vi "RTS Combination Server.vi"() -> ()   [LabVIEW 2016]
uses:
  Drivers/WAGO 750-881/Type Definitions/Wago Main Control.ctl
  Drivers/WAGO 750-881/Type Definitions/Wago Output Data Process Image.ctl
  Drivers/WAGO 750-881/Type Definitions/Wago Room Condtions.ctl
  Drivers/WAGO 750-881/Type Definitions/Wago Door Relays.ctl
  Drivers/WAGO 750-881/Type Definitions/Wago Contactor Settings.ctl
  Drivers/WAGO 750-881/Type Definitions/Wago Ground Leakage.ctl
  Drivers/WAGO 750-881/Type Definitions/Wago Input Process Image.ctl
  Drivers/WAGO 750-881/Type Definitions/Wago Room PID Settings.ctl
  Drivers/WAGO 750-881/Type Definitions/Wago Measured Input Data.ctl
  Drivers/WAGO 750-881/Type Definitions/Wago Room Setpoint Targets.ctl
  Type Definitions/RTS Modbus Connections.ctl
  <vilib>/NI/Modbus Library/API/Master/Modbus Master.lvclass
  Drivers/Yokogawa MX100/Type Definitions/MX100 Initialization.ctl
  Drivers/Yokogawa MX100/Type Definitions/MX100 Data.ctl
  Type Definitions/RTS Configuration Setup.ctl
  Type Definitions/RTS Wago Config.ctl
  Type Definitions/RTS APLUS Config.ctl
  Type Definitions/RTS Yokogawa MX Config.ctl
  Type Definitions/RTS Replay Server Control.ctl
  Type Definitions/RTS Server Configuration.ctl
  Type Definitions/RTS Station Settions TCP Comms.ctl
  Type Definitions/RTS Chamber Save Status.ctl
  Type Definitions/RTS Test Pattern.ctl
  Type Definitions/RTS Chamber Data.ctl
  Utility/Type Definitions/UTILITY Power Data.ctl
  Type Definitions/RTS Chamber TCs.ctl
  Type Definitions/RTS MX5 AUX Data.ctl
  Type Definitions/RTS TDMS Filename Locations.ctl
  Type Definitions/RTS Save References.ctl
  Type Definitions/RTS All Station Door Opener Ctrl.ctl
  Type Definitions/RTS Station Relay Ops.ctl
  Type Definitions/RTS Door Opener Indicator.ctl
  Type Definitions/RTS Door Ops Client.ctl
  Type Definitions/RTS Door Opening Schedule.ctl
  Type Definitions/RTS Door Ops Sequence.ctl
  Drivers/WAGO 750-881/Type Definitions/Wago Ground Leakage Relays.ctl
  Drivers/WAGO 750-881/Type Definitions/Wago Polarity Selector Relays.ctl
  Drivers/WAGO 750-881/Type Definitions/Wago Polarity Selector.ctl
  Type Definitions/RTS Chamber Temperature Humidity Control.ctl
  Type Definitions/RTS Frequency Selector.ctl
  Type Definitions/RTS Reset Watt Hours.ctl
  Drivers/WAGO 750-881/Type Definitions/Wago Voltage Adjustment Parameters.ctl
  Drivers/WAGO 750-881/Type Definitions/Wago Door Settings.ctl
  Drivers/WAGO 750-881/Type Definitions/Wago Door Relays By Station.ctl
  Drivers/WAGO 750-881/Type Definitions/Wago Door Operation.ctl
  Type Definitions/RTS Enable Door Openers.ctl
  Type Definitions/RTS Select System Number.ctl
  Drivers/WAGO 750-881/Type Definitions/Wago Room Run.ctl
  Drivers/WAGO 750-881/Type Definitions/Wago Room Enable.ctl
  Type Definitions/RTS Save Titles.ctl
  <vilib>/event_ctls.llb/usereventprio.ctl
  Drivers/WAGO 750-881/Type Definitions/Wago Input Commands.ctl
  Type Definitions/RTS TCP Multiple Connections Data.ctl
  Type Definitions/RTS Room Selector.ctl
  <vilib>/Utility/error.llb/whitespace.ctl
  <vilib>/NI/Modbus Library/API/Wrapper/Create TCP Master.vi
  <vilib>/NI/Modbus Library/API/Wrapper/API Main.lvlib
panel:
  in  "Save Array":bool
  out "Save Array":string[](array[string])
  out "Exit":bool=TRUE
  out "Start Data Save Loop":bool=TRUE
  in  "Save Rate (Sec)":i32=50
  out "Custom Saved Title Save Loop":T1
  out "TDMS Data Save Loop":T2
  out "RTS Config Setup Save Loop":T4
  out "All Door Opener Ctrl 2":T13 {"Station 8"."Station Slide"."Chamber 1-1"."Start Time" format="%<%X\n%x>T"; "Station 8"."Station Slide"."Chamber 1-1"."End Time" format="%<%X\n%x>T"; "Station 8"."Station Slide"."Time Count (s)" format="%.2f"; "Station 8"."Station Cab"."Chamber 1-1"."Start Time" format="%<%X\n%x>T"; "Station 8"."Station Cab"."Chamber 1-1"."End Time" format="%<%X\n%x>T"; "Station 8"."Station Cab"."Time Count (s)" format="%.2f"; "Station 8"."Station Freezer"."Chamber 1-1"."Start Time" format="%<%X\n%x>T"; "Station 8"."Station Freezer"."Chamber 1-1"."End Time" format="%<%X\n%x>T"; "Station 8"."Station Freezer"."Time Count (s)" format="%.2f"; "Station 7"."Station Slide"."Chamber 1-1"."Start Time" format="%<%X\n%x>T"; "Station 7"."Station Slide"."Chamber 1-1"."End Time" format="%<%X\n%x>T"; "Station 7"."Station Slide"."Time Count (s)" format="%.2f"; "Station 7"."Station Cab"."Chamber 1-1"."Start Time" format="%<%X\n%x>T"; "Station 7"."Station Cab"."Chamber 1-1"."End Time" format="%<%X\n%x>T"; "Station 7"."Station Cab"."Time Count (s)" format="%.2f"; "Station 7"."Station Freezer"."Chamber 1-1"."Start Time" format="%<%X\n%x>T"; "Station 7"."Station Freezer"."Chamber 1-1"."End Time" format="%<%X\n%x>T"; "Station 7"."Station Freezer"."Time Count (s)" format="%.2f"; "Station 6"."Station Slide"."Chamber 1-1"."Start Time" format="%<%X\n%x>T"; "Station 6"."Station Slide"."Chamber 1-1"."End Time" format="%<%X\n%x>T"; "Station 6"."Station Slide"."Time Count (s)" format="%.2f"; "Station 6"."Station Cab"."Chamber 1-1"."Start Time" format="%<%X\n%x>T"; "Station 6"."Station Cab"."Chamber 1-1"."End Time" format="%<%X\n%x>T"; "Station 6"."Station Cab"."Time Count (s)" format="%.2f"; "Station 6"."Station Freezer"."Chamber 1-1"."Start Time" format="%<%X\n%x>T"; "Station 6"."Station Freezer"."Chamber 1-1"."End Time" format="%<%X\n%x>T"; "Station 6"."Station Freezer"."Time Count (s)" format="%.2f"; "Station 5"."Station Slide"."Chamber 1-1"."Start Time" format="%<%X\n%x>T"; "Station 5"."Station Slide"."Chamber 1-1"."End Time" format="%<%X\n%x>T"; "Station 5"."Station Slide"."Time Count (s)" format="%.2f"; "Station 5"."Station Cab"."Chamber 1-1"."Start Time" format="%<%X\n%x>T"; "Station 5"."Station Cab"."Chamber 1-1"."End Time" format="%<%X\n%x>T"; "Station 5"."Station Cab"."Time Count (s)" format="%.2f"; "Station 5"."Station Freezer"."Chamber 1-1"."Start Time" format="%<%X\n%x>T"; "Station 5"."Station Freezer"."Chamber 1-1"."End Time" format="%<%X\n%x>T"; "Station 5"."Station Freezer"."Time Count (s)" format="%.2f"; "Station 4"."Station Slide"."Chamber 1-1"."Start Time" format="%<%X\n%x>T"; "Station 4"."Station Slide"."Chamber 1-1"."End Time" format="%<%X\n%x>T"; "Station 4"."Station Slide"."Time Count (s)" format="%.2f"; "Station 4"."Station Cab"."Chamber 1-1"."Start Time" format="%<%X\n%x>T"; "Station 4"."Station Cab"."Chamber 1-1"."End Time" format="%<%X\n%x>T"; "Station 4"."Station Cab"."Time Count (s)" format="%.2f"; "Station 4"."Station Freezer"."Chamber 1-1"."Start Time" format="%<%X\n%x>T"; "Station 4"."Station Freezer"."Chamber 1-1"."End Time" format="%<%X\n%x>T"; "Station 4"."Station Freezer"."Time Count (s)" format="%.2f"; "Station 3"."Station Slide"."Chamber 1-1"."Start Time" format="%<%X\n%x>T"; "Station 3"."Station Slide"."Chamber 1-1"."End Time" format="%<%X\n%x>T"; "Station 3"."Station Slide"."Time Count (s)" format="%.2f"; "Station 3"."Station Cab"."Chamber 1-1"."Start Time" format="%<%X\n%x>T"; "Station 3"."Station Cab"."Chamber 1-1"."End Time" format="%<%X\n%x>T"; "Station 3"."Station Cab"."Time Count (s)" format="%.2f"; "Station 3"."Station Freezer"."Chamber 1-1"."Start Time" format="%<%X\n%x>T"; "Station 3"."Station Freezer"."Chamber 1-1"."End Time" format="%<%X\n%x>T"; "Station 3"."Station Freezer"."Time Count (s)" format="%.2f"; "Station 2"."Station Slide"."Chamber 1-1"."Start Time" format="%<%X\n%x>T"; "Station 2"."Station Slide"."Chamber 1-1"."End Time" format="%<%X\n%x>T"; "Station 2"."Station Slide"."Time Count (s)" format="%.2f"; "Station 2"."Station Cab"."Chamber 1-1"."Start Time" format="%<%X\n%x>T"; "Station 2"."Station Cab"."Chamber 1-1"."End Time" format="%<%X\n%x>T"; "Station 2"."Station Cab"."Time Count (s)" format="%.2f"; "Station 2"."Station Freezer"."Chamber 1-1"."Start Time" format="%<%X\n%x>T"; "Station 2"."Station Freezer"."Chamber 1-1"."End Time" format="%<%X\n%x>T"; "Station 2"."Station Freezer"."Time Count (s)" format="%.2f"; "Station 1"."Station Slide"."Chamber 1-1"."Start Time" format="%<%X\n%x>T"; "Station 1"."Station Slide"."Chamber 1-1"."End Time" format="%<%X\n%x>T"; "Station 1"."Station Slide"."Time Count (s)" format="%.2f"; "Station 1"."Station Cab"."Chamber 1-1"."Start Time" format="%<%X\n%x>T"; "Station 1"."Station Cab"."Chamber 1-1"."End Time" format="%<%X\n%x>T"; "Station 1"."Station Cab"."Time Count (s)" format="%.2f"; "Station 1"."Station Freezer"."Chamber 1-1"."Start Time" format="%<%X\n%x>T"; "Station 1"."Station Freezer"."Chamber 1-1"."End Time" format="%<%X\n%x>T"; "Station 1"."Station Freezer"."Time Count (s)" format="%.2f"}
  out "System Number":T19="Sys1"
  in  "Disable MX":bool
  in  "Main Array":bool
  in  "All Data?":bool=TRUE
  in  "CSV Data Save":T2
  out "Main Array":string[](array[string])
  in  "Disable APLUS":bool
  in  "Initialize Rate":bool
  in  "Main Loop Rate (Seconds)":dbl=1.0
  out "Rate":dbl format="%0.2f"
  in  "K(0.3)":dbl=0.3 format="%#_13g"
  out "Chamber 1 Connections":i32
  in  "Tab Control":T20(tab)
  out "Chamber Data":T21 {"Room PID Settings"."Room Dehumid Temperature I (*RM Dehum I1)" max=30000 step=1; "Room PID Settings"."Room Dehumid Temperature P (*RM Dehum P1)" max=30000 step=1; "Room PID Settings"."Room Cool Temperature I (*RM Cool I1)" max=30000 step=1; "Room PID Settings"."Room Cool Temperature P (*RM Cool P1)" max=30000 step=1; "Room PID Settings"."Room Heat I (*RM Heat I1)" max=30000 step=1; "Room PID Settings"."Room Heat P (*RM Heat P1)" max=30000 step=1; "Room PID Settings"."Room Humidity I (*RM Hum I1)" max=30000 step=1; "Room PID Settings"."Room Humidity P (*RM Hum P1)" max=30000 step=1; "Room PID Settings"."Room Dry I (*RM Dry I1)" max=30000 step=1; "Room PID Settings"."Room Dry P(*RM Dry P1)" max=30000 step=1; "Station 8"."Voltage (V):Element 1 Avg" format="%.3g"; "Station 8"."Voltage (V):Element 2 Avg" format="%.3g"; "Station 8"."Max Watt Hours" format="%.3g"; "Station 8"."Power Factor:Element 2" format="%.3g"; "Station 8"."Power Factor:Element 1" format="%.3g"; "Station 8"."Apparent Power (VA):Element 2" format="%.3g"; "Station 8"."Apparent Power (VA):Element 1" format="%.3g"; "Station 8"."Frequency (Hz):Element 1" format="%.3g"; "Station 8"."Time:Element 1" format="%.3g"; "Station 8"."Voltage Crest Factor:Element 2" format="%.3g"; "Station 8"."Voltage Crest Factor:Element 1" format="%.3g"; "Station 8"."Voltage Harmonic (%):Element 2" format="%.3g"; "Station 8"."Voltage Harmonic (%):Element 1" format="%.3g"; "Station 8"."Current Crest Factor:Element 2" format="%.3g"; "Station 8"."Current Crest Factor:Element 1" format="%.3g"; "Station 8"."Voltage (V):Element 1" format="%.3g"; "Station 8"."Voltage (V):Element 2" format="%.3g"; "Station 8"."Watt Hours (Wh):Sigma" format="%.3f"; "Station 8"."Power (W):Sigma" format="%.3g"; "Station 8"."Current (A):Element 2" format="%.3g"; "Station 8"."Current (A):Element 1" format="%.3g"; "Station 7"."Voltage (V):Element 1 Avg" format="%.3g"; "Station 7"."Voltage (V):Element 2 Avg" format="%.3g"; "Station 7"."Max Watt Hours" format="%.3g"; "Station 7"."Power Factor:Element 2" format="%.3g"; "Station 7"."Power Factor:Element 1" format="%.3g"; "Station 7"."Apparent Power (VA):Element 2" format="%.3g"; "Station 7"."Apparent Power (VA):Element 1" format="%.3g"; "Station 7"."Frequency (Hz):Element 1" format="%.3g"; "Station 7"."Time:Element 1" format="%.3g"; "Station 7"."Voltage Crest Factor:Element 2" format="%.3g"; "Station 7"."Voltage Crest Factor:Element 1" format="%.3g"; "Station 7"."Voltage Harmonic (%):Element 2" format="%.3g"; "Station 7"."Voltage Harmonic (%):Element 1" format="%.3g"; "Station 7"."Current Crest Factor:Element 2" format="%.3g"; "Station 7"."Current Crest Factor:Element 1" format="%.3g"; "Station 7"."Voltage (V):Element 1" format="%.3g"; "Station 7"."Voltage (V):Element 2" format="%.3g"; "Station 7"."Watt Hours (Wh):Sigma" format="%.3f"; "Station 7"."Power (W):Sigma" format="%.3g"; "Station 7"."Current (A):Element 2" format="%.3g"; "Station 7"."Current (A):Element 1" format="%.3g"; "Station 6"."Voltage (V):Element 1 Avg" format="%.3g"; "Station 6"."Voltage (V):Element 2 Avg" format="%.3g"; "Station 6"."Max Watt Hours" format="%.3g"; "Station 6"."Power Factor:Element 2" format="%.3g"; "Station 6"."Power Factor:Element 1" format="%.3g"; "Station 6"."Apparent Power (VA):Element 2" format="%.3g"; "Station 6"."Apparent Power (VA):Element 1" format="%.3g"; "Station 6"."Frequency (Hz):Element 1" format="%.3g"; "Station 6"."Time:Element 1" format="%.3g"; "Station 6"."Voltage Crest Factor:Element 2" format="%.3g"; "Station 6"."Voltage Crest Factor:Element 1" format="%.3g"; "Station 6"."Voltage Harmonic (%):Element 2" format="%.3g"; "Station 6"."Voltage Harmonic (%):Element 1" format="%.3g"; "Station 6"."Current Crest Factor:Element 2" format="%.3g"; "Station 6"."Current Crest Factor:Element 1" format="%.3g"; "Station 6"."Voltage (V):Element 1" format="%.3g"; "Station 6"."Voltage (V):Element 2" format="%.3g"; "Station 6"."Watt Hours (Wh):Sigma" format="%.3f"; "Station 6"."Power (W):Sigma" format="%.3g"; "Station 6"."Current (A):Element 2" format="%.3g"; "Station 6"."Current (A):Element 1" format="%.3g"; "Station 5"."Voltage (V):Element 1 Avg" format="%.3g"; "Station 5"."Voltage (V):Element 2 Avg" format="%.3g"; "Station 5"."Max Watt Hours" format="%.3g"; "Station 5"."Power Factor:Element 2" format="%.3g"; "Station 5"."Power Factor:Element 1" format="%.3g"; "Station 5"."Apparent Power (VA):Element 2" format="%.3g"; "Station 5"."Apparent Power (VA):Element 1" format="%.3g"; "Station 5"."Frequency (Hz):Element 1" format="%.3g"; "Station 5"."Time:Element 1" format="%.3g"; "Station 5"."Voltage Crest Factor:Element 2" format="%.3g"; "Station 5"."Voltage Crest Factor:Element 1" format="%.3g"; "Station 5"."Voltage Harmonic (%):Element 2" format="%.3g"; "Station 5"."Voltage Harmonic (%):Element 1" format="%.3g"; "Station 5"."Current Crest Factor:Element 2" format="%.3g"; "Station 5"."Current Crest Factor:Element 1" format="%.3g"; "Station 5"."Voltage (V):Element 1" format="%.3g"; "Station 5"."Voltage (V):Element 2" format="%.3g"; "Station 5"."Watt Hours (Wh):Sigma" format="%.3f"; "Station 5"."Power (W):Sigma" format="%.3g"; "Station 5"."Current (A):Element 2" format="%.3g"; "Station 5"."Current (A):Element 1" format="%.3g"; "Station 4"."Voltage (V):Element 1 Avg" format="%.3g"; "Station 4"."Voltage (V):Element 2 Avg" format="%.3g"; "Station 4"."Max Watt Hours" format="%.3g"; "Station 4"."Power Factor:Element 2" format="%.3g"; "Station 4"."Power Factor:Element 1" format="%.3g"; "Station 4"."Apparent Power (VA):Element 2" format="%.3g"; "Station 4"."Apparent Power (VA):Element 1" format="%.3g"; "Station 4"."Frequency (Hz):Element 1" format="%.3g"; "Station 4"."Time:Element 1" format="%.3g"; "Station 4"."Voltage Crest Factor:Element 2" format="%.3g"; "Station 4"."Voltage Crest Factor:Element 1" format="%.3g"; "Station 4"."Voltage Harmonic (%):Element 2" format="%.3g"; "Station 4"."Voltage Harmonic (%):Element 1" format="%.3g"; "Station 4"."Current Crest Factor:Element 2" format="%.3g"; "Station 4"."Current Crest Factor:Element 1" format="%.3g"; "Station 4"."Voltage (V):Element 1" format="%.3g"; "Station 4"."Voltage (V):Element 2" format="%.3g"; "Station 4"."Watt Hours (Wh):Sigma" format="%.3f"; "Station 4"."Power (W):Sigma" format="%.3g"; "Station 4"."Current (A):Element 2" format="%.3g"; "Station 4"."Current (A):Element 1" format="%.3g"; "Station 3"."Voltage (V):Element 1 Avg" format="%.3g"; "Station 3"."Voltage (V):Element 2 Avg" format="%.3g"; "Station 3"."Max Watt Hours" format="%.3g"; "Station 3"."Power Factor:Element 2" format="%.3g"; "Station 3"."Power Factor:Element 1" format="%.3g"; "Station 3"."Apparent Power (VA):Element 2" format="%.3g"; "Station 3"."Apparent Power (VA):Element 1" format="%.3g"; "Station 3"."Frequency (Hz):Element 1" format="%.3g"; "Station 3"."Time:Element 1" format="%.3g"; "Station 3"."Voltage Crest Factor:Element 2" format="%.3g"; "Station 3"."Voltage Crest Factor:Element 1" format="%.3g"; "Station 3"."Voltage Harmonic (%):Element 2" format="%.3g"; "Station 3"."Voltage Harmonic (%):Element 1" format="%.3g"; "Station 3"."Current Crest Factor:Element 2" format="%.3g"; "Station 3"."Current Crest Factor:Element 1" format="%.3g"; "Station 3"."Voltage (V):Element 1" format="%.3g"; "Station 3"."Voltage (V):Element 2" format="%.3g"; "Station 3"."Watt Hours (Wh):Sigma" format="%.3f"; "Station 3"."Power (W):Sigma" format="%.3g"; "Station 3"."Current (A):Element 2" format="%.3g"; "Station 3"."Current (A):Element 1" format="%.3g"; "Station 2"."Voltage (V):Element 1 Avg" format="%.3g"; "Station 2"."Voltage (V):Element 2 Avg" format="%.3g"; "Station 2"."Max Watt Hours" format="%.3g"; "Station 2"."Power Factor:Element 2" format="%.3g"; "Station 2"."Power Factor:Element 1" format="%.3g"; "Station 2"."Apparent Power (VA):Element 2" format="%.3g"; "Station 2"."Apparent Power (VA):Element 1" format="%.3g"; "Station 2"."Frequency (Hz):Element 1" format="%.3g"; "Station 2"."Time:Element 1" format="%.3g"; "Station 2"."Voltage Crest Factor:Element 2" format="%.3g"; "Station 2"."Voltage Crest Factor:Element 1" format="%.3g"; "Station 2"."Voltage Harmonic (%):Element 2" format="%.3g"; "Station 2"."Voltage Harmonic (%):Element 1" format="%.3g"; "Station 2"."Current Crest Factor:Element 2" format="%.3g"; "Station 2"."Current Crest Factor:Element 1" format="%.3g"; "Station 2"."Voltage (V):Element 1" format="%.3g"; "Station 2"."Voltage (V):Element 2" format="%.3g"; "Station 2"."Watt Hours (Wh):Sigma" format="%.3f"; "Station 2"."Power (W):Sigma" format="%.3g"; "Station 2"."Current (A):Element 2" format="%.3g"; "Station 2"."Current (A):Element 1" format="%.3g"; "Station 1"."Voltage (V):Element 1 Avg" format="%.3g"; "Station 1"."Voltage (V):Element 2 Avg" format="%.3g"; "Station 1"."Max Watt Hours" format="%.3g"; "Station 1"."Power Factor:Element 2" format="%.3g"; "Station 1"."Power Factor:Element 1" format="%.3g"; "Station 1"."Apparent Power (VA):Element 2" format="%.3g"; "Station 1"."Apparent Power (VA):Element 1" format="%.3g"; "Station 1"."Frequency (Hz):Element 1" format="%.3g"; "Station 1"."Time:Element 1" format="%.3g"; "Station 1"."Voltage Crest Factor:Element 2" format="%.3g"; "Station 1"."Voltage Crest Factor:Element 1" format="%.3g"; "Station 1"."Voltage Harmonic (%):Element 2" format="%.3g"; "Station 1"."Voltage Harmonic (%):Element 1" format="%.3g"; "Station 1"."Current Crest Factor:Element 2" format="%.3g"; "Station 1"."Current Crest Factor:Element 1" format="%.3g"; "Station 1"."Voltage (V):Element 1" format="%.3g"; "Station 1"."Voltage (V):Element 2" format="%.3g"; "Station 1"."Watt Hours (Wh):Sigma" format="%.3f"; "Station 1"."Power (W):Sigma" format="%.3g"; "Station 1"."Current (A):Element 2" format="%.3g"; "Station 1"."Current (A):Element 1" format="%.3g"}
  out "RTS Config Setup Output":T4
  out "CSV Data Save Out":T2
  out "Error Out":errorcluster
  in  "Error In":errorcluster
  in  "All Door Opener Ctrl":T13 {"Station 8"."Station Slide"."Chamber 1-1"."Start Time" format="%<%X\n%x>T"; "Station 8"."Station Slide"."Chamber 1-1"."End Time" format="%<%X\n%x>T"; "Station 8"."Station Slide"."Time Count (s)" format="%.2f"; "Station 8"."Station Cab"."Chamber 1-1"."Start Time" format="%<%X\n%x>T"; "Station 8"."Station Cab"."Chamber 1-1"."End Time" format="%<%X\n%x>T"; "Station 8"."Station Cab"."Time Count (s)" format="%.2f"; "Station 8"."Station Freezer"."Chamber 1-1"."Start Time" format="%<%X\n%x>T"; "Station 8"."Station Freezer"."Chamber 1-1"."End Time" format="%<%X\n%x>T"; "Station 8"."Station Freezer"."Time Count (s)" format="%.2f"; "Station 7"."Station Slide"."Chamber 1-1"."Start Time" format="%<%X\n%x>T"; "Station 7"."Station Slide"."Chamber 1-1"."End Time" format="%<%X\n%x>T"; "Station 7"."Station Slide"."Time Count (s)" format="%.2f"; "Station 7"."Station Cab"."Chamber 1-1"."Start Time" format="%<%X\n%x>T"; "Station 7"."Station Cab"."Chamber 1-1"."End Time" format="%<%X\n%x>T"; "Station 7"."Station Cab"."Time Count (s)" format="%.2f"; "Station 7"."Station Freezer"."Chamber 1-1"."Start Time" format="%<%X\n%x>T"; "Station 7"."Station Freezer"."Chamber 1-1"."End Time" format="%<%X\n%x>T"; "Station 7"."Station Freezer"."Time Count (s)" format="%.2f"; "Station 6"."Station Slide"."Chamber 1-1"."Start Time" format="%<%X\n%x>T"; "Station 6"."Station Slide"."Chamber 1-1"."End Time" format="%<%X\n%x>T"; "Station 6"."Station Slide"."Time Count (s)" format="%.2f"; "Station 6"."Station Cab"."Chamber 1-1"."Start Time" format="%<%X\n%x>T"; "Station 6"."Station Cab"."Chamber 1-1"."End Time" format="%<%X\n%x>T"; "Station 6"."Station Cab"."Time Count (s)" format="%.2f"; "Station 6"."Station Freezer"."Chamber 1-1"."Start Time" format="%<%X\n%x>T"; "Station 6"."Station Freezer"."Chamber 1-1"."End Time" format="%<%X\n%x>T"; "Station 6"."Station Freezer"."Time Count (s)" format="%.2f"; "Station 5"."Station Slide"."Chamber 1-1"."Start Time" format="%<%X\n%x>T"; "Station 5"."Station Slide"."Chamber 1-1"."End Time" format="%<%X\n%x>T"; "Station 5"."Station Slide"."Time Count (s)" format="%.2f"; "Station 5"."Station Cab"."Chamber 1-1"."Start Time" format="%<%X\n%x>T"; "Station 5"."Station Cab"."Chamber 1-1"."End Time" format="%<%X\n%x>T"; "Station 5"."Station Cab"."Time Count (s)" format="%.2f"; "Station 5"."Station Freezer"."Chamber 1-1"."Start Time" format="%<%X\n%x>T"; "Station 5"."Station Freezer"."Chamber 1-1"."End Time" format="%<%X\n%x>T"; "Station 5"."Station Freezer"."Time Count (s)" format="%.2f"; "Station 4"."Station Slide"."Chamber 1-1"."Start Time" format="%<%X\n%x>T"; "Station 4"."Station Slide"."Chamber 1-1"."End Time" format="%<%X\n%x>T"; "Station 4"."Station Slide"."Time Count (s)" format="%.2f"; "Station 4"."Station Cab"."Chamber 1-1"."Start Time" format="%<%X\n%x>T"; "Station 4"."Station Cab"."Chamber 1-1"."End Time" format="%<%X\n%x>T"; "Station 4"."Station Cab"."Time Count (s)" format="%.2f"; "Station 4"."Station Freezer"."Chamber 1-1"."Start Time" format="%<%X\n%x>T"; "Station 4"."Station Freezer"."Chamber 1-1"."End Time" format="%<%X\n%x>T"; "Station 4"."Station Freezer"."Time Count (s)" format="%.2f"; "Station 3"."Station Slide"."Chamber 1-1"."Start Time" format="%<%X\n%x>T"; "Station 3"."Station Slide"."Chamber 1-1"."End Time" format="%<%X\n%x>T"; "Station 3"."Station Slide"."Time Count (s)" format="%.2f"; "Station 3"."Station Cab"."Chamber 1-1"."Start Time" format="%<%X\n%x>T"; "Station 3"."Station Cab"."Chamber 1-1"."End Time" format="%<%X\n%x>T"; "Station 3"."Station Cab"."Time Count (s)" format="%.2f"; "Station 3"."Station Freezer"."Chamber 1-1"."Start Time" format="%<%X\n%x>T"; "Station 3"."Station Freezer"."Chamber 1-1"."End Time" format="%<%X\n%x>T"; "Station 3"."Station Freezer"."Time Count (s)" format="%.2f"; "Station 2"."Station Slide"."Chamber 1-1"."Start Time" format="%<%X\n%x>T"; "Station 2"."Station Slide"."Chamber 1-1"."End Time" format="%<%X\n%x>T"; "Station 2"."Station Slide"."Time Count (s)" format="%.2f"; "Station 2"."Station Cab"."Chamber 1-1"."Start Time" format="%<%X\n%x>T"; "Station 2"."Station Cab"."Chamber 1-1"."End Time" format="%<%X\n%x>T"; "Station 2"."Station Cab"."Time Count (s)" format="%.2f"; "Station 2"."Station Freezer"."Chamber 1-1"."Start Time" format="%<%X\n%x>T"; "Station 2"."Station Freezer"."Chamber 1-1"."End Time" format="%<%X\n%x>T"; "Station 2"."Station Freezer"."Time Count (s)" format="%.2f"; "Station 1"."Station Slide"."Chamber 1-1"."Start Time" format="%<%X\n%x>T"; "Station 1"."Station Slide"."Chamber 1-1"."End Time" format="%<%X\n%x>T"; "Station 1"."Station Slide"."Time Count (s)" format="%.2f"; "Station 1"."Station Cab"."Chamber 1-1"."Start Time" format="%<%X\n%x>T"; "Station 1"."Station Cab"."Chamber 1-1"."End Time" format="%<%X\n%x>T"; "Station 1"."Station Cab"."Time Count (s)" format="%.2f"; "Station 1"."Station Freezer"."Chamber 1-1"."Start Time" format="%<%X\n%x>T"; "Station 1"."Station Freezer"."Chamber 1-1"."End Time" format="%<%X\n%x>T"; "Station 1"."Station Freezer"."Time Count (s)" format="%.2f"}
  out "Door Output Relays":T25
  in  "Test Chamber Set Parameters":bool
  out "Set Chamber Conditions":bool
  out "Matching Setpoints?":bool
  out "Room Setpoints Set Parameter Algo":T29
  out "Chamber Setpoint Reference":T16 {"Start Time" format="%<%X\n%x>T"; "End Time" format="%<%X\n%x>T"}
  out "Index":i32
  in  "Station 8 CMD":bool
  in  "Station 7 CMD":bool
  in  "Station 6 CMD":bool
  in  "Station 5 CMD":bool
  in  "Station 4 CMD":bool
  in  "Station 3 CMD":bool
  in  "Station 2 CMD":bool
  in  "Station 1 CMD":bool
  in  "Door Settings":T32={"Station 1"={"Freezer"=enum."Clear Time Close Door", "Cab"=enum."Clear Time Close Door", "Slide"=enum."Clear Time Close Door"}, "Station 2"={"Freezer"=enum."Clear Time Close Door", "Cab"=enum."Clear Time Close Door", "Slide"=enum."Clear Time Close Door"}, "Station 3"={"Freezer"=enum."Clear Time Close Door", "Cab"=enum."Clear Time Close Door", "Slide"=enum."Clear Time Close Door"}, "Station 4"={"Freezer"=enum."Clear Time Close Door", "Cab"=enum."Clear Time Close Door", "Slide"=enum."Clear Time Close Door"}, "Station 5"={"Freezer"=enum."Clear Time Close Door", "Cab"=enum."Clear Time Close Door", "Slide"=enum."Clear Time Close Door"}, "Station 6"={"Freezer"=enum."Clear Time Close Door", "Cab"=enum."Clear Time Close Door", "Slide"=enum."Clear Time Close Door"}, "Station 7"={"Freezer"=enum."Clear Time Close Door", "Cab"=enum."Clear Time Close Door", "Slide"=enum."Clear Time Close Door"}, "Station 8"={"Freezer"=enum."Clear Time Close Door", "Cab"=enum."Clear Time Close Door", "Slide"=enum."Clear Time Close Door"}, "Door Enable"=enum."Enable Door Openers"}
  in  "Room Run":T36
  in  "Room OK?":T37
  out "Custom Commands":string[](array[string])
  out "Read Door CMD":string
  out "Server to Client Data":string[][](array[string])
  in  "Reload PID":bool
  in  "Room PID Parameters":bool
  in  "Room PID Settings":T30={"Room Dry P(*RM Dry P1)"=200, "Room Dry I (*RM Dry I1)"=15000, "Room Humidity P (*RM Hum P1)"=400, "Room Humidity I (*RM Hum I1)"=15000, "Room Heat P (*RM Heat P1)"=1000, "Room Heat I (*RM Heat I1)"=2000, "Room Cool Temperature P (*RM Cool P1)"=500, "Room Cool Temperature I (*RM Cool I1)"=6000, "Room Dehumid Temperature P (*RM Dehum P1)"=500, "Room Dehumid Temperature I (*RM Dehum I1)"=6000} {"Room Dehumid Temperature I (*RM Dehum I1)" max=30000 step=1; "Room Dehumid Temperature P (*RM Dehum P1)" max=30000 step=1; "Room Cool Temperature I (*RM Cool I1)" max=30000 step=1; "Room Cool Temperature P (*RM Cool P1)" max=30000 step=1; "Room Heat I (*RM Heat I1)" max=30000 step=1; "Room Heat P (*RM Heat P1)" max=30000 step=1; "Room Humidity I (*RM Hum I1)" max=30000 step=1; "Room Humidity P (*RM Hum P1)" max=30000 step=1; "Room Dry I (*RM Dry I1)" max=30000 step=1; "Room Dry P(*RM Dry P1)" max=30000 step=1}
  in  "Wh Reset 8":T38 caption="Wh Reset"
  in  "Frequency 8":T39 caption="Frequency" items=["60 Hz", "50 Hz"]
  in  "Voltage 8":dbl caption="Voltage"
  in  "Wh Reset 7":T38 caption="Wh Reset"
  in  "Frequency 7":T39 caption="Frequency" items=["60 Hz", "50 Hz"]
  in  "Voltage 7":dbl caption="Voltage"
  in  "Wh Reset 6":T38 caption="Wh Reset"
  in  "Frequency 6":T39 caption="Frequency" items=["60 Hz", "50 Hz"]
  in  "Voltage 6":dbl caption="Voltage"
  in  "Wh Reset 5":T38 caption="Wh Reset"
  in  "Frequency 5":T39 caption="Frequency" items=["60 Hz", "50 Hz"]
  in  "Voltage 5":dbl caption="Voltage"
  in  "Wh Reset 4":T38 caption="Wh Reset"
  in  "Frequency 4":T39 caption="Frequency" items=["60 Hz", "50 Hz"]
  in  "Voltage 4":dbl caption="Voltage"
  in  "Wh Reset 3":T38 caption="Wh Reset"
  in  "Frequency 3":T39 caption="Frequency" items=["60 Hz", "50 Hz"]
  in  "Voltage 3":dbl caption="Voltage"
  in  "Wh Reset 2":T38 caption="Wh Reset"
  in  "Frequency 2":T39 caption="Frequency" items=["60 Hz", "50 Hz"]
  in  "Voltage 2":dbl caption="Voltage"
  in  "Wh Reset 1":T38 caption="Wh Reset"
  in  "Frequency":T39 items=["60 Hz", "50 Hz"]
  in  "Voltage":dbl
  in  "Station Voltage Send 5":bool
  in  "Station Voltage Send 1":bool
  in  "Station Voltage Send 6":bool
  in  "Station Voltage Send 2":bool
  in  "Station Voltage Send 7":bool
  in  "Station Voltage Send 3":bool
  in  "Station Voltage Send 8":bool
  in  "Station Voltage Send 4":bool
  in  "Polarity Selector":T40
  in  "Ground Leak Relays":T42
  out "Wago Data Output":T43 {"Input Process Image"."Software Constants"."Room PID Settings"."Room Dehumid Temperature I (*RM Dehum I1)" max=30000 step=1; "Input Process Image"."Software Constants"."Room PID Settings"."Room Dehumid Temperature P (*RM Dehum P1)" max=30000 step=1; "Input Process Image"."Software Constants"."Room PID Settings"."Room Cool Temperature I (*RM Cool I1)" max=30000 step=1; "Input Process Image"."Software Constants"."Room PID Settings"."Room Cool Temperature P (*RM Cool P1)" max=30000 step=1; "Input Process Image"."Software Constants"."Room PID Settings"."Room Heat I (*RM Heat I1)" max=30000 step=1; "Input Process Image"."Software Constants"."Room PID Settings"."Room Heat P (*RM Heat P1)" max=30000 step=1; "Input Process Image"."Software Constants"."Room PID Settings"."Room Humidity I (*RM Hum I1)" max=30000 step=1; "Input Process Image"."Software Constants"."Room PID Settings"."Room Humidity P (*RM Hum P1)" max=30000 step=1; "Input Process Image"."Software Constants"."Room PID Settings"."Room Dry I (*RM Dry I1)" max=30000 step=1; "Input Process Image"."Software Constants"."Room PID Settings"."Room Dry P(*RM Dry P1)" max=30000 step=1}
  in  "Room Setpoints":T46={"Room Setpoint Temperature (*RM Dry Set P1)"=90.0, "Room Setpoint Humidity (*RM Hum Set P1)"=20.0, "Room Cool Temperature (*RM Cool Setp 1)"=65.0, "Room Dehum Temperature (*RM De Hum Set P1)"=60.0} {"Room Dehum Temperature (*RM De Hum Set P1)" min=30.0 max=120.0; "Room Cool Temperature (*RM Cool Setp 1)" min=30.0 max=120.0; "Room Setpoint Humidity (*RM Hum Set P1)" min=5.0 max=98.0; "Room Setpoint Temperature (*RM Dry Set P1)" min=40.0 max=120.0}
  in  "Update Room Setpoint":bool
  in  "Voltage Adjustment Parameters":T47={"Volt Rate 1"=5, "Volt Rate 2"=5, "Volt Rate 3"=0, "Volt Rate 4"=0, "Volt Rate 5"=0, "Volt Rate 6"=0, "Volt Rate 7"=0, "Volt Rate 8"=0, "Volt Window 1 & 5"=30, "Volt Window 2 & 6"=60, "Volt Window 3 & 7 "=0, "Volt Window 4 & 8"=0}
  in  "Update Voltage Adjustment Parameters":bool
  in  "Core System Path":path=path "D:/RTSdata/Haier RTS"
  in  "Device Connections":T48={"Wago ModBus Connection"=refnum, "APLUS 1 Modbus Connection"=refnum, "APLUS 2 Modbus Connection"=refnum, "APLUS 3 Modbus Connection"=refnum, "APLUS 4 Modbus Connection"=refnum, "APLUS 5 Modbus Connection"=refnum, "APLUS 6 Modbus Connection"=refnum, "APLUS 7 Modbus Connection"=refnum, "APLUS 8 Modbus Connection"=refnum, "MX 1 VISA Connection"="", "MX 2 VISA Connection"="", "MX 3 VISA Connection"="", "MX 4 VISA Connection"="", "MX 5 VISA Connection"="", "MX1"={"Base Time"=0, "Session Number"=0, "Last Data Number"={"High"=-1, "Low"=4294967295}, "Channel List"=[], "FIFO Number (0)"=0, "Channel Number (1)"=1, "Select FIFO or Channel (F:Channel)"=FALSE, "MX100 Data"={"Measurement Values out"=[], "Date/Time"=""}}, "MX2"={"Base Time"=0, "Session Number"=0, "Last Data Number"={"High"=-1, "Low"=4294967295}, "Channel List"=[], "FIFO Number (0)"=0, "Channel Number (1)"=1, "Select FIFO or Channel (F:Channel)"=FALSE, "MX100 Data"={"Measurement Values out"=[], "Date/Time"=""}}, "MX3"={"Base Time"=0, "Session Number"=0, "Last Data Number"={"High"=-1, "Low"=4294967295}, "Channel List"=[], "FIFO Number (0)"=0, "Channel Number (1)"=1, "Select FIFO or Channel (F:Channel)"=FALSE, "MX100 Data"={"Measurement Values out"=[], "Date/Time"=""}}, "MX4"={"Base Time"=0, "Session Number"=0, "Last Data Number"={"High"=-1, "Low"=4294967295}, "Channel List"=[], "FIFO Number (0)"=0, "Channel Number (1)"=1, "Select FIFO or Channel (F:Channel)"=FALSE, "MX100 Data"={"Measurement Values out"=[], "Date/Time"=""}}, "MX5"={"Base Time"=0, "Session Number"=0, "Last Data Number"={"High"=-1, "Low"=4294967295}, "Channel List"=[], "FIFO Number (0)"=0, "Channel Number (1)"=1, "Select FIFO or Channel (F:Channel)"=FALSE, "MX100 Data"={"Measurement Values out"=[], "Date/Time"=""}}} {"MX5"."Channel Number (1)" min=1 max=60 step=1; "MX5"."FIFO Number (0)" min=-1 max=2 step=1; "MX4"."Channel Number (1)" min=1 max=60 step=1; "MX4"."FIFO Number (0)" min=-1 max=2 step=1; "MX3"."Channel Number (1)" min=1 max=60 step=1; "MX3"."FIFO Number (0)" min=-1 max=2 step=1; "MX2"."Channel Number (1)" min=1 max=60 step=1; "MX2"."FIFO Number (0)" min=-1 max=2 step=1; "MX1"."Channel Number (1)" min=1 max=60 step=1; "MX1"."FIFO Number (0)" min=-1 max=2 step=1}
  in  "Wago Data Input":T43 {"Input Process Image"."Software Constants"."Room PID Settings"."Room Dehumid Temperature I (*RM Dehum I1)" max=30000 step=1; "Input Process Image"."Software Constants"."Room PID Settings"."Room Dehumid Temperature P (*RM Dehum P1)" max=30000 step=1; "Input Process Image"."Software Constants"."Room PID Settings"."Room Cool Temperature I (*RM Cool I1)" max=30000 step=1; "Input Process Image"."Software Constants"."Room PID Settings"."Room Cool Temperature P (*RM Cool P1)" max=30000 step=1; "Input Process Image"."Software Constants"."Room PID Settings"."Room Heat I (*RM Heat I1)" max=30000 step=1; "Input Process Image"."Software Constants"."Room PID Settings"."Room Heat P (*RM Heat P1)" max=30000 step=1; "Input Process Image"."Software Constants"."Room PID Settings"."Room Humidity I (*RM Hum I1)" max=30000 step=1; "Input Process Image"."Software Constants"."Room PID Settings"."Room Humidity P (*RM Hum P1)" max=30000 step=1; "Input Process Image"."Software Constants"."Room PID Settings"."Room Dry I (*RM Dry I1)" max=30000 step=1; "Input Process Image"."Software Constants"."Room PID Settings"."Room Dry P(*RM Dry P1)" max=30000 step=1}
  # "RTS Server Application Interface"
  # "D:\\Hooks RTS"
  # "C:\\Technology Lab\\NI-2010\\Trunk\\Refrigeration\\RTS\\Old System"
  # "This application only polls the data from each of the \ninstruments. It will post the data in string comma delimited\nformat and post to TCP port."
  # "Chamber Conditions:"
  # "Chamber Conditions:"
  # "Chamber Conditions:"
  # "Chamber Conditions:"
  # "Chamber Conditions:"
  # "Chamber Conditions:"
  # "Chamber Conditions:"
  # "Chamber Conditions:"
  # "Chamber Conditions:"
  # "Chamber Conditions:"
  # "Chamber Conditions:"
  # "Chamber Conditions:"
  # "Chamber Conditions:"
  # "Chamber Conditions:"
  # "Chamber Conditions:"
  # "Chamber Conditions:"
  # "Chamber Conditions:"
  # "Chamber Conditions:"
  # "Chamber Conditions:"
  # "Chamber Conditions:"
  # "Chamber Conditions:"
  # "Chamber Conditions:"
  # "Chamber Conditions:"
  # "Chamber Conditions:"
  # "APLUS"
  # "MX100"
  # "Wago Controller"
  # "Chamber Conditions:"
  # "Chamber Conditions:"
  # "Chamber Conditions:"
  # "Chamber Conditions:"
  # "Chamber Conditions:"
  # "Chamber Conditions:"
  # "Chamber Conditions:"
  # "Chamber Conditions:"
  # "Chamber Conditions:"
  # "Chamber Conditions:"
  # "Chamber Conditions:"
  # "Chamber Conditions:"
  # "Chamber Conditions:"
  # "Chamber Conditions:"
  # "Chamber Conditions:"
  # "Chamber Conditions:"
  # "Chamber Conditions:"
  # "Chamber Conditions:"
  # "Chamber Conditions:"
  # "Chamber Conditions:"
  # "Chamber Conditions:"
  # "Chamber Conditions:"
  # "Chamber Conditions:"
  # "Chamber Conditions:"
  # "Chamber Conditions:"
  # "Voltage, Frequency & Watt Hour Selection"
  # "Station 1"
  # "Station 5"
  # "Station 2"
  # "Station 6"
  # "Station 3"
  # "Station 7"
  # "Station 4"
  # "Station 8"
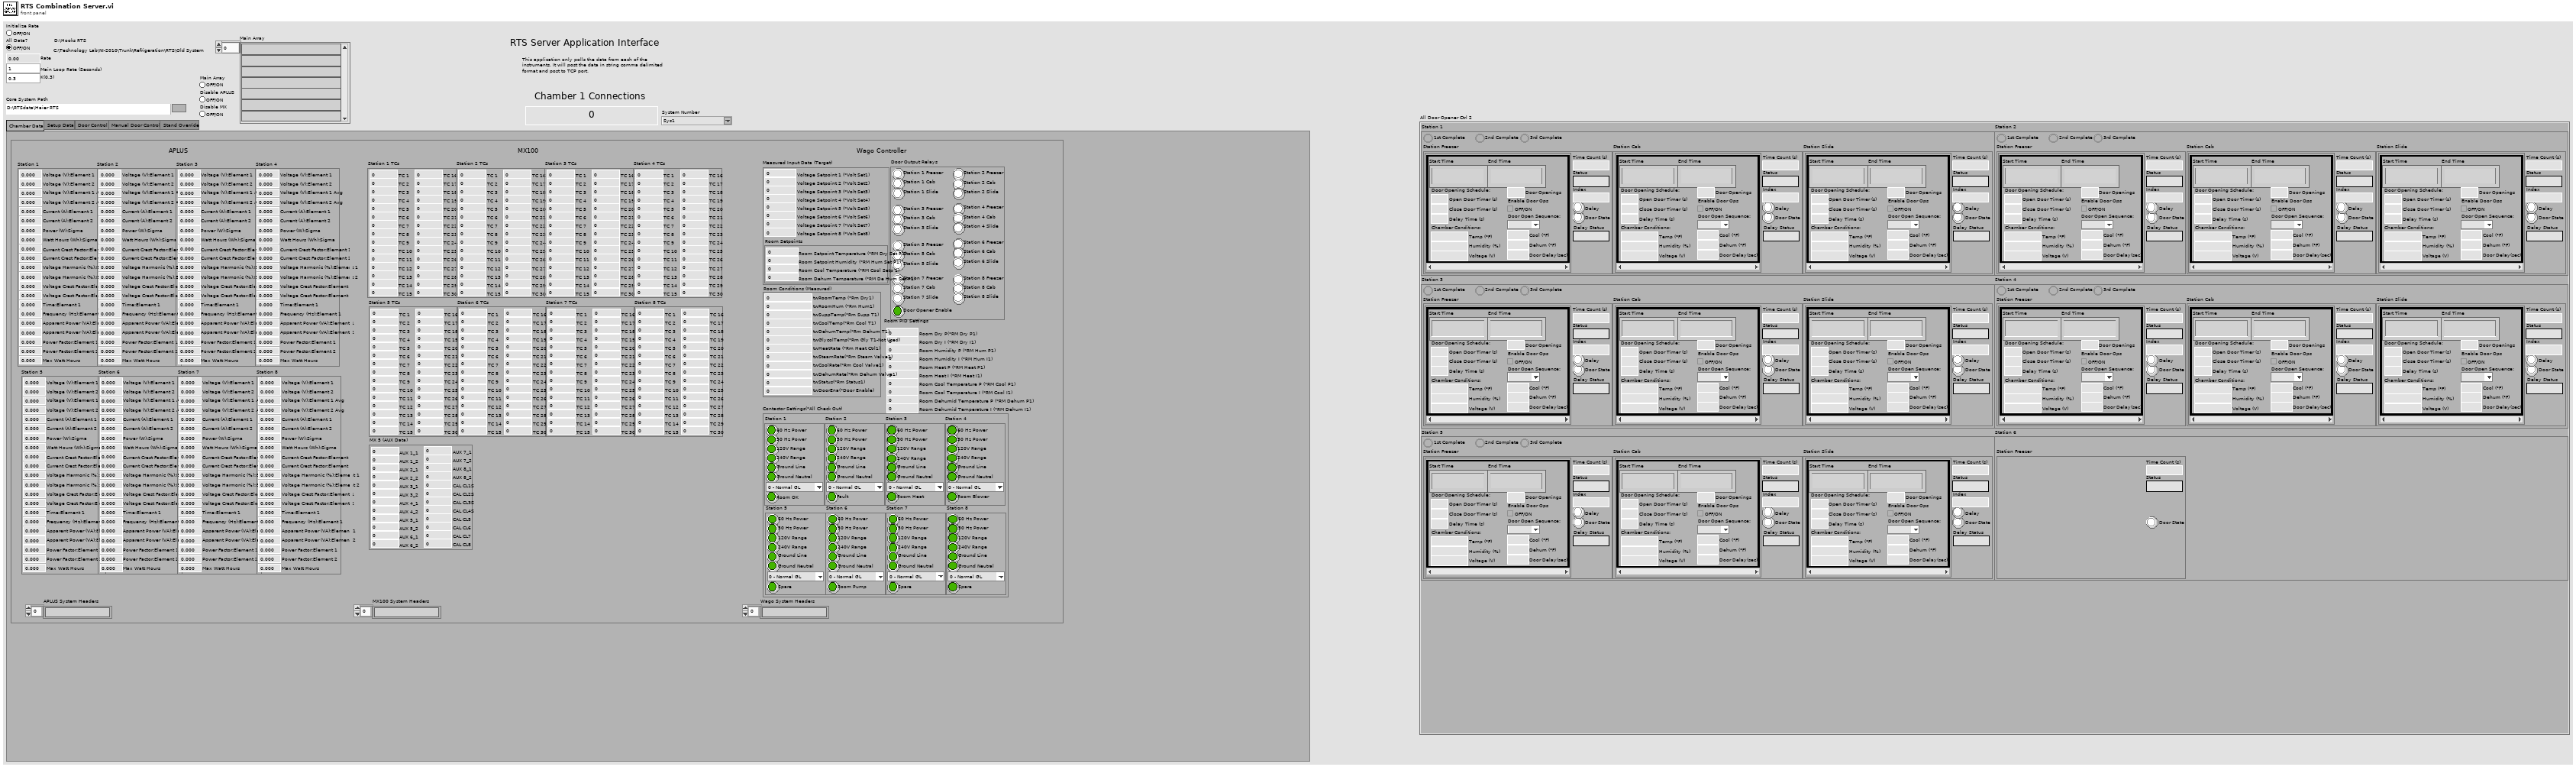
[diagram p1: front panel]
types:
  T1 = typedef "RTS Save Titles.ctl" = cluster{"Custom Saved Titles 1":string[][], "Custom Saved Titles 2":string[][], "Custom Saved Titles 3":string[][], "Custom Saved Titles 4":string[][], "Custom Saved Titles 5":string[][], "Custom Saved Titles 6":string[][], "Custom Saved Titles 7":string[][], "Custom Saved Titles 8":string[][]}
  T2 = typedef "RTS TDMS Filename Locations.ctl" = cluster{"CSV File Location":path, "CSV File Location 2":path, "CSV File Location 3":path, "CSV File Location 4":path, "CSV File Location 5":path, "CSV File Location 6":path, "CSV File Location 7":path, "CSV File Location 8":path, "Save References":T3}
  T3 = typedef "RTS Save References.ctl" = cluster{"CSV 1":refnum<file>, "CSV 2":refnum<file>, "CSV 3":refnum<file>, "CSV 4":refnum<file>, "CSV 5":refnum<file>, "CSV 6":refnum<file>, "CSV 7":refnum<file>, "CSV 8":refnum<file>}
  T4 = typedef "RTS Configuration Setup.ctl" = cluster{"Wago RTS":T5, "APLUS Array":T6[], "Yokogawa MX100 RTS Array":T7[], "Replay Server":T8[], "Server Configuration Array":T9[], "Station Settings":T10}
  T5 = typedef "RTS Wago Config.ctl" = cluster{"Disable":u16, "Interval":u16, "Controller":u16, "Address":u16, "IP Address":string, "AtoDmax":u16, "FullScale":u16, "VoltageType":u16, "Window1":u16, "Control1":u16, "Window2":u16, "Control2":u16}
  T6 = typedef "RTS APLUS Config.ctl" = cluster{"Disable":u16, "IP Address":string, "Input (4 Wire Unbalanced Load)":u16, "Dual Input (L1 115V, L2 230V)":u16, "LowLeakLimit":dbl, "Voltage Type":u16}
  T7 = typedef "RTS Yokogawa MX Config.ctl" = cluster{"IP Address":string, "TC Type":string, "Interval":u16, "Single Range":u16, "CalcWh":u16}
  T8 = typedef "RTS Replay Server Control.ctl" = cluster{"Interval":i16, "Repeat":u16, "Station":u16, "Load Path":path, "AutoMap":u16, "WattFactor":dbl, "AmpFactor":dbl}
  T9 = typedef "RTS Server Configuration.ctl" = cluster{"System":u16, "SysID":u16, "Title":string, "Enabled Server":u16, "Directory":string, "Configuration":string, "ValUpdate":u16, "TrendUpdate":u16, "ControlUpdate":u16, "Monitor":u16, "Pfact":u16, "Pipe":string, "TcpIP":u16, "Tunit":string, "ResultPath":path, "Door Sch DataLink":path, "MaxTCRate":u16, "Recovery":u16, "AutoRecovery":u16, "UsePowerFactor":u16, "OperatorPath":string, "Room":u16, "Station":u16, "Title":string, "DefMake":string, "Enabled Stall":u16, "Room":u16, "Title":string, "Station 1":u16, "Enabled 1":u16, "Station 2":u16, "Enabled 2":u16, "Station 3":u16, "Enabled 3":u16, "Station 4":u16, "Enabled 4":u16, "Station 5":u16, "Enabled 5":u16, "Station 6":u16, "Enabled 6":u16, "Station 7":u16, "Enabled 7":u16, "Station 8":u16, "Enabled 8":u16, "Title S1":string, "Title S2":string, "Title S3":string, "Title S5":string, "Title S6":string, "Title S7":string, "Title S8":string, "Title S4":string}
  T10 = typedef "RTS Station Settions TCP Comms.ctl" = cluster{"Point Files":cluster{"Point File 1":path, "Point File 2":path, "Point File 3":path, "Point File 4":path, "Point File 5":path, "Point File 6":path, "Point File 7":path, "Point File 8":path}, "Save Status":T11, "Setup Info":cluster{"Setup Info Station 1":string[][], "Setup Info Station 2":string[][], "Setup Info Station 3":string[][], "Setup Info Station 4":string[][], "Setup Info Station 5":string[][], "Setup Info Station 6":string[][], "Setup Info Station 7":string[][], "Setup Info Station 8":string[][]}, "Chamber Test Pattern":T12}
  T11 = typedef "RTS Chamber Save Status.ctl" = cluster{"Save Status 1":bool, "Save Status 2":bool, "Save Status 3":bool, "Save Status 4":bool, "Save Status 5":bool, "Save Status 6":bool, "Save Status 7":bool, "Save Status 8":bool}
  T12 = typedef "RTS Test Pattern.ctl" = cluster{" Pattern 1":path, "Pattern 2":path, "Pattern 3":path, "Pattern 4":path, "Pattern 5":path, "Pattern 6":path, "Pattern 7":path, "Pattern 8":path}
  T13 = typedef "RTS All Station Door Opener Ctrl.ctl" = cluster{"Station 1":T14, "Station 2":T14, "Station 3":T14, "Station 4":T14, "Station 5":T14, "Station 6":T14, "Station 7":T14, "Station 8":T14}
  T14 = typedef "RTS Station Relay Ops.ctl" = cluster{"Station Freezer":T15, "Station Cab":T15, "Station Slide":T15, "1st Complete":bool, "2nd Complete":bool, "3rd Complete":bool}
  T15 = typedef "RTS Door Opener Indicator.ctl" = cluster{"Time Count (s)":dbl, "Status":string, "Door State":bool, "Delay":bool, "Chamber 1-1":T16[], "Index":i32, "Delay Status":string}
  T16 = typedef "RTS Door Ops Client.ctl" = cluster{"End Time":timestamp, "Start Time":timestamp, "Door Opening Schedule:":T17, "Enable Door Ops":bool, "Door Openings":u32, "Temp (°F)":dbl, "Humidity (%)":dbl, "Voltage (V)":dbl, "Door Open Sequence:":T18, "Door Delay(sec)":dbl, "Dehum (°F)":dbl, "Cool (°F)":dbl}
  T17 = typedef "RTS Door Opening Schedule.ctl" = cluster{"Open Door Timer (s)":dbl, "Delay Time (s)":dbl, "Close Door Timer (s)":dbl}
  T18 = typedef "RTS Door Ops Sequence.ctl" = enum16{"", "1st", "2nd", "3rd"}
  T19 = typedef "RTS Select System Number.ctl" = string
  T20 = enum32{"Chamber Data", "Setup Data", "Door Control", "Manual Door Control", "Stand Override"}
  T21 = typedef "RTS Chamber Data.ctl" = cluster{"Station 1":T22, "Station 2":T22, "Station 3":T22, "Station 4":T22, "Station 5":T22, "Station 6":T22, "Station 7":T22, "Station 8":T22, "Station 1 TCs":T23, "Station 2 TCs":T23, "Station 3 TCs":T23, "Station 4 TCs":T23, "Station 5 TCs":T23, "Station 6 TCs":T23, "Station 7 TCs":T23, "Station 8 TCs":T23, "MX 5 (AUX Data)":T24, "Door Output Relays":T25, "Contactor Settings(*All Check Out)":T26, "Measured Input Data (Target)":T28, "Room PID Settings":T30, "Room Conditions (Measured)":T31, "APLUS System Headers":string[], "MX100 System Headers":string[], "Wago System Headers":string[]}
  T22 = typedef "UTILITY Power Data.ctl" = cluster{"Current (A):Element 1":dbl, "Current (A):Element 2":dbl, "Power (W):Sigma":dbl, "Watt Hours (Wh):Sigma":dbl, "Voltage (V):Element 2":dbl, "Voltage (V):Element 1":dbl, "Current Crest Factor:Element 1":dbl, "Current Crest Factor:Element 2":dbl, "Voltage Harmonic (%):Element 1":dbl, "Voltage Harmonic (%):Element 2":dbl, "Voltage Crest Factor:Element 1":dbl, "Voltage Crest Factor:Element 2":dbl, "Time:Element 1":dbl, "Frequency (Hz):Element 1":dbl, "Apparent Power (VA):Element 1":dbl, "Apparent Power (VA):Element 2":dbl, "Power Factor:Element 1":dbl, "Power Factor:Element 2":dbl, "Max Watt Hours":dbl, "Voltage (V):Element 2 Avg":dbl, "Voltage (V):Element 1 Avg":dbl}
  T23 = typedef "RTS Chamber TCs.ctl" = cluster{"TC 1":dbl, "TC 2":dbl, "TC 3":dbl, "TC 4":dbl, "TC 5":dbl, "TC 6":dbl, "TC 7":dbl, "TC 8":dbl, "TC 9":dbl, "TC 10":dbl, "TC 11":dbl, "TC 12":dbl, "TC 13":dbl, "TC 14":dbl, "TC 15":dbl, "TC 16":dbl, "TC 17":dbl, "TC 18":dbl, "TC 19":dbl, "TC 20":dbl, "TC 21":dbl, "TC 22":dbl, "TC 23":dbl, "TC 24":dbl, "TC 25":dbl, "TC 26":dbl, "TC 27":dbl, "TC 28":dbl, "TC 29":dbl, "TC 30":dbl}
  T24 = typedef "RTS MX5 AUX Data.ctl" = cluster{"AUX 1_1":dbl, "AUX 1_2":dbl, "AUX 2_1":dbl, "AUX 2_2":dbl, "AUX 3_1":dbl, "AUX 3_2":dbl, "AUX 4_1":dbl, "AUX 4_2":dbl, "AUX 5_1":dbl, "AUX 5_2":dbl, "AUX 6_1":dbl, "AUX 6_2":dbl, "AUX 7_1":dbl, "AUX 7_2":dbl, "AUX 8_1":dbl, "AUX 8_2":dbl, "CAL CL1S":dbl, "CAL CL2S":dbl, "CAL CL3S":dbl, "CAL CL4S":dbl, "CAL CL5":dbl, "CAL CL6":dbl, "CAL CL7":dbl, "CAL CL8":dbl}
  T25 = typedef "Wago Door Relays.ctl" = cluster{"Station 1 Freezer":bool, "Station 1 Cab":bool, "Station 1 Slide":bool, "Station 2 Freezer":bool, "Station 2 Cab":bool, "Station 2 Slide":bool, "Station 3 Freezer":bool, "Station 3 Cab":bool, "Station 3 Slide":bool, "Station 4 Freezer":bool, "Station 4 Cab":bool, "Station 4 Slide":bool, "Station 5 Freezer":bool, "Station 5 Cab":bool, "Station 5 Slide":bool, "Station 6 Freezer":bool, "Station 6 Cab":bool, "Station 6 Slide":bool, "Station 7 Freezer":bool, "Station 7 Cab":bool, "Station 7 Slide":bool, "Station 8 Freezer":bool, "Station 8 Cab":bool, "Station 8 Slide":bool, "Door Opener Enable":bool}
  T26 = typedef "Wago Contactor Settings.ctl" = cluster{"Station 1":cluster{"60 Hz Power":bool, "50 Hz Power":bool, "120V Range":bool, "240V Range":bool, "Ground Line":bool, "Ground Neutral":bool, "Room OK":bool, "Ground Leakage":T27}, "Station 2":cluster{"60 Hz Power":bool, "50 Hz Power":bool, "120V Range":bool, "240V Range":bool, "Ground Line":bool, "Ground Neutral":bool, "Fault":bool, "Ground Leakage":T27}, "Station 3":cluster{"60 Hz Power":bool, "50 Hz Power":bool, "120V Range":bool, "240V Range":bool, "Ground Line":bool, "Ground Neutral":bool, "Room Heat":bool, "Ground Leakage":T27}, "Station 4":cluster{"60 Hz Power":bool, "50 Hz Power":bool, "120V Range":bool, "240V Range":bool, "Ground Line":bool, "Ground Neutral":bool, "Room Blower":bool, "Ground Leakage":T27}, "Station 5":cluster{"60 Hz Power":bool, "50 Hz Power":bool, "120V Range":bool, "240V Range":bool, "Ground Line":bool, "Ground Neutral":bool, "Spare":bool, "Ground Leakage":T27}, "Station 6":cluster{"60 Hz Power":bool, "50 Hz Power":bool, "120V Range":bool, "240V Range":bool, "Ground Line":bool, "Ground Neutral":bool, "Room Pump":bool, "Ground Leakage":T27}, "Station 7":cluster{"60 Hz Power":bool, "50 Hz Power":bool, "120V Range":bool, "240V Range":bool, "Ground Line":bool, "Ground Neutral":bool, "Spare":bool, "Ground Leakage":T27}, "Station 8":cluster{"60 Hz Power":bool, "50 Hz Power":bool, "120V Range":bool, "240V Range":bool, "Ground Line":bool, "Ground Neutral":bool, "Spare":bool, "Ground Leakage":T27}}
  T27 = typedef "Wago Ground Leakage.ctl" = enum16{"0 - Normal GL", "1 - Measure GL"}
  T28 = typedef "Wago Measured Input Data.ctl" = cluster{"Voltage Setpoint 1 (*Volt Set1)":dbl, "Voltage Setpoint 2 (*Volt Set2)":dbl, "Voltage Setpoint 3 (*Volt Set3)":dbl, "Voltage Setpoint 4 (*Volt Set4)":dbl, "Voltage Setpoint 5 (*Volt Set5)":dbl, "Voltage Setpoint 6 (*Volt Set6)":dbl, "Voltage Setpoint 7 (*Volt Set7)":dbl, "Voltage Setpoint 8 (*Volt Set8)":dbl, "Room Setpoints":T29}
  T29 = typedef "Wago Room Setpoint Targets.ctl" = cluster{"Room Setpoint Temperature (*RM Dry Set P1)":dbl, "Room Setpoint Humidity (*RM Hum Set P1)":dbl, "Room Cool Temperature (*RM Cool Setp 1)":dbl, "Room Dehum Temperature (*RM De Hum Set P1)":dbl}
  T30 = typedef "Wago Room PID Settings.ctl" = cluster{"Room Dry P(*RM Dry P1)":u16, "Room Dry I (*RM Dry I1)":u16, "Room Humidity P (*RM Hum P1)":u16, "Room Humidity I (*RM Hum I1)":u16, "Room Heat P (*RM Heat P1)":u16, "Room Heat I (*RM Heat I1)":u16, "Room Cool Temperature P (*RM Cool P1)":u16, "Room Cool Temperature I (*RM Cool I1)":u16, "Room Dehumid Temperature P (*RM Dehum P1)":u16, "Room Dehumid Temperature I (*RM Dehum I1)":u16}
  T31 = typedef "Wago Room Condtions.ctl" = cluster{"twDoorEna(*Door Enable)":u16, "twStatus(*Rm Status1)":u16, "twRoomTemp (*Rm Dry1)":dbl, "twRoomHum (*Rm Hum1)":dbl, "twSuppTemp(*Rm Supp T1)":dbl, "twCoolTemp(*Rm Cool T1)":dbl, "twDehumTemp(*Rm Dehum T1)":dbl, "twGlycolTemp(*Rm Gly T1-Not Used)":dbl, "twDehumRate(*Rm Dehum Valve1)":dbl, "twCoolRate(*Rm Cool Valve1)":dbl, "twSteamRate(*Rm Steam Valve1)":dbl, "twHeatRate (*Rm Heat Ctrl1)":dbl}
  T32 = typedef "Wago Door Settings.ctl" = cluster{"Station 1":T33, "Station 2":T33, "Station 3":T33, "Station 4":T33, "Station 5":T33, "Station 6":T33, "Station 7":T33, "Station 8":T33, "Door Enable":T35}
  T33 = typedef "Wago Door Relays By Station.ctl" = cluster{"Freezer":T34, "Cab":T34, "Slide":T34}
  T34 = typedef "Wago Door Operation.ctl" = enum16{"Clear Time Close Door", "Open Door", "Close Door", "PLC Timed Door Op"}
  T35 = typedef "RTS Enable Door Openers.ctl" = enum16{"Disable Door Openers", "Enable Door Openers"}
  T36 = typedef "Wago Room Run.ctl" = enum16{"Room Shutdown", "Room Run"}
  T37 = typedef "Wago Room Enable.ctl" = enum16{"Room Disable", "Room OK"}
  T38 = typedef "RTS Reset Watt Hours.ctl" = enum16{"", "Reset Watt Hours"}
  T39 = typedef "RTS Frequency Selector.ctl" = u16
  T40 = typedef "Wago Polarity Selector Relays.ctl" = cluster{"Station 1":T41, "Station 2":T41, "Station 3":T41, "Station 4":T41, "Station 5":T41, "Station 6":T41, "Station 7":T41, "Station 8":T41}
  T41 = typedef "Wago Polarity Selector.ctl" = enum16{"Ground Neutral", "Ground Line"}
  T42 = typedef "Wago Ground Leakage Relays.ctl" = cluster{"Ground Leakage 1":T27, "Ground Leakage 2":T27, "Ground Leakage 3":T27, "Ground Leakage 4":T27, "Ground Leakage 5":T27, "Ground Leakage 6":T27, "Ground Leakage 7":T27, "Ground Leakage 8":T27}
  T43 = typedef "Wago Main Control.ctl" = cluster{"Output Data Process Image":T44, "Input Process Image":T45, "System Send Data":string[][], "System Data To Save":string[][]}
  T44 = typedef "Wago Output Data Process Image.ctl" = cluster{"Room Door Opener Status":cluster{"Station 1, Door 1":u16, "Station 1, Door 2":u16, "Station 1, Door 3":u16, "Station 2, Door 1":u16, "Station 2, Door 2":u16, "Station 2, Door 3":u16, "Station 3, Door 1":u16, "Station 3, Door 2":u16, "Station 3, Door 3":u16, "Station 4, Door 1":u16, "Station 4, Door 2":u16, "Station 4, Door 3":u16, "Station 5, Door 1":u16, "Station 5, Door 2":u16, "Station 5, Door 3":u16, "Station 6, Door 1":u16, "Station 6, Door 2":u16, "Station 6, Door 3":u16, "Station 7, Door 1":u16, "Station 7, Door 2":u16, "Station 7, Door 3":u16, "Station 8, Door 1":u16, "Station 8, Door 2":u16, "Station 8, Door 3":u16}, "Room Conditions (Measured)":T31, "Chamber AO Controls (Controls Chamber)":cluster{"twDehumCtrl (mA)":u16, "twCoolCtrl (mA)":u16, "twSteamCtrl (mA)":u16, "twHeatCtrl (mA)":u16}, "Variac Output(*All Check Out)":cluster{"Station 1 Volt Increase":bool, "Station 1 Volt Decrease":bool, "Station 2 Volt Increase":bool, "Station 2 Volt Decrease":bool, "Station 3 Volt Increase":bool, "Station 3 Volt Decrease":bool, "Station 4 Volt Increase":bool, "Station 4 Volt Decrease":bool, "Station 5 Volt Increase":bool, "Station 5 Volt Decrease":bool, "Station 6 Volt Increase":bool, "Station 6 Volt Decrease":bool, "Station 7 Volt Increase":bool, "Station 7 Volt Decrease":bool, "Station 8 Volt Increase":bool, "Station 8 Volt Decrease":bool}, "Door Output Relays":T25, "Wago Input Voltage Monitor (*Target_ All Check Out)":cluster{"twWoltMon1":dbl, "twWoltMon2":dbl, "twWoltMon3":dbl, "twWoltMon4":dbl, "twWoltMon5":dbl, "twWoltMon6":dbl, "twWoltMon7":dbl, "twWoltMon8":dbl, "twVoltStat1":u16, "twVoltStat2":u16, "twVoltStat3":u16, "twVoltStat4":u16, "twVoltStat5":u16, "twVoltStat6":u16, "twVoltStat7":u16, "twVoltStat8":u16}, "Contactor Settings(*All Check Out)":T26}
  T45 = typedef "Wago Input Process Image.ctl" = cluster{"fbEstop":bool, "fbDoors":bool, "fbSafety":bool, "Input Variables":cluster{"Station 1 Volt 1":dbl, "Station 1 Volt 2":dbl, "Station 2 Volt 1":dbl, "Station 2 Volt 2":dbl, "Station 3 Volt 1":dbl, "Station 3 Volt 2":dbl, "Station 4 Volt 1":dbl, "Station 4 Volt 2":dbl, "Station 5 Volt 1":dbl, "Station 5 Volt 2":dbl, "Station 6 Volt 1":dbl, "Station 6 Volt 2":dbl, "Station 7 Volt 1":dbl, "Station 7 Votl 2":dbl, "Station 8 Volt 1":dbl, "Station 8 Volt 2":dbl}, "Input Data":cluster{"Room Humidity  (Measured)":dbl, "Room Temperature (Measured)":dbl, "Spare 1":dbl, "Spare 2":dbl, "Supply Temperature (Measured)":dbl, "Cooling Temperature (Measured)":dbl, "Dehumidification Temperature (Measured)":dbl, "Un-used":dbl}, "Software Constants":cluster{"Volt Rate 1":u16, "Volt Rate 2":u16, "Volt Rate 3":u16, "Volt Rate 4":u16, "Volt Rate 5":u16, "Volt Rate 6":u16, "Volt Rate 7":u16, "Volt Rate 8":u16, "Volt Window 1":u16, "Volt Window 2":u16, "Volt Window 3":u16, "Volt Window 4":u16, "Volt Window 5":u16, "Volt Window 6":u16, "Volt Window 7":u16, "Volt Window 8":u16, "Voltage Range 1":u16, "Voltage Range 2":u16, "Voltage Range 3":u16, "Voltage Range 4":u16, "Voltage Range 5":u16, "Voltage Range 6":u16, "Voltage Range 7":u16, "Voltage Range 8":u16, "Voltage Polarity 1":u16, "Voltage Polarity 2":u16, "Voltage Polarity 3":u16, "Voltage Polarity 4":u16, "Voltage Polarity 5":u16, "Voltage Polarity 6":u16, "Voltage Polarity 7":u16, "Voltage Polarity 8":u16, "Room Run":bool, "Room OK":bool, "Room Testing":bool, "Room PID Settings":T30}, "Measured Input Data (Target)":T28}
  T46 = typedef "RTS Chamber Temperature Humidity Control.ctl" = cluster{"Room Setpoint Temperature (*RM Dry Set P1)":dbl, "Room Setpoint Humidity (*RM Hum Set P1)":dbl, "Room Cool Temperature (*RM Cool Setp 1)":dbl, "Room Dehum Temperature (*RM De Hum Set P1)":dbl}
  T47 = typedef "Wago Voltage Adjustment Parameters.ctl" = cluster{"Volt Rate 1":u16, "Volt Rate 2":u16, "Volt Rate 3":u16, "Volt Rate 4":u16, "Volt Rate 5":u16, "Volt Rate 6":u16, "Volt Rate 7":u16, "Volt Rate 8":u16, "Volt Window 1 & 5":u16, "Volt Window 2 & 6":u16, "Volt Window 3 & 7 ":u16, "Volt Window 4 & 8":u16}
  T48 = typedef "RTS Modbus Connections.ctl" = cluster{"Wago ModBus Connection":refnum<class "Modbus Master.lvclass">, "APLUS 1 Modbus Connection":refnum<class "Modbus Master.lvclass">, "APLUS 2 Modbus Connection":refnum<class "Modbus Master.lvclass">, "APLUS 3 Modbus Connection":refnum<class "Modbus Master.lvclass">, "APLUS 4 Modbus Connection":refnum<class "Modbus Master.lvclass">, "APLUS 5 Modbus Connection":refnum<class "Modbus Master.lvclass">, "APLUS 6 Modbus Connection":refnum<class "Modbus Master.lvclass">, "APLUS 7 Modbus Connection":refnum<class "Modbus Master.lvclass">, "APLUS 8 Modbus Connection":refnum<class "Modbus Master.lvclass">, "MX 1 VISA Connection":refnum<visa-resource-name>, "MX 2 VISA Connection":refnum<visa-resource-name>, "MX 3 VISA Connection":refnum<visa-resource-name>, "MX 4 VISA Connection":refnum<visa-resource-name>, "MX 5 VISA Connection":refnum<visa-resource-name>, "MX1":T49, "MX2":T49, "MX3":T49, "MX4":T49, "MX5":T49}
  T49 = typedef "MX100 Initialization.ctl" = cluster{"Base Time":i32, "Session Number":i32, "Last Data Number":cluster{"High":i32, "Low":u32}, "Channel List":string[], "FIFO Number (0)":i32, "Channel Number (1)":i32, "Select FIFO or Channel (F:Channel)":bool, "MX100 Data":T50}
  T50 = typedef "MX100 Data.ctl" = cluster{"Measurement Values out":dbl[], "Date/Time":string}
  T51 = enum32{"invalid app kind", "Development System", "Run Time System", "Student Edition", "Embedded LabVIEW", "Evaluation", "Custom"}
  T52 = enum32{"Invalid", "Standard", "Closed", "Hidden", "Minimized", "Maximized"}
  T53 = typedef "RTS Room Selector.ctl" = string
  T54 = typedef "RTS TCP Multiple Connections Data.ctl" = cluster{"Clients":refnum<k5>[], "Listener":refnum<k5>, "Data Array":string[]}
  T55 = cluster{"Core":cluster{"Current VI Reference":refnum<vi>, "Close Panel on Exit?":bool}, "Wago Data Input":T43, "Device Connections":T48, "Modbus Remote Port":u16, "Chamber Data":T21, "Data":T54, "RTS Config Setup":T4, "Send Data":string[][], "CSV Data Save":T2, "All Door Opener Ctrl":T13, "Custom Command":string[]}
  T56 = typedef "Wago Input Commands.ctl" = u16
  T57 = cluster{"Current VI Reference":refnum<vi>, "Close Panel on Exit?":bool}
  T58 = typedef "whitespace.ctl" = u16
  T59 = typedef "usereventprio.ctl" = enum32{"high priority", "normal priority"}
  T60 = cluster{"Core":cluster{"Current VI Reference":refnum<vi>, "Close Panel on Exit?":bool}, "CSV Data Save (Updated)":T2}
  T61 = cluster{"CSV 1":bool, "CSV 2":bool, "CSV 3":bool, "CSV 4":bool, "CSV 5":bool, "CSV 6":bool, "CSV 7":bool, "CSV 8":bool}
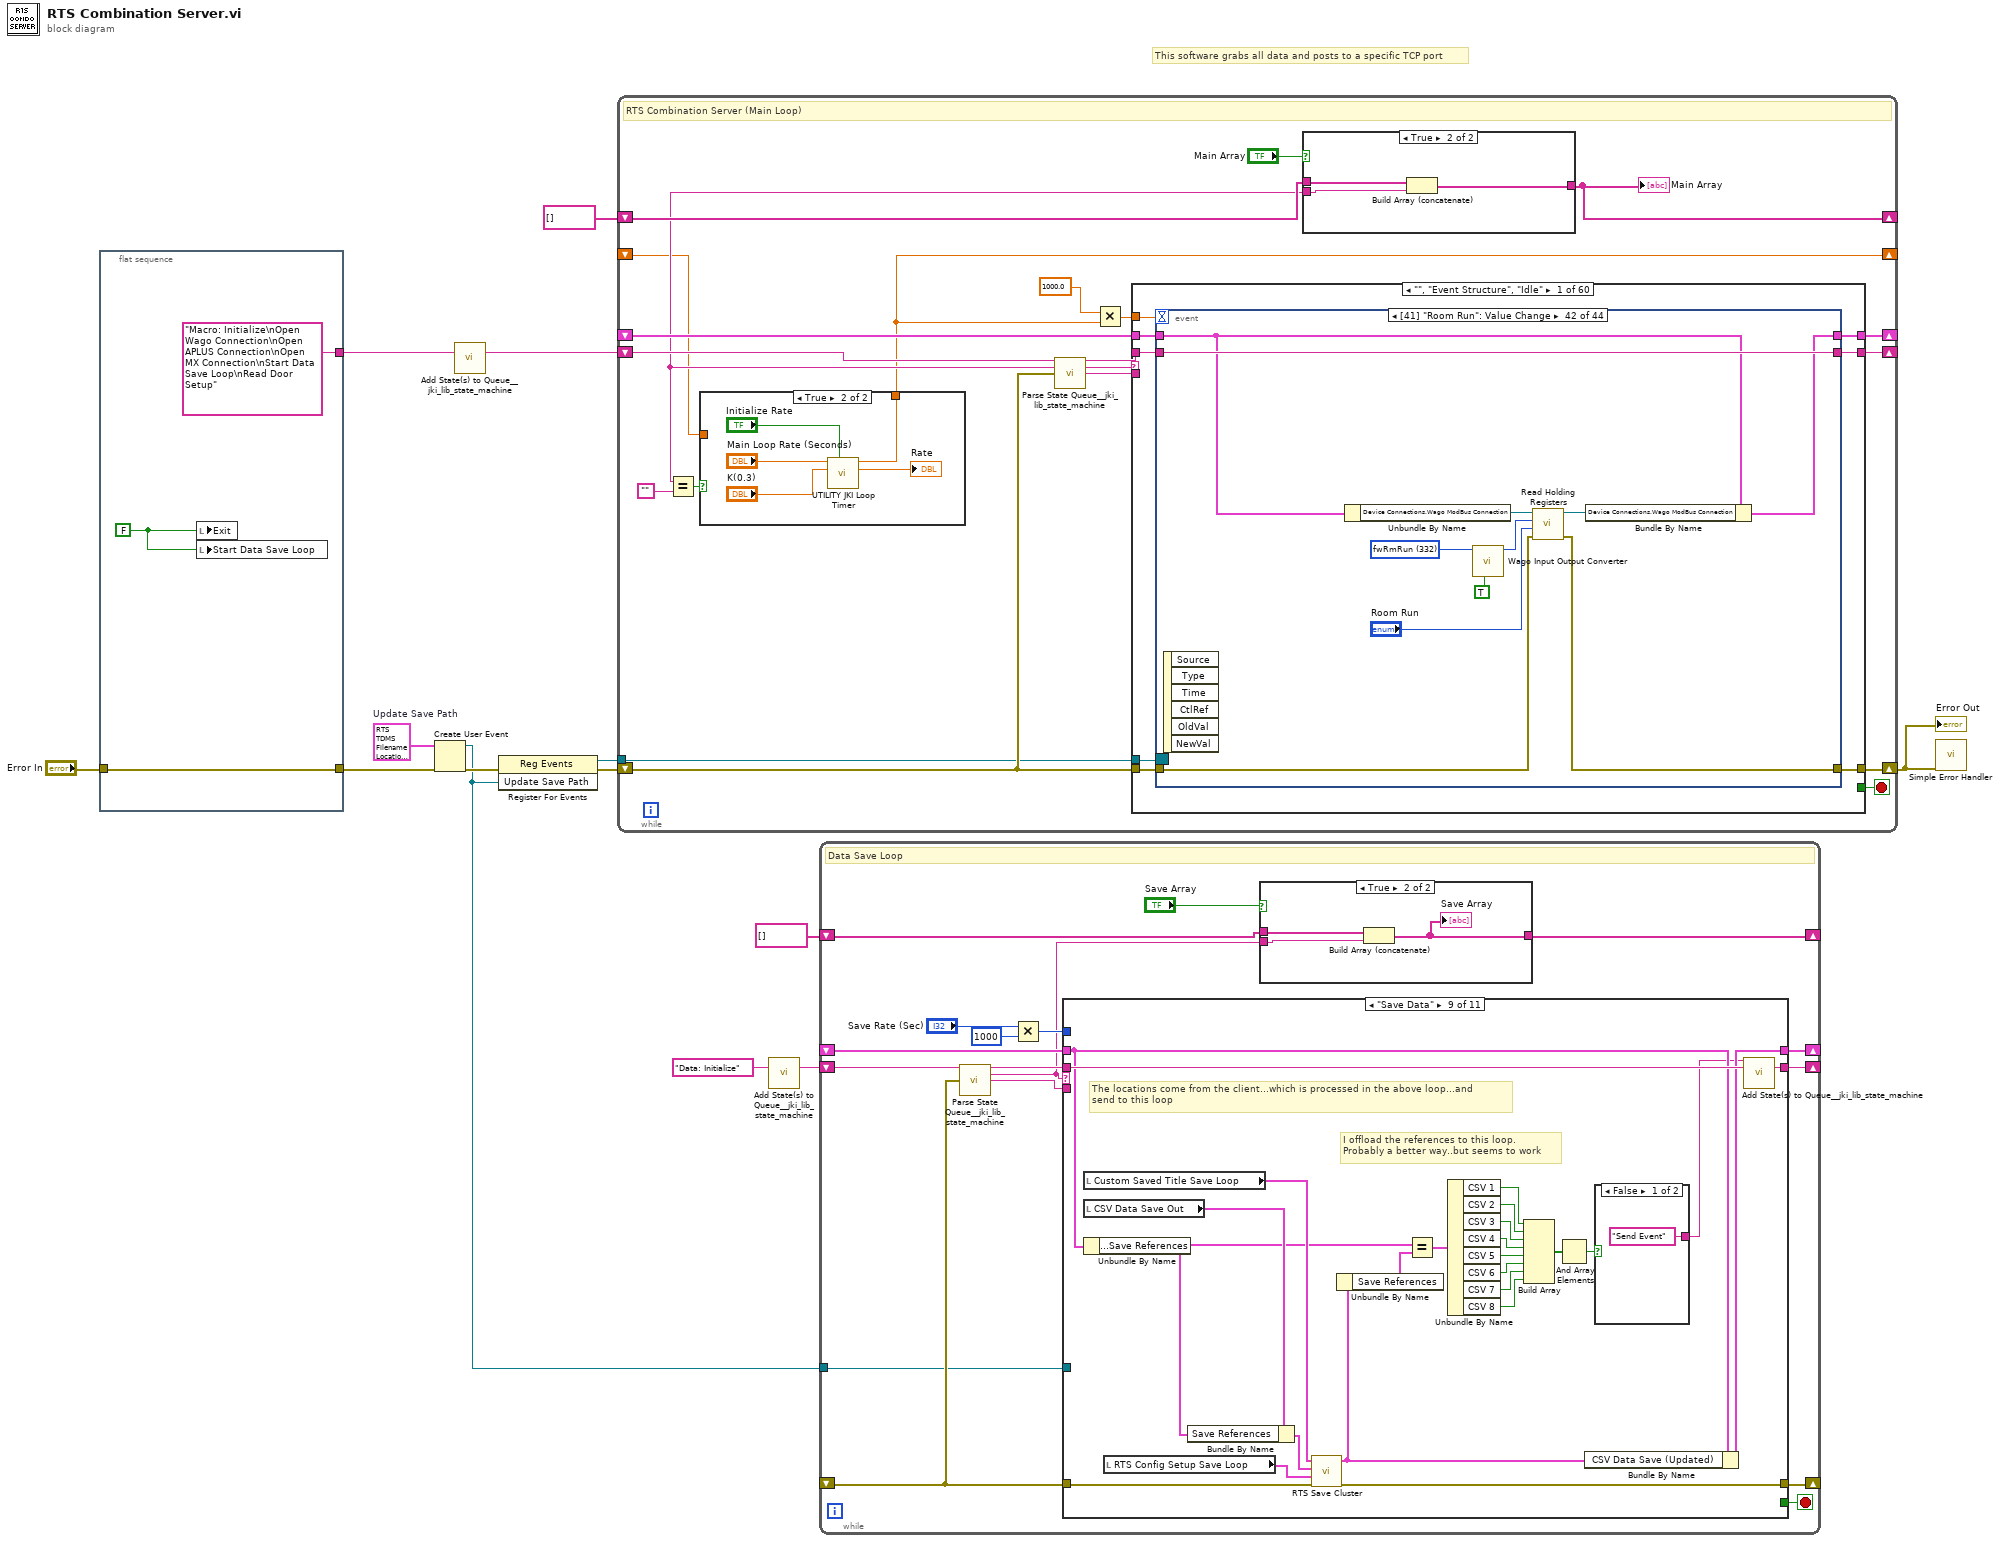
[diagram p0: block diagram]
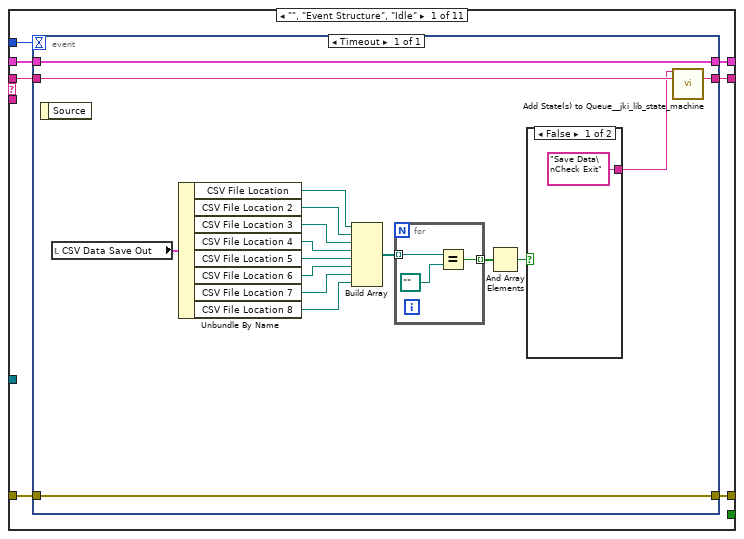
[diagram p3: hidden frame]
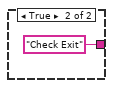
[diagram p4: hidden frame]
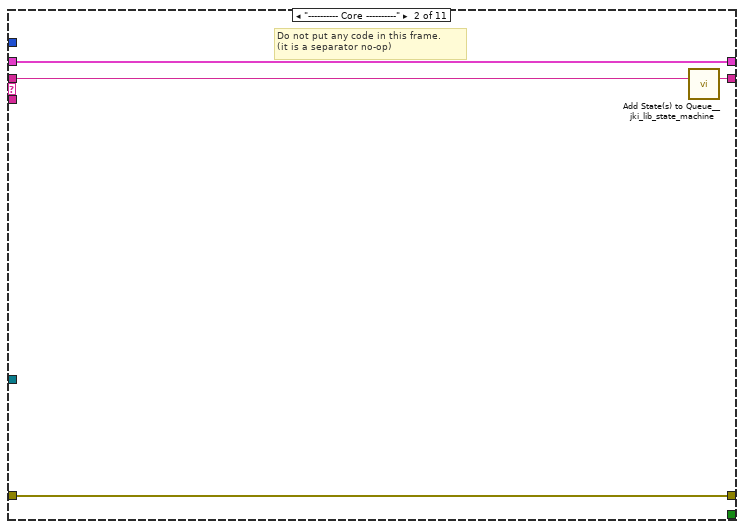
[diagram p5: hidden frame]
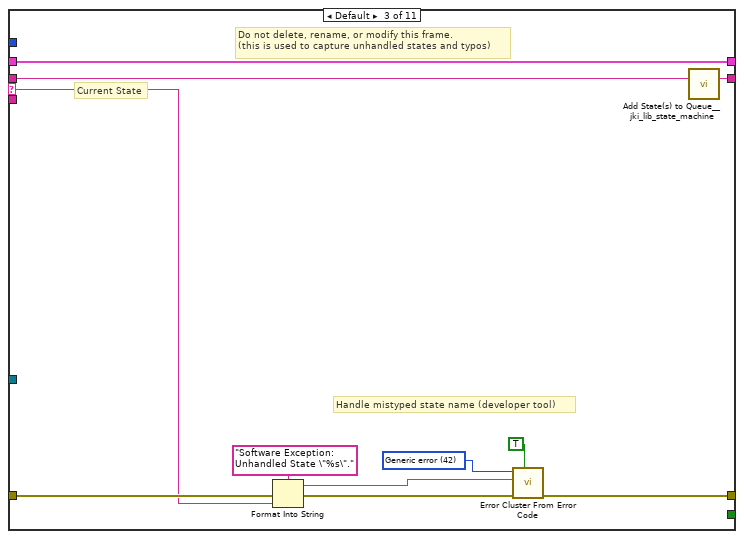
[diagram p6: hidden frame]
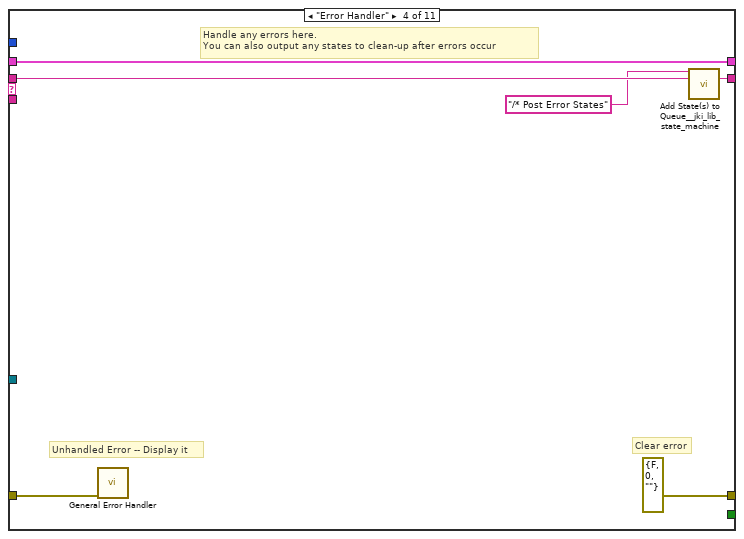
[diagram p7: hidden frame]
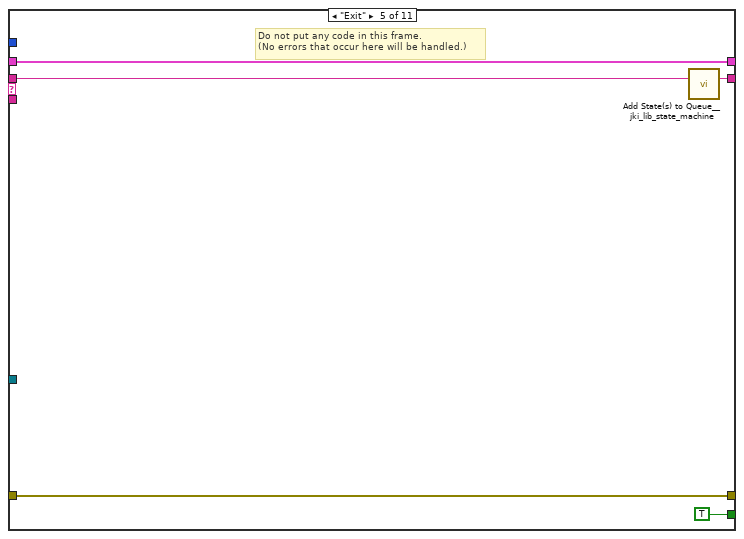
[diagram p8: hidden frame]
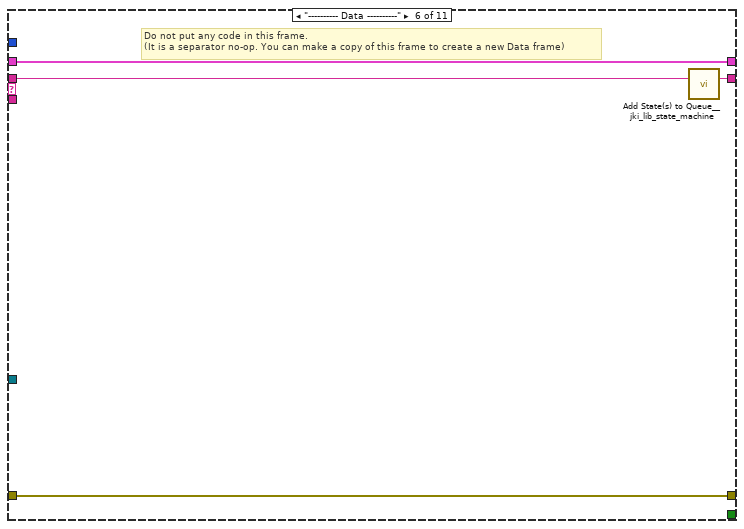
[diagram p9: hidden frame]
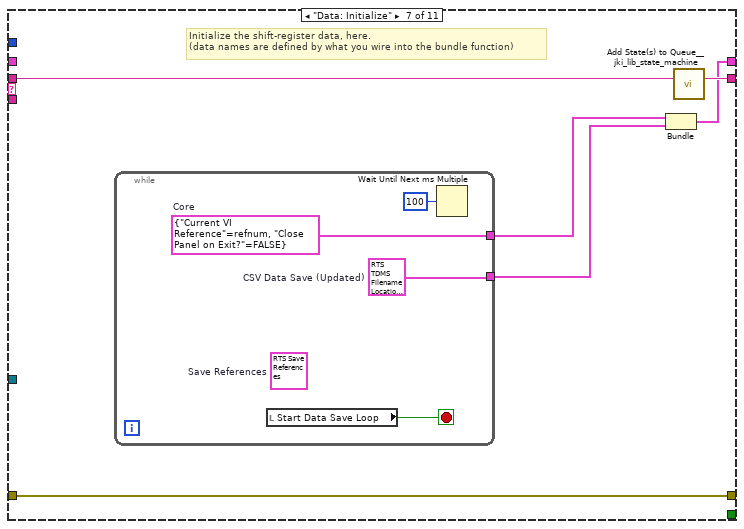
[diagram p10: hidden frame]
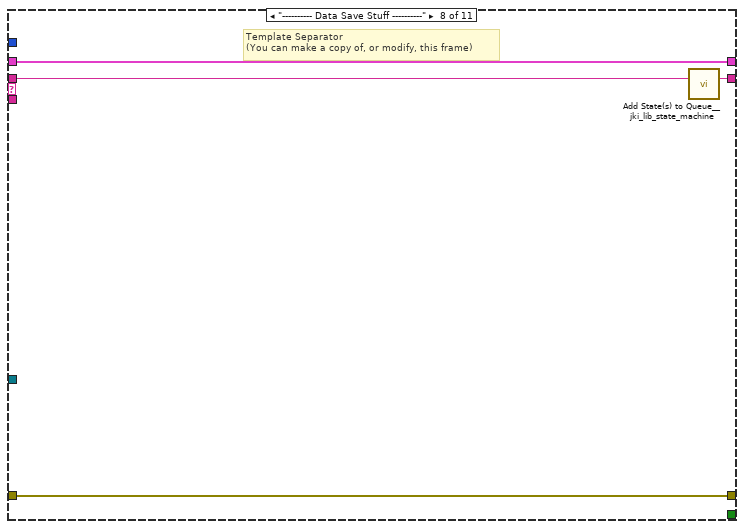
[diagram p11: hidden frame]
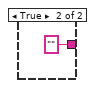
[diagram p12: hidden frame]
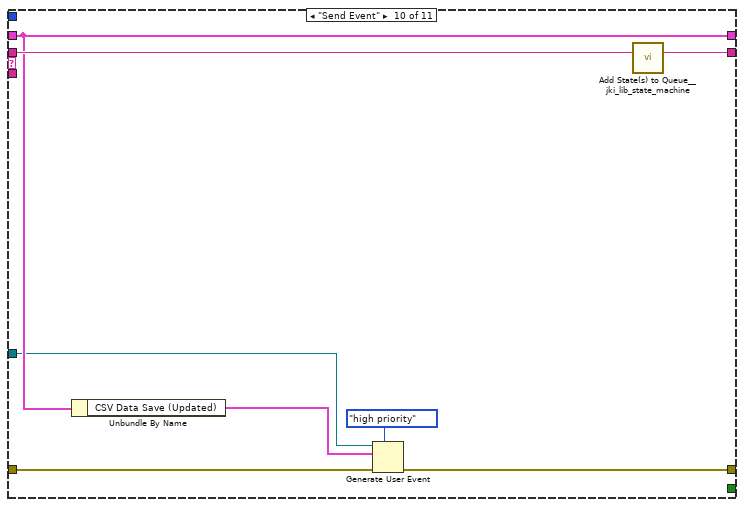
[diagram p13: hidden frame]
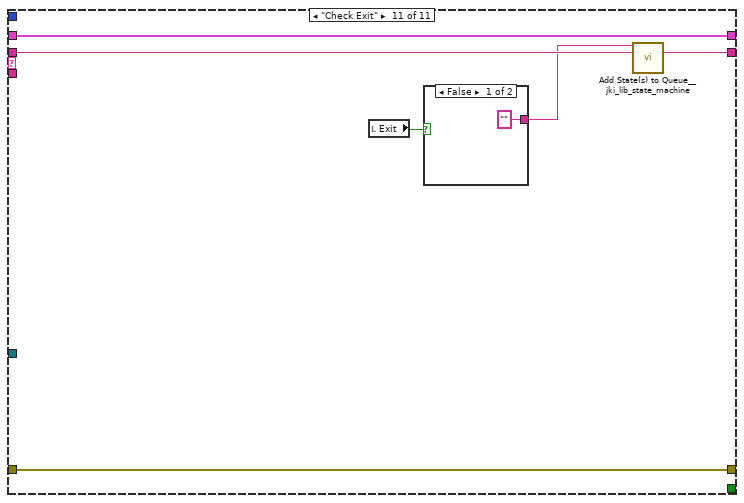
[diagram p14: hidden frame]
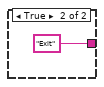
[diagram p15: hidden frame]
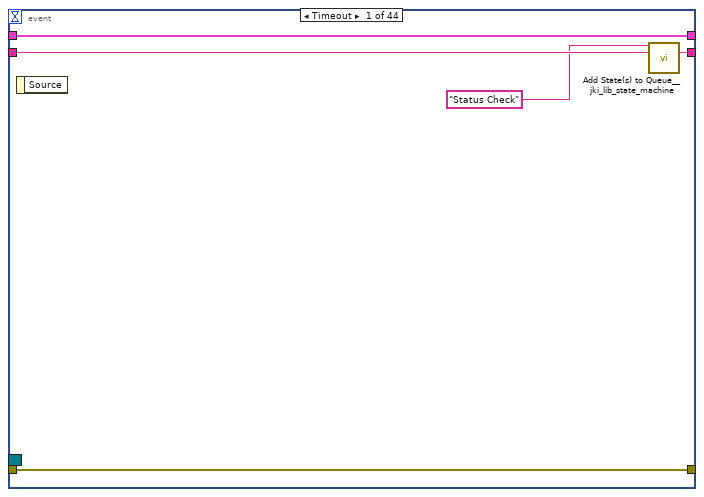
[diagram p18: hidden frame]
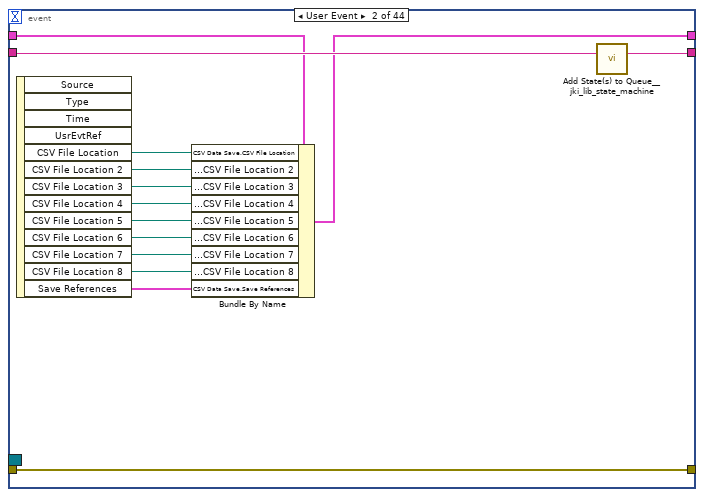
[diagram p19: hidden frame]
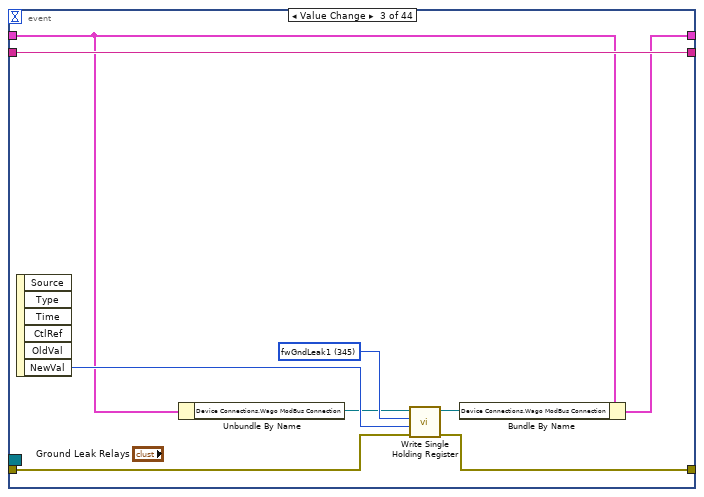
[diagram p20: hidden frame]
diagram:
  w1 = T2 {"CSV File Location"=path "", "CSV File Location 2"=path "", "CSV File Location 3"=path "", "CSV File Location 4"=path "", "CSV File Location 5"=path "", "CSV File Location 6"=path "", "CSV File Location 7"=path "", "CSV File Location 8"=path "", "Save References"={"CSV 1"=refnum, "CSV 2"=refnum, "CSV 3"=refnum, "CSV 4"=refnum, "CSV 5"=refnum, "CSV 6"=refnum, "CSV 7"=refnum, "CSV 8"=refnum}}  # Update Save Path
  # "This software grabs all data and posts to a specific TCP port"
  n1 = flat-sequence {
    tunnel: "Error In" -> [w17]
    tunnel: [w17] -> w6
    tunnel: ["Macro: Initialize\nOpen Wago Connection\nOpen APLUS Connection\nOpen MX Connection\nStart Data Save Loop\nRead Door Setup"] -> w12
    frame #0 {
      w15 = FALSE ("Exit")
      n2 = local write "Exit"(w15) -> ()
      n3 = local write "Start Data Save Loop"(w15) -> ()
    }
  }
  n4 = Create User Event(user event datatype=w1, error in=w6) -> (user event=w3:refnum<user-event>, error out=w5:errorcluster)
  n5 = call <vilib>:"Add State(s) to Queue__jki_lib_state_machine.vi"("State(s) in (\"\")"=w12) -> ("States Out"=w14:string)  [unwired: 14 in]
  n6 = register-events(error in=w5, w3) -> (reference out=w2:refnum<event-registration>, error out=w4:errorcluster)  [unwired: 1 in]
  n7 = while "RTS Combination Server" {
    shift-right: [w31] -> _
    shift-left: _ -> [w30]
    shift-right: [w34] -> w10
    shift-left: w4 -> [w19]
    shift-right: [w33] -> _
    shift-left: w14 -> [w35]
    shift-right: [w28] -> _
    shift-left: string[] [] -> [w29]
    shift-right: [w22] -> _
    shift-left: _ -> [w21]
    tunnel: w2 -> [w18]
    stop <- w32 stop-if-true
    # "RTS Combination Server (Main Loop)"
    n8 = call <vilib>:"Parse State Queue__jki_lib_state_machine.vi"("State Queue"=w35, "Error In (no error)"=w19) -> ("Remaining States"=w37:string, "Current State"=w26:string, "Arguments"=w36:string)  [unwired: 11 in]
    n9 = Equal?(x=w26, y="") -> (x = y?=w27:bool)
    n10 = case shown="True" w27 {
      tunnel: [w38 w39] -> w22
      tunnel: w21 -> [w38 _]
      frame False {
      }
      frame True {
        n11 = call "UTILITY JKI Loop Timer.vi"("Initialize Rate"="Initialize Rate", "K(0.3)"="K(0.3)", "Scan Rate (Seconds)"="Main Loop Rate (Seconds)") -> ("Rate"=→"Rate":dbl, "New Time"=w39:dbl)  [unwired: 7 in]
      }
    }
    n12 = Multiply(x=1000.0, y=w22) -> (x*y=w23:dbl)
    n13 = case shown="\"\", \"Event Structure\", \"Idle\"" w26 {
      selector: w26 -> [_ _ w618 _ _ _ _ _ _ _ _ _ _ _ _ _ _ _ _ _ _ _ _ _ _ _ _ _ _ _ _ _ _ _ _ _ _ _ _ _ _ _ _ _ _ _ _ _ _ _ _ _ _ _ _ _ _ _ _ _]
      tunnel: w37 -> [w55 w617 w622 w640 w646 w651 w655 w670 w676 w680 w692 w698 w709 w740 w749 w757 w772 w786 w797 w813 w828 w841 w848 w862 w881 w885 w890 w900 w904 w915 w942 w953 w964 w975 w986 w997 w1008 w1019 w1031 w1043 w1055 w1067 w1079 w1091 w1104 w1118 w1127 w1145 w1154 _ w1182 w1194 w1206 w1218 w1230 w1242 w1254 w1266 w1280 w1286]
      tunnel: w36 -> [_ _ _ _ _ _ _ _ _ _ _ w693 w703 _ _ _ _ _ _ _ _ _ _ _ _ _ _ _ _ _ _ _ _ _ _ _ _ _ _ _ _ _ _ _ _ _ _ _ _ _ _ _ _ _ _ _ _ _ _ _]
      tunnel: w30 -> [w53 w614 w620 w631 w643 w649 w652 _ w672 w677 w685 w696 w705 w736 w744 w751 w769 w782 w792 w810 w825 w839 w844 w860 w865 w882 w887 w897 w901 w909 w938 w948 w957 w969 w980 w991 w1002 w1013 w1026 w1037 w1048 w1060 w1072 w1087 w1098 w1114 w1125 w1140 w1150 w1166 w1178 w1192 w1199 w1208 w1223 w1235 w1247 w1259 w1277 w1282]
      tunnel: [w52 w615 w624 w637 errorcluster {"status"=FALSE, "code"=0, "source"=""} ("error out") w648 w653 w667 w671 w678 w688 w694 w706 w737 w745 w753 w766 w783 w793 w808 w821 w838 w845 w857 w879 w883 w888 w898 w902 w906 w939 w950 w959 w970 w981 w992 w1003 w1014 w1027 w1039 w1051 w1063 w1075 w1080 w1101 w1110 w1119 w1142 w1151 w1168 w1172 w1188 w1196 w1210 w1220 w1232 w1244 w1256 w1273 w1284] -> w34
      tunnel: w19 -> [w51 w615 w623 w637 w641 w648 w653 w667 w673 w678 w689 w695 w707 w738 w746 w755 w767 w784 w794 w809 w822 w838 w846 w858 w874 w883 w888 w898 w902 w907 w940 w951 w960 w971 w982 w993 w1004 w1015 w1028 w1040 w1052 w1064 w1076 w1081 w1102 w1116 w1120 w1143 w1152 w1169 w1180 w1189 w1197 w1211 w1221 w1233 w1245 w1257 w1274 w1284]
      tunnel: [w54 w616 w621 w639 w645 w650 w654 w669 w675 w679 w691 w697 w708 w739 w748 w756 w771 w785 w796 w812 w827 w840 w847 w861 w880 w884 w889 w899 w903 w914 w941 w952 w963 w974 w985 w996 w1007 w1018 w1030 w1042 w1054 w1066 w1078 w1090 w1103 w1117 w1126 w1144 w1155 w1170 w1181 w1193 w1205 w1217 w1229 w1241 w1253 w1265 w1279 w1285] -> w33
      tunnel: [_ _ _ _ _ w647 _ _ _ _ _ _ _ _ _ _ _ _ _ _ _ _ _ _ _ _ _ _ _ _ _ _ _ _ _ _ _ _ _ _ _ _ _ _ _ _ _ _ _ _ _ _ _ _ _ _ _ _ _ _] -> w32
      tunnel: [w50 w614 w620 w638 w643 w649 w652 w668 w672 w677 w687 w696 w705 w735 w747 w754 w770 w782 w795 w810 w826 w839 w844 w859 w864 w882 w887 w897 w901 w908 w937 w947 w958 w968 w979 w990 w1001 w1012 w1025 w1036 w1047 w1059 w1071 w1086 w1097 w1113 w1124 w1139 w1149 w1167 w1179 w1191 w1198 w1209 w1222 w1234 w1246 w1258 w1276 w1282] -> w31
      tunnel: w23 -> [w49 _ _ _ _ _ _ _ _ _ _ _ _ _ _ _ _ _ _ _ _ _ _ _ _ _ _ _ _ _ _ _ _ _ _ _ _ _ _ _ _ _ _ _ _ _ _ _ _ _ _ _ _ _ _ _ _ _ _ _]
      tunnel: w18 -> [w48 _ _ _ _ _ _ _ _ _ _ _ _ _ _ _ _ _ _ _ _ _ _ _ _ _ _ _ _ _ _ _ _ _ _ _ _ _ _ _ _ _ _ _ _ _ _ _ _ _ _ _ _ _ _ _ _ _ _ _]
      frame "", "Event Structure", "Idle" {
        n14 = event shown="[41] \"Room Run\": Value Change" {
          selector: w48 -> [_ _ _ _ _ _ _ _ _ _ _ _ _ _ _ _ _ _ _ _ _ _ _ _ _ _ _ _ _ _ _ _ _ _ _ _ _ _ _ _ _ _ _ _]
          dyn-events: _ -> [_ _ _ _ _ _ _ _ _ _ _ _ _ _ _ _ _ _ _ _ _ _ _ _ _ _ _ _ _ _ _ _ _ _ _ _ _ _ _ _ _ _ _ _]
          timeout: w49 -> [_ _ _ _ _ _ _ _ _ _ _ _ _ _ _ _ _ _ _ _ _ _ _ _ _ _ _ _ _ _ _ _ _ _ _ _ _ _ _ _ _ _ _ _]
          tunnel: w55 -> [w60 w73 w83 w90 w101 w110 w117 w128 w137 w146 w155 w164 w171 w181 w189 w198 w209 w216 w226 w230 w245 w266 w287 w308 w329 w350 w371 w392 w407 w415 w425 w433 w452 w470 w488 w506 w524 w542 w560 w578 w585 w596 w606 w613]
          tunnel: [w59 w74 w83 w90 w101 w110 w117 w128 w137 w146 w155 w164 w171 w181 w189 w198 w209 w216 w226 w229 w245 w266 w287 w308 w329 w350 w371 w392 w407 w415 w425 w434 w452 w470 w488 w506 w524 w542 w560 w578 w585 w596 w607 w612] -> w54
          tunnel: w53 -> [w57 w72 w78 w86 w94 w103 w112 w121 w130 w139 w148 w158 w166 w175 w184 w194 w202 w210 w220 w228 w235 w254 w277 w297 w319 w338 w359 w381 w401 w409 w416 w430 w438 w455 w475 w491 w509 w529 w545 w563 w584 w593 w604 w610]
          tunnel: [w58 w61 w75 w84 w95 w106 w116 w123 w134 w141 w151 w156 w168 w179 w188 w197 w205 w214 w222 w231 w240 w261 w285 w306 w327 w348 w369 w390 w403 w413 w420 w426 w435 w458 w472 w494 w512 w530 w543 w561 w579 w590 w605 w611] -> w52
          tunnel: w51 -> [w58 w61 w80 w88 w97 w107 w115 w124 w132 w142 w152 w160 w170 w178 w187 w196 w206 w215 w224 w231 w239 w260 w280 w302 w322 w344 w365 w385 w404 w412 w422 w427 w439 w459 w476 w495 w513 w531 w548 w565 w580 w591 w605 w611]
          tunnel: [w57 w71 w77 w85 w93 w102 w111 w120 w129 w138 w147 w157 w165 w174 w183 w193 w201 w211 w219 w228 w234 w253 w276 w296 w318 w337 w358 w380 w400 w408 w418 w429 w437 w454 w474 w490 w508 w528 w544 w562 w583 w592 w603 w610] -> w50
          event Timeout {
            n15 = event-data() -> ()  [unwired: 1 in, 1 out]
            n16 = call <vilib>:"Add State(s) to Queue__jki_lib_state_machine.vi"("State(s) in Front (\"\")"="Status Check" ("State(s) in Front (\"\")"), "State(s) in (\"\")"=w60) -> ("States Out"=w59:string)  [unwired: 13 in]
          }
          event User Event {
            n17 = event-data() -> ("CSV File Location"=w70:path, "CSV File Location 2"=w69:path, "CSV File Location 3"=w68:path, "CSV File Location 4"=w67:path, "CSV File Location 5"=w66:path, "CSV File Location 6"=w65:path, "CSV File Location 7"=w64:path, "CSV File Location 8"=w63:path, "Save References"=w62:T3)  [unwired: 1 in, 4 out]
            n18 = Bundle By Name(cluster=w72, "CSV Data Save.CSV File Location"=w70, "CSV Data Save.CSV File Location 2"=w69, "CSV Data Save.CSV File Location 3"=w68, "CSV Data Save.CSV File Location 4"=w67, "CSV Data Save.CSV File Location 5"=w66, "CSV Data Save.CSV File Location 6"=w65, "CSV Data Save.CSV File Location 7"=w64, "CSV Data Save.CSV File Location 8"=w63, "CSV Data Save.Save References"=w62) -> (w71:T55)
            n19 = call <vilib>:"Add State(s) to Queue__jki_lib_state_machine.vi"("State(s) in (\"\")"=w73) -> ("States Out"=w74:string)  [unwired: 14 in]
          }
          event Value Change {
            w82 = T56 345 items=["fwS1Volt1"=0, "fwS1Volt2"=1, "fwS2Volt1"=2, "fwS2Volt2"=3, "fwS3Volt1"=4, "fwS3Volt2"=5, "fwS4Volt1"=6, "fwS4Volt2"=7, "fwS5Volt1"=8, "fwS5Volt2"=9, "fwS6Volt1"=10, "fwS6Volt2 "=11, "fwS7Volt1"=12, "fwS7Volt2"=13, "fwS8Volt1"=14, "fwS8Volt2"=15, "fwRoomHum"=16, "fwRoomTemp"=17, "fwAISpare1"=18, "fwAISpare2"=19, "fwSuppTemp"=20, "fwCoolTemp"=21, "fwDehumTemp"=22, "fwUnused"=23, "Bool Inputs"=24, "gwVoltRate1"=256, "gwVoltRate2"=257, "gwVoltRate3"=258, "gwVoltRate4"=259, "gwVoltRate5"=260, "gwVoltRate6"=261, "gwVoltRate7"=262, "gwVoltRate8"=263, "gwVoltWindow5/1"=264, "gwVoltWindow6/2"=265, "gwVoltWindow7/3"=266, "gwVoltWindow8/4"=267, "fwVoltSet1"=272, "fwVoltSet2"=273, "fwVoltSet3"=274, "fwVoltSet4"=275, "fwVoltSet5"=276, "fwVoltSet6"=277, "fwVoltSet7"=278, "fwVoltSet8"=279, "fwVoltRng1"=280, "fwVoltRng2"=281, "fwVoltRng3"=282, "fwVoltRng4"=283, "fwVoltRng5"=284, "fwVoltRng6"=285, "fwVoltRng7"=286, "fwVoltRng8"=287, "fwVoltPol1"=296, "fwVoltPol2"=297, "fwVoltPol3"=298, "fwVoltPol4"=299, "fwVoltPol5"=300, "fwVoltPol6"=301, "fwVoltPol7"=302, "fwVoltPol8"=303, "Rm1St1Dr1Cmd"=304, "Rm1St2Dr1Cmd"=305, "Rm1St3Dr1Cmd"=306, "Rm1St4Dr1Cmd"=307, "Rm1St5Dr1Cmd"=308, "Rm1St6Dr1Cmd"=309, "Rm1St7Dr1Cmd"=310, "Rm1St8Dr1Cmd"=311, "Rm1St1Dr2Cmd"=312, "Rm1St2Dr2Cmd"=313, "Rm1St3Dr2Cmd"=314, "Rm1St4Dr2Cmd"=315, "Rm1St5Dr2Cmd"=316, "Rm1St6Dr2Cmd"=317, "Rm1St7Dr2Cmd"=318, "Rm1St8Dr2Cmd"=319, "Rm1St1Dr3Cmd"=320, "Rm1St2Dr3Cmd"=321, "Rm1St3Dr3Cmd"=322, "Rm1St4Dr3Cmd"=323, "Rm1St5Dr3Cmd"=324, "Rm1St6Dr3Cmd"=325, "Rm1St7Dr3Cmd"=326, "Rm1St8Dr3Cmd"=327, "fwRmTempSP"=328, "fwRmHumSP"=329, "fwCoolTempSP"=330, "fwDehumTempSP"=331, "fwRmRun"=332, "fwRmOk"=333, "fwTesting"=334, "fwRmDryP"=335, "fwRmDryI"=336, "fwRmHumP"=337, "fwRmHumI"=338, "fwRmHeatP"=339, "fwRmHeatI"=340, "fwCoolTempP"=341, "fwCoolTempI"=342, "fwDehumTempP"=343, "fwDehumTempI"=344, "fwGndLeak1"=345, "fwGndLeak2"=346, "fwGndLeak3"=347, "fwGndLeak4"=348, "fwGndLeak5"=349, "fwGndLeak6"=350, "fwGndLeak7"=351, "fwGndLeak8"=352, "Rm1OpenerCmd"=353] ("Ring")
            n20 = event-data() -> ("NewVal"=w81:T27)  [unwired: 1 in, 5 out]
            n21 = Unbundle By Name(w78) -> ("Device Connections.Wago ModBus Connection"=w79:refnum<class "Modbus Master.lvclass">)
            n22 = call-dynamic "Write Single Holding Register.vi"("error in"=w80, "register to write"=w81, "address"=w82, "Modbus master in"=w79) -> ("error out"=w75:errorcluster, "Modbus master out"=w76:refnum<class "Modbus Master.lvclass">)  [unwired: 6 in]
            n23 = Bundle By Name(cluster=w78, "Device Connections.Wago ModBus Connection"=w76) -> (w77:T55)
          }
          event Value Change {
            w92 = T56 346 items=["fwS1Volt1"=0, "fwS1Volt2"=1, "fwS2Volt1"=2, "fwS2Volt2"=3, "fwS3Volt1"=4, "fwS3Volt2"=5, "fwS4Volt1"=6, "fwS4Volt2"=7, "fwS5Volt1"=8, "fwS5Volt2"=9, "fwS6Volt1"=10, "fwS6Volt2 "=11, "fwS7Volt1"=12, "fwS7Volt2"=13, "fwS8Volt1"=14, "fwS8Volt2"=15, "fwRoomHum"=16, "fwRoomTemp"=17, "fwAISpare1"=18, "fwAISpare2"=19, "fwSuppTemp"=20, "fwCoolTemp"=21, "fwDehumTemp"=22, "fwUnused"=23, "Bool Inputs"=24, "gwVoltRate1"=256, "gwVoltRate2"=257, "gwVoltRate3"=258, "gwVoltRate4"=259, "gwVoltRate5"=260, "gwVoltRate6"=261, "gwVoltRate7"=262, "gwVoltRate8"=263, "gwVoltWindow5/1"=264, "gwVoltWindow6/2"=265, "gwVoltWindow7/3"=266, "gwVoltWindow8/4"=267, "fwVoltSet1"=272, "fwVoltSet2"=273, "fwVoltSet3"=274, "fwVoltSet4"=275, "fwVoltSet5"=276, "fwVoltSet6"=277, "fwVoltSet7"=278, "fwVoltSet8"=279, "fwVoltRng1"=280, "fwVoltRng2"=281, "fwVoltRng3"=282, "fwVoltRng4"=283, "fwVoltRng5"=284, "fwVoltRng6"=285, "fwVoltRng7"=286, "fwVoltRng8"=287, "fwVoltPol1"=296, "fwVoltPol2"=297, "fwVoltPol3"=298, "fwVoltPol4"=299, "fwVoltPol5"=300, "fwVoltPol6"=301, "fwVoltPol7"=302, "fwVoltPol8"=303, "Rm1St1Dr1Cmd"=304, "Rm1St2Dr1Cmd"=305, "Rm1St3Dr1Cmd"=306, "Rm1St4Dr1Cmd"=307, "Rm1St5Dr1Cmd"=308, "Rm1St6Dr1Cmd"=309, "Rm1St7Dr1Cmd"=310, "Rm1St8Dr1Cmd"=311, "Rm1St1Dr2Cmd"=312, "Rm1St2Dr2Cmd"=313, "Rm1St3Dr2Cmd"=314, "Rm1St4Dr2Cmd"=315, "Rm1St5Dr2Cmd"=316, "Rm1St6Dr2Cmd"=317, "Rm1St7Dr2Cmd"=318, "Rm1St8Dr2Cmd"=319, "Rm1St1Dr3Cmd"=320, "Rm1St2Dr3Cmd"=321, "Rm1St3Dr3Cmd"=322, "Rm1St4Dr3Cmd"=323, "Rm1St5Dr3Cmd"=324, "Rm1St6Dr3Cmd"=325, "Rm1St7Dr3Cmd"=326, "Rm1St8Dr3Cmd"=327, "fwRmTempSP"=328, "fwRmHumSP"=329, "fwCoolTempSP"=330, "fwDehumTempSP"=331, "fwRmRun"=332, "fwRmOk"=333, "fwTesting"=334, "fwRmDryP"=335, "fwRmDryI"=336, "fwRmHumP"=337, "fwRmHumI"=338, "fwRmHeatP"=339, "fwRmHeatI"=340, "fwCoolTempP"=341, "fwCoolTempI"=342, "fwDehumTempP"=343, "fwDehumTempI"=344, "fwGndLeak1"=345, "fwGndLeak2"=346, "fwGndLeak3"=347, "fwGndLeak4"=348, "fwGndLeak5"=349, "fwGndLeak6"=350, "fwGndLeak7"=351, "fwGndLeak8"=352, "Rm1OpenerCmd"=353] ("Ring")
            n24 = event-data() -> ("NewVal"=w91:T27)  [unwired: 1 in, 5 out]
            n25 = Unbundle By Name(w86) -> ("Device Connections.Wago ModBus Connection"=w89:refnum<class "Modbus Master.lvclass">)
            n26 = call-dynamic "Write Single Holding Register.vi"("error in"=w88, "register to write"=w91, "address"=w92, "Modbus master in"=w89) -> ("error out"=w84:errorcluster, "Modbus master out"=w87:refnum<class "Modbus Master.lvclass">)  [unwired: 6 in]
            n27 = Bundle By Name(cluster=w86, "Device Connections.Wago ModBus Connection"=w87) -> (w85:T55)
          }
          event Value Change {
            w100 = T56 347 items=["fwS1Volt1"=0, "fwS1Volt2"=1, "fwS2Volt1"=2, "fwS2Volt2"=3, "fwS3Volt1"=4, "fwS3Volt2"=5, "fwS4Volt1"=6, "fwS4Volt2"=7, "fwS5Volt1"=8, "fwS5Volt2"=9, "fwS6Volt1"=10, "fwS6Volt2 "=11, "fwS7Volt1"=12, "fwS7Volt2"=13, "fwS8Volt1"=14, "fwS8Volt2"=15, "fwRoomHum"=16, "fwRoomTemp"=17, "fwAISpare1"=18, "fwAISpare2"=19, "fwSuppTemp"=20, "fwCoolTemp"=21, "fwDehumTemp"=22, "fwUnused"=23, "Bool Inputs"=24, "gwVoltRate1"=256, "gwVoltRate2"=257, "gwVoltRate3"=258, "gwVoltRate4"=259, "gwVoltRate5"=260, "gwVoltRate6"=261, "gwVoltRate7"=262, "gwVoltRate8"=263, "gwVoltWindow5/1"=264, "gwVoltWindow6/2"=265, "gwVoltWindow7/3"=266, "gwVoltWindow8/4"=267, "fwVoltSet1"=272, "fwVoltSet2"=273, "fwVoltSet3"=274, "fwVoltSet4"=275, "fwVoltSet5"=276, "fwVoltSet6"=277, "fwVoltSet7"=278, "fwVoltSet8"=279, "fwVoltRng1"=280, "fwVoltRng2"=281, "fwVoltRng3"=282, "fwVoltRng4"=283, "fwVoltRng5"=284, "fwVoltRng6"=285, "fwVoltRng7"=286, "fwVoltRng8"=287, "fwVoltPol1"=296, "fwVoltPol2"=297, "fwVoltPol3"=298, "fwVoltPol4"=299, "fwVoltPol5"=300, "fwVoltPol6"=301, "fwVoltPol7"=302, "fwVoltPol8"=303, "Rm1St1Dr1Cmd"=304, "Rm1St2Dr1Cmd"=305, "Rm1St3Dr1Cmd"=306, "Rm1St4Dr1Cmd"=307, "Rm1St5Dr1Cmd"=308, "Rm1St6Dr1Cmd"=309, "Rm1St7Dr1Cmd"=310, "Rm1St8Dr1Cmd"=311, "Rm1St1Dr2Cmd"=312, "Rm1St2Dr2Cmd"=313, "Rm1St3Dr2Cmd"=314, "Rm1St4Dr2Cmd"=315, "Rm1St5Dr2Cmd"=316, "Rm1St6Dr2Cmd"=317, "Rm1St7Dr2Cmd"=318, "Rm1St8Dr2Cmd"=319, "Rm1St1Dr3Cmd"=320, "Rm1St2Dr3Cmd"=321, "Rm1St3Dr3Cmd"=322, "Rm1St4Dr3Cmd"=323, "Rm1St5Dr3Cmd"=324, "Rm1St6Dr3Cmd"=325, "Rm1St7Dr3Cmd"=326, "Rm1St8Dr3Cmd"=327, "fwRmTempSP"=328, "fwRmHumSP"=329, "fwCoolTempSP"=330, "fwDehumTempSP"=331, "fwRmRun"=332, "fwRmOk"=333, "fwTesting"=334, "fwRmDryP"=335, "fwRmDryI"=336, "fwRmHumP"=337, "fwRmHumI"=338, "fwRmHeatP"=339, "fwRmHeatI"=340, "fwCoolTempP"=341, "fwCoolTempI"=342, "fwDehumTempP"=343, "fwDehumTempI"=344, "fwGndLeak1"=345, "fwGndLeak2"=346, "fwGndLeak3"=347, "fwGndLeak4"=348, "fwGndLeak5"=349, "fwGndLeak6"=350, "fwGndLeak7"=351, "fwGndLeak8"=352, "Rm1OpenerCmd"=353] ("Ring")
            n28 = event-data() -> ("NewVal"=w99:T27)  [unwired: 1 in, 5 out]
            n29 = Unbundle By Name(w94) -> ("Device Connections.Wago ModBus Connection"=w98:refnum<class "Modbus Master.lvclass">)
            n30 = call-dynamic "Write Single Holding Register.vi"("error in"=w97, "register to write"=w99, "address"=w100, "Modbus master in"=w98) -> ("error out"=w95:errorcluster, "Modbus master out"=w96:refnum<class "Modbus Master.lvclass">)  [unwired: 6 in]
            n31 = Bundle By Name(cluster=w94, "Device Connections.Wago ModBus Connection"=w96) -> (w93:T55)
          }
          event Value Change {
            w108 = T56 348 items=["fwS1Volt1"=0, "fwS1Volt2"=1, "fwS2Volt1"=2, "fwS2Volt2"=3, "fwS3Volt1"=4, "fwS3Volt2"=5, "fwS4Volt1"=6, "fwS4Volt2"=7, "fwS5Volt1"=8, "fwS5Volt2"=9, "fwS6Volt1"=10, "fwS6Volt2 "=11, "fwS7Volt1"=12, "fwS7Volt2"=13, "fwS8Volt1"=14, "fwS8Volt2"=15, "fwRoomHum"=16, "fwRoomTemp"=17, "fwAISpare1"=18, "fwAISpare2"=19, "fwSuppTemp"=20, "fwCoolTemp"=21, "fwDehumTemp"=22, "fwUnused"=23, "Bool Inputs"=24, "gwVoltRate1"=256, "gwVoltRate2"=257, "gwVoltRate3"=258, "gwVoltRate4"=259, "gwVoltRate5"=260, "gwVoltRate6"=261, "gwVoltRate7"=262, "gwVoltRate8"=263, "gwVoltWindow5/1"=264, "gwVoltWindow6/2"=265, "gwVoltWindow7/3"=266, "gwVoltWindow8/4"=267, "fwVoltSet1"=272, "fwVoltSet2"=273, "fwVoltSet3"=274, "fwVoltSet4"=275, "fwVoltSet5"=276, "fwVoltSet6"=277, "fwVoltSet7"=278, "fwVoltSet8"=279, "fwVoltRng1"=280, "fwVoltRng2"=281, "fwVoltRng3"=282, "fwVoltRng4"=283, "fwVoltRng5"=284, "fwVoltRng6"=285, "fwVoltRng7"=286, "fwVoltRng8"=287, "fwVoltPol1"=296, "fwVoltPol2"=297, "fwVoltPol3"=298, "fwVoltPol4"=299, "fwVoltPol5"=300, "fwVoltPol6"=301, "fwVoltPol7"=302, "fwVoltPol8"=303, "Rm1St1Dr1Cmd"=304, "Rm1St2Dr1Cmd"=305, "Rm1St3Dr1Cmd"=306, "Rm1St4Dr1Cmd"=307, "Rm1St5Dr1Cmd"=308, "Rm1St6Dr1Cmd"=309, "Rm1St7Dr1Cmd"=310, "Rm1St8Dr1Cmd"=311, "Rm1St1Dr2Cmd"=312, "Rm1St2Dr2Cmd"=313, "Rm1St3Dr2Cmd"=314, "Rm1St4Dr2Cmd"=315, "Rm1St5Dr2Cmd"=316, "Rm1St6Dr2Cmd"=317, "Rm1St7Dr2Cmd"=318, "Rm1St8Dr2Cmd"=319, "Rm1St1Dr3Cmd"=320, "Rm1St2Dr3Cmd"=321, "Rm1St3Dr3Cmd"=322, "Rm1St4Dr3Cmd"=323, "Rm1St5Dr3Cmd"=324, "Rm1St6Dr3Cmd"=325, "Rm1St7Dr3Cmd"=326, "Rm1St8Dr3Cmd"=327, "fwRmTempSP"=328, "fwRmHumSP"=329, "fwCoolTempSP"=330, "fwDehumTempSP"=331, "fwRmRun"=332, "fwRmOk"=333, "fwTesting"=334, "fwRmDryP"=335, "fwRmDryI"=336, "fwRmHumP"=337, "fwRmHumI"=338, "fwRmHeatP"=339, "fwRmHeatI"=340, "fwCoolTempP"=341, "fwCoolTempI"=342, "fwDehumTempP"=343, "fwDehumTempI"=344, "fwGndLeak1"=345, "fwGndLeak2"=346, "fwGndLeak3"=347, "fwGndLeak4"=348, "fwGndLeak5"=349, "fwGndLeak6"=350, "fwGndLeak7"=351, "fwGndLeak8"=352, "Rm1OpenerCmd"=353] ("Ring")
            # "Disconnect from the slave\nand display errors"
            n32 = event-data() -> ("NewVal"=w109:T27)  [unwired: 1 in, 5 out]
            n33 = Unbundle By Name(w103) -> ("Device Connections.Wago ModBus Connection"=w105:refnum<class "Modbus Master.lvclass">)
            n34 = call-dynamic "Write Single Holding Register.vi"("error in"=w107, "register to write"=w109, "address"=w108, "Modbus master in"=w105) -> ("error out"=w106:errorcluster, "Modbus master out"=w104:refnum<class "Modbus Master.lvclass">)  [unwired: 6 in]
            n35 = Bundle By Name(cluster=w103, "Device Connections.Wago ModBus Connection"=w104) -> (w102:T55)
          }
          event Value Change {
            w119 = T56 349 items=["fwS1Volt1"=0, "fwS1Volt2"=1, "fwS2Volt1"=2, "fwS2Volt2"=3, "fwS3Volt1"=4, "fwS3Volt2"=5, "fwS4Volt1"=6, "fwS4Volt2"=7, "fwS5Volt1"=8, "fwS5Volt2"=9, "fwS6Volt1"=10, "fwS6Volt2 "=11, "fwS7Volt1"=12, "fwS7Volt2"=13, "fwS8Volt1"=14, "fwS8Volt2"=15, "fwRoomHum"=16, "fwRoomTemp"=17, "fwAISpare1"=18, "fwAISpare2"=19, "fwSuppTemp"=20, "fwCoolTemp"=21, "fwDehumTemp"=22, "fwUnused"=23, "Bool Inputs"=24, "gwVoltRate1"=256, "gwVoltRate2"=257, "gwVoltRate3"=258, "gwVoltRate4"=259, "gwVoltRate5"=260, "gwVoltRate6"=261, "gwVoltRate7"=262, "gwVoltRate8"=263, "gwVoltWindow5/1"=264, "gwVoltWindow6/2"=265, "gwVoltWindow7/3"=266, "gwVoltWindow8/4"=267, "fwVoltSet1"=272, "fwVoltSet2"=273, "fwVoltSet3"=274, "fwVoltSet4"=275, "fwVoltSet5"=276, "fwVoltSet6"=277, "fwVoltSet7"=278, "fwVoltSet8"=279, "fwVoltRng1"=280, "fwVoltRng2"=281, "fwVoltRng3"=282, "fwVoltRng4"=283, "fwVoltRng5"=284, "fwVoltRng6"=285, "fwVoltRng7"=286, "fwVoltRng8"=287, "fwVoltPol1"=296, "fwVoltPol2"=297, "fwVoltPol3"=298, "fwVoltPol4"=299, "fwVoltPol5"=300, "fwVoltPol6"=301, "fwVoltPol7"=302, "fwVoltPol8"=303, "Rm1St1Dr1Cmd"=304, "Rm1St2Dr1Cmd"=305, "Rm1St3Dr1Cmd"=306, "Rm1St4Dr1Cmd"=307, "Rm1St5Dr1Cmd"=308, "Rm1St6Dr1Cmd"=309, "Rm1St7Dr1Cmd"=310, "Rm1St8Dr1Cmd"=311, "Rm1St1Dr2Cmd"=312, "Rm1St2Dr2Cmd"=313, "Rm1St3Dr2Cmd"=314, "Rm1St4Dr2Cmd"=315, "Rm1St5Dr2Cmd"=316, "Rm1St6Dr2Cmd"=317, "Rm1St7Dr2Cmd"=318, "Rm1St8Dr2Cmd"=319, "Rm1St1Dr3Cmd"=320, "Rm1St2Dr3Cmd"=321, "Rm1St3Dr3Cmd"=322, "Rm1St4Dr3Cmd"=323, "Rm1St5Dr3Cmd"=324, "Rm1St6Dr3Cmd"=325, "Rm1St7Dr3Cmd"=326, "Rm1St8Dr3Cmd"=327, "fwRmTempSP"=328, "fwRmHumSP"=329, "fwCoolTempSP"=330, "fwDehumTempSP"=331, "fwRmRun"=332, "fwRmOk"=333, "fwTesting"=334, "fwRmDryP"=335, "fwRmDryI"=336, "fwRmHumP"=337, "fwRmHumI"=338, "fwRmHeatP"=339, "fwRmHeatI"=340, "fwCoolTempP"=341, "fwCoolTempI"=342, "fwDehumTempP"=343, "fwDehumTempI"=344, "fwGndLeak1"=345, "fwGndLeak2"=346, "fwGndLeak3"=347, "fwGndLeak4"=348, "fwGndLeak5"=349, "fwGndLeak6"=350, "fwGndLeak7"=351, "fwGndLeak8"=352, "Rm1OpenerCmd"=353] ("Ring")
            n36 = event-data() -> ("NewVal"=w118:T27)  [unwired: 1 in, 5 out]
            n37 = Unbundle By Name(w112) -> ("Device Connections.Wago ModBus Connection"=w114:refnum<class "Modbus Master.lvclass">)
            n38 = call-dynamic "Write Single Holding Register.vi"("error in"=w115, "register to write"=w118, "address"=w119, "Modbus master in"=w114) -> ("error out"=w116:errorcluster, "Modbus master out"=w113:refnum<class "Modbus Master.lvclass">)  [unwired: 6 in]
            n39 = Bundle By Name(cluster=w112, "Device Connections.Wago ModBus Connection"=w113) -> (w111:T55)
          }
          event Value Change {
            w127 = T56 350 items=["fwS1Volt1"=0, "fwS1Volt2"=1, "fwS2Volt1"=2, "fwS2Volt2"=3, "fwS3Volt1"=4, "fwS3Volt2"=5, "fwS4Volt1"=6, "fwS4Volt2"=7, "fwS5Volt1"=8, "fwS5Volt2"=9, "fwS6Volt1"=10, "fwS6Volt2 "=11, "fwS7Volt1"=12, "fwS7Volt2"=13, "fwS8Volt1"=14, "fwS8Volt2"=15, "fwRoomHum"=16, "fwRoomTemp"=17, "fwAISpare1"=18, "fwAISpare2"=19, "fwSuppTemp"=20, "fwCoolTemp"=21, "fwDehumTemp"=22, "fwUnused"=23, "Bool Inputs"=24, "gwVoltRate1"=256, "gwVoltRate2"=257, "gwVoltRate3"=258, "gwVoltRate4"=259, "gwVoltRate5"=260, "gwVoltRate6"=261, "gwVoltRate7"=262, "gwVoltRate8"=263, "gwVoltWindow5/1"=264, "gwVoltWindow6/2"=265, "gwVoltWindow7/3"=266, "gwVoltWindow8/4"=267, "fwVoltSet1"=272, "fwVoltSet2"=273, "fwVoltSet3"=274, "fwVoltSet4"=275, "fwVoltSet5"=276, "fwVoltSet6"=277, "fwVoltSet7"=278, "fwVoltSet8"=279, "fwVoltRng1"=280, "fwVoltRng2"=281, "fwVoltRng3"=282, "fwVoltRng4"=283, "fwVoltRng5"=284, "fwVoltRng6"=285, "fwVoltRng7"=286, "fwVoltRng8"=287, "fwVoltPol1"=296, "fwVoltPol2"=297, "fwVoltPol3"=298, "fwVoltPol4"=299, "fwVoltPol5"=300, "fwVoltPol6"=301, "fwVoltPol7"=302, "fwVoltPol8"=303, "Rm1St1Dr1Cmd"=304, "Rm1St2Dr1Cmd"=305, "Rm1St3Dr1Cmd"=306, "Rm1St4Dr1Cmd"=307, "Rm1St5Dr1Cmd"=308, "Rm1St6Dr1Cmd"=309, "Rm1St7Dr1Cmd"=310, "Rm1St8Dr1Cmd"=311, "Rm1St1Dr2Cmd"=312, "Rm1St2Dr2Cmd"=313, "Rm1St3Dr2Cmd"=314, "Rm1St4Dr2Cmd"=315, "Rm1St5Dr2Cmd"=316, "Rm1St6Dr2Cmd"=317, "Rm1St7Dr2Cmd"=318, "Rm1St8Dr2Cmd"=319, "Rm1St1Dr3Cmd"=320, "Rm1St2Dr3Cmd"=321, "Rm1St3Dr3Cmd"=322, "Rm1St4Dr3Cmd"=323, "Rm1St5Dr3Cmd"=324, "Rm1St6Dr3Cmd"=325, "Rm1St7Dr3Cmd"=326, "Rm1St8Dr3Cmd"=327, "fwRmTempSP"=328, "fwRmHumSP"=329, "fwCoolTempSP"=330, "fwDehumTempSP"=331, "fwRmRun"=332, "fwRmOk"=333, "fwTesting"=334, "fwRmDryP"=335, "fwRmDryI"=336, "fwRmHumP"=337, "fwRmHumI"=338, "fwRmHeatP"=339, "fwRmHeatI"=340, "fwCoolTempP"=341, "fwCoolTempI"=342, "fwDehumTempP"=343, "fwDehumTempI"=344, "fwGndLeak1"=345, "fwGndLeak2"=346, "fwGndLeak3"=347, "fwGndLeak4"=348, "fwGndLeak5"=349, "fwGndLeak6"=350, "fwGndLeak7"=351, "fwGndLeak8"=352, "Rm1OpenerCmd"=353] ("Ring")
            n40 = event-data() -> ("NewVal"=w126:T27)  [unwired: 1 in, 5 out]
            n41 = Unbundle By Name(w121) -> ("Device Connections.Wago ModBus Connection"=w125:refnum<class "Modbus Master.lvclass">)
            n42 = call-dynamic "Write Single Holding Register.vi"("error in"=w124, "register to write"=w126, "address"=w127, "Modbus master in"=w125) -> ("error out"=w123:errorcluster, "Modbus master out"=w122:refnum<class "Modbus Master.lvclass">)  [unwired: 6 in]
            n43 = Bundle By Name(cluster=w121, "Device Connections.Wago ModBus Connection"=w122) -> (w120:T55)
          }
          event Value Change {
            w136 = T56 351 items=["fwS1Volt1"=0, "fwS1Volt2"=1, "fwS2Volt1"=2, "fwS2Volt2"=3, "fwS3Volt1"=4, "fwS3Volt2"=5, "fwS4Volt1"=6, "fwS4Volt2"=7, "fwS5Volt1"=8, "fwS5Volt2"=9, "fwS6Volt1"=10, "fwS6Volt2 "=11, "fwS7Volt1"=12, "fwS7Volt2"=13, "fwS8Volt1"=14, "fwS8Volt2"=15, "fwRoomHum"=16, "fwRoomTemp"=17, "fwAISpare1"=18, "fwAISpare2"=19, "fwSuppTemp"=20, "fwCoolTemp"=21, "fwDehumTemp"=22, "fwUnused"=23, "Bool Inputs"=24, "gwVoltRate1"=256, "gwVoltRate2"=257, "gwVoltRate3"=258, "gwVoltRate4"=259, "gwVoltRate5"=260, "gwVoltRate6"=261, "gwVoltRate7"=262, "gwVoltRate8"=263, "gwVoltWindow5/1"=264, "gwVoltWindow6/2"=265, "gwVoltWindow7/3"=266, "gwVoltWindow8/4"=267, "fwVoltSet1"=272, "fwVoltSet2"=273, "fwVoltSet3"=274, "fwVoltSet4"=275, "fwVoltSet5"=276, "fwVoltSet6"=277, "fwVoltSet7"=278, "fwVoltSet8"=279, "fwVoltRng1"=280, "fwVoltRng2"=281, "fwVoltRng3"=282, "fwVoltRng4"=283, "fwVoltRng5"=284, "fwVoltRng6"=285, "fwVoltRng7"=286, "fwVoltRng8"=287, "fwVoltPol1"=296, "fwVoltPol2"=297, "fwVoltPol3"=298, "fwVoltPol4"=299, "fwVoltPol5"=300, "fwVoltPol6"=301, "fwVoltPol7"=302, "fwVoltPol8"=303, "Rm1St1Dr1Cmd"=304, "Rm1St2Dr1Cmd"=305, "Rm1St3Dr1Cmd"=306, "Rm1St4Dr1Cmd"=307, "Rm1St5Dr1Cmd"=308, "Rm1St6Dr1Cmd"=309, "Rm1St7Dr1Cmd"=310, "Rm1St8Dr1Cmd"=311, "Rm1St1Dr2Cmd"=312, "Rm1St2Dr2Cmd"=313, "Rm1St3Dr2Cmd"=314, "Rm1St4Dr2Cmd"=315, "Rm1St5Dr2Cmd"=316, "Rm1St6Dr2Cmd"=317, "Rm1St7Dr2Cmd"=318, "Rm1St8Dr2Cmd"=319, "Rm1St1Dr3Cmd"=320, "Rm1St2Dr3Cmd"=321, "Rm1St3Dr3Cmd"=322, "Rm1St4Dr3Cmd"=323, "Rm1St5Dr3Cmd"=324, "Rm1St6Dr3Cmd"=325, "Rm1St7Dr3Cmd"=326, "Rm1St8Dr3Cmd"=327, "fwRmTempSP"=328, "fwRmHumSP"=329, "fwCoolTempSP"=330, "fwDehumTempSP"=331, "fwRmRun"=332, "fwRmOk"=333, "fwTesting"=334, "fwRmDryP"=335, "fwRmDryI"=336, "fwRmHumP"=337, "fwRmHumI"=338, "fwRmHeatP"=339, "fwRmHeatI"=340, "fwCoolTempP"=341, "fwCoolTempI"=342, "fwDehumTempP"=343, "fwDehumTempI"=344, "fwGndLeak1"=345, "fwGndLeak2"=346, "fwGndLeak3"=347, "fwGndLeak4"=348, "fwGndLeak5"=349, "fwGndLeak6"=350, "fwGndLeak7"=351, "fwGndLeak8"=352, "Rm1OpenerCmd"=353] ("Ring")
            n44 = event-data() -> ("NewVal"=w135:T27)  [unwired: 1 in, 5 out]
            n45 = Unbundle By Name(w130) -> ("Device Connections.Wago ModBus Connection"=w133:refnum<class "Modbus Master.lvclass">)
            n46 = call-dynamic "Write Single Holding Register.vi"("error in"=w132, "register to write"=w135, "address"=w136, "Modbus master in"=w133) -> ("error out"=w134:errorcluster, "Modbus master out"=w131:refnum<class "Modbus Master.lvclass">)  [unwired: 6 in]
            n47 = Bundle By Name(cluster=w130, "Device Connections.Wago ModBus Connection"=w131) -> (w129:T55)
          }
          event Value Change {
            w145 = T56 352 items=["fwS1Volt1"=0, "fwS1Volt2"=1, "fwS2Volt1"=2, "fwS2Volt2"=3, "fwS3Volt1"=4, "fwS3Volt2"=5, "fwS4Volt1"=6, "fwS4Volt2"=7, "fwS5Volt1"=8, "fwS5Volt2"=9, "fwS6Volt1"=10, "fwS6Volt2 "=11, "fwS7Volt1"=12, "fwS7Volt2"=13, "fwS8Volt1"=14, "fwS8Volt2"=15, "fwRoomHum"=16, "fwRoomTemp"=17, "fwAISpare1"=18, "fwAISpare2"=19, "fwSuppTemp"=20, "fwCoolTemp"=21, "fwDehumTemp"=22, "fwUnused"=23, "Bool Inputs"=24, "gwVoltRate1"=256, "gwVoltRate2"=257, "gwVoltRate3"=258, "gwVoltRate4"=259, "gwVoltRate5"=260, "gwVoltRate6"=261, "gwVoltRate7"=262, "gwVoltRate8"=263, "gwVoltWindow5/1"=264, "gwVoltWindow6/2"=265, "gwVoltWindow7/3"=266, "gwVoltWindow8/4"=267, "fwVoltSet1"=272, "fwVoltSet2"=273, "fwVoltSet3"=274, "fwVoltSet4"=275, "fwVoltSet5"=276, "fwVoltSet6"=277, "fwVoltSet7"=278, "fwVoltSet8"=279, "fwVoltRng1"=280, "fwVoltRng2"=281, "fwVoltRng3"=282, "fwVoltRng4"=283, "fwVoltRng5"=284, "fwVoltRng6"=285, "fwVoltRng7"=286, "fwVoltRng8"=287, "fwVoltPol1"=296, "fwVoltPol2"=297, "fwVoltPol3"=298, "fwVoltPol4"=299, "fwVoltPol5"=300, "fwVoltPol6"=301, "fwVoltPol7"=302, "fwVoltPol8"=303, "Rm1St1Dr1Cmd"=304, "Rm1St2Dr1Cmd"=305, "Rm1St3Dr1Cmd"=306, "Rm1St4Dr1Cmd"=307, "Rm1St5Dr1Cmd"=308, "Rm1St6Dr1Cmd"=309, "Rm1St7Dr1Cmd"=310, "Rm1St8Dr1Cmd"=311, "Rm1St1Dr2Cmd"=312, "Rm1St2Dr2Cmd"=313, "Rm1St3Dr2Cmd"=314, "Rm1St4Dr2Cmd"=315, "Rm1St5Dr2Cmd"=316, "Rm1St6Dr2Cmd"=317, "Rm1St7Dr2Cmd"=318, "Rm1St8Dr2Cmd"=319, "Rm1St1Dr3Cmd"=320, "Rm1St2Dr3Cmd"=321, "Rm1St3Dr3Cmd"=322, "Rm1St4Dr3Cmd"=323, "Rm1St5Dr3Cmd"=324, "Rm1St6Dr3Cmd"=325, "Rm1St7Dr3Cmd"=326, "Rm1St8Dr3Cmd"=327, "fwRmTempSP"=328, "fwRmHumSP"=329, "fwCoolTempSP"=330, "fwDehumTempSP"=331, "fwRmRun"=332, "fwRmOk"=333, "fwTesting"=334, "fwRmDryP"=335, "fwRmDryI"=336, "fwRmHumP"=337, "fwRmHumI"=338, "fwRmHeatP"=339, "fwRmHeatI"=340, "fwCoolTempP"=341, "fwCoolTempI"=342, "fwDehumTempP"=343, "fwDehumTempI"=344, "fwGndLeak1"=345, "fwGndLeak2"=346, "fwGndLeak3"=347, "fwGndLeak4"=348, "fwGndLeak5"=349, "fwGndLeak6"=350, "fwGndLeak7"=351, "fwGndLeak8"=352, "Rm1OpenerCmd"=353] ("Ring")
            n48 = event-data() -> ("NewVal"=w144:T27)  [unwired: 1 in, 5 out]
            n49 = Unbundle By Name(w139) -> ("Device Connections.Wago ModBus Connection"=w143:refnum<class "Modbus Master.lvclass">)
            n50 = call-dynamic "Write Single Holding Register.vi"("error in"=w142, "register to write"=w144, "address"=w145, "Modbus master in"=w143) -> ("error out"=w141:errorcluster, "Modbus master out"=w140:refnum<class "Modbus Master.lvclass">)  [unwired: 6 in]
            n51 = Bundle By Name(cluster=w139, "Device Connections.Wago ModBus Connection"=w140) -> (w138:T55)
          }
          event Value Change {
            w153 = T56 296 items=["fwS1Volt1"=0, "fwS1Volt2"=1, "fwS2Volt1"=2, "fwS2Volt2"=3, "fwS3Volt1"=4, "fwS3Volt2"=5, "fwS4Volt1"=6, "fwS4Volt2"=7, "fwS5Volt1"=8, "fwS5Volt2"=9, "fwS6Volt1"=10, "fwS6Volt2 "=11, "fwS7Volt1"=12, "fwS7Volt2"=13, "fwS8Volt1"=14, "fwS8Volt2"=15, "fwRoomHum"=16, "fwRoomTemp"=17, "fwAISpare1"=18, "fwAISpare2"=19, "fwSuppTemp"=20, "fwCoolTemp"=21, "fwDehumTemp"=22, "fwUnused"=23, "Bool Inputs"=24, "gwVoltRate1"=256, "gwVoltRate2"=257, "gwVoltRate3"=258, "gwVoltRate4"=259, "gwVoltRate5"=260, "gwVoltRate6"=261, "gwVoltRate7"=262, "gwVoltRate8"=263, "gwVoltWindow5/1"=264, "gwVoltWindow6/2"=265, "gwVoltWindow7/3"=266, "gwVoltWindow8/4"=267, "fwVoltSet1"=272, "fwVoltSet2"=273, "fwVoltSet3"=274, "fwVoltSet4"=275, "fwVoltSet5"=276, "fwVoltSet6"=277, "fwVoltSet7"=278, "fwVoltSet8"=279, "fwVoltRng1"=280, "fwVoltRng2"=281, "fwVoltRng3"=282, "fwVoltRng4"=283, "fwVoltRng5"=284, "fwVoltRng6"=285, "fwVoltRng7"=286, "fwVoltRng8"=287, "fwVoltPol1"=296, "fwVoltPol2"=297, "fwVoltPol3"=298, "fwVoltPol4"=299, "fwVoltPol5"=300, "fwVoltPol6"=301, "fwVoltPol7"=302, "fwVoltPol8"=303, "Rm1St1Dr1Cmd"=304, "Rm1St2Dr1Cmd"=305, "Rm1St3Dr1Cmd"=306, "Rm1St4Dr1Cmd"=307, "Rm1St5Dr1Cmd"=308, "Rm1St6Dr1Cmd"=309, "Rm1St7Dr1Cmd"=310, "Rm1St8Dr1Cmd"=311, "Rm1St1Dr2Cmd"=312, "Rm1St2Dr2Cmd"=313, "Rm1St3Dr2Cmd"=314, "Rm1St4Dr2Cmd"=315, "Rm1St5Dr2Cmd"=316, "Rm1St6Dr2Cmd"=317, "Rm1St7Dr2Cmd"=318, "Rm1St8Dr2Cmd"=319, "Rm1St1Dr3Cmd"=320, "Rm1St2Dr3Cmd"=321, "Rm1St3Dr3Cmd"=322, "Rm1St4Dr3Cmd"=323, "Rm1St5Dr3Cmd"=324, "Rm1St6Dr3Cmd"=325, "Rm1St7Dr3Cmd"=326, "Rm1St8Dr3Cmd"=327, "fwRmTempSP"=328, "fwRmHumSP"=329, "fwCoolTempSP"=330, "fwDehumTempSP"=331, "fwRmRun"=332, "fwRmOk"=333, "fwTesting"=334, "fwRmDryP"=335, "fwRmDryI"=336, "fwRmHumP"=337, "fwRmHumI"=338, "fwRmHeatP"=339, "fwRmHeatI"=340, "fwCoolTempP"=341, "fwCoolTempI"=342, "fwDehumTempP"=343, "fwDehumTempI"=344, "fwGndLeak1"=345, "fwGndLeak2"=346, "fwGndLeak3"=347, "fwGndLeak4"=348, "fwGndLeak5"=349, "fwGndLeak6"=350, "fwGndLeak7"=351, "fwGndLeak8"=352, "Rm1OpenerCmd"=353] ("Ring")
            n52 = event-data() -> ("NewVal"=w154:T41)  [unwired: 1 in, 5 out]
            n53 = Unbundle By Name(w148) -> ("Device Connections.Wago ModBus Connection"=w150:refnum<class "Modbus Master.lvclass">)
            n54 = call-dynamic "Write Single Holding Register.vi"("error in"=w152, "register to write"=w154, "address"=w153, "Modbus master in"=w150) -> ("error out"=w151:errorcluster, "Modbus master out"=w149:refnum<class "Modbus Master.lvclass">)  [unwired: 6 in]
            n55 = Bundle By Name(cluster=w148, "Device Connections.Wago ModBus Connection"=w149) -> (w147:T55)
          }
          event Value Change {
            w163 = T56 297 items=["fwS1Volt1"=0, "fwS1Volt2"=1, "fwS2Volt1"=2, "fwS2Volt2"=3, "fwS3Volt1"=4, "fwS3Volt2"=5, "fwS4Volt1"=6, "fwS4Volt2"=7, "fwS5Volt1"=8, "fwS5Volt2"=9, "fwS6Volt1"=10, "fwS6Volt2 "=11, "fwS7Volt1"=12, "fwS7Volt2"=13, "fwS8Volt1"=14, "fwS8Volt2"=15, "fwRoomHum"=16, "fwRoomTemp"=17, "fwAISpare1"=18, "fwAISpare2"=19, "fwSuppTemp"=20, "fwCoolTemp"=21, "fwDehumTemp"=22, "fwUnused"=23, "Bool Inputs"=24, "gwVoltRate1"=256, "gwVoltRate2"=257, "gwVoltRate3"=258, "gwVoltRate4"=259, "gwVoltRate5"=260, "gwVoltRate6"=261, "gwVoltRate7"=262, "gwVoltRate8"=263, "gwVoltWindow5/1"=264, "gwVoltWindow6/2"=265, "gwVoltWindow7/3"=266, "gwVoltWindow8/4"=267, "fwVoltSet1"=272, "fwVoltSet2"=273, "fwVoltSet3"=274, "fwVoltSet4"=275, "fwVoltSet5"=276, "fwVoltSet6"=277, "fwVoltSet7"=278, "fwVoltSet8"=279, "fwVoltRng1"=280, "fwVoltRng2"=281, "fwVoltRng3"=282, "fwVoltRng4"=283, "fwVoltRng5"=284, "fwVoltRng6"=285, "fwVoltRng7"=286, "fwVoltRng8"=287, "fwVoltPol1"=296, "fwVoltPol2"=297, "fwVoltPol3"=298, "fwVoltPol4"=299, "fwVoltPol5"=300, "fwVoltPol6"=301, "fwVoltPol7"=302, "fwVoltPol8"=303, "Rm1St1Dr1Cmd"=304, "Rm1St2Dr1Cmd"=305, "Rm1St3Dr1Cmd"=306, "Rm1St4Dr1Cmd"=307, "Rm1St5Dr1Cmd"=308, "Rm1St6Dr1Cmd"=309, "Rm1St7Dr1Cmd"=310, "Rm1St8Dr1Cmd"=311, "Rm1St1Dr2Cmd"=312, "Rm1St2Dr2Cmd"=313, "Rm1St3Dr2Cmd"=314, "Rm1St4Dr2Cmd"=315, "Rm1St5Dr2Cmd"=316, "Rm1St6Dr2Cmd"=317, "Rm1St7Dr2Cmd"=318, "Rm1St8Dr2Cmd"=319, "Rm1St1Dr3Cmd"=320, "Rm1St2Dr3Cmd"=321, "Rm1St3Dr3Cmd"=322, "Rm1St4Dr3Cmd"=323, "Rm1St5Dr3Cmd"=324, "Rm1St6Dr3Cmd"=325, "Rm1St7Dr3Cmd"=326, "Rm1St8Dr3Cmd"=327, "fwRmTempSP"=328, "fwRmHumSP"=329, "fwCoolTempSP"=330, "fwDehumTempSP"=331, "fwRmRun"=332, "fwRmOk"=333, "fwTesting"=334, "fwRmDryP"=335, "fwRmDryI"=336, "fwRmHumP"=337, "fwRmHumI"=338, "fwRmHeatP"=339, "fwRmHeatI"=340, "fwCoolTempP"=341, "fwCoolTempI"=342, "fwDehumTempP"=343, "fwDehumTempI"=344, "fwGndLeak1"=345, "fwGndLeak2"=346, "fwGndLeak3"=347, "fwGndLeak4"=348, "fwGndLeak5"=349, "fwGndLeak6"=350, "fwGndLeak7"=351, "fwGndLeak8"=352, "Rm1OpenerCmd"=353] ("Ring")
            n56 = event-data() -> ("NewVal"=w162:T41)  [unwired: 1 in, 5 out]
            n57 = Unbundle By Name(w158) -> ("Device Connections.Wago ModBus Connection"=w161:refnum<class "Modbus Master.lvclass">)
            n58 = call-dynamic "Write Single Holding Register.vi"("error in"=w160, "register to write"=w162, "address"=w163, "Modbus master in"=w161) -> ("error out"=w156:errorcluster, "Modbus master out"=w159:refnum<class "Modbus Master.lvclass">)  [unwired: 6 in]
            n59 = Bundle By Name(cluster=w158, "Device Connections.Wago ModBus Connection"=w159) -> (w157:T55)
          }
          event Value Change {
            w173 = T56 298 items=["fwS1Volt1"=0, "fwS1Volt2"=1, "fwS2Volt1"=2, "fwS2Volt2"=3, "fwS3Volt1"=4, "fwS3Volt2"=5, "fwS4Volt1"=6, "fwS4Volt2"=7, "fwS5Volt1"=8, "fwS5Volt2"=9, "fwS6Volt1"=10, "fwS6Volt2 "=11, "fwS7Volt1"=12, "fwS7Volt2"=13, "fwS8Volt1"=14, "fwS8Volt2"=15, "fwRoomHum"=16, "fwRoomTemp"=17, "fwAISpare1"=18, "fwAISpare2"=19, "fwSuppTemp"=20, "fwCoolTemp"=21, "fwDehumTemp"=22, "fwUnused"=23, "Bool Inputs"=24, "gwVoltRate1"=256, "gwVoltRate2"=257, "gwVoltRate3"=258, "gwVoltRate4"=259, "gwVoltRate5"=260, "gwVoltRate6"=261, "gwVoltRate7"=262, "gwVoltRate8"=263, "gwVoltWindow5/1"=264, "gwVoltWindow6/2"=265, "gwVoltWindow7/3"=266, "gwVoltWindow8/4"=267, "fwVoltSet1"=272, "fwVoltSet2"=273, "fwVoltSet3"=274, "fwVoltSet4"=275, "fwVoltSet5"=276, "fwVoltSet6"=277, "fwVoltSet7"=278, "fwVoltSet8"=279, "fwVoltRng1"=280, "fwVoltRng2"=281, "fwVoltRng3"=282, "fwVoltRng4"=283, "fwVoltRng5"=284, "fwVoltRng6"=285, "fwVoltRng7"=286, "fwVoltRng8"=287, "fwVoltPol1"=296, "fwVoltPol2"=297, "fwVoltPol3"=298, "fwVoltPol4"=299, "fwVoltPol5"=300, "fwVoltPol6"=301, "fwVoltPol7"=302, "fwVoltPol8"=303, "Rm1St1Dr1Cmd"=304, "Rm1St2Dr1Cmd"=305, "Rm1St3Dr1Cmd"=306, "Rm1St4Dr1Cmd"=307, "Rm1St5Dr1Cmd"=308, "Rm1St6Dr1Cmd"=309, "Rm1St7Dr1Cmd"=310, "Rm1St8Dr1Cmd"=311, "Rm1St1Dr2Cmd"=312, "Rm1St2Dr2Cmd"=313, "Rm1St3Dr2Cmd"=314, "Rm1St4Dr2Cmd"=315, "Rm1St5Dr2Cmd"=316, "Rm1St6Dr2Cmd"=317, "Rm1St7Dr2Cmd"=318, "Rm1St8Dr2Cmd"=319, "Rm1St1Dr3Cmd"=320, "Rm1St2Dr3Cmd"=321, "Rm1St3Dr3Cmd"=322, "Rm1St4Dr3Cmd"=323, "Rm1St5Dr3Cmd"=324, "Rm1St6Dr3Cmd"=325, "Rm1St7Dr3Cmd"=326, "Rm1St8Dr3Cmd"=327, "fwRmTempSP"=328, "fwRmHumSP"=329, "fwCoolTempSP"=330, "fwDehumTempSP"=331, "fwRmRun"=332, "fwRmOk"=333, "fwTesting"=334, "fwRmDryP"=335, "fwRmDryI"=336, "fwRmHumP"=337, "fwRmHumI"=338, "fwRmHeatP"=339, "fwRmHeatI"=340, "fwCoolTempP"=341, "fwCoolTempI"=342, "fwDehumTempP"=343, "fwDehumTempI"=344, "fwGndLeak1"=345, "fwGndLeak2"=346, "fwGndLeak3"=347, "fwGndLeak4"=348, "fwGndLeak5"=349, "fwGndLeak6"=350, "fwGndLeak7"=351, "fwGndLeak8"=352, "Rm1OpenerCmd"=353] ("Ring")
            n60 = event-data() -> ("NewVal"=w172:T41)  [unwired: 1 in, 5 out]
            n61 = Unbundle By Name(w166) -> ("Device Connections.Wago ModBus Connection"=w169:refnum<class "Modbus Master.lvclass">)
            n62 = call-dynamic "Write Single Holding Register.vi"("error in"=w170, "register to write"=w172, "address"=w173, "Modbus master in"=w169) -> ("error out"=w168:errorcluster, "Modbus master out"=w167:refnum<class "Modbus Master.lvclass">)  [unwired: 6 in]
            n63 = Bundle By Name(cluster=w166, "Device Connections.Wago ModBus Connection"=w167) -> (w165:T55)
          }
          event Value Change {
            w182 = T56 299 items=["fwS1Volt1"=0, "fwS1Volt2"=1, "fwS2Volt1"=2, "fwS2Volt2"=3, "fwS3Volt1"=4, "fwS3Volt2"=5, "fwS4Volt1"=6, "fwS4Volt2"=7, "fwS5Volt1"=8, "fwS5Volt2"=9, "fwS6Volt1"=10, "fwS6Volt2 "=11, "fwS7Volt1"=12, "fwS7Volt2"=13, "fwS8Volt1"=14, "fwS8Volt2"=15, "fwRoomHum"=16, "fwRoomTemp"=17, "fwAISpare1"=18, "fwAISpare2"=19, "fwSuppTemp"=20, "fwCoolTemp"=21, "fwDehumTemp"=22, "fwUnused"=23, "Bool Inputs"=24, "gwVoltRate1"=256, "gwVoltRate2"=257, "gwVoltRate3"=258, "gwVoltRate4"=259, "gwVoltRate5"=260, "gwVoltRate6"=261, "gwVoltRate7"=262, "gwVoltRate8"=263, "gwVoltWindow5/1"=264, "gwVoltWindow6/2"=265, "gwVoltWindow7/3"=266, "gwVoltWindow8/4"=267, "fwVoltSet1"=272, "fwVoltSet2"=273, "fwVoltSet3"=274, "fwVoltSet4"=275, "fwVoltSet5"=276, "fwVoltSet6"=277, "fwVoltSet7"=278, "fwVoltSet8"=279, "fwVoltRng1"=280, "fwVoltRng2"=281, "fwVoltRng3"=282, "fwVoltRng4"=283, "fwVoltRng5"=284, "fwVoltRng6"=285, "fwVoltRng7"=286, "fwVoltRng8"=287, "fwVoltPol1"=296, "fwVoltPol2"=297, "fwVoltPol3"=298, "fwVoltPol4"=299, "fwVoltPol5"=300, "fwVoltPol6"=301, "fwVoltPol7"=302, "fwVoltPol8"=303, "Rm1St1Dr1Cmd"=304, "Rm1St2Dr1Cmd"=305, "Rm1St3Dr1Cmd"=306, "Rm1St4Dr1Cmd"=307, "Rm1St5Dr1Cmd"=308, "Rm1St6Dr1Cmd"=309, "Rm1St7Dr1Cmd"=310, "Rm1St8Dr1Cmd"=311, "Rm1St1Dr2Cmd"=312, "Rm1St2Dr2Cmd"=313, "Rm1St3Dr2Cmd"=314, "Rm1St4Dr2Cmd"=315, "Rm1St5Dr2Cmd"=316, "Rm1St6Dr2Cmd"=317, "Rm1St7Dr2Cmd"=318, "Rm1St8Dr2Cmd"=319, "Rm1St1Dr3Cmd"=320, "Rm1St2Dr3Cmd"=321, "Rm1St3Dr3Cmd"=322, "Rm1St4Dr3Cmd"=323, "Rm1St5Dr3Cmd"=324, "Rm1St6Dr3Cmd"=325, "Rm1St7Dr3Cmd"=326, "Rm1St8Dr3Cmd"=327, "fwRmTempSP"=328, "fwRmHumSP"=329, "fwCoolTempSP"=330, "fwDehumTempSP"=331, "fwRmRun"=332, "fwRmOk"=333, "fwTesting"=334, "fwRmDryP"=335, "fwRmDryI"=336, "fwRmHumP"=337, "fwRmHumI"=338, "fwRmHeatP"=339, "fwRmHeatI"=340, "fwCoolTempP"=341, "fwCoolTempI"=342, "fwDehumTempP"=343, "fwDehumTempI"=344, "fwGndLeak1"=345, "fwGndLeak2"=346, "fwGndLeak3"=347, "fwGndLeak4"=348, "fwGndLeak5"=349, "fwGndLeak6"=350, "fwGndLeak7"=351, "fwGndLeak8"=352, "Rm1OpenerCmd"=353] ("Ring")
            n64 = event-data() -> ("NewVal"=w180:T41)  [unwired: 1 in, 5 out]
            n65 = Unbundle By Name(w175) -> ("Device Connections.Wago ModBus Connection"=w177:refnum<class "Modbus Master.lvclass">)
            n66 = call-dynamic "Write Single Holding Register.vi"("error in"=w178, "register to write"=w180, "address"=w182, "Modbus master in"=w177) -> ("error out"=w179:errorcluster, "Modbus master out"=w176:refnum<class "Modbus Master.lvclass">)  [unwired: 6 in]
            n67 = Bundle By Name(cluster=w175, "Device Connections.Wago ModBus Connection"=w176) -> (w174:T55)
          }
          event Value Change {
            w191 = T56 300 items=["fwS1Volt1"=0, "fwS1Volt2"=1, "fwS2Volt1"=2, "fwS2Volt2"=3, "fwS3Volt1"=4, "fwS3Volt2"=5, "fwS4Volt1"=6, "fwS4Volt2"=7, "fwS5Volt1"=8, "fwS5Volt2"=9, "fwS6Volt1"=10, "fwS6Volt2 "=11, "fwS7Volt1"=12, "fwS7Volt2"=13, "fwS8Volt1"=14, "fwS8Volt2"=15, "fwRoomHum"=16, "fwRoomTemp"=17, "fwAISpare1"=18, "fwAISpare2"=19, "fwSuppTemp"=20, "fwCoolTemp"=21, "fwDehumTemp"=22, "fwUnused"=23, "Bool Inputs"=24, "gwVoltRate1"=256, "gwVoltRate2"=257, "gwVoltRate3"=258, "gwVoltRate4"=259, "gwVoltRate5"=260, "gwVoltRate6"=261, "gwVoltRate7"=262, "gwVoltRate8"=263, "gwVoltWindow5/1"=264, "gwVoltWindow6/2"=265, "gwVoltWindow7/3"=266, "gwVoltWindow8/4"=267, "fwVoltSet1"=272, "fwVoltSet2"=273, "fwVoltSet3"=274, "fwVoltSet4"=275, "fwVoltSet5"=276, "fwVoltSet6"=277, "fwVoltSet7"=278, "fwVoltSet8"=279, "fwVoltRng1"=280, "fwVoltRng2"=281, "fwVoltRng3"=282, "fwVoltRng4"=283, "fwVoltRng5"=284, "fwVoltRng6"=285, "fwVoltRng7"=286, "fwVoltRng8"=287, "fwVoltPol1"=296, "fwVoltPol2"=297, "fwVoltPol3"=298, "fwVoltPol4"=299, "fwVoltPol5"=300, "fwVoltPol6"=301, "fwVoltPol7"=302, "fwVoltPol8"=303, "Rm1St1Dr1Cmd"=304, "Rm1St2Dr1Cmd"=305, "Rm1St3Dr1Cmd"=306, "Rm1St4Dr1Cmd"=307, "Rm1St5Dr1Cmd"=308, "Rm1St6Dr1Cmd"=309, "Rm1St7Dr1Cmd"=310, "Rm1St8Dr1Cmd"=311, "Rm1St1Dr2Cmd"=312, "Rm1St2Dr2Cmd"=313, "Rm1St3Dr2Cmd"=314, "Rm1St4Dr2Cmd"=315, "Rm1St5Dr2Cmd"=316, "Rm1St6Dr2Cmd"=317, "Rm1St7Dr2Cmd"=318, "Rm1St8Dr2Cmd"=319, "Rm1St1Dr3Cmd"=320, "Rm1St2Dr3Cmd"=321, "Rm1St3Dr3Cmd"=322, "Rm1St4Dr3Cmd"=323, "Rm1St5Dr3Cmd"=324, "Rm1St6Dr3Cmd"=325, "Rm1St7Dr3Cmd"=326, "Rm1St8Dr3Cmd"=327, "fwRmTempSP"=328, "fwRmHumSP"=329, "fwCoolTempSP"=330, "fwDehumTempSP"=331, "fwRmRun"=332, "fwRmOk"=333, "fwTesting"=334, "fwRmDryP"=335, "fwRmDryI"=336, "fwRmHumP"=337, "fwRmHumI"=338, "fwRmHeatP"=339, "fwRmHeatI"=340, "fwCoolTempP"=341, "fwCoolTempI"=342, "fwDehumTempP"=343, "fwDehumTempI"=344, "fwGndLeak1"=345, "fwGndLeak2"=346, "fwGndLeak3"=347, "fwGndLeak4"=348, "fwGndLeak5"=349, "fwGndLeak6"=350, "fwGndLeak7"=351, "fwGndLeak8"=352, "Rm1OpenerCmd"=353] ("Ring")
            n68 = event-data() -> ("NewVal"=w190:T41)  [unwired: 1 in, 5 out]
            n69 = Unbundle By Name(w184) -> ("Device Connections.Wago ModBus Connection"=w186:refnum<class "Modbus Master.lvclass">)
            n70 = call-dynamic "Write Single Holding Register.vi"("error in"=w187, "register to write"=w190, "address"=w191, "Modbus master in"=w186) -> ("error out"=w188:errorcluster, "Modbus master out"=w185:refnum<class "Modbus Master.lvclass">)  [unwired: 6 in]
            n71 = Bundle By Name(cluster=w184, "Device Connections.Wago ModBus Connection"=w185) -> (w183:T55)
          }
          event Value Change {
            w200 = T56 301 items=["fwS1Volt1"=0, "fwS1Volt2"=1, "fwS2Volt1"=2, "fwS2Volt2"=3, "fwS3Volt1"=4, "fwS3Volt2"=5, "fwS4Volt1"=6, "fwS4Volt2"=7, "fwS5Volt1"=8, "fwS5Volt2"=9, "fwS6Volt1"=10, "fwS6Volt2 "=11, "fwS7Volt1"=12, "fwS7Volt2"=13, "fwS8Volt1"=14, "fwS8Volt2"=15, "fwRoomHum"=16, "fwRoomTemp"=17, "fwAISpare1"=18, "fwAISpare2"=19, "fwSuppTemp"=20, "fwCoolTemp"=21, "fwDehumTemp"=22, "fwUnused"=23, "Bool Inputs"=24, "gwVoltRate1"=256, "gwVoltRate2"=257, "gwVoltRate3"=258, "gwVoltRate4"=259, "gwVoltRate5"=260, "gwVoltRate6"=261, "gwVoltRate7"=262, "gwVoltRate8"=263, "gwVoltWindow5/1"=264, "gwVoltWindow6/2"=265, "gwVoltWindow7/3"=266, "gwVoltWindow8/4"=267, "fwVoltSet1"=272, "fwVoltSet2"=273, "fwVoltSet3"=274, "fwVoltSet4"=275, "fwVoltSet5"=276, "fwVoltSet6"=277, "fwVoltSet7"=278, "fwVoltSet8"=279, "fwVoltRng1"=280, "fwVoltRng2"=281, "fwVoltRng3"=282, "fwVoltRng4"=283, "fwVoltRng5"=284, "fwVoltRng6"=285, "fwVoltRng7"=286, "fwVoltRng8"=287, "fwVoltPol1"=296, "fwVoltPol2"=297, "fwVoltPol3"=298, "fwVoltPol4"=299, "fwVoltPol5"=300, "fwVoltPol6"=301, "fwVoltPol7"=302, "fwVoltPol8"=303, "Rm1St1Dr1Cmd"=304, "Rm1St2Dr1Cmd"=305, "Rm1St3Dr1Cmd"=306, "Rm1St4Dr1Cmd"=307, "Rm1St5Dr1Cmd"=308, "Rm1St6Dr1Cmd"=309, "Rm1St7Dr1Cmd"=310, "Rm1St8Dr1Cmd"=311, "Rm1St1Dr2Cmd"=312, "Rm1St2Dr2Cmd"=313, "Rm1St3Dr2Cmd"=314, "Rm1St4Dr2Cmd"=315, "Rm1St5Dr2Cmd"=316, "Rm1St6Dr2Cmd"=317, "Rm1St7Dr2Cmd"=318, "Rm1St8Dr2Cmd"=319, "Rm1St1Dr3Cmd"=320, "Rm1St2Dr3Cmd"=321, "Rm1St3Dr3Cmd"=322, "Rm1St4Dr3Cmd"=323, "Rm1St5Dr3Cmd"=324, "Rm1St6Dr3Cmd"=325, "Rm1St7Dr3Cmd"=326, "Rm1St8Dr3Cmd"=327, "fwRmTempSP"=328, "fwRmHumSP"=329, "fwCoolTempSP"=330, "fwDehumTempSP"=331, "fwRmRun"=332, "fwRmOk"=333, "fwTesting"=334, "fwRmDryP"=335, "fwRmDryI"=336, "fwRmHumP"=337, "fwRmHumI"=338, "fwRmHeatP"=339, "fwRmHeatI"=340, "fwCoolTempP"=341, "fwCoolTempI"=342, "fwDehumTempP"=343, "fwDehumTempI"=344, "fwGndLeak1"=345, "fwGndLeak2"=346, "fwGndLeak3"=347, "fwGndLeak4"=348, "fwGndLeak5"=349, "fwGndLeak6"=350, "fwGndLeak7"=351, "fwGndLeak8"=352, "Rm1OpenerCmd"=353] ("Ring")
            n72 = event-data() -> ("NewVal"=w199:T41)  [unwired: 1 in, 5 out]
            n73 = Unbundle By Name(w194) -> ("Device Connections.Wago ModBus Connection"=w192:refnum<class "Modbus Master.lvclass">)
            n74 = call-dynamic "Write Single Holding Register.vi"("error in"=w196, "register to write"=w199, "address"=w200, "Modbus master in"=w192) -> ("error out"=w197:errorcluster, "Modbus master out"=w195:refnum<class "Modbus Master.lvclass">)  [unwired: 6 in]
            n75 = Bundle By Name(cluster=w194, "Device Connections.Wago ModBus Connection"=w195) -> (w193:T55)
          }
          event Value Change {
            w208 = T56 302 items=["fwS1Volt1"=0, "fwS1Volt2"=1, "fwS2Volt1"=2, "fwS2Volt2"=3, "fwS3Volt1"=4, "fwS3Volt2"=5, "fwS4Volt1"=6, "fwS4Volt2"=7, "fwS5Volt1"=8, "fwS5Volt2"=9, "fwS6Volt1"=10, "fwS6Volt2 "=11, "fwS7Volt1"=12, "fwS7Volt2"=13, "fwS8Volt1"=14, "fwS8Volt2"=15, "fwRoomHum"=16, "fwRoomTemp"=17, "fwAISpare1"=18, "fwAISpare2"=19, "fwSuppTemp"=20, "fwCoolTemp"=21, "fwDehumTemp"=22, "fwUnused"=23, "Bool Inputs"=24, "gwVoltRate1"=256, "gwVoltRate2"=257, "gwVoltRate3"=258, "gwVoltRate4"=259, "gwVoltRate5"=260, "gwVoltRate6"=261, "gwVoltRate7"=262, "gwVoltRate8"=263, "gwVoltWindow5/1"=264, "gwVoltWindow6/2"=265, "gwVoltWindow7/3"=266, "gwVoltWindow8/4"=267, "fwVoltSet1"=272, "fwVoltSet2"=273, "fwVoltSet3"=274, "fwVoltSet4"=275, "fwVoltSet5"=276, "fwVoltSet6"=277, "fwVoltSet7"=278, "fwVoltSet8"=279, "fwVoltRng1"=280, "fwVoltRng2"=281, "fwVoltRng3"=282, "fwVoltRng4"=283, "fwVoltRng5"=284, "fwVoltRng6"=285, "fwVoltRng7"=286, "fwVoltRng8"=287, "fwVoltPol1"=296, "fwVoltPol2"=297, "fwVoltPol3"=298, "fwVoltPol4"=299, "fwVoltPol5"=300, "fwVoltPol6"=301, "fwVoltPol7"=302, "fwVoltPol8"=303, "Rm1St1Dr1Cmd"=304, "Rm1St2Dr1Cmd"=305, "Rm1St3Dr1Cmd"=306, "Rm1St4Dr1Cmd"=307, "Rm1St5Dr1Cmd"=308, "Rm1St6Dr1Cmd"=309, "Rm1St7Dr1Cmd"=310, "Rm1St8Dr1Cmd"=311, "Rm1St1Dr2Cmd"=312, "Rm1St2Dr2Cmd"=313, "Rm1St3Dr2Cmd"=314, "Rm1St4Dr2Cmd"=315, "Rm1St5Dr2Cmd"=316, "Rm1St6Dr2Cmd"=317, "Rm1St7Dr2Cmd"=318, "Rm1St8Dr2Cmd"=319, "Rm1St1Dr3Cmd"=320, "Rm1St2Dr3Cmd"=321, "Rm1St3Dr3Cmd"=322, "Rm1St4Dr3Cmd"=323, "Rm1St5Dr3Cmd"=324, "Rm1St6Dr3Cmd"=325, "Rm1St7Dr3Cmd"=326, "Rm1St8Dr3Cmd"=327, "fwRmTempSP"=328, "fwRmHumSP"=329, "fwCoolTempSP"=330, "fwDehumTempSP"=331, "fwRmRun"=332, "fwRmOk"=333, "fwTesting"=334, "fwRmDryP"=335, "fwRmDryI"=336, "fwRmHumP"=337, "fwRmHumI"=338, "fwRmHeatP"=339, "fwRmHeatI"=340, "fwCoolTempP"=341, "fwCoolTempI"=342, "fwDehumTempP"=343, "fwDehumTempI"=344, "fwGndLeak1"=345, "fwGndLeak2"=346, "fwGndLeak3"=347, "fwGndLeak4"=348, "fwGndLeak5"=349, "fwGndLeak6"=350, "fwGndLeak7"=351, "fwGndLeak8"=352, "Rm1OpenerCmd"=353] ("Ring")
            n76 = event-data() -> ("NewVal"=w207:T41)  [unwired: 1 in, 5 out]
            n77 = Unbundle By Name(w202) -> ("Device Connections.Wago ModBus Connection"=w204:refnum<class "Modbus Master.lvclass">)
            n78 = call-dynamic "Write Single Holding Register.vi"("error in"=w206, "register to write"=w207, "address"=w208, "Modbus master in"=w204) -> ("error out"=w205:errorcluster, "Modbus master out"=w203:refnum<class "Modbus Master.lvclass">)  [unwired: 6 in]
            n79 = Bundle By Name(cluster=w202, "Device Connections.Wago ModBus Connection"=w203) -> (w201:T55)
          }
          event Value Change {
            w218 = T56 303 items=["fwS1Volt1"=0, "fwS1Volt2"=1, "fwS2Volt1"=2, "fwS2Volt2"=3, "fwS3Volt1"=4, "fwS3Volt2"=5, "fwS4Volt1"=6, "fwS4Volt2"=7, "fwS5Volt1"=8, "fwS5Volt2"=9, "fwS6Volt1"=10, "fwS6Volt2 "=11, "fwS7Volt1"=12, "fwS7Volt2"=13, "fwS8Volt1"=14, "fwS8Volt2"=15, "fwRoomHum"=16, "fwRoomTemp"=17, "fwAISpare1"=18, "fwAISpare2"=19, "fwSuppTemp"=20, "fwCoolTemp"=21, "fwDehumTemp"=22, "fwUnused"=23, "Bool Inputs"=24, "gwVoltRate1"=256, "gwVoltRate2"=257, "gwVoltRate3"=258, "gwVoltRate4"=259, "gwVoltRate5"=260, "gwVoltRate6"=261, "gwVoltRate7"=262, "gwVoltRate8"=263, "gwVoltWindow5/1"=264, "gwVoltWindow6/2"=265, "gwVoltWindow7/3"=266, "gwVoltWindow8/4"=267, "fwVoltSet1"=272, "fwVoltSet2"=273, "fwVoltSet3"=274, "fwVoltSet4"=275, "fwVoltSet5"=276, "fwVoltSet6"=277, "fwVoltSet7"=278, "fwVoltSet8"=279, "fwVoltRng1"=280, "fwVoltRng2"=281, "fwVoltRng3"=282, "fwVoltRng4"=283, "fwVoltRng5"=284, "fwVoltRng6"=285, "fwVoltRng7"=286, "fwVoltRng8"=287, "fwVoltPol1"=296, "fwVoltPol2"=297, "fwVoltPol3"=298, "fwVoltPol4"=299, "fwVoltPol5"=300, "fwVoltPol6"=301, "fwVoltPol7"=302, "fwVoltPol8"=303, "Rm1St1Dr1Cmd"=304, "Rm1St2Dr1Cmd"=305, "Rm1St3Dr1Cmd"=306, "Rm1St4Dr1Cmd"=307, "Rm1St5Dr1Cmd"=308, "Rm1St6Dr1Cmd"=309, "Rm1St7Dr1Cmd"=310, "Rm1St8Dr1Cmd"=311, "Rm1St1Dr2Cmd"=312, "Rm1St2Dr2Cmd"=313, "Rm1St3Dr2Cmd"=314, "Rm1St4Dr2Cmd"=315, "Rm1St5Dr2Cmd"=316, "Rm1St6Dr2Cmd"=317, "Rm1St7Dr2Cmd"=318, "Rm1St8Dr2Cmd"=319, "Rm1St1Dr3Cmd"=320, "Rm1St2Dr3Cmd"=321, "Rm1St3Dr3Cmd"=322, "Rm1St4Dr3Cmd"=323, "Rm1St5Dr3Cmd"=324, "Rm1St6Dr3Cmd"=325, "Rm1St7Dr3Cmd"=326, "Rm1St8Dr3Cmd"=327, "fwRmTempSP"=328, "fwRmHumSP"=329, "fwCoolTempSP"=330, "fwDehumTempSP"=331, "fwRmRun"=332, "fwRmOk"=333, "fwTesting"=334, "fwRmDryP"=335, "fwRmDryI"=336, "fwRmHumP"=337, "fwRmHumI"=338, "fwRmHeatP"=339, "fwRmHeatI"=340, "fwCoolTempP"=341, "fwCoolTempI"=342, "fwDehumTempP"=343, "fwDehumTempI"=344, "fwGndLeak1"=345, "fwGndLeak2"=346, "fwGndLeak3"=347, "fwGndLeak4"=348, "fwGndLeak5"=349, "fwGndLeak6"=350, "fwGndLeak7"=351, "fwGndLeak8"=352, "Rm1OpenerCmd"=353] ("Ring")
            n80 = event-data() -> ("NewVal"=w217:T41)  [unwired: 1 in, 5 out]
            n81 = Unbundle By Name(w210) -> ("Device Connections.Wago ModBus Connection"=w213:refnum<class "Modbus Master.lvclass">)
            n82 = call-dynamic "Write Single Holding Register.vi"("error in"=w215, "register to write"=w217, "address"=w218, "Modbus master in"=w213) -> ("error out"=w214:errorcluster, "Modbus master out"=w212:refnum<class "Modbus Master.lvclass">)  [unwired: 6 in]
            n83 = Bundle By Name(cluster=w210, "Device Connections.Wago ModBus Connection"=w212) -> (w211:T55)
          }
          event "Update Room Setpoint": Value Change {
            n84 = event-data() -> ()  [unwired: 1 in, 6 out]
            n85 = Unbundle By Name(w220) -> ("Device Connections.Wago ModBus Connection"=w223:refnum<class "Modbus Master.lvclass">)
            n86 = call "Wago Chamber Setpoints.vi"("error in (no error)"=w224, "Room Setpoints"="Room Setpoints", "Modbus Master in"=w223) -> ("error out"=w222:errorcluster, "Modbus master out"=w221:refnum<class "Modbus Master.lvclass">)  [unwired: 7 in]
            n87 = Bundle By Name(cluster=w220, "Device Connections.Wago ModBus Connection"=w221) -> (w219:T55)
          }
          event "Test Chamber Set Parameters": Value Change {
            n88 = event-data() -> ()  [unwired: 1 in, 6 out]
            n89 = call <vilib>:"Add State(s) to Queue__jki_lib_state_machine.vi"("State(s) in Front (\"\")"="Set Chamber Parameters" ("State(s) in Front (\"\")"), "State(s) in (\"\")"=w230) -> ("States Out"=w229:string)  [unwired: 13 in]
          }
          event "Station Voltage Send 1": Value Change {
            n90 = event-data() -> ()  [unwired: 1 in, 6 out]
            n91 = Unbundle By Name(w235) -> ("Device Connections.APLUS 1 Modbus Connection"=w236:refnum<class "Modbus Master.lvclass">, "Device Connections.Wago ModBus Connection"=w237:refnum<class "Modbus Master.lvclass">)
            n92 = call "RTS Voltage Frequency Selector.vi"("Frequency"="Frequency", "Station Number"=u16 1, "Voltage"="Voltage", "error in (no error)"=w239, "Modbus Master in"=w237) -> ("error out"=w238:errorcluster, "Modbus master out"=w232:refnum<class "Modbus Master.lvclass">)  [unwired: 5 in]
            n93 = case shown="\"Reset Watt Hours\"" "Wh Reset 1" {
              tunnel: w238 -> [w247 w250]
              tunnel: [w247 w251] -> w240
              tunnel: w236 -> [w246 w249]
              tunnel: [w246 w248] -> w233
              frame "", Default {
              }
              frame "Reset Watt Hours" {
                n94 = call "APLUS Reset WH Coil.vi"("Error In"=w250, "Reset WattHours"=TRUE, "Modbus Master in"=w249) -> ("Error Out"=w251:errorcluster, "Modbus Master out"=w248:refnum<class "Modbus Master.lvclass">)  [unwired: 7 in]
              }
            }
            n95 = Bundle By Name(cluster=w235, "Device Connections.APLUS 1 Modbus Connection"=w233, "Device Connections.Wago ModBus Connection"=w232) -> (w234:T55)
          }
          event "Station Voltage Send 2": Value Change {
            n96 = event-data() -> ()  [unwired: 1 in, 6 out]
            n97 = Unbundle By Name(w254) -> ("Device Connections.APLUS 2 Modbus Connection"=w258:refnum<class "Modbus Master.lvclass">, "Device Connections.Wago ModBus Connection"=w259:refnum<class "Modbus Master.lvclass">)
            n98 = call "RTS Voltage Frequency Selector.vi"("Frequency"="Frequency 2", "Station Number"=u16 2, "Voltage"="Voltage 2", "error in (no error)"=w260, "Modbus Master in"=w259) -> ("error out"=w257:errorcluster, "Modbus master out"=w255:refnum<class "Modbus Master.lvclass">)  [unwired: 5 in]
            n99 = case shown="\"Reset Watt Hours\"" "Wh Reset 2" {
              tunnel: w257 -> [w268 w271]
              tunnel: [w268 w272] -> w261
              tunnel: w258 -> [w267 w270]
              tunnel: [w267 w269] -> w256
              frame "", Default {
              }
              frame "Reset Watt Hours" {
                n100 = call "APLUS Reset WH Coil.vi"("Error In"=w271, "Reset WattHours"=TRUE, "Modbus Master in"=w270) -> ("Error Out"=w272:errorcluster, "Modbus Master out"=w269:refnum<class "Modbus Master.lvclass">)  [unwired: 7 in]
              }
            }
            n101 = Bundle By Name(cluster=w254, "Device Connections.APLUS 2 Modbus Connection"=w256, "Device Connections.Wago ModBus Connection"=w255) -> (w253:T55)
          }
          event "Station Voltage Send 3": Value Change {
            n102 = event-data() -> ()  [unwired: 1 in, 6 out]
            n103 = Unbundle By Name(w277) -> ("Device Connections.APLUS 3 Modbus Connection"=w279:refnum<class "Modbus Master.lvclass">, "Device Connections.Wago ModBus Connection"=w278:refnum<class "Modbus Master.lvclass">)
            n104 = call "RTS Voltage Frequency Selector.vi"("Frequency"="Frequency 3", "Station Number"=u16 3, "Voltage"="Voltage 3", "error in (no error)"=w280, "Modbus Master in"=w278) -> ("error out"=w281:errorcluster, "Modbus master out"=w275:refnum<class "Modbus Master.lvclass">)  [unwired: 5 in]
            n105 = case shown="\"\", Default" "Wh Reset 3" {
              tunnel: w281 -> [w289 w292]
              tunnel: [w289 w293] -> w285
              tunnel: w279 -> [w288 w291]
              tunnel: [w288 w290] -> w274
              frame "", Default {
              }
              frame "Reset Watt Hours" {
                n106 = call "APLUS Reset WH Coil.vi"("Error In"=w292, "Reset WattHours"=TRUE, "Modbus Master in"=w291) -> ("Error Out"=w293:errorcluster, "Modbus Master out"=w290:refnum<class "Modbus Master.lvclass">)  [unwired: 7 in]
              }
            }
            n107 = Bundle By Name(cluster=w277, "Device Connections.APLUS 3 Modbus Connection"=w274, "Device Connections.Wago ModBus Connection"=w275) -> (w276:T55)
          }
          event "Station Voltage Send 4": Value Change {
            n108 = event-data() -> ()  [unwired: 1 in, 6 out]
            n109 = Unbundle By Name(w297) -> ("Device Connections.APLUS 4 Modbus Connection"=w299:refnum<class "Modbus Master.lvclass">, "Device Connections.Wago ModBus Connection"=w300:refnum<class "Modbus Master.lvclass">)
            n110 = call "RTS Voltage Frequency Selector.vi"("Frequency"="Frequency 4", "Station Number"=u16 4, "Voltage"="Voltage 4", "error in (no error)"=w302, "Modbus Master in"=w300) -> ("error out"=w301:errorcluster, "Modbus master out"=w295:refnum<class "Modbus Master.lvclass">)  [unwired: 5 in]
            n111 = case shown="\"Reset Watt Hours\"" "Wh Reset 4" {
              tunnel: w301 -> [w310 w314]
              tunnel: [w310 w313] -> w306
              tunnel: w299 -> [w309 w312]
              tunnel: [w309 w311] -> w298
              frame "", Default {
              }
              frame "Reset Watt Hours" {
                n112 = call "APLUS Reset WH Coil.vi"("Error In"=w314, "Reset WattHours"=TRUE, "Modbus Master in"=w312) -> ("Error Out"=w313:errorcluster, "Modbus Master out"=w311:refnum<class "Modbus Master.lvclass">)  [unwired: 7 in]
              }
            }
            n113 = Bundle By Name(cluster=w297, "Device Connections.APLUS 4 Modbus Connection"=w298, "Device Connections.Wago ModBus Connection"=w295) -> (w296:T55)
          }
          event "Station Voltage Send 5": Value Change {
            n114 = event-data() -> ()  [unwired: 1 in, 6 out]
            n115 = Unbundle By Name(w319) -> ("Device Connections.APLUS 5 Modbus Connection"=w320:refnum<class "Modbus Master.lvclass">, "Device Connections.Wago ModBus Connection"=w321:refnum<class "Modbus Master.lvclass">)
            n116 = call "RTS Voltage Frequency Selector.vi"("Frequency"="Frequency 5", "Station Number"=u16 5, "Voltage"="Voltage 5", "error in (no error)"=w322, "Modbus Master in"=w321) -> ("error out"=w323:errorcluster, "Modbus master out"=w316:refnum<class "Modbus Master.lvclass">)  [unwired: 5 in]
            n117 = case shown="\"\", Default" "Wh Reset 5" {
              tunnel: w323 -> [w331 w335]
              tunnel: [w331 w334] -> w327
              tunnel: w320 -> [w330 w333]
              tunnel: [w330 w332] -> w317
              frame "", Default {
              }
              frame "Reset Watt Hours" {
                n118 = call "APLUS Reset WH Coil.vi"("Error In"=w335, "Reset WattHours"=TRUE, "Modbus Master in"=w333) -> ("Error Out"=w334:errorcluster, "Modbus Master out"=w332:refnum<class "Modbus Master.lvclass">)  [unwired: 7 in]
              }
            }
            n119 = Bundle By Name(cluster=w319, "Device Connections.APLUS 5 Modbus Connection"=w317, "Device Connections.Wago ModBus Connection"=w316) -> (w318:T55)
          }
          event "Station Voltage Send 6": Value Change {
            n120 = event-data() -> ()  [unwired: 1 in, 6 out]
            n121 = Unbundle By Name(w338) -> ("Device Connections.APLUS 6 Modbus Connection"=w341:refnum<class "Modbus Master.lvclass">, "Device Connections.Wago ModBus Connection"=w342:refnum<class "Modbus Master.lvclass">)
            n122 = call "RTS Voltage Frequency Selector.vi"("Frequency"="Frequency 6", "Station Number"=u16 6, "Voltage"="Voltage 6", "error in (no error)"=w344, "Modbus Master in"=w342) -> ("error out"=w343:errorcluster, "Modbus master out"=w339:refnum<class "Modbus Master.lvclass">)  [unwired: 5 in]
            n123 = case shown="\"Reset Watt Hours\"" "Wh Reset 6" {
              tunnel: w343 -> [w352 w356]
              tunnel: [w352 w355] -> w348
              tunnel: w341 -> [w351 w354]
              tunnel: [w351 w353] -> w340
              frame "", Default {
              }
              frame "Reset Watt Hours" {
                n124 = call "APLUS Reset WH Coil.vi"("Error In"=w356, "Reset WattHours"=TRUE, "Modbus Master in"=w354) -> ("Error Out"=w355:errorcluster, "Modbus Master out"=w353:refnum<class "Modbus Master.lvclass">)  [unwired: 7 in]
              }
            }
            n125 = Bundle By Name(cluster=w338, "Device Connections.APLUS 6 Modbus Connection"=w340, "Device Connections.Wago ModBus Connection"=w339) -> (w337:T55)
          }
          event "Station Voltage Send 7": Value Change {
            n126 = event-data() -> ()  [unwired: 1 in, 6 out]
            n127 = Unbundle By Name(w359) -> ("Device Connections.APLUS 7 Modbus Connection"=w362:refnum<class "Modbus Master.lvclass">, "Device Connections.Wago ModBus Connection"=w363:refnum<class "Modbus Master.lvclass">)
            n128 = call "RTS Voltage Frequency Selector.vi"("Frequency"="Frequency 7", "Station Number"=u16 7, "Voltage"="Voltage 7", "error in (no error)"=w365, "Modbus Master in"=w363) -> ("error out"=w364:errorcluster, "Modbus master out"=w361:refnum<class "Modbus Master.lvclass">)  [unwired: 5 in]
            n129 = case shown="\"Reset Watt Hours\"" "Wh Reset 7" {
              tunnel: w364 -> [w373 w377]
              tunnel: [w373 w376] -> w369
              tunnel: w362 -> [w372 w375]
              tunnel: [w372 w374] -> w360
              frame "", Default {
              }
              frame "Reset Watt Hours" {
                n130 = call "APLUS Reset WH Coil.vi"("Error In"=w377, "Reset WattHours"=TRUE, "Modbus Master in"=w375) -> ("Error Out"=w376:errorcluster, "Modbus Master out"=w374:refnum<class "Modbus Master.lvclass">)  [unwired: 7 in]
              }
            }
            n131 = Bundle By Name(cluster=w359, "Device Connections.APLUS 7 Modbus Connection"=w360, "Device Connections.Wago ModBus Connection"=w361) -> (w358:T55)
          }
          event "Station Voltage Send 8": Value Change {
            n132 = event-data() -> ()  [unwired: 1 in, 6 out]
            n133 = Unbundle By Name(w381) -> ("Device Connections.APLUS 8 Modbus Connection"=w383:refnum<class "Modbus Master.lvclass">, "Device Connections.Wago ModBus Connection"=w384:refnum<class "Modbus Master.lvclass">)
            n134 = call "RTS Voltage Frequency Selector.vi"("Frequency"="Frequency 8", "Station Number"=u16 8, "Voltage"="Voltage 8", "error in (no error)"=w385, "Modbus Master in"=w384) -> ("error out"=w386:errorcluster, "Modbus master out"=w379:refnum<class "Modbus Master.lvclass">)  [unwired: 5 in]
            n135 = case shown="\"Reset Watt Hours\"" "Wh Reset 8" {
              tunnel: w386 -> [w394 w397]
              tunnel: [w394 w398] -> w390
              tunnel: w383 -> [w393 w396]
              tunnel: [w393 w395] -> w382
              frame "", Default {
              }
              frame "Reset Watt Hours" {
                n136 = call "APLUS Reset WH Coil.vi"("Error In"=w397, "Reset WattHours"=TRUE, "Modbus Master in"=w396) -> ("Error Out"=w398:errorcluster, "Modbus Master out"=w395:refnum<class "Modbus Master.lvclass">)  [unwired: 7 in]
              }
            }
            n137 = Bundle By Name(cluster=w381, "Device Connections.APLUS 8 Modbus Connection"=w382, "Device Connections.Wago ModBus Connection"=w379) -> (w380:T55)
          }
          event "Update Voltage Adjustment Parameters": Value Change {
            n138 = event-data() -> ()  [unwired: 1 in, 6 out]
            n139 = Unbundle By Name(w401) -> ("Device Connections.Wago ModBus Connection"=w405:refnum<class "Modbus Master.lvclass">)
            n140 = call "Wago Update Voltage Adjustment Parameters.vi"("error in (no error)"=w404, "Voltage Adjustment Parameters"="Voltage Adjustment Parameters", "Modbus Master in"=w405) -> ("error out"=w403:errorcluster, "Modbus master out"=w402:refnum<class "Modbus Master.lvclass">)  [unwired: 7 in]
            n141 = Bundle By Name(cluster=w401, "Device Connections.Wago ModBus Connection"=w402) -> (w400:T55)
          }
          event "Room PID Parameters": Value Change {
            n142 = event-data() -> ()  [unwired: 1 in, 6 out]
            n143 = Unbundle By Name(w409) -> ("Device Connections.Wago ModBus Connection"=w411:refnum<class "Modbus Master.lvclass">)
            n144 = call "Wago Room PID Setting SET.vi"("error in (no error)"=w412, "Room PID Settings"="Room PID Settings", "Modbus Master in"=w411) -> ("error out"=w413:errorcluster, "Modbus master out"=w410:refnum<class "Modbus Master.lvclass">)  [unwired: 7 in]
            n145 = Bundle By Name(cluster=w409, "Device Connections.Wago ModBus Connection"=w410) -> (w408:T55)
          }
          event "Reload PID": Value Change {
            # "This will pull the latest saved\nparameters from file"
            n146 = event-data() -> ()  [unwired: 1 in, 6 out]
            n147 = local read "Core System Path"() -> (w424:path)
            n148 = call "Wago Reload PIDs.vi"("Error In"=w422, "Path"=w424) -> ("Error Out"=w421:errorcluster, "Room PID Settings"=w423:T30)  [unwired: 8 in]
            n149 = Unbundle By Name(w416) -> ("Device Connections.Wago ModBus Connection"=w417:refnum<class "Modbus Master.lvclass">)
            n150 = call "Wago Room PID Setting SET.vi"("error in (no error)"=w421, "Room PID Settings"=w423, "Modbus Master in"=w417) -> ("error out"=w420:errorcluster, "Modbus master out"=w419:refnum<class "Modbus Master.lvclass">)  [unwired: 7 in]
            n151 = local write "Room PID Settings"(w423) -> ()
            n152 = Bundle By Name(cluster=w416, "Device Connections.Wago ModBus Connection"=w419) -> (w418:T55)
          }
          event Value Change {
            n153 = event-data() -> ("NewVal"=w432:T35)  [unwired: 1 in, 5 out]
            n154 = Unbundle By Name(w430) -> ("Device Connections.Wago ModBus Connection"=w431:refnum<class "Modbus Master.lvclass">)
            n155 = call "RTS Door Ops CMD.vi"("error in (no error)"=w427, "Door Enable"=w432, "Modbus Master in"=w431) -> ("error out"=w426:errorcluster, "Modbus Master out"=w428:refnum<class "Modbus Master.lvclass">)  [unwired: 7 in]
            n156 = Bundle By Name(cluster=w430, "Device Connections.Wago ModBus Connection"=w428) -> (w429:T55)
            n157 = call <vilib>:"Add State(s) to Queue__jki_lib_state_machine.vi"("State(s) in (\"\")"=w433) -> ("States Out"=w434:string)  [unwired: 14 in]
          }
          event "Station 1 CMD": Value Change {
            w444 = T56 320 items=["fwS1Volt1"=0, "fwS1Volt2"=1, "fwS2Volt1"=2, "fwS2Volt2"=3, "fwS3Volt1"=4, "fwS3Volt2"=5, "fwS4Volt1"=6, "fwS4Volt2"=7, "fwS5Volt1"=8, "fwS5Volt2"=9, "fwS6Volt1"=10, "fwS6Volt2 "=11, "fwS7Volt1"=12, "fwS7Volt2"=13, "fwS8Volt1"=14, "fwS8Volt2"=15, "fwRoomHum"=16, "fwRoomTemp"=17, "fwAISpare1"=18, "fwAISpare2"=19, "fwSuppTemp"=20, "fwCoolTemp"=21, "fwDehumTemp"=22, "fwUnused"=23, "Bool Inputs"=24, "gwVoltRate1"=256, "gwVoltRate2"=257, "gwVoltRate3"=258, "gwVoltRate4"=259, "gwVoltRate5"=260, "gwVoltRate6"=261, "gwVoltRate7"=262, "gwVoltRate8"=263, "gwVoltWindow5/1"=264, "gwVoltWindow6/2"=265, "gwVoltWindow7/3"=266, "gwVoltWindow8/4"=267, "fwVoltSet1"=272, "fwVoltSet2"=273, "fwVoltSet3"=274, "fwVoltSet4"=275, "fwVoltSet5"=276, "fwVoltSet6"=277, "fwVoltSet7"=278, "fwVoltSet8"=279, "fwVoltRng1"=280, "fwVoltRng2"=281, "fwVoltRng3"=282, "fwVoltRng4"=283, "fwVoltRng5"=284, "fwVoltRng6"=285, "fwVoltRng7"=286, "fwVoltRng8"=287, "fwVoltPol1"=296, "fwVoltPol2"=297, "fwVoltPol3"=298, "fwVoltPol4"=299, "fwVoltPol5"=300, "fwVoltPol6"=301, "fwVoltPol7"=302, "fwVoltPol8"=303, "Rm1St1Dr1Cmd"=304, "Rm1St2Dr1Cmd"=305, "Rm1St3Dr1Cmd"=306, "Rm1St4Dr1Cmd"=307, "Rm1St5Dr1Cmd"=308, "Rm1St6Dr1Cmd"=309, "Rm1St7Dr1Cmd"=310, "Rm1St8Dr1Cmd"=311, "Rm1St1Dr2Cmd"=312, "Rm1St2Dr2Cmd"=313, "Rm1St3Dr2Cmd"=314, "Rm1St4Dr2Cmd"=315, "Rm1St5Dr2Cmd"=316, "Rm1St6Dr2Cmd"=317, "Rm1St7Dr2Cmd"=318, "Rm1St8Dr2Cmd"=319, "Rm1St1Dr3Cmd"=320, "Rm1St2Dr3Cmd"=321, "Rm1St3Dr3Cmd"=322, "Rm1St4Dr3Cmd"=323, "Rm1St5Dr3Cmd"=324, "Rm1St6Dr3Cmd"=325, "Rm1St7Dr3Cmd"=326, "Rm1St8Dr3Cmd"=327, "fwRmTempSP"=328, "fwRmHumSP"=329, "fwCoolTempSP"=330, "fwDehumTempSP"=331, "fwRmRun"=332, "fwRmOk"=333, "fwTesting"=334, "fwRmDryP"=335, "fwRmDryI"=336, "fwRmHumP"=337, "fwRmHumI"=338, "fwRmHeatP"=339, "fwRmHeatI"=340, "fwCoolTempP"=341, "fwCoolTempI"=342, "fwDehumTempP"=343, "fwDehumTempI"=344, "fwGndLeak1"=345, "fwGndLeak2"=346, "fwGndLeak3"=347, "fwGndLeak4"=348, "fwGndLeak5"=349, "fwGndLeak6"=350, "fwGndLeak7"=351, "fwGndLeak8"=352, "Rm1OpenerCmd"=353] ("Ring")
            w443 = T56 312 items=["fwS1Volt1"=0, "fwS1Volt2"=1, "fwS2Volt1"=2, "fwS2Volt2"=3, "fwS3Volt1"=4, "fwS3Volt2"=5, "fwS4Volt1"=6, "fwS4Volt2"=7, "fwS5Volt1"=8, "fwS5Volt2"=9, "fwS6Volt1"=10, "fwS6Volt2 "=11, "fwS7Volt1"=12, "fwS7Volt2"=13, "fwS8Volt1"=14, "fwS8Volt2"=15, "fwRoomHum"=16, "fwRoomTemp"=17, "fwAISpare1"=18, "fwAISpare2"=19, "fwSuppTemp"=20, "fwCoolTemp"=21, "fwDehumTemp"=22, "fwUnused"=23, "Bool Inputs"=24, "gwVoltRate1"=256, "gwVoltRate2"=257, "gwVoltRate3"=258, "gwVoltRate4"=259, "gwVoltRate5"=260, "gwVoltRate6"=261, "gwVoltRate7"=262, "gwVoltRate8"=263, "gwVoltWindow5/1"=264, "gwVoltWindow6/2"=265, "gwVoltWindow7/3"=266, "gwVoltWindow8/4"=267, "fwVoltSet1"=272, "fwVoltSet2"=273, "fwVoltSet3"=274, "fwVoltSet4"=275, "fwVoltSet5"=276, "fwVoltSet6"=277, "fwVoltSet7"=278, "fwVoltSet8"=279, "fwVoltRng1"=280, "fwVoltRng2"=281, "fwVoltRng3"=282, "fwVoltRng4"=283, "fwVoltRng5"=284, "fwVoltRng6"=285, "fwVoltRng7"=286, "fwVoltRng8"=287, "fwVoltPol1"=296, "fwVoltPol2"=297, "fwVoltPol3"=298, "fwVoltPol4"=299, "fwVoltPol5"=300, "fwVoltPol6"=301, "fwVoltPol7"=302, "fwVoltPol8"=303, "Rm1St1Dr1Cmd"=304, "Rm1St2Dr1Cmd"=305, "Rm1St3Dr1Cmd"=306, "Rm1St4Dr1Cmd"=307, "Rm1St5Dr1Cmd"=308, "Rm1St6Dr1Cmd"=309, "Rm1St7Dr1Cmd"=310, "Rm1St8Dr1Cmd"=311, "Rm1St1Dr2Cmd"=312, "Rm1St2Dr2Cmd"=313, "Rm1St3Dr2Cmd"=314, "Rm1St4Dr2Cmd"=315, "Rm1St5Dr2Cmd"=316, "Rm1St6Dr2Cmd"=317, "Rm1St7Dr2Cmd"=318, "Rm1St8Dr2Cmd"=319, "Rm1St1Dr3Cmd"=320, "Rm1St2Dr3Cmd"=321, "Rm1St3Dr3Cmd"=322, "Rm1St4Dr3Cmd"=323, "Rm1St5Dr3Cmd"=324, "Rm1St6Dr3Cmd"=325, "Rm1St7Dr3Cmd"=326, "Rm1St8Dr3Cmd"=327, "fwRmTempSP"=328, "fwRmHumSP"=329, "fwCoolTempSP"=330, "fwDehumTempSP"=331, "fwRmRun"=332, "fwRmOk"=333, "fwTesting"=334, "fwRmDryP"=335, "fwRmDryI"=336, "fwRmHumP"=337, "fwRmHumI"=338, "fwRmHeatP"=339, "fwRmHeatI"=340, "fwCoolTempP"=341, "fwCoolTempI"=342, "fwDehumTempP"=343, "fwDehumTempI"=344, "fwGndLeak1"=345, "fwGndLeak2"=346, "fwGndLeak3"=347, "fwGndLeak4"=348, "fwGndLeak5"=349, "fwGndLeak6"=350, "fwGndLeak7"=351, "fwGndLeak8"=352, "Rm1OpenerCmd"=353] ("Ring")
            w442 = T56 304 items=["fwS1Volt1"=0, "fwS1Volt2"=1, "fwS2Volt1"=2, "fwS2Volt2"=3, "fwS3Volt1"=4, "fwS3Volt2"=5, "fwS4Volt1"=6, "fwS4Volt2"=7, "fwS5Volt1"=8, "fwS5Volt2"=9, "fwS6Volt1"=10, "fwS6Volt2 "=11, "fwS7Volt1"=12, "fwS7Volt2"=13, "fwS8Volt1"=14, "fwS8Volt2"=15, "fwRoomHum"=16, "fwRoomTemp"=17, "fwAISpare1"=18, "fwAISpare2"=19, "fwSuppTemp"=20, "fwCoolTemp"=21, "fwDehumTemp"=22, "fwUnused"=23, "Bool Inputs"=24, "gwVoltRate1"=256, "gwVoltRate2"=257, "gwVoltRate3"=258, "gwVoltRate4"=259, "gwVoltRate5"=260, "gwVoltRate6"=261, "gwVoltRate7"=262, "gwVoltRate8"=263, "gwVoltWindow5/1"=264, "gwVoltWindow6/2"=265, "gwVoltWindow7/3"=266, "gwVoltWindow8/4"=267, "fwVoltSet1"=272, "fwVoltSet2"=273, "fwVoltSet3"=274, "fwVoltSet4"=275, "fwVoltSet5"=276, "fwVoltSet6"=277, "fwVoltSet7"=278, "fwVoltSet8"=279, "fwVoltRng1"=280, "fwVoltRng2"=281, "fwVoltRng3"=282, "fwVoltRng4"=283, "fwVoltRng5"=284, "fwVoltRng6"=285, "fwVoltRng7"=286, "fwVoltRng8"=287, "fwVoltPol1"=296, "fwVoltPol2"=297, "fwVoltPol3"=298, "fwVoltPol4"=299, "fwVoltPol5"=300, "fwVoltPol6"=301, "fwVoltPol7"=302, "fwVoltPol8"=303, "Rm1St1Dr1Cmd"=304, "Rm1St2Dr1Cmd"=305, "Rm1St3Dr1Cmd"=306, "Rm1St4Dr1Cmd"=307, "Rm1St5Dr1Cmd"=308, "Rm1St6Dr1Cmd"=309, "Rm1St7Dr1Cmd"=310, "Rm1St8Dr1Cmd"=311, "Rm1St1Dr2Cmd"=312, "Rm1St2Dr2Cmd"=313, "Rm1St3Dr2Cmd"=314, "Rm1St4Dr2Cmd"=315, "Rm1St5Dr2Cmd"=316, "Rm1St6Dr2Cmd"=317, "Rm1St7Dr2Cmd"=318, "Rm1St8Dr2Cmd"=319, "Rm1St1Dr3Cmd"=320, "Rm1St2Dr3Cmd"=321, "Rm1St3Dr3Cmd"=322, "Rm1St4Dr3Cmd"=323, "Rm1St5Dr3Cmd"=324, "Rm1St6Dr3Cmd"=325, "Rm1St7Dr3Cmd"=326, "Rm1St8Dr3Cmd"=327, "fwRmTempSP"=328, "fwRmHumSP"=329, "fwCoolTempSP"=330, "fwDehumTempSP"=331, "fwRmRun"=332, "fwRmOk"=333, "fwTesting"=334, "fwRmDryP"=335, "fwRmDryI"=336, "fwRmHumP"=337, "fwRmHumI"=338, "fwRmHeatP"=339, "fwRmHeatI"=340, "fwCoolTempP"=341, "fwCoolTempI"=342, "fwDehumTempP"=343, "fwDehumTempI"=344, "fwGndLeak1"=345, "fwGndLeak2"=346, "fwGndLeak3"=347, "fwGndLeak4"=348, "fwGndLeak5"=349, "fwGndLeak6"=350, "fwGndLeak7"=351, "fwGndLeak8"=352, "Rm1OpenerCmd"=353] ("Ring")
            n158 = event-data() -> ()  [unwired: 1 in, 6 out]
            n159 = Unbundle By Name(w438) -> ("Device Connections.Wago ModBus Connection"=w440:refnum<class "Modbus Master.lvclass">)
            n160 = Unbundle By Name("Door Settings") -> ("Station 1.Slide"=w451:T34, "Station 1.Cab"=w450:T34, "Station 1.Freezer"=w449:T34)
            n161 = call-dynamic "Write Single Holding Register.vi"("error in"=w439, "register to write"=w449, "address"=w442, "Modbus master in"=w440) -> ("error out"=w445:errorcluster, "Modbus master out"=w447:refnum<class "Modbus Master.lvclass">)  [unwired: 6 in]
            n162 = call-dynamic "Write Single Holding Register.vi"("error in"=w445, "register to write"=w450, "address"=w443, "Modbus master in"=w447) -> ("error out"=w446:errorcluster, "Modbus master out"=w448:refnum<class "Modbus Master.lvclass">)  [unwired: 6 in]
            n163 = call-dynamic "Write Single Holding Register.vi"("error in"=w446, "register to write"=w451, "address"=w444, "Modbus master in"=w448) -> ("error out"=w435:errorcluster, "Modbus master out"=w436:refnum<class "Modbus Master.lvclass">)  [unwired: 6 in]
            n164 = Bundle By Name(cluster=w438, "Device Connections.Wago ModBus Connection"=w436) -> (w437:T55)
          }
          event "Station 2 CMD": Value Change {
            w467 = T56 321 items=["fwS1Volt1"=0, "fwS1Volt2"=1, "fwS2Volt1"=2, "fwS2Volt2"=3, "fwS3Volt1"=4, "fwS3Volt2"=5, "fwS4Volt1"=6, "fwS4Volt2"=7, "fwS5Volt1"=8, "fwS5Volt2"=9, "fwS6Volt1"=10, "fwS6Volt2 "=11, "fwS7Volt1"=12, "fwS7Volt2"=13, "fwS8Volt1"=14, "fwS8Volt2"=15, "fwRoomHum"=16, "fwRoomTemp"=17, "fwAISpare1"=18, "fwAISpare2"=19, "fwSuppTemp"=20, "fwCoolTemp"=21, "fwDehumTemp"=22, "fwUnused"=23, "Bool Inputs"=24, "gwVoltRate1"=256, "gwVoltRate2"=257, "gwVoltRate3"=258, "gwVoltRate4"=259, "gwVoltRate5"=260, "gwVoltRate6"=261, "gwVoltRate7"=262, "gwVoltRate8"=263, "gwVoltWindow5/1"=264, "gwVoltWindow6/2"=265, "gwVoltWindow7/3"=266, "gwVoltWindow8/4"=267, "fwVoltSet1"=272, "fwVoltSet2"=273, "fwVoltSet3"=274, "fwVoltSet4"=275, "fwVoltSet5"=276, "fwVoltSet6"=277, "fwVoltSet7"=278, "fwVoltSet8"=279, "fwVoltRng1"=280, "fwVoltRng2"=281, "fwVoltRng3"=282, "fwVoltRng4"=283, "fwVoltRng5"=284, "fwVoltRng6"=285, "fwVoltRng7"=286, "fwVoltRng8"=287, "fwVoltPol1"=296, "fwVoltPol2"=297, "fwVoltPol3"=298, "fwVoltPol4"=299, "fwVoltPol5"=300, "fwVoltPol6"=301, "fwVoltPol7"=302, "fwVoltPol8"=303, "Rm1St1Dr1Cmd"=304, "Rm1St2Dr1Cmd"=305, "Rm1St3Dr1Cmd"=306, "Rm1St4Dr1Cmd"=307, "Rm1St5Dr1Cmd"=308, "Rm1St6Dr1Cmd"=309, "Rm1St7Dr1Cmd"=310, "Rm1St8Dr1Cmd"=311, "Rm1St1Dr2Cmd"=312, "Rm1St2Dr2Cmd"=313, "Rm1St3Dr2Cmd"=314, "Rm1St4Dr2Cmd"=315, "Rm1St5Dr2Cmd"=316, "Rm1St6Dr2Cmd"=317, "Rm1St7Dr2Cmd"=318, "Rm1St8Dr2Cmd"=319, "Rm1St1Dr3Cmd"=320, "Rm1St2Dr3Cmd"=321, "Rm1St3Dr3Cmd"=322, "Rm1St4Dr3Cmd"=323, "Rm1St5Dr3Cmd"=324, "Rm1St6Dr3Cmd"=325, "Rm1St7Dr3Cmd"=326, "Rm1St8Dr3Cmd"=327, "fwRmTempSP"=328, "fwRmHumSP"=329, "fwCoolTempSP"=330, "fwDehumTempSP"=331, "fwRmRun"=332, "fwRmOk"=333, "fwTesting"=334, "fwRmDryP"=335, "fwRmDryI"=336, "fwRmHumP"=337, "fwRmHumI"=338, "fwRmHeatP"=339, "fwRmHeatI"=340, "fwCoolTempP"=341, "fwCoolTempI"=342, "fwDehumTempP"=343, "fwDehumTempI"=344, "fwGndLeak1"=345, "fwGndLeak2"=346, "fwGndLeak3"=347, "fwGndLeak4"=348, "fwGndLeak5"=349, "fwGndLeak6"=350, "fwGndLeak7"=351, "fwGndLeak8"=352, "Rm1OpenerCmd"=353] ("Ring")
            w468 = T56 313 items=["fwS1Volt1"=0, "fwS1Volt2"=1, "fwS2Volt1"=2, "fwS2Volt2"=3, "fwS3Volt1"=4, "fwS3Volt2"=5, "fwS4Volt1"=6, "fwS4Volt2"=7, "fwS5Volt1"=8, "fwS5Volt2"=9, "fwS6Volt1"=10, "fwS6Volt2 "=11, "fwS7Volt1"=12, "fwS7Volt2"=13, "fwS8Volt1"=14, "fwS8Volt2"=15, "fwRoomHum"=16, "fwRoomTemp"=17, "fwAISpare1"=18, "fwAISpare2"=19, "fwSuppTemp"=20, "fwCoolTemp"=21, "fwDehumTemp"=22, "fwUnused"=23, "Bool Inputs"=24, "gwVoltRate1"=256, "gwVoltRate2"=257, "gwVoltRate3"=258, "gwVoltRate4"=259, "gwVoltRate5"=260, "gwVoltRate6"=261, "gwVoltRate7"=262, "gwVoltRate8"=263, "gwVoltWindow5/1"=264, "gwVoltWindow6/2"=265, "gwVoltWindow7/3"=266, "gwVoltWindow8/4"=267, "fwVoltSet1"=272, "fwVoltSet2"=273, "fwVoltSet3"=274, "fwVoltSet4"=275, "fwVoltSet5"=276, "fwVoltSet6"=277, "fwVoltSet7"=278, "fwVoltSet8"=279, "fwVoltRng1"=280, "fwVoltRng2"=281, "fwVoltRng3"=282, "fwVoltRng4"=283, "fwVoltRng5"=284, "fwVoltRng6"=285, "fwVoltRng7"=286, "fwVoltRng8"=287, "fwVoltPol1"=296, "fwVoltPol2"=297, "fwVoltPol3"=298, "fwVoltPol4"=299, "fwVoltPol5"=300, "fwVoltPol6"=301, "fwVoltPol7"=302, "fwVoltPol8"=303, "Rm1St1Dr1Cmd"=304, "Rm1St2Dr1Cmd"=305, "Rm1St3Dr1Cmd"=306, "Rm1St4Dr1Cmd"=307, "Rm1St5Dr1Cmd"=308, "Rm1St6Dr1Cmd"=309, "Rm1St7Dr1Cmd"=310, "Rm1St8Dr1Cmd"=311, "Rm1St1Dr2Cmd"=312, "Rm1St2Dr2Cmd"=313, "Rm1St3Dr2Cmd"=314, "Rm1St4Dr2Cmd"=315, "Rm1St5Dr2Cmd"=316, "Rm1St6Dr2Cmd"=317, "Rm1St7Dr2Cmd"=318, "Rm1St8Dr2Cmd"=319, "Rm1St1Dr3Cmd"=320, "Rm1St2Dr3Cmd"=321, "Rm1St3Dr3Cmd"=322, "Rm1St4Dr3Cmd"=323, "Rm1St5Dr3Cmd"=324, "Rm1St6Dr3Cmd"=325, "Rm1St7Dr3Cmd"=326, "Rm1St8Dr3Cmd"=327, "fwRmTempSP"=328, "fwRmHumSP"=329, "fwCoolTempSP"=330, "fwDehumTempSP"=331, "fwRmRun"=332, "fwRmOk"=333, "fwTesting"=334, "fwRmDryP"=335, "fwRmDryI"=336, "fwRmHumP"=337, "fwRmHumI"=338, "fwRmHeatP"=339, "fwRmHeatI"=340, "fwCoolTempP"=341, "fwCoolTempI"=342, "fwDehumTempP"=343, "fwDehumTempI"=344, "fwGndLeak1"=345, "fwGndLeak2"=346, "fwGndLeak3"=347, "fwGndLeak4"=348, "fwGndLeak5"=349, "fwGndLeak6"=350, "fwGndLeak7"=351, "fwGndLeak8"=352, "Rm1OpenerCmd"=353] ("Ring")
            w469 = T56 305 items=["fwS1Volt1"=0, "fwS1Volt2"=1, "fwS2Volt1"=2, "fwS2Volt2"=3, "fwS3Volt1"=4, "fwS3Volt2"=5, "fwS4Volt1"=6, "fwS4Volt2"=7, "fwS5Volt1"=8, "fwS5Volt2"=9, "fwS6Volt1"=10, "fwS6Volt2 "=11, "fwS7Volt1"=12, "fwS7Volt2"=13, "fwS8Volt1"=14, "fwS8Volt2"=15, "fwRoomHum"=16, "fwRoomTemp"=17, "fwAISpare1"=18, "fwAISpare2"=19, "fwSuppTemp"=20, "fwCoolTemp"=21, "fwDehumTemp"=22, "fwUnused"=23, "Bool Inputs"=24, "gwVoltRate1"=256, "gwVoltRate2"=257, "gwVoltRate3"=258, "gwVoltRate4"=259, "gwVoltRate5"=260, "gwVoltRate6"=261, "gwVoltRate7"=262, "gwVoltRate8"=263, "gwVoltWindow5/1"=264, "gwVoltWindow6/2"=265, "gwVoltWindow7/3"=266, "gwVoltWindow8/4"=267, "fwVoltSet1"=272, "fwVoltSet2"=273, "fwVoltSet3"=274, "fwVoltSet4"=275, "fwVoltSet5"=276, "fwVoltSet6"=277, "fwVoltSet7"=278, "fwVoltSet8"=279, "fwVoltRng1"=280, "fwVoltRng2"=281, "fwVoltRng3"=282, "fwVoltRng4"=283, "fwVoltRng5"=284, "fwVoltRng6"=285, "fwVoltRng7"=286, "fwVoltRng8"=287, "fwVoltPol1"=296, "fwVoltPol2"=297, "fwVoltPol3"=298, "fwVoltPol4"=299, "fwVoltPol5"=300, "fwVoltPol6"=301, "fwVoltPol7"=302, "fwVoltPol8"=303, "Rm1St1Dr1Cmd"=304, "Rm1St2Dr1Cmd"=305, "Rm1St3Dr1Cmd"=306, "Rm1St4Dr1Cmd"=307, "Rm1St5Dr1Cmd"=308, "Rm1St6Dr1Cmd"=309, "Rm1St7Dr1Cmd"=310, "Rm1St8Dr1Cmd"=311, "Rm1St1Dr2Cmd"=312, "Rm1St2Dr2Cmd"=313, "Rm1St3Dr2Cmd"=314, "Rm1St4Dr2Cmd"=315, "Rm1St5Dr2Cmd"=316, "Rm1St6Dr2Cmd"=317, "Rm1St7Dr2Cmd"=318, "Rm1St8Dr2Cmd"=319, "Rm1St1Dr3Cmd"=320, "Rm1St2Dr3Cmd"=321, "Rm1St3Dr3Cmd"=322, "Rm1St4Dr3Cmd"=323, "Rm1St5Dr3Cmd"=324, "Rm1St6Dr3Cmd"=325, "Rm1St7Dr3Cmd"=326, "Rm1St8Dr3Cmd"=327, "fwRmTempSP"=328, "fwRmHumSP"=329, "fwCoolTempSP"=330, "fwDehumTempSP"=331, "fwRmRun"=332, "fwRmOk"=333, "fwTesting"=334, "fwRmDryP"=335, "fwRmDryI"=336, "fwRmHumP"=337, "fwRmHumI"=338, "fwRmHeatP"=339, "fwRmHeatI"=340, "fwCoolTempP"=341, "fwCoolTempI"=342, "fwDehumTempP"=343, "fwDehumTempI"=344, "fwGndLeak1"=345, "fwGndLeak2"=346, "fwGndLeak3"=347, "fwGndLeak4"=348, "fwGndLeak5"=349, "fwGndLeak6"=350, "fwGndLeak7"=351, "fwGndLeak8"=352, "Rm1OpenerCmd"=353] ("Ring")
            n165 = event-data() -> ()  [unwired: 1 in, 6 out]
            n166 = local read "Door Settings"() -> (w457:T32)
            n167 = Unbundle By Name(w455) -> ("Device Connections.Wago ModBus Connection"=w453:refnum<class "Modbus Master.lvclass">)
            n168 = Unbundle By Name(w457) -> ("Station 2.Slide"=w462:T34, "Station 2.Cab"=w463:T34, "Station 2.Freezer"=w464:T34)
            n169 = call-dynamic "Write Single Holding Register.vi"("error in"=w459, "register to write"=w464, "address"=w469, "Modbus master in"=w453) -> ("error out"=w461:errorcluster, "Modbus master out"=w466:refnum<class "Modbus Master.lvclass">)  [unwired: 6 in]
            n170 = call-dynamic "Write Single Holding Register.vi"("error in"=w461, "register to write"=w463, "address"=w468, "Modbus master in"=w466) -> ("error out"=w460:errorcluster, "Modbus master out"=w465:refnum<class "Modbus Master.lvclass">)  [unwired: 6 in]
            n171 = call-dynamic "Write Single Holding Register.vi"("error in"=w460, "register to write"=w462, "address"=w467, "Modbus master in"=w465) -> ("error out"=w458:errorcluster, "Modbus master out"=w456:refnum<class "Modbus Master.lvclass">)  [unwired: 6 in]
            n172 = Bundle By Name(cluster=w455, "Device Connections.Wago ModBus Connection"=w456) -> (w454:T55)
          }
          event "Station 3 CMD": Value Change {
            w481 = T56 322 items=["fwS1Volt1"=0, "fwS1Volt2"=1, "fwS2Volt1"=2, "fwS2Volt2"=3, "fwS3Volt1"=4, "fwS3Volt2"=5, "fwS4Volt1"=6, "fwS4Volt2"=7, "fwS5Volt1"=8, "fwS5Volt2"=9, "fwS6Volt1"=10, "fwS6Volt2 "=11, "fwS7Volt1"=12, "fwS7Volt2"=13, "fwS8Volt1"=14, "fwS8Volt2"=15, "fwRoomHum"=16, "fwRoomTemp"=17, "fwAISpare1"=18, "fwAISpare2"=19, "fwSuppTemp"=20, "fwCoolTemp"=21, "fwDehumTemp"=22, "fwUnused"=23, "Bool Inputs"=24, "gwVoltRate1"=256, "gwVoltRate2"=257, "gwVoltRate3"=258, "gwVoltRate4"=259, "gwVoltRate5"=260, "gwVoltRate6"=261, "gwVoltRate7"=262, "gwVoltRate8"=263, "gwVoltWindow5/1"=264, "gwVoltWindow6/2"=265, "gwVoltWindow7/3"=266, "gwVoltWindow8/4"=267, "fwVoltSet1"=272, "fwVoltSet2"=273, "fwVoltSet3"=274, "fwVoltSet4"=275, "fwVoltSet5"=276, "fwVoltSet6"=277, "fwVoltSet7"=278, "fwVoltSet8"=279, "fwVoltRng1"=280, "fwVoltRng2"=281, "fwVoltRng3"=282, "fwVoltRng4"=283, "fwVoltRng5"=284, "fwVoltRng6"=285, "fwVoltRng7"=286, "fwVoltRng8"=287, "fwVoltPol1"=296, "fwVoltPol2"=297, "fwVoltPol3"=298, "fwVoltPol4"=299, "fwVoltPol5"=300, "fwVoltPol6"=301, "fwVoltPol7"=302, "fwVoltPol8"=303, "Rm1St1Dr1Cmd"=304, "Rm1St2Dr1Cmd"=305, "Rm1St3Dr1Cmd"=306, "Rm1St4Dr1Cmd"=307, "Rm1St5Dr1Cmd"=308, "Rm1St6Dr1Cmd"=309, "Rm1St7Dr1Cmd"=310, "Rm1St8Dr1Cmd"=311, "Rm1St1Dr2Cmd"=312, "Rm1St2Dr2Cmd"=313, "Rm1St3Dr2Cmd"=314, "Rm1St4Dr2Cmd"=315, "Rm1St5Dr2Cmd"=316, "Rm1St6Dr2Cmd"=317, "Rm1St7Dr2Cmd"=318, "Rm1St8Dr2Cmd"=319, "Rm1St1Dr3Cmd"=320, "Rm1St2Dr3Cmd"=321, "Rm1St3Dr3Cmd"=322, "Rm1St4Dr3Cmd"=323, "Rm1St5Dr3Cmd"=324, "Rm1St6Dr3Cmd"=325, "Rm1St7Dr3Cmd"=326, "Rm1St8Dr3Cmd"=327, "fwRmTempSP"=328, "fwRmHumSP"=329, "fwCoolTempSP"=330, "fwDehumTempSP"=331, "fwRmRun"=332, "fwRmOk"=333, "fwTesting"=334, "fwRmDryP"=335, "fwRmDryI"=336, "fwRmHumP"=337, "fwRmHumI"=338, "fwRmHeatP"=339, "fwRmHeatI"=340, "fwCoolTempP"=341, "fwCoolTempI"=342, "fwDehumTempP"=343, "fwDehumTempI"=344, "fwGndLeak1"=345, "fwGndLeak2"=346, "fwGndLeak3"=347, "fwGndLeak4"=348, "fwGndLeak5"=349, "fwGndLeak6"=350, "fwGndLeak7"=351, "fwGndLeak8"=352, "Rm1OpenerCmd"=353] ("Ring")
            w482 = T56 314 items=["fwS1Volt1"=0, "fwS1Volt2"=1, "fwS2Volt1"=2, "fwS2Volt2"=3, "fwS3Volt1"=4, "fwS3Volt2"=5, "fwS4Volt1"=6, "fwS4Volt2"=7, "fwS5Volt1"=8, "fwS5Volt2"=9, "fwS6Volt1"=10, "fwS6Volt2 "=11, "fwS7Volt1"=12, "fwS7Volt2"=13, "fwS8Volt1"=14, "fwS8Volt2"=15, "fwRoomHum"=16, "fwRoomTemp"=17, "fwAISpare1"=18, "fwAISpare2"=19, "fwSuppTemp"=20, "fwCoolTemp"=21, "fwDehumTemp"=22, "fwUnused"=23, "Bool Inputs"=24, "gwVoltRate1"=256, "gwVoltRate2"=257, "gwVoltRate3"=258, "gwVoltRate4"=259, "gwVoltRate5"=260, "gwVoltRate6"=261, "gwVoltRate7"=262, "gwVoltRate8"=263, "gwVoltWindow5/1"=264, "gwVoltWindow6/2"=265, "gwVoltWindow7/3"=266, "gwVoltWindow8/4"=267, "fwVoltSet1"=272, "fwVoltSet2"=273, "fwVoltSet3"=274, "fwVoltSet4"=275, "fwVoltSet5"=276, "fwVoltSet6"=277, "fwVoltSet7"=278, "fwVoltSet8"=279, "fwVoltRng1"=280, "fwVoltRng2"=281, "fwVoltRng3"=282, "fwVoltRng4"=283, "fwVoltRng5"=284, "fwVoltRng6"=285, "fwVoltRng7"=286, "fwVoltRng8"=287, "fwVoltPol1"=296, "fwVoltPol2"=297, "fwVoltPol3"=298, "fwVoltPol4"=299, "fwVoltPol5"=300, "fwVoltPol6"=301, "fwVoltPol7"=302, "fwVoltPol8"=303, "Rm1St1Dr1Cmd"=304, "Rm1St2Dr1Cmd"=305, "Rm1St3Dr1Cmd"=306, "Rm1St4Dr1Cmd"=307, "Rm1St5Dr1Cmd"=308, "Rm1St6Dr1Cmd"=309, "Rm1St7Dr1Cmd"=310, "Rm1St8Dr1Cmd"=311, "Rm1St1Dr2Cmd"=312, "Rm1St2Dr2Cmd"=313, "Rm1St3Dr2Cmd"=314, "Rm1St4Dr2Cmd"=315, "Rm1St5Dr2Cmd"=316, "Rm1St6Dr2Cmd"=317, "Rm1St7Dr2Cmd"=318, "Rm1St8Dr2Cmd"=319, "Rm1St1Dr3Cmd"=320, "Rm1St2Dr3Cmd"=321, "Rm1St3Dr3Cmd"=322, "Rm1St4Dr3Cmd"=323, "Rm1St5Dr3Cmd"=324, "Rm1St6Dr3Cmd"=325, "Rm1St7Dr3Cmd"=326, "Rm1St8Dr3Cmd"=327, "fwRmTempSP"=328, "fwRmHumSP"=329, "fwCoolTempSP"=330, "fwDehumTempSP"=331, "fwRmRun"=332, "fwRmOk"=333, "fwTesting"=334, "fwRmDryP"=335, "fwRmDryI"=336, "fwRmHumP"=337, "fwRmHumI"=338, "fwRmHeatP"=339, "fwRmHeatI"=340, "fwCoolTempP"=341, "fwCoolTempI"=342, "fwDehumTempP"=343, "fwDehumTempI"=344, "fwGndLeak1"=345, "fwGndLeak2"=346, "fwGndLeak3"=347, "fwGndLeak4"=348, "fwGndLeak5"=349, "fwGndLeak6"=350, "fwGndLeak7"=351, "fwGndLeak8"=352, "Rm1OpenerCmd"=353] ("Ring")
            w487 = T56 306 items=["fwS1Volt1"=0, "fwS1Volt2"=1, "fwS2Volt1"=2, "fwS2Volt2"=3, "fwS3Volt1"=4, "fwS3Volt2"=5, "fwS4Volt1"=6, "fwS4Volt2"=7, "fwS5Volt1"=8, "fwS5Volt2"=9, "fwS6Volt1"=10, "fwS6Volt2 "=11, "fwS7Volt1"=12, "fwS7Volt2"=13, "fwS8Volt1"=14, "fwS8Volt2"=15, "fwRoomHum"=16, "fwRoomTemp"=17, "fwAISpare1"=18, "fwAISpare2"=19, "fwSuppTemp"=20, "fwCoolTemp"=21, "fwDehumTemp"=22, "fwUnused"=23, "Bool Inputs"=24, "gwVoltRate1"=256, "gwVoltRate2"=257, "gwVoltRate3"=258, "gwVoltRate4"=259, "gwVoltRate5"=260, "gwVoltRate6"=261, "gwVoltRate7"=262, "gwVoltRate8"=263, "gwVoltWindow5/1"=264, "gwVoltWindow6/2"=265, "gwVoltWindow7/3"=266, "gwVoltWindow8/4"=267, "fwVoltSet1"=272, "fwVoltSet2"=273, "fwVoltSet3"=274, "fwVoltSet4"=275, "fwVoltSet5"=276, "fwVoltSet6"=277, "fwVoltSet7"=278, "fwVoltSet8"=279, "fwVoltRng1"=280, "fwVoltRng2"=281, "fwVoltRng3"=282, "fwVoltRng4"=283, "fwVoltRng5"=284, "fwVoltRng6"=285, "fwVoltRng7"=286, "fwVoltRng8"=287, "fwVoltPol1"=296, "fwVoltPol2"=297, "fwVoltPol3"=298, "fwVoltPol4"=299, "fwVoltPol5"=300, "fwVoltPol6"=301, "fwVoltPol7"=302, "fwVoltPol8"=303, "Rm1St1Dr1Cmd"=304, "Rm1St2Dr1Cmd"=305, "Rm1St3Dr1Cmd"=306, "Rm1St4Dr1Cmd"=307, "Rm1St5Dr1Cmd"=308, "Rm1St6Dr1Cmd"=309, "Rm1St7Dr1Cmd"=310, "Rm1St8Dr1Cmd"=311, "Rm1St1Dr2Cmd"=312, "Rm1St2Dr2Cmd"=313, "Rm1St3Dr2Cmd"=314, "Rm1St4Dr2Cmd"=315, "Rm1St5Dr2Cmd"=316, "Rm1St6Dr2Cmd"=317, "Rm1St7Dr2Cmd"=318, "Rm1St8Dr2Cmd"=319, "Rm1St1Dr3Cmd"=320, "Rm1St2Dr3Cmd"=321, "Rm1St3Dr3Cmd"=322, "Rm1St4Dr3Cmd"=323, "Rm1St5Dr3Cmd"=324, "Rm1St6Dr3Cmd"=325, "Rm1St7Dr3Cmd"=326, "Rm1St8Dr3Cmd"=327, "fwRmTempSP"=328, "fwRmHumSP"=329, "fwCoolTempSP"=330, "fwDehumTempSP"=331, "fwRmRun"=332, "fwRmOk"=333, "fwTesting"=334, "fwRmDryP"=335, "fwRmDryI"=336, "fwRmHumP"=337, "fwRmHumI"=338, "fwRmHeatP"=339, "fwRmHeatI"=340, "fwCoolTempP"=341, "fwCoolTempI"=342, "fwDehumTempP"=343, "fwDehumTempI"=344, "fwGndLeak1"=345, "fwGndLeak2"=346, "fwGndLeak3"=347, "fwGndLeak4"=348, "fwGndLeak5"=349, "fwGndLeak6"=350, "fwGndLeak7"=351, "fwGndLeak8"=352, "Rm1OpenerCmd"=353] ("Ring")
            n173 = event-data() -> ()  [unwired: 1 in, 6 out]
            n174 = local read "Door Settings"() -> (w471:T32)
            n175 = Unbundle By Name(w475) -> ("Device Connections.Wago ModBus Connection"=w477:refnum<class "Modbus Master.lvclass">)
            n176 = Unbundle By Name(w471) -> ("Station 3.Slide"=w483:T34, "Station 3.Cab"=w484:T34, "Station 3.Freezer"=w485:T34)
            n177 = call-dynamic "Write Single Holding Register.vi"("error in"=w476, "register to write"=w485, "address"=w487, "Modbus master in"=w477) -> ("error out"=w479:errorcluster, "Modbus master out"=w486:refnum<class "Modbus Master.lvclass">)  [unwired: 6 in]
            n178 = call-dynamic "Write Single Holding Register.vi"("error in"=w479, "register to write"=w484, "address"=w482, "Modbus master in"=w486) -> ("error out"=w478:errorcluster, "Modbus master out"=w480:refnum<class "Modbus Master.lvclass">)  [unwired: 6 in]
            n179 = call-dynamic "Write Single Holding Register.vi"("error in"=w478, "register to write"=w483, "address"=w481, "Modbus master in"=w480) -> ("error out"=w472:errorcluster, "Modbus master out"=w473:refnum<class "Modbus Master.lvclass">)  [unwired: 6 in]
            n180 = Bundle By Name(cluster=w475, "Device Connections.Wago ModBus Connection"=w473) -> (w474:T55)
          }
          event "Station 4 CMD": Value Change {
            w503 = T56 323 items=["fwS1Volt1"=0, "fwS1Volt2"=1, "fwS2Volt1"=2, "fwS2Volt2"=3, "fwS3Volt1"=4, "fwS3Volt2"=5, "fwS4Volt1"=6, "fwS4Volt2"=7, "fwS5Volt1"=8, "fwS5Volt2"=9, "fwS6Volt1"=10, "fwS6Volt2 "=11, "fwS7Volt1"=12, "fwS7Volt2"=13, "fwS8Volt1"=14, "fwS8Volt2"=15, "fwRoomHum"=16, "fwRoomTemp"=17, "fwAISpare1"=18, "fwAISpare2"=19, "fwSuppTemp"=20, "fwCoolTemp"=21, "fwDehumTemp"=22, "fwUnused"=23, "Bool Inputs"=24, "gwVoltRate1"=256, "gwVoltRate2"=257, "gwVoltRate3"=258, "gwVoltRate4"=259, "gwVoltRate5"=260, "gwVoltRate6"=261, "gwVoltRate7"=262, "gwVoltRate8"=263, "gwVoltWindow5/1"=264, "gwVoltWindow6/2"=265, "gwVoltWindow7/3"=266, "gwVoltWindow8/4"=267, "fwVoltSet1"=272, "fwVoltSet2"=273, "fwVoltSet3"=274, "fwVoltSet4"=275, "fwVoltSet5"=276, "fwVoltSet6"=277, "fwVoltSet7"=278, "fwVoltSet8"=279, "fwVoltRng1"=280, "fwVoltRng2"=281, "fwVoltRng3"=282, "fwVoltRng4"=283, "fwVoltRng5"=284, "fwVoltRng6"=285, "fwVoltRng7"=286, "fwVoltRng8"=287, "fwVoltPol1"=296, "fwVoltPol2"=297, "fwVoltPol3"=298, "fwVoltPol4"=299, "fwVoltPol5"=300, "fwVoltPol6"=301, "fwVoltPol7"=302, "fwVoltPol8"=303, "Rm1St1Dr1Cmd"=304, "Rm1St2Dr1Cmd"=305, "Rm1St3Dr1Cmd"=306, "Rm1St4Dr1Cmd"=307, "Rm1St5Dr1Cmd"=308, "Rm1St6Dr1Cmd"=309, "Rm1St7Dr1Cmd"=310, "Rm1St8Dr1Cmd"=311, "Rm1St1Dr2Cmd"=312, "Rm1St2Dr2Cmd"=313, "Rm1St3Dr2Cmd"=314, "Rm1St4Dr2Cmd"=315, "Rm1St5Dr2Cmd"=316, "Rm1St6Dr2Cmd"=317, "Rm1St7Dr2Cmd"=318, "Rm1St8Dr2Cmd"=319, "Rm1St1Dr3Cmd"=320, "Rm1St2Dr3Cmd"=321, "Rm1St3Dr3Cmd"=322, "Rm1St4Dr3Cmd"=323, "Rm1St5Dr3Cmd"=324, "Rm1St6Dr3Cmd"=325, "Rm1St7Dr3Cmd"=326, "Rm1St8Dr3Cmd"=327, "fwRmTempSP"=328, "fwRmHumSP"=329, "fwCoolTempSP"=330, "fwDehumTempSP"=331, "fwRmRun"=332, "fwRmOk"=333, "fwTesting"=334, "fwRmDryP"=335, "fwRmDryI"=336, "fwRmHumP"=337, "fwRmHumI"=338, "fwRmHeatP"=339, "fwRmHeatI"=340, "fwCoolTempP"=341, "fwCoolTempI"=342, "fwDehumTempP"=343, "fwDehumTempI"=344, "fwGndLeak1"=345, "fwGndLeak2"=346, "fwGndLeak3"=347, "fwGndLeak4"=348, "fwGndLeak5"=349, "fwGndLeak6"=350, "fwGndLeak7"=351, "fwGndLeak8"=352, "Rm1OpenerCmd"=353] ("Ring")
            w504 = T56 315 items=["fwS1Volt1"=0, "fwS1Volt2"=1, "fwS2Volt1"=2, "fwS2Volt2"=3, "fwS3Volt1"=4, "fwS3Volt2"=5, "fwS4Volt1"=6, "fwS4Volt2"=7, "fwS5Volt1"=8, "fwS5Volt2"=9, "fwS6Volt1"=10, "fwS6Volt2 "=11, "fwS7Volt1"=12, "fwS7Volt2"=13, "fwS8Volt1"=14, "fwS8Volt2"=15, "fwRoomHum"=16, "fwRoomTemp"=17, "fwAISpare1"=18, "fwAISpare2"=19, "fwSuppTemp"=20, "fwCoolTemp"=21, "fwDehumTemp"=22, "fwUnused"=23, "Bool Inputs"=24, "gwVoltRate1"=256, "gwVoltRate2"=257, "gwVoltRate3"=258, "gwVoltRate4"=259, "gwVoltRate5"=260, "gwVoltRate6"=261, "gwVoltRate7"=262, "gwVoltRate8"=263, "gwVoltWindow5/1"=264, "gwVoltWindow6/2"=265, "gwVoltWindow7/3"=266, "gwVoltWindow8/4"=267, "fwVoltSet1"=272, "fwVoltSet2"=273, "fwVoltSet3"=274, "fwVoltSet4"=275, "fwVoltSet5"=276, "fwVoltSet6"=277, "fwVoltSet7"=278, "fwVoltSet8"=279, "fwVoltRng1"=280, "fwVoltRng2"=281, "fwVoltRng3"=282, "fwVoltRng4"=283, "fwVoltRng5"=284, "fwVoltRng6"=285, "fwVoltRng7"=286, "fwVoltRng8"=287, "fwVoltPol1"=296, "fwVoltPol2"=297, "fwVoltPol3"=298, "fwVoltPol4"=299, "fwVoltPol5"=300, "fwVoltPol6"=301, "fwVoltPol7"=302, "fwVoltPol8"=303, "Rm1St1Dr1Cmd"=304, "Rm1St2Dr1Cmd"=305, "Rm1St3Dr1Cmd"=306, "Rm1St4Dr1Cmd"=307, "Rm1St5Dr1Cmd"=308, "Rm1St6Dr1Cmd"=309, "Rm1St7Dr1Cmd"=310, "Rm1St8Dr1Cmd"=311, "Rm1St1Dr2Cmd"=312, "Rm1St2Dr2Cmd"=313, "Rm1St3Dr2Cmd"=314, "Rm1St4Dr2Cmd"=315, "Rm1St5Dr2Cmd"=316, "Rm1St6Dr2Cmd"=317, "Rm1St7Dr2Cmd"=318, "Rm1St8Dr2Cmd"=319, "Rm1St1Dr3Cmd"=320, "Rm1St2Dr3Cmd"=321, "Rm1St3Dr3Cmd"=322, "Rm1St4Dr3Cmd"=323, "Rm1St5Dr3Cmd"=324, "Rm1St6Dr3Cmd"=325, "Rm1St7Dr3Cmd"=326, "Rm1St8Dr3Cmd"=327, "fwRmTempSP"=328, "fwRmHumSP"=329, "fwCoolTempSP"=330, "fwDehumTempSP"=331, "fwRmRun"=332, "fwRmOk"=333, "fwTesting"=334, "fwRmDryP"=335, "fwRmDryI"=336, "fwRmHumP"=337, "fwRmHumI"=338, "fwRmHeatP"=339, "fwRmHeatI"=340, "fwCoolTempP"=341, "fwCoolTempI"=342, "fwDehumTempP"=343, "fwDehumTempI"=344, "fwGndLeak1"=345, "fwGndLeak2"=346, "fwGndLeak3"=347, "fwGndLeak4"=348, "fwGndLeak5"=349, "fwGndLeak6"=350, "fwGndLeak7"=351, "fwGndLeak8"=352, "Rm1OpenerCmd"=353] ("Ring")
            w505 = T56 307 items=["fwS1Volt1"=0, "fwS1Volt2"=1, "fwS2Volt1"=2, "fwS2Volt2"=3, "fwS3Volt1"=4, "fwS3Volt2"=5, "fwS4Volt1"=6, "fwS4Volt2"=7, "fwS5Volt1"=8, "fwS5Volt2"=9, "fwS6Volt1"=10, "fwS6Volt2 "=11, "fwS7Volt1"=12, "fwS7Volt2"=13, "fwS8Volt1"=14, "fwS8Volt2"=15, "fwRoomHum"=16, "fwRoomTemp"=17, "fwAISpare1"=18, "fwAISpare2"=19, "fwSuppTemp"=20, "fwCoolTemp"=21, "fwDehumTemp"=22, "fwUnused"=23, "Bool Inputs"=24, "gwVoltRate1"=256, "gwVoltRate2"=257, "gwVoltRate3"=258, "gwVoltRate4"=259, "gwVoltRate5"=260, "gwVoltRate6"=261, "gwVoltRate7"=262, "gwVoltRate8"=263, "gwVoltWindow5/1"=264, "gwVoltWindow6/2"=265, "gwVoltWindow7/3"=266, "gwVoltWindow8/4"=267, "fwVoltSet1"=272, "fwVoltSet2"=273, "fwVoltSet3"=274, "fwVoltSet4"=275, "fwVoltSet5"=276, "fwVoltSet6"=277, "fwVoltSet7"=278, "fwVoltSet8"=279, "fwVoltRng1"=280, "fwVoltRng2"=281, "fwVoltRng3"=282, "fwVoltRng4"=283, "fwVoltRng5"=284, "fwVoltRng6"=285, "fwVoltRng7"=286, "fwVoltRng8"=287, "fwVoltPol1"=296, "fwVoltPol2"=297, "fwVoltPol3"=298, "fwVoltPol4"=299, "fwVoltPol5"=300, "fwVoltPol6"=301, "fwVoltPol7"=302, "fwVoltPol8"=303, "Rm1St1Dr1Cmd"=304, "Rm1St2Dr1Cmd"=305, "Rm1St3Dr1Cmd"=306, "Rm1St4Dr1Cmd"=307, "Rm1St5Dr1Cmd"=308, "Rm1St6Dr1Cmd"=309, "Rm1St7Dr1Cmd"=310, "Rm1St8Dr1Cmd"=311, "Rm1St1Dr2Cmd"=312, "Rm1St2Dr2Cmd"=313, "Rm1St3Dr2Cmd"=314, "Rm1St4Dr2Cmd"=315, "Rm1St5Dr2Cmd"=316, "Rm1St6Dr2Cmd"=317, "Rm1St7Dr2Cmd"=318, "Rm1St8Dr2Cmd"=319, "Rm1St1Dr3Cmd"=320, "Rm1St2Dr3Cmd"=321, "Rm1St3Dr3Cmd"=322, "Rm1St4Dr3Cmd"=323, "Rm1St5Dr3Cmd"=324, "Rm1St6Dr3Cmd"=325, "Rm1St7Dr3Cmd"=326, "Rm1St8Dr3Cmd"=327, "fwRmTempSP"=328, "fwRmHumSP"=329, "fwCoolTempSP"=330, "fwDehumTempSP"=331, "fwRmRun"=332, "fwRmOk"=333, "fwTesting"=334, "fwRmDryP"=335, "fwRmDryI"=336, "fwRmHumP"=337, "fwRmHumI"=338, "fwRmHeatP"=339, "fwRmHeatI"=340, "fwCoolTempP"=341, "fwCoolTempI"=342, "fwDehumTempP"=343, "fwDehumTempI"=344, "fwGndLeak1"=345, "fwGndLeak2"=346, "fwGndLeak3"=347, "fwGndLeak4"=348, "fwGndLeak5"=349, "fwGndLeak6"=350, "fwGndLeak7"=351, "fwGndLeak8"=352, "Rm1OpenerCmd"=353] ("Ring")
            n181 = event-data() -> ()  [unwired: 1 in, 6 out]
            n182 = Unbundle By Name(w491) -> ("Device Connections.Wago ModBus Connection"=w492:refnum<class "Modbus Master.lvclass">)
            n183 = local read "Door Settings"() -> (w493:T32)
            n184 = Unbundle By Name(w493) -> ("Station 4.Slide"=w498:T34, "Station 4.Cab"=w499:T34, "Station 4.Freezer"=w500:T34)
            n185 = call-dynamic "Write Single Holding Register.vi"("error in"=w495, "register to write"=w500, "address"=w505, "Modbus master in"=w492) -> ("error out"=w497:errorcluster, "Modbus master out"=w502:refnum<class "Modbus Master.lvclass">)  [unwired: 6 in]
            n186 = call-dynamic "Write Single Holding Register.vi"("error in"=w497, "register to write"=w499, "address"=w504, "Modbus master in"=w502) -> ("error out"=w496:errorcluster, "Modbus master out"=w501:refnum<class "Modbus Master.lvclass">)  [unwired: 6 in]
            n187 = call-dynamic "Write Single Holding Register.vi"("error in"=w496, "register to write"=w498, "address"=w503, "Modbus master in"=w501) -> ("error out"=w494:errorcluster, "Modbus master out"=w489:refnum<class "Modbus Master.lvclass">)  [unwired: 6 in]
            n188 = Bundle By Name(cluster=w491, "Device Connections.Wago ModBus Connection"=w489) -> (w490:T55)
          }
          event "Station 5 CMD": Value Change {
            w521 = T56 324 items=["fwS1Volt1"=0, "fwS1Volt2"=1, "fwS2Volt1"=2, "fwS2Volt2"=3, "fwS3Volt1"=4, "fwS3Volt2"=5, "fwS4Volt1"=6, "fwS4Volt2"=7, "fwS5Volt1"=8, "fwS5Volt2"=9, "fwS6Volt1"=10, "fwS6Volt2 "=11, "fwS7Volt1"=12, "fwS7Volt2"=13, "fwS8Volt1"=14, "fwS8Volt2"=15, "fwRoomHum"=16, "fwRoomTemp"=17, "fwAISpare1"=18, "fwAISpare2"=19, "fwSuppTemp"=20, "fwCoolTemp"=21, "fwDehumTemp"=22, "fwUnused"=23, "Bool Inputs"=24, "gwVoltRate1"=256, "gwVoltRate2"=257, "gwVoltRate3"=258, "gwVoltRate4"=259, "gwVoltRate5"=260, "gwVoltRate6"=261, "gwVoltRate7"=262, "gwVoltRate8"=263, "gwVoltWindow5/1"=264, "gwVoltWindow6/2"=265, "gwVoltWindow7/3"=266, "gwVoltWindow8/4"=267, "fwVoltSet1"=272, "fwVoltSet2"=273, "fwVoltSet3"=274, "fwVoltSet4"=275, "fwVoltSet5"=276, "fwVoltSet6"=277, "fwVoltSet7"=278, "fwVoltSet8"=279, "fwVoltRng1"=280, "fwVoltRng2"=281, "fwVoltRng3"=282, "fwVoltRng4"=283, "fwVoltRng5"=284, "fwVoltRng6"=285, "fwVoltRng7"=286, "fwVoltRng8"=287, "fwVoltPol1"=296, "fwVoltPol2"=297, "fwVoltPol3"=298, "fwVoltPol4"=299, "fwVoltPol5"=300, "fwVoltPol6"=301, "fwVoltPol7"=302, "fwVoltPol8"=303, "Rm1St1Dr1Cmd"=304, "Rm1St2Dr1Cmd"=305, "Rm1St3Dr1Cmd"=306, "Rm1St4Dr1Cmd"=307, "Rm1St5Dr1Cmd"=308, "Rm1St6Dr1Cmd"=309, "Rm1St7Dr1Cmd"=310, "Rm1St8Dr1Cmd"=311, "Rm1St1Dr2Cmd"=312, "Rm1St2Dr2Cmd"=313, "Rm1St3Dr2Cmd"=314, "Rm1St4Dr2Cmd"=315, "Rm1St5Dr2Cmd"=316, "Rm1St6Dr2Cmd"=317, "Rm1St7Dr2Cmd"=318, "Rm1St8Dr2Cmd"=319, "Rm1St1Dr3Cmd"=320, "Rm1St2Dr3Cmd"=321, "Rm1St3Dr3Cmd"=322, "Rm1St4Dr3Cmd"=323, "Rm1St5Dr3Cmd"=324, "Rm1St6Dr3Cmd"=325, "Rm1St7Dr3Cmd"=326, "Rm1St8Dr3Cmd"=327, "fwRmTempSP"=328, "fwRmHumSP"=329, "fwCoolTempSP"=330, "fwDehumTempSP"=331, "fwRmRun"=332, "fwRmOk"=333, "fwTesting"=334, "fwRmDryP"=335, "fwRmDryI"=336, "fwRmHumP"=337, "fwRmHumI"=338, "fwRmHeatP"=339, "fwRmHeatI"=340, "fwCoolTempP"=341, "fwCoolTempI"=342, "fwDehumTempP"=343, "fwDehumTempI"=344, "fwGndLeak1"=345, "fwGndLeak2"=346, "fwGndLeak3"=347, "fwGndLeak4"=348, "fwGndLeak5"=349, "fwGndLeak6"=350, "fwGndLeak7"=351, "fwGndLeak8"=352, "Rm1OpenerCmd"=353] ("Ring")
            w522 = T56 316 items=["fwS1Volt1"=0, "fwS1Volt2"=1, "fwS2Volt1"=2, "fwS2Volt2"=3, "fwS3Volt1"=4, "fwS3Volt2"=5, "fwS4Volt1"=6, "fwS4Volt2"=7, "fwS5Volt1"=8, "fwS5Volt2"=9, "fwS6Volt1"=10, "fwS6Volt2 "=11, "fwS7Volt1"=12, "fwS7Volt2"=13, "fwS8Volt1"=14, "fwS8Volt2"=15, "fwRoomHum"=16, "fwRoomTemp"=17, "fwAISpare1"=18, "fwAISpare2"=19, "fwSuppTemp"=20, "fwCoolTemp"=21, "fwDehumTemp"=22, "fwUnused"=23, "Bool Inputs"=24, "gwVoltRate1"=256, "gwVoltRate2"=257, "gwVoltRate3"=258, "gwVoltRate4"=259, "gwVoltRate5"=260, "gwVoltRate6"=261, "gwVoltRate7"=262, "gwVoltRate8"=263, "gwVoltWindow5/1"=264, "gwVoltWindow6/2"=265, "gwVoltWindow7/3"=266, "gwVoltWindow8/4"=267, "fwVoltSet1"=272, "fwVoltSet2"=273, "fwVoltSet3"=274, "fwVoltSet4"=275, "fwVoltSet5"=276, "fwVoltSet6"=277, "fwVoltSet7"=278, "fwVoltSet8"=279, "fwVoltRng1"=280, "fwVoltRng2"=281, "fwVoltRng3"=282, "fwVoltRng4"=283, "fwVoltRng5"=284, "fwVoltRng6"=285, "fwVoltRng7"=286, "fwVoltRng8"=287, "fwVoltPol1"=296, "fwVoltPol2"=297, "fwVoltPol3"=298, "fwVoltPol4"=299, "fwVoltPol5"=300, "fwVoltPol6"=301, "fwVoltPol7"=302, "fwVoltPol8"=303, "Rm1St1Dr1Cmd"=304, "Rm1St2Dr1Cmd"=305, "Rm1St3Dr1Cmd"=306, "Rm1St4Dr1Cmd"=307, "Rm1St5Dr1Cmd"=308, "Rm1St6Dr1Cmd"=309, "Rm1St7Dr1Cmd"=310, "Rm1St8Dr1Cmd"=311, "Rm1St1Dr2Cmd"=312, "Rm1St2Dr2Cmd"=313, "Rm1St3Dr2Cmd"=314, "Rm1St4Dr2Cmd"=315, "Rm1St5Dr2Cmd"=316, "Rm1St6Dr2Cmd"=317, "Rm1St7Dr2Cmd"=318, "Rm1St8Dr2Cmd"=319, "Rm1St1Dr3Cmd"=320, "Rm1St2Dr3Cmd"=321, "Rm1St3Dr3Cmd"=322, "Rm1St4Dr3Cmd"=323, "Rm1St5Dr3Cmd"=324, "Rm1St6Dr3Cmd"=325, "Rm1St7Dr3Cmd"=326, "Rm1St8Dr3Cmd"=327, "fwRmTempSP"=328, "fwRmHumSP"=329, "fwCoolTempSP"=330, "fwDehumTempSP"=331, "fwRmRun"=332, "fwRmOk"=333, "fwTesting"=334, "fwRmDryP"=335, "fwRmDryI"=336, "fwRmHumP"=337, "fwRmHumI"=338, "fwRmHeatP"=339, "fwRmHeatI"=340, "fwCoolTempP"=341, "fwCoolTempI"=342, "fwDehumTempP"=343, "fwDehumTempI"=344, "fwGndLeak1"=345, "fwGndLeak2"=346, "fwGndLeak3"=347, "fwGndLeak4"=348, "fwGndLeak5"=349, "fwGndLeak6"=350, "fwGndLeak7"=351, "fwGndLeak8"=352, "Rm1OpenerCmd"=353] ("Ring")
            w523 = T56 308 items=["fwS1Volt1"=0, "fwS1Volt2"=1, "fwS2Volt1"=2, "fwS2Volt2"=3, "fwS3Volt1"=4, "fwS3Volt2"=5, "fwS4Volt1"=6, "fwS4Volt2"=7, "fwS5Volt1"=8, "fwS5Volt2"=9, "fwS6Volt1"=10, "fwS6Volt2 "=11, "fwS7Volt1"=12, "fwS7Volt2"=13, "fwS8Volt1"=14, "fwS8Volt2"=15, "fwRoomHum"=16, "fwRoomTemp"=17, "fwAISpare1"=18, "fwAISpare2"=19, "fwSuppTemp"=20, "fwCoolTemp"=21, "fwDehumTemp"=22, "fwUnused"=23, "Bool Inputs"=24, "gwVoltRate1"=256, "gwVoltRate2"=257, "gwVoltRate3"=258, "gwVoltRate4"=259, "gwVoltRate5"=260, "gwVoltRate6"=261, "gwVoltRate7"=262, "gwVoltRate8"=263, "gwVoltWindow5/1"=264, "gwVoltWindow6/2"=265, "gwVoltWindow7/3"=266, "gwVoltWindow8/4"=267, "fwVoltSet1"=272, "fwVoltSet2"=273, "fwVoltSet3"=274, "fwVoltSet4"=275, "fwVoltSet5"=276, "fwVoltSet6"=277, "fwVoltSet7"=278, "fwVoltSet8"=279, "fwVoltRng1"=280, "fwVoltRng2"=281, "fwVoltRng3"=282, "fwVoltRng4"=283, "fwVoltRng5"=284, "fwVoltRng6"=285, "fwVoltRng7"=286, "fwVoltRng8"=287, "fwVoltPol1"=296, "fwVoltPol2"=297, "fwVoltPol3"=298, "fwVoltPol4"=299, "fwVoltPol5"=300, "fwVoltPol6"=301, "fwVoltPol7"=302, "fwVoltPol8"=303, "Rm1St1Dr1Cmd"=304, "Rm1St2Dr1Cmd"=305, "Rm1St3Dr1Cmd"=306, "Rm1St4Dr1Cmd"=307, "Rm1St5Dr1Cmd"=308, "Rm1St6Dr1Cmd"=309, "Rm1St7Dr1Cmd"=310, "Rm1St8Dr1Cmd"=311, "Rm1St1Dr2Cmd"=312, "Rm1St2Dr2Cmd"=313, "Rm1St3Dr2Cmd"=314, "Rm1St4Dr2Cmd"=315, "Rm1St5Dr2Cmd"=316, "Rm1St6Dr2Cmd"=317, "Rm1St7Dr2Cmd"=318, "Rm1St8Dr2Cmd"=319, "Rm1St1Dr3Cmd"=320, "Rm1St2Dr3Cmd"=321, "Rm1St3Dr3Cmd"=322, "Rm1St4Dr3Cmd"=323, "Rm1St5Dr3Cmd"=324, "Rm1St6Dr3Cmd"=325, "Rm1St7Dr3Cmd"=326, "Rm1St8Dr3Cmd"=327, "fwRmTempSP"=328, "fwRmHumSP"=329, "fwCoolTempSP"=330, "fwDehumTempSP"=331, "fwRmRun"=332, "fwRmOk"=333, "fwTesting"=334, "fwRmDryP"=335, "fwRmDryI"=336, "fwRmHumP"=337, "fwRmHumI"=338, "fwRmHeatP"=339, "fwRmHeatI"=340, "fwCoolTempP"=341, "fwCoolTempI"=342, "fwDehumTempP"=343, "fwDehumTempI"=344, "fwGndLeak1"=345, "fwGndLeak2"=346, "fwGndLeak3"=347, "fwGndLeak4"=348, "fwGndLeak5"=349, "fwGndLeak6"=350, "fwGndLeak7"=351, "fwGndLeak8"=352, "Rm1OpenerCmd"=353] ("Ring")
            n189 = event-data() -> ()  [unwired: 1 in, 6 out]
            n190 = Unbundle By Name(w509) -> ("Device Connections.Wago ModBus Connection"=w511:refnum<class "Modbus Master.lvclass">)
            n191 = local read "Door Settings"() -> (w507:T32)
            n192 = Unbundle By Name(w507) -> ("Station 5.Slide"=w516:T34, "Station 5.Cab"=w517:T34, "Station 5.Freezer"=w518:T34)
            n193 = call-dynamic "Write Single Holding Register.vi"("error in"=w513, "register to write"=w518, "address"=w523, "Modbus master in"=w511) -> ("error out"=w515:errorcluster, "Modbus master out"=w520:refnum<class "Modbus Master.lvclass">)  [unwired: 6 in]
            n194 = call-dynamic "Write Single Holding Register.vi"("error in"=w515, "register to write"=w517, "address"=w522, "Modbus master in"=w520) -> ("error out"=w514:errorcluster, "Modbus master out"=w519:refnum<class "Modbus Master.lvclass">)  [unwired: 6 in]
            n195 = call-dynamic "Write Single Holding Register.vi"("error in"=w514, "register to write"=w516, "address"=w521, "Modbus master in"=w519) -> ("error out"=w512:errorcluster, "Modbus master out"=w510:refnum<class "Modbus Master.lvclass">)  [unwired: 6 in]
            n196 = Bundle By Name(cluster=w509, "Device Connections.Wago ModBus Connection"=w510) -> (w508:T55)
          }
          event "Station 6 CMD": Value Change {
            w539 = T56 325 items=["fwS1Volt1"=0, "fwS1Volt2"=1, "fwS2Volt1"=2, "fwS2Volt2"=3, "fwS3Volt1"=4, "fwS3Volt2"=5, "fwS4Volt1"=6, "fwS4Volt2"=7, "fwS5Volt1"=8, "fwS5Volt2"=9, "fwS6Volt1"=10, "fwS6Volt2 "=11, "fwS7Volt1"=12, "fwS7Volt2"=13, "fwS8Volt1"=14, "fwS8Volt2"=15, "fwRoomHum"=16, "fwRoomTemp"=17, "fwAISpare1"=18, "fwAISpare2"=19, "fwSuppTemp"=20, "fwCoolTemp"=21, "fwDehumTemp"=22, "fwUnused"=23, "Bool Inputs"=24, "gwVoltRate1"=256, "gwVoltRate2"=257, "gwVoltRate3"=258, "gwVoltRate4"=259, "gwVoltRate5"=260, "gwVoltRate6"=261, "gwVoltRate7"=262, "gwVoltRate8"=263, "gwVoltWindow5/1"=264, "gwVoltWindow6/2"=265, "gwVoltWindow7/3"=266, "gwVoltWindow8/4"=267, "fwVoltSet1"=272, "fwVoltSet2"=273, "fwVoltSet3"=274, "fwVoltSet4"=275, "fwVoltSet5"=276, "fwVoltSet6"=277, "fwVoltSet7"=278, "fwVoltSet8"=279, "fwVoltRng1"=280, "fwVoltRng2"=281, "fwVoltRng3"=282, "fwVoltRng4"=283, "fwVoltRng5"=284, "fwVoltRng6"=285, "fwVoltRng7"=286, "fwVoltRng8"=287, "fwVoltPol1"=296, "fwVoltPol2"=297, "fwVoltPol3"=298, "fwVoltPol4"=299, "fwVoltPol5"=300, "fwVoltPol6"=301, "fwVoltPol7"=302, "fwVoltPol8"=303, "Rm1St1Dr1Cmd"=304, "Rm1St2Dr1Cmd"=305, "Rm1St3Dr1Cmd"=306, "Rm1St4Dr1Cmd"=307, "Rm1St5Dr1Cmd"=308, "Rm1St6Dr1Cmd"=309, "Rm1St7Dr1Cmd"=310, "Rm1St8Dr1Cmd"=311, "Rm1St1Dr2Cmd"=312, "Rm1St2Dr2Cmd"=313, "Rm1St3Dr2Cmd"=314, "Rm1St4Dr2Cmd"=315, "Rm1St5Dr2Cmd"=316, "Rm1St6Dr2Cmd"=317, "Rm1St7Dr2Cmd"=318, "Rm1St8Dr2Cmd"=319, "Rm1St1Dr3Cmd"=320, "Rm1St2Dr3Cmd"=321, "Rm1St3Dr3Cmd"=322, "Rm1St4Dr3Cmd"=323, "Rm1St5Dr3Cmd"=324, "Rm1St6Dr3Cmd"=325, "Rm1St7Dr3Cmd"=326, "Rm1St8Dr3Cmd"=327, "fwRmTempSP"=328, "fwRmHumSP"=329, "fwCoolTempSP"=330, "fwDehumTempSP"=331, "fwRmRun"=332, "fwRmOk"=333, "fwTesting"=334, "fwRmDryP"=335, "fwRmDryI"=336, "fwRmHumP"=337, "fwRmHumI"=338, "fwRmHeatP"=339, "fwRmHeatI"=340, "fwCoolTempP"=341, "fwCoolTempI"=342, "fwDehumTempP"=343, "fwDehumTempI"=344, "fwGndLeak1"=345, "fwGndLeak2"=346, "fwGndLeak3"=347, "fwGndLeak4"=348, "fwGndLeak5"=349, "fwGndLeak6"=350, "fwGndLeak7"=351, "fwGndLeak8"=352, "Rm1OpenerCmd"=353] ("Ring")
            w540 = T56 317 items=["fwS1Volt1"=0, "fwS1Volt2"=1, "fwS2Volt1"=2, "fwS2Volt2"=3, "fwS3Volt1"=4, "fwS3Volt2"=5, "fwS4Volt1"=6, "fwS4Volt2"=7, "fwS5Volt1"=8, "fwS5Volt2"=9, "fwS6Volt1"=10, "fwS6Volt2 "=11, "fwS7Volt1"=12, "fwS7Volt2"=13, "fwS8Volt1"=14, "fwS8Volt2"=15, "fwRoomHum"=16, "fwRoomTemp"=17, "fwAISpare1"=18, "fwAISpare2"=19, "fwSuppTemp"=20, "fwCoolTemp"=21, "fwDehumTemp"=22, "fwUnused"=23, "Bool Inputs"=24, "gwVoltRate1"=256, "gwVoltRate2"=257, "gwVoltRate3"=258, "gwVoltRate4"=259, "gwVoltRate5"=260, "gwVoltRate6"=261, "gwVoltRate7"=262, "gwVoltRate8"=263, "gwVoltWindow5/1"=264, "gwVoltWindow6/2"=265, "gwVoltWindow7/3"=266, "gwVoltWindow8/4"=267, "fwVoltSet1"=272, "fwVoltSet2"=273, "fwVoltSet3"=274, "fwVoltSet4"=275, "fwVoltSet5"=276, "fwVoltSet6"=277, "fwVoltSet7"=278, "fwVoltSet8"=279, "fwVoltRng1"=280, "fwVoltRng2"=281, "fwVoltRng3"=282, "fwVoltRng4"=283, "fwVoltRng5"=284, "fwVoltRng6"=285, "fwVoltRng7"=286, "fwVoltRng8"=287, "fwVoltPol1"=296, "fwVoltPol2"=297, "fwVoltPol3"=298, "fwVoltPol4"=299, "fwVoltPol5"=300, "fwVoltPol6"=301, "fwVoltPol7"=302, "fwVoltPol8"=303, "Rm1St1Dr1Cmd"=304, "Rm1St2Dr1Cmd"=305, "Rm1St3Dr1Cmd"=306, "Rm1St4Dr1Cmd"=307, "Rm1St5Dr1Cmd"=308, "Rm1St6Dr1Cmd"=309, "Rm1St7Dr1Cmd"=310, "Rm1St8Dr1Cmd"=311, "Rm1St1Dr2Cmd"=312, "Rm1St2Dr2Cmd"=313, "Rm1St3Dr2Cmd"=314, "Rm1St4Dr2Cmd"=315, "Rm1St5Dr2Cmd"=316, "Rm1St6Dr2Cmd"=317, "Rm1St7Dr2Cmd"=318, "Rm1St8Dr2Cmd"=319, "Rm1St1Dr3Cmd"=320, "Rm1St2Dr3Cmd"=321, "Rm1St3Dr3Cmd"=322, "Rm1St4Dr3Cmd"=323, "Rm1St5Dr3Cmd"=324, "Rm1St6Dr3Cmd"=325, "Rm1St7Dr3Cmd"=326, "Rm1St8Dr3Cmd"=327, "fwRmTempSP"=328, "fwRmHumSP"=329, "fwCoolTempSP"=330, "fwDehumTempSP"=331, "fwRmRun"=332, "fwRmOk"=333, "fwTesting"=334, "fwRmDryP"=335, "fwRmDryI"=336, "fwRmHumP"=337, "fwRmHumI"=338, "fwRmHeatP"=339, "fwRmHeatI"=340, "fwCoolTempP"=341, "fwCoolTempI"=342, "fwDehumTempP"=343, "fwDehumTempI"=344, "fwGndLeak1"=345, "fwGndLeak2"=346, "fwGndLeak3"=347, "fwGndLeak4"=348, "fwGndLeak5"=349, "fwGndLeak6"=350, "fwGndLeak7"=351, "fwGndLeak8"=352, "Rm1OpenerCmd"=353] ("Ring")
            w541 = T56 309 items=["fwS1Volt1"=0, "fwS1Volt2"=1, "fwS2Volt1"=2, "fwS2Volt2"=3, "fwS3Volt1"=4, "fwS3Volt2"=5, "fwS4Volt1"=6, "fwS4Volt2"=7, "fwS5Volt1"=8, "fwS5Volt2"=9, "fwS6Volt1"=10, "fwS6Volt2 "=11, "fwS7Volt1"=12, "fwS7Volt2"=13, "fwS8Volt1"=14, "fwS8Volt2"=15, "fwRoomHum"=16, "fwRoomTemp"=17, "fwAISpare1"=18, "fwAISpare2"=19, "fwSuppTemp"=20, "fwCoolTemp"=21, "fwDehumTemp"=22, "fwUnused"=23, "Bool Inputs"=24, "gwVoltRate1"=256, "gwVoltRate2"=257, "gwVoltRate3"=258, "gwVoltRate4"=259, "gwVoltRate5"=260, "gwVoltRate6"=261, "gwVoltRate7"=262, "gwVoltRate8"=263, "gwVoltWindow5/1"=264, "gwVoltWindow6/2"=265, "gwVoltWindow7/3"=266, "gwVoltWindow8/4"=267, "fwVoltSet1"=272, "fwVoltSet2"=273, "fwVoltSet3"=274, "fwVoltSet4"=275, "fwVoltSet5"=276, "fwVoltSet6"=277, "fwVoltSet7"=278, "fwVoltSet8"=279, "fwVoltRng1"=280, "fwVoltRng2"=281, "fwVoltRng3"=282, "fwVoltRng4"=283, "fwVoltRng5"=284, "fwVoltRng6"=285, "fwVoltRng7"=286, "fwVoltRng8"=287, "fwVoltPol1"=296, "fwVoltPol2"=297, "fwVoltPol3"=298, "fwVoltPol4"=299, "fwVoltPol5"=300, "fwVoltPol6"=301, "fwVoltPol7"=302, "fwVoltPol8"=303, "Rm1St1Dr1Cmd"=304, "Rm1St2Dr1Cmd"=305, "Rm1St3Dr1Cmd"=306, "Rm1St4Dr1Cmd"=307, "Rm1St5Dr1Cmd"=308, "Rm1St6Dr1Cmd"=309, "Rm1St7Dr1Cmd"=310, "Rm1St8Dr1Cmd"=311, "Rm1St1Dr2Cmd"=312, "Rm1St2Dr2Cmd"=313, "Rm1St3Dr2Cmd"=314, "Rm1St4Dr2Cmd"=315, "Rm1St5Dr2Cmd"=316, "Rm1St6Dr2Cmd"=317, "Rm1St7Dr2Cmd"=318, "Rm1St8Dr2Cmd"=319, "Rm1St1Dr3Cmd"=320, "Rm1St2Dr3Cmd"=321, "Rm1St3Dr3Cmd"=322, "Rm1St4Dr3Cmd"=323, "Rm1St5Dr3Cmd"=324, "Rm1St6Dr3Cmd"=325, "Rm1St7Dr3Cmd"=326, "Rm1St8Dr3Cmd"=327, "fwRmTempSP"=328, "fwRmHumSP"=329, "fwCoolTempSP"=330, "fwDehumTempSP"=331, "fwRmRun"=332, "fwRmOk"=333, "fwTesting"=334, "fwRmDryP"=335, "fwRmDryI"=336, "fwRmHumP"=337, "fwRmHumI"=338, "fwRmHeatP"=339, "fwRmHeatI"=340, "fwCoolTempP"=341, "fwCoolTempI"=342, "fwDehumTempP"=343, "fwDehumTempI"=344, "fwGndLeak1"=345, "fwGndLeak2"=346, "fwGndLeak3"=347, "fwGndLeak4"=348, "fwGndLeak5"=349, "fwGndLeak6"=350, "fwGndLeak7"=351, "fwGndLeak8"=352, "Rm1OpenerCmd"=353] ("Ring")
            n197 = event-data() -> ()  [unwired: 1 in, 6 out]
            n198 = Unbundle By Name(w529) -> ("Device Connections.Wago ModBus Connection"=w526:refnum<class "Modbus Master.lvclass">)
            n199 = local read "Door Settings"() -> (w525:T32)
            n200 = Unbundle By Name(w525) -> ("Station 6.Slide"=w534:T34, "Station 6.Cab"=w535:T34, "Station 6.Freezer"=w536:T34)
            n201 = call-dynamic "Write Single Holding Register.vi"("error in"=w531, "register to write"=w536, "address"=w541, "Modbus master in"=w526) -> ("error out"=w533:errorcluster, "Modbus master out"=w538:refnum<class "Modbus Master.lvclass">)  [unwired: 6 in]
            n202 = call-dynamic "Write Single Holding Register.vi"("error in"=w533, "register to write"=w535, "address"=w540, "Modbus master in"=w538) -> ("error out"=w532:errorcluster, "Modbus master out"=w537:refnum<class "Modbus Master.lvclass">)  [unwired: 6 in]
            n203 = call-dynamic "Write Single Holding Register.vi"("error in"=w532, "register to write"=w534, "address"=w539, "Modbus master in"=w537) -> ("error out"=w530:errorcluster, "Modbus master out"=w527:refnum<class "Modbus Master.lvclass">)  [unwired: 6 in]
            n204 = Bundle By Name(cluster=w529, "Device Connections.Wago ModBus Connection"=w527) -> (w528:T55)
          }
          event "Station 7 CMD": Value Change {
            w557 = T56 326 items=["fwS1Volt1"=0, "fwS1Volt2"=1, "fwS2Volt1"=2, "fwS2Volt2"=3, "fwS3Volt1"=4, "fwS3Volt2"=5, "fwS4Volt1"=6, "fwS4Volt2"=7, "fwS5Volt1"=8, "fwS5Volt2"=9, "fwS6Volt1"=10, "fwS6Volt2 "=11, "fwS7Volt1"=12, "fwS7Volt2"=13, "fwS8Volt1"=14, "fwS8Volt2"=15, "fwRoomHum"=16, "fwRoomTemp"=17, "fwAISpare1"=18, "fwAISpare2"=19, "fwSuppTemp"=20, "fwCoolTemp"=21, "fwDehumTemp"=22, "fwUnused"=23, "Bool Inputs"=24, "gwVoltRate1"=256, "gwVoltRate2"=257, "gwVoltRate3"=258, "gwVoltRate4"=259, "gwVoltRate5"=260, "gwVoltRate6"=261, "gwVoltRate7"=262, "gwVoltRate8"=263, "gwVoltWindow5/1"=264, "gwVoltWindow6/2"=265, "gwVoltWindow7/3"=266, "gwVoltWindow8/4"=267, "fwVoltSet1"=272, "fwVoltSet2"=273, "fwVoltSet3"=274, "fwVoltSet4"=275, "fwVoltSet5"=276, "fwVoltSet6"=277, "fwVoltSet7"=278, "fwVoltSet8"=279, "fwVoltRng1"=280, "fwVoltRng2"=281, "fwVoltRng3"=282, "fwVoltRng4"=283, "fwVoltRng5"=284, "fwVoltRng6"=285, "fwVoltRng7"=286, "fwVoltRng8"=287, "fwVoltPol1"=296, "fwVoltPol2"=297, "fwVoltPol3"=298, "fwVoltPol4"=299, "fwVoltPol5"=300, "fwVoltPol6"=301, "fwVoltPol7"=302, "fwVoltPol8"=303, "Rm1St1Dr1Cmd"=304, "Rm1St2Dr1Cmd"=305, "Rm1St3Dr1Cmd"=306, "Rm1St4Dr1Cmd"=307, "Rm1St5Dr1Cmd"=308, "Rm1St6Dr1Cmd"=309, "Rm1St7Dr1Cmd"=310, "Rm1St8Dr1Cmd"=311, "Rm1St1Dr2Cmd"=312, "Rm1St2Dr2Cmd"=313, "Rm1St3Dr2Cmd"=314, "Rm1St4Dr2Cmd"=315, "Rm1St5Dr2Cmd"=316, "Rm1St6Dr2Cmd"=317, "Rm1St7Dr2Cmd"=318, "Rm1St8Dr2Cmd"=319, "Rm1St1Dr3Cmd"=320, "Rm1St2Dr3Cmd"=321, "Rm1St3Dr3Cmd"=322, "Rm1St4Dr3Cmd"=323, "Rm1St5Dr3Cmd"=324, "Rm1St6Dr3Cmd"=325, "Rm1St7Dr3Cmd"=326, "Rm1St8Dr3Cmd"=327, "fwRmTempSP"=328, "fwRmHumSP"=329, "fwCoolTempSP"=330, "fwDehumTempSP"=331, "fwRmRun"=332, "fwRmOk"=333, "fwTesting"=334, "fwRmDryP"=335, "fwRmDryI"=336, "fwRmHumP"=337, "fwRmHumI"=338, "fwRmHeatP"=339, "fwRmHeatI"=340, "fwCoolTempP"=341, "fwCoolTempI"=342, "fwDehumTempP"=343, "fwDehumTempI"=344, "fwGndLeak1"=345, "fwGndLeak2"=346, "fwGndLeak3"=347, "fwGndLeak4"=348, "fwGndLeak5"=349, "fwGndLeak6"=350, "fwGndLeak7"=351, "fwGndLeak8"=352, "Rm1OpenerCmd"=353] ("Ring")
            w558 = T56 318 items=["fwS1Volt1"=0, "fwS1Volt2"=1, "fwS2Volt1"=2, "fwS2Volt2"=3, "fwS3Volt1"=4, "fwS3Volt2"=5, "fwS4Volt1"=6, "fwS4Volt2"=7, "fwS5Volt1"=8, "fwS5Volt2"=9, "fwS6Volt1"=10, "fwS6Volt2 "=11, "fwS7Volt1"=12, "fwS7Volt2"=13, "fwS8Volt1"=14, "fwS8Volt2"=15, "fwRoomHum"=16, "fwRoomTemp"=17, "fwAISpare1"=18, "fwAISpare2"=19, "fwSuppTemp"=20, "fwCoolTemp"=21, "fwDehumTemp"=22, "fwUnused"=23, "Bool Inputs"=24, "gwVoltRate1"=256, "gwVoltRate2"=257, "gwVoltRate3"=258, "gwVoltRate4"=259, "gwVoltRate5"=260, "gwVoltRate6"=261, "gwVoltRate7"=262, "gwVoltRate8"=263, "gwVoltWindow5/1"=264, "gwVoltWindow6/2"=265, "gwVoltWindow7/3"=266, "gwVoltWindow8/4"=267, "fwVoltSet1"=272, "fwVoltSet2"=273, "fwVoltSet3"=274, "fwVoltSet4"=275, "fwVoltSet5"=276, "fwVoltSet6"=277, "fwVoltSet7"=278, "fwVoltSet8"=279, "fwVoltRng1"=280, "fwVoltRng2"=281, "fwVoltRng3"=282, "fwVoltRng4"=283, "fwVoltRng5"=284, "fwVoltRng6"=285, "fwVoltRng7"=286, "fwVoltRng8"=287, "fwVoltPol1"=296, "fwVoltPol2"=297, "fwVoltPol3"=298, "fwVoltPol4"=299, "fwVoltPol5"=300, "fwVoltPol6"=301, "fwVoltPol7"=302, "fwVoltPol8"=303, "Rm1St1Dr1Cmd"=304, "Rm1St2Dr1Cmd"=305, "Rm1St3Dr1Cmd"=306, "Rm1St4Dr1Cmd"=307, "Rm1St5Dr1Cmd"=308, "Rm1St6Dr1Cmd"=309, "Rm1St7Dr1Cmd"=310, "Rm1St8Dr1Cmd"=311, "Rm1St1Dr2Cmd"=312, "Rm1St2Dr2Cmd"=313, "Rm1St3Dr2Cmd"=314, "Rm1St4Dr2Cmd"=315, "Rm1St5Dr2Cmd"=316, "Rm1St6Dr2Cmd"=317, "Rm1St7Dr2Cmd"=318, "Rm1St8Dr2Cmd"=319, "Rm1St1Dr3Cmd"=320, "Rm1St2Dr3Cmd"=321, "Rm1St3Dr3Cmd"=322, "Rm1St4Dr3Cmd"=323, "Rm1St5Dr3Cmd"=324, "Rm1St6Dr3Cmd"=325, "Rm1St7Dr3Cmd"=326, "Rm1St8Dr3Cmd"=327, "fwRmTempSP"=328, "fwRmHumSP"=329, "fwCoolTempSP"=330, "fwDehumTempSP"=331, "fwRmRun"=332, "fwRmOk"=333, "fwTesting"=334, "fwRmDryP"=335, "fwRmDryI"=336, "fwRmHumP"=337, "fwRmHumI"=338, "fwRmHeatP"=339, "fwRmHeatI"=340, "fwCoolTempP"=341, "fwCoolTempI"=342, "fwDehumTempP"=343, "fwDehumTempI"=344, "fwGndLeak1"=345, "fwGndLeak2"=346, "fwGndLeak3"=347, "fwGndLeak4"=348, "fwGndLeak5"=349, "fwGndLeak6"=350, "fwGndLeak7"=351, "fwGndLeak8"=352, "Rm1OpenerCmd"=353] ("Ring")
            w559 = T56 310 items=["fwS1Volt1"=0, "fwS1Volt2"=1, "fwS2Volt1"=2, "fwS2Volt2"=3, "fwS3Volt1"=4, "fwS3Volt2"=5, "fwS4Volt1"=6, "fwS4Volt2"=7, "fwS5Volt1"=8, "fwS5Volt2"=9, "fwS6Volt1"=10, "fwS6Volt2 "=11, "fwS7Volt1"=12, "fwS7Volt2"=13, "fwS8Volt1"=14, "fwS8Volt2"=15, "fwRoomHum"=16, "fwRoomTemp"=17, "fwAISpare1"=18, "fwAISpare2"=19, "fwSuppTemp"=20, "fwCoolTemp"=21, "fwDehumTemp"=22, "fwUnused"=23, "Bool Inputs"=24, "gwVoltRate1"=256, "gwVoltRate2"=257, "gwVoltRate3"=258, "gwVoltRate4"=259, "gwVoltRate5"=260, "gwVoltRate6"=261, "gwVoltRate7"=262, "gwVoltRate8"=263, "gwVoltWindow5/1"=264, "gwVoltWindow6/2"=265, "gwVoltWindow7/3"=266, "gwVoltWindow8/4"=267, "fwVoltSet1"=272, "fwVoltSet2"=273, "fwVoltSet3"=274, "fwVoltSet4"=275, "fwVoltSet5"=276, "fwVoltSet6"=277, "fwVoltSet7"=278, "fwVoltSet8"=279, "fwVoltRng1"=280, "fwVoltRng2"=281, "fwVoltRng3"=282, "fwVoltRng4"=283, "fwVoltRng5"=284, "fwVoltRng6"=285, "fwVoltRng7"=286, "fwVoltRng8"=287, "fwVoltPol1"=296, "fwVoltPol2"=297, "fwVoltPol3"=298, "fwVoltPol4"=299, "fwVoltPol5"=300, "fwVoltPol6"=301, "fwVoltPol7"=302, "fwVoltPol8"=303, "Rm1St1Dr1Cmd"=304, "Rm1St2Dr1Cmd"=305, "Rm1St3Dr1Cmd"=306, "Rm1St4Dr1Cmd"=307, "Rm1St5Dr1Cmd"=308, "Rm1St6Dr1Cmd"=309, "Rm1St7Dr1Cmd"=310, "Rm1St8Dr1Cmd"=311, "Rm1St1Dr2Cmd"=312, "Rm1St2Dr2Cmd"=313, "Rm1St3Dr2Cmd"=314, "Rm1St4Dr2Cmd"=315, "Rm1St5Dr2Cmd"=316, "Rm1St6Dr2Cmd"=317, "Rm1St7Dr2Cmd"=318, "Rm1St8Dr2Cmd"=319, "Rm1St1Dr3Cmd"=320, "Rm1St2Dr3Cmd"=321, "Rm1St3Dr3Cmd"=322, "Rm1St4Dr3Cmd"=323, "Rm1St5Dr3Cmd"=324, "Rm1St6Dr3Cmd"=325, "Rm1St7Dr3Cmd"=326, "Rm1St8Dr3Cmd"=327, "fwRmTempSP"=328, "fwRmHumSP"=329, "fwCoolTempSP"=330, "fwDehumTempSP"=331, "fwRmRun"=332, "fwRmOk"=333, "fwTesting"=334, "fwRmDryP"=335, "fwRmDryI"=336, "fwRmHumP"=337, "fwRmHumI"=338, "fwRmHeatP"=339, "fwRmHeatI"=340, "fwCoolTempP"=341, "fwCoolTempI"=342, "fwDehumTempP"=343, "fwDehumTempI"=344, "fwGndLeak1"=345, "fwGndLeak2"=346, "fwGndLeak3"=347, "fwGndLeak4"=348, "fwGndLeak5"=349, "fwGndLeak6"=350, "fwGndLeak7"=351, "fwGndLeak8"=352, "Rm1OpenerCmd"=353] ("Ring")
            n205 = event-data() -> ()  [unwired: 1 in, 6 out]
            n206 = Unbundle By Name(w545) -> ("Device Connections.Wago ModBus Connection"=w547:refnum<class "Modbus Master.lvclass">)
            n207 = local read "Door Settings"() -> (w549:T32)
            n208 = Unbundle By Name(w549) -> ("Station 7.Slide"=w552:T34, "Station 7.Cab"=w553:T34, "Station 7.Freezer"=w554:T34)
            n209 = call-dynamic "Write Single Holding Register.vi"("error in"=w548, "register to write"=w554, "address"=w559, "Modbus master in"=w547) -> ("error out"=w551:errorcluster, "Modbus master out"=w556:refnum<class "Modbus Master.lvclass">)  [unwired: 6 in]
            n210 = call-dynamic "Write Single Holding Register.vi"("error in"=w551, "register to write"=w553, "address"=w558, "Modbus master in"=w556) -> ("error out"=w550:errorcluster, "Modbus master out"=w555:refnum<class "Modbus Master.lvclass">)  [unwired: 6 in]
            n211 = call-dynamic "Write Single Holding Register.vi"("error in"=w550, "register to write"=w552, "address"=w557, "Modbus master in"=w555) -> ("error out"=w543:errorcluster, "Modbus master out"=w546:refnum<class "Modbus Master.lvclass">)  [unwired: 6 in]
            n212 = Bundle By Name(cluster=w545, "Device Connections.Wago ModBus Connection"=w546) -> (w544:T55)
          }
          event "Station 8 CMD": Value Change {
            w570 = T56 327 items=["fwS1Volt1"=0, "fwS1Volt2"=1, "fwS2Volt1"=2, "fwS2Volt2"=3, "fwS3Volt1"=4, "fwS3Volt2"=5, "fwS4Volt1"=6, "fwS4Volt2"=7, "fwS5Volt1"=8, "fwS5Volt2"=9, "fwS6Volt1"=10, "fwS6Volt2 "=11, "fwS7Volt1"=12, "fwS7Volt2"=13, "fwS8Volt1"=14, "fwS8Volt2"=15, "fwRoomHum"=16, "fwRoomTemp"=17, "fwAISpare1"=18, "fwAISpare2"=19, "fwSuppTemp"=20, "fwCoolTemp"=21, "fwDehumTemp"=22, "fwUnused"=23, "Bool Inputs"=24, "gwVoltRate1"=256, "gwVoltRate2"=257, "gwVoltRate3"=258, "gwVoltRate4"=259, "gwVoltRate5"=260, "gwVoltRate6"=261, "gwVoltRate7"=262, "gwVoltRate8"=263, "gwVoltWindow5/1"=264, "gwVoltWindow6/2"=265, "gwVoltWindow7/3"=266, "gwVoltWindow8/4"=267, "fwVoltSet1"=272, "fwVoltSet2"=273, "fwVoltSet3"=274, "fwVoltSet4"=275, "fwVoltSet5"=276, "fwVoltSet6"=277, "fwVoltSet7"=278, "fwVoltSet8"=279, "fwVoltRng1"=280, "fwVoltRng2"=281, "fwVoltRng3"=282, "fwVoltRng4"=283, "fwVoltRng5"=284, "fwVoltRng6"=285, "fwVoltRng7"=286, "fwVoltRng8"=287, "fwVoltPol1"=296, "fwVoltPol2"=297, "fwVoltPol3"=298, "fwVoltPol4"=299, "fwVoltPol5"=300, "fwVoltPol6"=301, "fwVoltPol7"=302, "fwVoltPol8"=303, "Rm1St1Dr1Cmd"=304, "Rm1St2Dr1Cmd"=305, "Rm1St3Dr1Cmd"=306, "Rm1St4Dr1Cmd"=307, "Rm1St5Dr1Cmd"=308, "Rm1St6Dr1Cmd"=309, "Rm1St7Dr1Cmd"=310, "Rm1St8Dr1Cmd"=311, "Rm1St1Dr2Cmd"=312, "Rm1St2Dr2Cmd"=313, "Rm1St3Dr2Cmd"=314, "Rm1St4Dr2Cmd"=315, "Rm1St5Dr2Cmd"=316, "Rm1St6Dr2Cmd"=317, "Rm1St7Dr2Cmd"=318, "Rm1St8Dr2Cmd"=319, "Rm1St1Dr3Cmd"=320, "Rm1St2Dr3Cmd"=321, "Rm1St3Dr3Cmd"=322, "Rm1St4Dr3Cmd"=323, "Rm1St5Dr3Cmd"=324, "Rm1St6Dr3Cmd"=325, "Rm1St7Dr3Cmd"=326, "Rm1St8Dr3Cmd"=327, "fwRmTempSP"=328, "fwRmHumSP"=329, "fwCoolTempSP"=330, "fwDehumTempSP"=331, "fwRmRun"=332, "fwRmOk"=333, "fwTesting"=334, "fwRmDryP"=335, "fwRmDryI"=336, "fwRmHumP"=337, "fwRmHumI"=338, "fwRmHeatP"=339, "fwRmHeatI"=340, "fwCoolTempP"=341, "fwCoolTempI"=342, "fwDehumTempP"=343, "fwDehumTempI"=344, "fwGndLeak1"=345, "fwGndLeak2"=346, "fwGndLeak3"=347, "fwGndLeak4"=348, "fwGndLeak5"=349, "fwGndLeak6"=350, "fwGndLeak7"=351, "fwGndLeak8"=352, "Rm1OpenerCmd"=353] ("Ring")
            w571 = T56 319 items=["fwS1Volt1"=0, "fwS1Volt2"=1, "fwS2Volt1"=2, "fwS2Volt2"=3, "fwS3Volt1"=4, "fwS3Volt2"=5, "fwS4Volt1"=6, "fwS4Volt2"=7, "fwS5Volt1"=8, "fwS5Volt2"=9, "fwS6Volt1"=10, "fwS6Volt2 "=11, "fwS7Volt1"=12, "fwS7Volt2"=13, "fwS8Volt1"=14, "fwS8Volt2"=15, "fwRoomHum"=16, "fwRoomTemp"=17, "fwAISpare1"=18, "fwAISpare2"=19, "fwSuppTemp"=20, "fwCoolTemp"=21, "fwDehumTemp"=22, "fwUnused"=23, "Bool Inputs"=24, "gwVoltRate1"=256, "gwVoltRate2"=257, "gwVoltRate3"=258, "gwVoltRate4"=259, "gwVoltRate5"=260, "gwVoltRate6"=261, "gwVoltRate7"=262, "gwVoltRate8"=263, "gwVoltWindow5/1"=264, "gwVoltWindow6/2"=265, "gwVoltWindow7/3"=266, "gwVoltWindow8/4"=267, "fwVoltSet1"=272, "fwVoltSet2"=273, "fwVoltSet3"=274, "fwVoltSet4"=275, "fwVoltSet5"=276, "fwVoltSet6"=277, "fwVoltSet7"=278, "fwVoltSet8"=279, "fwVoltRng1"=280, "fwVoltRng2"=281, "fwVoltRng3"=282, "fwVoltRng4"=283, "fwVoltRng5"=284, "fwVoltRng6"=285, "fwVoltRng7"=286, "fwVoltRng8"=287, "fwVoltPol1"=296, "fwVoltPol2"=297, "fwVoltPol3"=298, "fwVoltPol4"=299, "fwVoltPol5"=300, "fwVoltPol6"=301, "fwVoltPol7"=302, "fwVoltPol8"=303, "Rm1St1Dr1Cmd"=304, "Rm1St2Dr1Cmd"=305, "Rm1St3Dr1Cmd"=306, "Rm1St4Dr1Cmd"=307, "Rm1St5Dr1Cmd"=308, "Rm1St6Dr1Cmd"=309, "Rm1St7Dr1Cmd"=310, "Rm1St8Dr1Cmd"=311, "Rm1St1Dr2Cmd"=312, "Rm1St2Dr2Cmd"=313, "Rm1St3Dr2Cmd"=314, "Rm1St4Dr2Cmd"=315, "Rm1St5Dr2Cmd"=316, "Rm1St6Dr2Cmd"=317, "Rm1St7Dr2Cmd"=318, "Rm1St8Dr2Cmd"=319, "Rm1St1Dr3Cmd"=320, "Rm1St2Dr3Cmd"=321, "Rm1St3Dr3Cmd"=322, "Rm1St4Dr3Cmd"=323, "Rm1St5Dr3Cmd"=324, "Rm1St6Dr3Cmd"=325, "Rm1St7Dr3Cmd"=326, "Rm1St8Dr3Cmd"=327, "fwRmTempSP"=328, "fwRmHumSP"=329, "fwCoolTempSP"=330, "fwDehumTempSP"=331, "fwRmRun"=332, "fwRmOk"=333, "fwTesting"=334, "fwRmDryP"=335, "fwRmDryI"=336, "fwRmHumP"=337, "fwRmHumI"=338, "fwRmHeatP"=339, "fwRmHeatI"=340, "fwCoolTempP"=341, "fwCoolTempI"=342, "fwDehumTempP"=343, "fwDehumTempI"=344, "fwGndLeak1"=345, "fwGndLeak2"=346, "fwGndLeak3"=347, "fwGndLeak4"=348, "fwGndLeak5"=349, "fwGndLeak6"=350, "fwGndLeak7"=351, "fwGndLeak8"=352, "Rm1OpenerCmd"=353] ("Ring")
            w577 = T56 311 items=["fwS1Volt1"=0, "fwS1Volt2"=1, "fwS2Volt1"=2, "fwS2Volt2"=3, "fwS3Volt1"=4, "fwS3Volt2"=5, "fwS4Volt1"=6, "fwS4Volt2"=7, "fwS5Volt1"=8, "fwS5Volt2"=9, "fwS6Volt1"=10, "fwS6Volt2 "=11, "fwS7Volt1"=12, "fwS7Volt2"=13, "fwS8Volt1"=14, "fwS8Volt2"=15, "fwRoomHum"=16, "fwRoomTemp"=17, "fwAISpare1"=18, "fwAISpare2"=19, "fwSuppTemp"=20, "fwCoolTemp"=21, "fwDehumTemp"=22, "fwUnused"=23, "Bool Inputs"=24, "gwVoltRate1"=256, "gwVoltRate2"=257, "gwVoltRate3"=258, "gwVoltRate4"=259, "gwVoltRate5"=260, "gwVoltRate6"=261, "gwVoltRate7"=262, "gwVoltRate8"=263, "gwVoltWindow5/1"=264, "gwVoltWindow6/2"=265, "gwVoltWindow7/3"=266, "gwVoltWindow8/4"=267, "fwVoltSet1"=272, "fwVoltSet2"=273, "fwVoltSet3"=274, "fwVoltSet4"=275, "fwVoltSet5"=276, "fwVoltSet6"=277, "fwVoltSet7"=278, "fwVoltSet8"=279, "fwVoltRng1"=280, "fwVoltRng2"=281, "fwVoltRng3"=282, "fwVoltRng4"=283, "fwVoltRng5"=284, "fwVoltRng6"=285, "fwVoltRng7"=286, "fwVoltRng8"=287, "fwVoltPol1"=296, "fwVoltPol2"=297, "fwVoltPol3"=298, "fwVoltPol4"=299, "fwVoltPol5"=300, "fwVoltPol6"=301, "fwVoltPol7"=302, "fwVoltPol8"=303, "Rm1St1Dr1Cmd"=304, "Rm1St2Dr1Cmd"=305, "Rm1St3Dr1Cmd"=306, "Rm1St4Dr1Cmd"=307, "Rm1St5Dr1Cmd"=308, "Rm1St6Dr1Cmd"=309, "Rm1St7Dr1Cmd"=310, "Rm1St8Dr1Cmd"=311, "Rm1St1Dr2Cmd"=312, "Rm1St2Dr2Cmd"=313, "Rm1St3Dr2Cmd"=314, "Rm1St4Dr2Cmd"=315, "Rm1St5Dr2Cmd"=316, "Rm1St6Dr2Cmd"=317, "Rm1St7Dr2Cmd"=318, "Rm1St8Dr2Cmd"=319, "Rm1St1Dr3Cmd"=320, "Rm1St2Dr3Cmd"=321, "Rm1St3Dr3Cmd"=322, "Rm1St4Dr3Cmd"=323, "Rm1St5Dr3Cmd"=324, "Rm1St6Dr3Cmd"=325, "Rm1St7Dr3Cmd"=326, "Rm1St8Dr3Cmd"=327, "fwRmTempSP"=328, "fwRmHumSP"=329, "fwCoolTempSP"=330, "fwDehumTempSP"=331, "fwRmRun"=332, "fwRmOk"=333, "fwTesting"=334, "fwRmDryP"=335, "fwRmDryI"=336, "fwRmHumP"=337, "fwRmHumI"=338, "fwRmHeatP"=339, "fwRmHeatI"=340, "fwCoolTempP"=341, "fwCoolTempI"=342, "fwDehumTempP"=343, "fwDehumTempI"=344, "fwGndLeak1"=345, "fwGndLeak2"=346, "fwGndLeak3"=347, "fwGndLeak4"=348, "fwGndLeak5"=349, "fwGndLeak6"=350, "fwGndLeak7"=351, "fwGndLeak8"=352, "Rm1OpenerCmd"=353] ("Ring")
            n213 = event-data() -> ()  [unwired: 1 in, 6 out]
            n214 = Unbundle By Name(w563) -> ("Device Connections.Wago ModBus Connection"=w566:refnum<class "Modbus Master.lvclass">)
            n215 = local read "Door Settings"() -> (w567:T32)
            n216 = Unbundle By Name(w567) -> ("Station 8.Slide"=w573:T34, "Station 8.Cab"=w574:T34, "Station 8.Freezer"=w575:T34)
            n217 = call-dynamic "Write Single Holding Register.vi"("error in"=w565, "register to write"=w575, "address"=w577, "Modbus master in"=w566) -> ("error out"=w572:errorcluster, "Modbus master out"=w576:refnum<class "Modbus Master.lvclass">)  [unwired: 6 in]
            n218 = call-dynamic "Write Single Holding Register.vi"("error in"=w572, "register to write"=w574, "address"=w571, "Modbus master in"=w576) -> ("error out"=w568:errorcluster, "Modbus master out"=w569:refnum<class "Modbus Master.lvclass">)  [unwired: 6 in]
            n219 = call-dynamic "Write Single Holding Register.vi"("error in"=w568, "register to write"=w573, "address"=w570, "Modbus master in"=w569) -> ("error out"=w561:errorcluster, "Modbus master out"=w564:refnum<class "Modbus Master.lvclass">)  [unwired: 6 in]
            n220 = Bundle By Name(cluster=w563, "Device Connections.Wago ModBus Connection"=w564) -> (w562:T55)
          }
          event Value Change {
            w587 = T56 333 items=["fwS1Volt1"=0, "fwS1Volt2"=1, "fwS2Volt1"=2, "fwS2Volt2"=3, "fwS3Volt1"=4, "fwS3Volt2"=5, "fwS4Volt1"=6, "fwS4Volt2"=7, "fwS5Volt1"=8, "fwS5Volt2"=9, "fwS6Volt1"=10, "fwS6Volt2 "=11, "fwS7Volt1"=12, "fwS7Volt2"=13, "fwS8Volt1"=14, "fwS8Volt2"=15, "fwRoomHum"=16, "fwRoomTemp"=17, "fwAISpare1"=18, "fwAISpare2"=19, "fwSuppTemp"=20, "fwCoolTemp"=21, "fwDehumTemp"=22, "fwUnused"=23, "Bool Inputs"=24, "gwVoltRate1"=256, "gwVoltRate2"=257, "gwVoltRate3"=258, "gwVoltRate4"=259, "gwVoltRate5"=260, "gwVoltRate6"=261, "gwVoltRate7"=262, "gwVoltRate8"=263, "gwVoltWindow5/1"=264, "gwVoltWindow6/2"=265, "gwVoltWindow7/3"=266, "gwVoltWindow8/4"=267, "fwVoltSet1"=272, "fwVoltSet2"=273, "fwVoltSet3"=274, "fwVoltSet4"=275, "fwVoltSet5"=276, "fwVoltSet6"=277, "fwVoltSet7"=278, "fwVoltSet8"=279, "fwVoltRng1"=280, "fwVoltRng2"=281, "fwVoltRng3"=282, "fwVoltRng4"=283, "fwVoltRng5"=284, "fwVoltRng6"=285, "fwVoltRng7"=286, "fwVoltRng8"=287, "fwVoltPol1"=296, "fwVoltPol2"=297, "fwVoltPol3"=298, "fwVoltPol4"=299, "fwVoltPol5"=300, "fwVoltPol6"=301, "fwVoltPol7"=302, "fwVoltPol8"=303, "Rm1St1Dr1Cmd"=304, "Rm1St2Dr1Cmd"=305, "Rm1St3Dr1Cmd"=306, "Rm1St4Dr1Cmd"=307, "Rm1St5Dr1Cmd"=308, "Rm1St6Dr1Cmd"=309, "Rm1St7Dr1Cmd"=310, "Rm1St8Dr1Cmd"=311, "Rm1St1Dr2Cmd"=312, "Rm1St2Dr2Cmd"=313, "Rm1St3Dr2Cmd"=314, "Rm1St4Dr2Cmd"=315, "Rm1St5Dr2Cmd"=316, "Rm1St6Dr2Cmd"=317, "Rm1St7Dr2Cmd"=318, "Rm1St8Dr2Cmd"=319, "Rm1St1Dr3Cmd"=320, "Rm1St2Dr3Cmd"=321, "Rm1St3Dr3Cmd"=322, "Rm1St4Dr3Cmd"=323, "Rm1St5Dr3Cmd"=324, "Rm1St6Dr3Cmd"=325, "Rm1St7Dr3Cmd"=326, "Rm1St8Dr3Cmd"=327, "fwRmTempSP"=328, "fwRmHumSP"=329, "fwCoolTempSP"=330, "fwDehumTempSP"=331, "fwRmRun"=332, "fwRmOk"=333, "fwTesting"=334, "fwRmDryP"=335, "fwRmDryI"=336, "fwRmHumP"=337, "fwRmHumI"=338, "fwRmHeatP"=339, "fwRmHeatI"=340, "fwCoolTempP"=341, "fwCoolTempI"=342, "fwDehumTempP"=343, "fwDehumTempI"=344, "fwGndLeak1"=345, "fwGndLeak2"=346, "fwGndLeak3"=347, "fwGndLeak4"=348, "fwGndLeak5"=349, "fwGndLeak6"=350, "fwGndLeak7"=351, "fwGndLeak8"=352, "Rm1OpenerCmd"=353] ("Ring")
            n221 = event-data() -> ()  [unwired: 1 in, 6 out]
            n222 = Unbundle By Name(w584) -> ("Device Connections.Wago ModBus Connection"=w581:refnum<class "Modbus Master.lvclass">)
            n223 = call "Wago Input Output Converter.vi"("Input to Output?"=TRUE, "Input Command"=w587) -> ("Read Input Command Location"=w588:i32)  [unwired: 9 in]
            n224 = call-dynamic "Read Holding Registers.vi"("error in"=w580, "number of inputs"="Room OK?", "starting address"=w588, "Modbus master in"=w581) -> ("error out"=w579:errorcluster, "Modbus master out"=w582:refnum<class "Modbus Master.lvclass">)  [unwired: 5 in, 1 out]
            n225 = Bundle By Name(cluster=w584, "Device Connections.Wago ModBus Connection"=w582) -> (w583:T55)
          }
          event Value Change {
            w599 = T56 332 items=["fwS1Volt1"=0, "fwS1Volt2"=1, "fwS2Volt1"=2, "fwS2Volt2"=3, "fwS3Volt1"=4, "fwS3Volt2"=5, "fwS4Volt1"=6, "fwS4Volt2"=7, "fwS5Volt1"=8, "fwS5Volt2"=9, "fwS6Volt1"=10, "fwS6Volt2 "=11, "fwS7Volt1"=12, "fwS7Volt2"=13, "fwS8Volt1"=14, "fwS8Volt2"=15, "fwRoomHum"=16, "fwRoomTemp"=17, "fwAISpare1"=18, "fwAISpare2"=19, "fwSuppTemp"=20, "fwCoolTemp"=21, "fwDehumTemp"=22, "fwUnused"=23, "Bool Inputs"=24, "gwVoltRate1"=256, "gwVoltRate2"=257, "gwVoltRate3"=258, "gwVoltRate4"=259, "gwVoltRate5"=260, "gwVoltRate6"=261, "gwVoltRate7"=262, "gwVoltRate8"=263, "gwVoltWindow5/1"=264, "gwVoltWindow6/2"=265, "gwVoltWindow7/3"=266, "gwVoltWindow8/4"=267, "fwVoltSet1"=272, "fwVoltSet2"=273, "fwVoltSet3"=274, "fwVoltSet4"=275, "fwVoltSet5"=276, "fwVoltSet6"=277, "fwVoltSet7"=278, "fwVoltSet8"=279, "fwVoltRng1"=280, "fwVoltRng2"=281, "fwVoltRng3"=282, "fwVoltRng4"=283, "fwVoltRng5"=284, "fwVoltRng6"=285, "fwVoltRng7"=286, "fwVoltRng8"=287, "fwVoltPol1"=296, "fwVoltPol2"=297, "fwVoltPol3"=298, "fwVoltPol4"=299, "fwVoltPol5"=300, "fwVoltPol6"=301, "fwVoltPol7"=302, "fwVoltPol8"=303, "Rm1St1Dr1Cmd"=304, "Rm1St2Dr1Cmd"=305, "Rm1St3Dr1Cmd"=306, "Rm1St4Dr1Cmd"=307, "Rm1St5Dr1Cmd"=308, "Rm1St6Dr1Cmd"=309, "Rm1St7Dr1Cmd"=310, "Rm1St8Dr1Cmd"=311, "Rm1St1Dr2Cmd"=312, "Rm1St2Dr2Cmd"=313, "Rm1St3Dr2Cmd"=314, "Rm1St4Dr2Cmd"=315, "Rm1St5Dr2Cmd"=316, "Rm1St6Dr2Cmd"=317, "Rm1St7Dr2Cmd"=318, "Rm1St8Dr2Cmd"=319, "Rm1St1Dr3Cmd"=320, "Rm1St2Dr3Cmd"=321, "Rm1St3Dr3Cmd"=322, "Rm1St4Dr3Cmd"=323, "Rm1St5Dr3Cmd"=324, "Rm1St6Dr3Cmd"=325, "Rm1St7Dr3Cmd"=326, "Rm1St8Dr3Cmd"=327, "fwRmTempSP"=328, "fwRmHumSP"=329, "fwCoolTempSP"=330, "fwDehumTempSP"=331, "fwRmRun"=332, "fwRmOk"=333, "fwTesting"=334, "fwRmDryP"=335, "fwRmDryI"=336, "fwRmHumP"=337, "fwRmHumI"=338, "fwRmHeatP"=339, "fwRmHeatI"=340, "fwCoolTempP"=341, "fwCoolTempI"=342, "fwDehumTempP"=343, "fwDehumTempI"=344, "fwGndLeak1"=345, "fwGndLeak2"=346, "fwGndLeak3"=347, "fwGndLeak4"=348, "fwGndLeak5"=349, "fwGndLeak6"=350, "fwGndLeak7"=351, "fwGndLeak8"=352, "Rm1OpenerCmd"=353] ("Ring")
            n226 = event-data() -> ()  [unwired: 1 in, 6 out]
            n227 = Unbundle By Name(w593) -> ("Device Connections.Wago ModBus Connection"=w595:refnum<class "Modbus Master.lvclass">)
            n228 = call "Wago Input Output Converter.vi"("Input to Output?"=TRUE, "Input Command"=w599) -> ("Read Input Command Location"=w598:i32)  [unwired: 9 in]
            n229 = call-dynamic "Read Holding Registers.vi"("error in"=w591, "number of inputs"="Room Run", "starting address"=w598, "Modbus master in"=w595) -> ("error out"=w590:errorcluster, "Modbus master out"=w594:refnum<class "Modbus Master.lvclass">)  [unwired: 5 in, 1 out]
            n230 = Bundle By Name(cluster=w593, "Device Connections.Wago ModBus Connection"=w594) -> (w592:T55)
          }
          event Value Change {
            n231 = event-data() -> ("NewVal"=w602:T13)  [unwired: 1 in, 5 out]
            n232 = Bundle By Name(cluster=w604, "All Door Opener Ctrl"=w602) -> (w603:T55)
            n233 = call <vilib>:"Add State(s) to Queue__jki_lib_state_machine.vi"("State(s) in Front (\"\")"="Read Door Setup" ("State(s) in Front (\"\")"), "State(s) in (\"\")"=w606) -> ("States Out"=w607:string)  [unwired: 13 in]
          }
          event Panel Close? {
            # "Discard the event because we'll close the front panel ourselves in Macro: Exit"
            # "Close Panel button (pressed) Event\n(this executes Macro: Exit to terminate the VI)"
            n234 = event-data() -> ()  [unwired: 1 in, 1 out]
            n235 = event-data("Discard?"=TRUE) -> ()  [unwired: 1 in, 1 out]
            n236 = call <vilib>:"Add State(s) to Queue__jki_lib_state_machine.vi"("State(s) in Front (\"\")"="Macro: Exit", "State(s) in (\"\")"=w613) -> ("States Out"=w612:string)  [unwired: 13 in]
          }
        }
      }
      frame "---------- Core ----------" {
        # "Do not put any code in this frame.\n(it is a separator no-op)"
        n237 = call <vilib>:"Add State(s) to Queue__jki_lib_state_machine.vi"("State(s) in (\"\")"=w617) -> ("States Out"=w616:string)  [unwired: 14 in]
      }
      frame Default {
        w627 = 42 items=["No error", "Argument error", "Memory is full", "Out of zone", "End of file", "File already open", "Generic file I/O error", "File not found", "File permission error", "Disk is full", "Duplicate path", "Too many files open", "System feature not enabled", "Resource file not found", "Cannot add resource", "Resource not found", "Image not found", "Image memory error", "Pen does not exist", "Config type invalid", "Config token not found", "Config parse error", "Config memory error", "Bad external code format", "Bad external code offset", "External code not present", "Null window", "Destroy window error", "Null menu", "Print aborted", "Bad print record", "Print driver error", "Windows error during printing", "Memory error during printing", "Print dialog error", "Generic print error", "Invalid device refnum", "Device not found", "Device parameter error", "Device unit error", "Cannot open device", "Device call aborted", "Generic error", "Cancelled by user", "Object ID too low", "Object ID too high", "Object not in heap", "Unknown heap", "Unknown object (invalid DefProc)", "Unknown object (DefProc not in table)", "Message out of range", "Invalid (null) method", "Unknown message", "Manager call not supported", "Bad address", "Network operation in progress", "Network operation timed out", "Connection is busy", "Network attribute not supported", "Network error", "Address in use", "System out of memory", "Connection aborted", "Connection refused", "Not connected", "Already connected", "Connection closed", "Initialization error (interapplication manager)", "Bad occurrence", "Wait on unbound occurrence handler", "Occurrence queue overflow", "Datalog type conflict", "Unused", "Unrecognized type (interapplication manager)", "Memory corrupt", "Failed to make temporary DLL", "Old CIN version", "Drag socket not found", "Failed to load drop-object", "Failed to register OLE object", "Failed to release OLE object", "Format specifier type mismatch", "Unknown format specifier", "Too few format specifiers", "Too many format specifiers", "Scan failed", "Newer CIN version", "Error converting to variant", "Runtime menu error", "Password tampered", "Variant attribute not found", "Incompatible variant data type", "Event data is not available", "Event Store is not present", "Occurrence is not found", "Event Queue is not created", "Event info is not available", "Refnum passed is NULL", "Error retrieving Class GUID", "Error retrieving CoClass GUID", "Error retrieving TypeLib GUID.", "Bad built application magic bytes.", "Specific driver is different from the specific driver associated with the Logical Name.", "There is no session opened to the class driver.", "Max Error", "MAX - Error with config objects", "MAX - Error loading configuration", "MAX - Group not supported"]
        # "Current State"
        # "Do not delete, rename, or modify this frame.\n(this is used to capture unhandled states and typos)"
        # "Handle mistyped state name (developer tool)"
        n238 = Format Into String(format string="Software Exception: Unhandled State \"%s\"." ("message"), error in=w623, w618) -> (resulting string=w626:string, error out=w625:errorcluster)  [unwired: 1 in]
        n239 = call <vilib>:"Error Cluster From Error Code.vi"("show call chain? (False)"=TRUE, "error in (no error)"=w625, "error message (\"\")"=w626, "error code (0)"=w627) -> ("error out"=w624:errorcluster)  [unwired: 5 in]
        n240 = call <vilib>:"Add State(s) to Queue__jki_lib_state_machine.vi"("State(s) in (\"\")"=w622) -> ("States Out"=w621:string)  [unwired: 14 in]
      }
      frame "Initialize Core Data" {
        # "Do not delete, rename, or modify this frame.\n(this is used to determine panel behavior on exit)"
        # "originally closed?"
        # "exe?"
        # "If panel starts closed or is an EXE, then close it when we exit"
        n241 = property class="VI"() -> ("Front Panel.Open"=w636:bool)  [unwired: 2 in, 2 out]
        n242 = property class="App"() -> ("App.Kind"=w635:T51)  [unwired: 2 in, 2 out]
        n243 = control-ref of="Current VI Reference"() -> (w629:refnum<vi>)
        n244 = Not(x=w636) -> (.not. x?=w633:bool)
        n245 = Equal?(x=w635, y=T51."Run Time System" ("Application:Kind")) -> (x = y?=w632:bool)
        n246 = Or(x=w633, y=w632) -> (x .or. y?=w630:bool)
        n247 = Bundle By Name(cluster=w631, "Core.Current VI Reference"=w629, "Core.Close Panel on Exit?"=w630) -> (w638:T55)
        n248 = call <vilib>:"Add State(s) to Queue__jki_lib_state_machine.vi"("State(s) in (\"\")"=w640) -> ("States Out"=w639:string)  [unwired: 14 in]
      }
      frame "Error Handler" {
        # "Unhandled Error -- Display it"
        # "Handle any errors here.\nYou can also output any states to clean-up after errors occur"
        # "Clear error"
        n249 = call <vilib>:"General Error Handler.vi"("error in (no error)"=w641) -> ()  [unwired: 10 in, 5 out]
        n250 = Stop(stop? (T)=w641) -> ()
        n251 = call <vilib>:"Add State(s) to Queue__jki_lib_state_machine.vi"("State(s) in Front (\"\")"="/* Post Error States", "State(s) in (\"\")"=w646) -> ("States Out"=w645:string)  [unwired: 13 in]
      }
      frame "Exit" {
        w647 = TRUE
        # "Do not put any code in this frame.\n(No errors that occur here will be handled.)"
        n252 = call <vilib>:"Add State(s) to Queue__jki_lib_state_machine.vi"("State(s) in (\"\")"=w651) -> ("States Out"=w650:string)  [unwired: 14 in]
        "Exit" <- w647
      }
      frame "---------- Data ----------" {
        # "Do not put any code in this frame.\n(It is a separator no-op. You can make a copy of this frame to create a new Data frame)"
        n253 = call <vilib>:"Add State(s) to Queue__jki_lib_state_machine.vi"("State(s) in (\"\")"=w655) -> ("States Out"=w654:string)  [unwired: 14 in]
      }
      frame "Data: Initialize" {
        w656 = string[] []  # Custom Command
        w660 = string[][] []  # Send Data
        w661 = T21 {"Station 1"={"Current (A):Element 1"=0.0, "Current (A):Element 2"=0.0, "Power (W):Sigma"=0.0, "Watt Hours (Wh):Sigma"=0.0, "Voltage (V):Element 2"=0.0, "Voltage (V):Element 1"=0.0, "Current Crest Factor:Element 1"=0.0, "Current Crest Factor:Element 2"=0.0, "Voltage Harmonic (%):Element 1"=0.0, "Voltage Harmonic (%):Element 2"=0.0, "Voltage Crest Factor:Element 1"=0.0, "Voltage Crest Factor:Element 2"=0.0, "Time:Element 1"=0.0, "Frequency (Hz):Element 1"=0.0, "Apparent Power (VA):Element 1"=0.0, "Apparent Power (VA):Element 2"=0.0, "Power Factor:Element 1"=0.0, "Power Factor:Element 2"=0.0, "Max Watt Hours"=0.0, "Voltage (V):Element 2 Avg"=0.0, "Voltage (V):Element 1 Avg"=0.0}, "Station 2"={"Current (A):Element 1"=0.0, "Current (A):Element 2"=0.0, "Power (W):Sigma"=0.0, "Watt Hours (Wh):Sigma"=0.0, "Voltage (V):Element 2"=0.0, "Voltage (V):Element 1"=0.0, "Current Crest Factor:Element 1"=0.0, "Current Crest Factor:Element 2"=0.0, "Voltage Harmonic (%):Element 1"=0.0, "Voltage Harmonic (%):Element 2"=0.0, "Voltage Crest Factor:Element 1"=0.0, "Voltage Crest Factor:Element 2"=0.0, "Time:Element 1"=0.0, "Frequency (Hz):Element 1"=0.0, "Apparent Power (VA):Element 1"=0.0, "Apparent Power (VA):Element 2"=0.0, "Power Factor:Element 1"=0.0, "Power Factor:Element 2"=0.0, "Max Watt Hours"=0.0, "Voltage (V):Element 2 Avg"=0.0, "Voltage (V):Element 1 Avg"=0.0}, "Station 3"={"Current (A):Element 1"=0.0, "Current (A):Element 2"=0.0, "Power (W):Sigma"=0.0, "Watt Hours (Wh):Sigma"=0.0, "Voltage (V):Element 2"=0.0, "Voltage (V):Element 1"=0.0, "Current Crest Factor:Element 1"=0.0, "Current Crest Factor:Element 2"=0.0, "Voltage Harmonic (%):Element 1"=0.0, "Voltage Harmonic (%):Element 2"=0.0, "Voltage Crest Factor:Element 1"=0.0, "Voltage Crest Factor:Element 2"=0.0, "Time:Element 1"=0.0, "Frequency (Hz):Element 1"=0.0, "Apparent Power (VA):Element 1"=0.0, "Apparent Power (VA):Element 2"=0.0, "Power Factor:Element 1"=0.0, "Power Factor:Element 2"=0.0, "Max Watt Hours"=0.0, "Voltage (V):Element 2 Avg"=0.0, "Voltage (V):Element 1 Avg"=0.0}, "Station 4"={"Current (A):Element 1"=0.0, "Current (A):Element 2"=0.0, "Power (W):Sigma"=0.0, "Watt Hours (Wh):Sigma"=0.0, "Voltage (V):Element 2"=0.0, "Voltage (V):Element 1"=0.0, "Current Crest Factor:Element 1"=0.0, "Current Crest Factor:Element 2"=0.0, "Voltage Harmonic (%):Element 1"=0.0, "Voltage Harmonic (%):Element 2"=0.0, "Voltage Crest Factor:Element 1"=0.0, "Voltage Crest Factor:Element 2"=0.0, "Time:Element 1"=0.0, "Frequency (Hz):Element 1"=0.0, "Apparent Power (VA):Element 1"=0.0, "Apparent Power (VA):Element 2"=0.0, "Power Factor:Element 1"=0.0, "Power Factor:Element 2"=0.0, "Max Watt Hours"=0.0, "Voltage (V):Element 2 Avg"=0.0, "Voltage (V):Element 1 Avg"=0.0}, "Station 5"={"Current (A):Element 1"=0.0, "Current (A):Element 2"=0.0, "Power (W):Sigma"=0.0, "Watt Hours (Wh):Sigma"=0.0, "Voltage (V):Element 2"=0.0, "Voltage (V):Element 1"=0.0, "Current Crest Factor:Element 1"=0.0, "Current Crest Factor:Element 2"=0.0, "Voltage Harmonic (%):Element 1"=0.0, "Voltage Harmonic (%):Element 2"=0.0, "Voltage Crest Factor:Element 1"=0.0, "Voltage Crest Factor:Element 2"=0.0, "Time:Element 1"=0.0, "Frequency (Hz):Element 1"=0.0, "Apparent Power (VA):Element 1"=0.0, "Apparent Power (VA):Element 2"=0.0, "Power Factor:Element 1"=0.0, "Power Factor:Element 2"=0.0, "Max Watt Hours"=0.0, "Voltage (V):Element 2 Avg"=0.0, "Voltage (V):Element 1 Avg"=0.0}, "Station 6"={"Current (A):Element 1"=0.0, "Current (A):Element 2"=0.0, "Power (W):Sigma"=0.0, "Watt Hours (Wh):Sigma"=0.0, "Voltage (V):Element 2"=0.0, "Voltage (V):Element 1"=0.0, "Current Crest Factor:Element 1"=0.0, "Current Crest Factor:Element 2"=0.0, "Voltage Harmonic (%):Element 1"=0.0, "Voltage Harmonic (%):Element 2"=0.0, "Voltage Crest Factor:Element 1"=0.0, "Voltage Crest Factor:Element 2"=0.0, "Time:Element 1"=0.0, "Frequency (Hz):Element 1"=0.0, "Apparent Power (VA):Element 1"=0.0, "Apparent Power (VA):Element 2"=0.0, "Power Factor:Element 1"=0.0, "Power Factor:Element 2"=0.0, "Max Watt Hours"=0.0, "Voltage (V):Element 2 Avg"=0.0, "Voltage (V):Element 1 Avg"=0.0}, "Station 7"={"Current (A):Element 1"=0.0, "Current (A):Element 2"=0.0, "Power (W):Sigma"=0.0, "Watt Hours (Wh):Sigma"=0.0, "Voltage (V):Element 2"=0.0, "Voltage (V):Element 1"=0.0, "Current Crest Factor:Element 1"=0.0, "Current Crest Factor:Element 2"=0.0, "Voltage Harmonic (%):Element 1"=0.0, "Voltage Harmonic (%):Element 2"=0.0, "Voltage Crest Factor:Element 1"=0.0, "Voltage Crest Factor:Element 2"=0.0, "Time:Element 1"=0.0, "Frequency (Hz):Element 1"=0.0, "Apparent Power (VA):Element 1"=0.0, "Apparent Power (VA):Element 2"=0.0, "Power Factor:Element 1"=0.0, "Power Factor:Element 2"=0.0, "Max Watt Hours"=0.0, "Voltage (V):Element 2 Avg"=0.0, "Voltage (V):Element 1 Avg"=0.0}, "Station 8"={"Current (A):Element 1"=0.0, "Current (A):Element 2"=0.0, "Power (W):Sigma"=0.0, "Watt Hours (Wh):Sigma"=0.0, "Voltage (V):Element 2"=0.0, "Voltage (V):Element 1"=0.0, "Current Crest Factor:Element 1"=0.0, "Current Crest Factor:Element 2"=0.0, "Voltage Harmonic (%):Element 1"=0.0, "Voltage Harmonic (%):Element 2"=0.0, "Voltage Crest Factor:Element 1"=0.0, "Voltage Crest Factor:Element 2"=0.0, "Time:Element 1"=0.0, "Frequency (Hz):Element 1"=0.0, "Apparent Power (VA):Element 1"=0.0, "Apparent Power (VA):Element 2"=0.0, "Power Factor:Element 1"=0.0, "Power Factor:Element 2"=0.0, "Max Watt Hours"=0.0, "Voltage (V):Element 2 Avg"=0.0, "Voltage (V):Element 1 Avg"=0.0}, "Station 1 TCs"={"TC 1"=0.0, "TC 2"=0.0, "TC 3"=0.0, "TC 4"=0.0, "TC 5"=0.0, "TC 6"=0.0, "TC 7"=0.0, "TC 8"=0.0, "TC 9"=0.0, "TC 10"=0.0, "TC 11"=0.0, "TC 12"=0.0, "TC 13"=0.0, "TC 14"=0.0, "TC 15"=0.0, "TC 16"=0.0, "TC 17"=0.0, "TC 18"=0.0, "TC 19"=0.0, "TC 20"=0.0, "TC 21"=0.0, "TC 22"=0.0, "TC 23"=0.0, "TC 24"=0.0, "TC 25"=0.0, "TC 26"=0.0, "TC 27"=0.0, "TC 28"=0.0, "TC 29"=0.0, "TC 30"=0.0}, "Station 2 TCs"={"TC 1"=0.0, "TC 2"=0.0, "TC 3"=0.0, "TC 4"=0.0, "TC 5"=0.0, "TC 6"=0.0, "TC 7"=0.0, "TC 8"=0.0, "TC 9"=0.0, "TC 10"=0.0, "TC 11"=0.0, "TC 12"=0.0, "TC 13"=0.0, "TC 14"=0.0, "TC 15"=0.0, "TC 16"=0.0, "TC 17"=0.0, "TC 18"=0.0, "TC 19"=0.0, "TC 20"=0.0, "TC 21"=0.0, "TC 22"=0.0, "TC 23"=0.0, "TC 24"=0.0, "TC 25"=0.0, "TC 26"=0.0, "TC 27"=0.0, "TC 28"=0.0, "TC 29"=0.0, "TC 30"=0.0}, "Station 3 TCs"={"TC 1"=0.0, "TC 2"=0.0, "TC 3"=0.0, "TC 4"=0.0, "TC 5"=0.0, "TC 6"=0.0, "TC 7"=0.0, "TC 8"=0.0, "TC 9"=0.0, "TC 10"=0.0, "TC 11"=0.0, "TC 12"=0.0, "TC 13"=0.0, "TC 14"=0.0, "TC 15"=0.0, "TC 16"=0.0, "TC 17"=0.0, "TC 18"=0.0, "TC 19"=0.0, "TC 20"=0.0, "TC 21"=0.0, "TC 22"=0.0, "TC 23"=0.0, "TC 24"=0.0, "TC 25"=0.0, "TC 26"=0.0, "TC 27"=0.0, "TC 28"=0.0, "TC 29"=0.0, "TC 30"=0.0}, "Station 4 TCs"={"TC 1"=0.0, "TC 2"=0.0, "TC 3"=0.0, "TC 4"=0.0, "TC 5"=0.0, "TC 6"=0.0, "TC 7"=0.0, "TC 8"=0.0, "TC 9"=0.0, "TC 10"=0.0, "TC 11"=0.0, "TC 12"=0.0, "TC 13"=0.0, "TC 14"=0.0, "TC 15"=0.0, "TC 16"=0.0, "TC 17"=0.0, "TC 18"=0.0, "TC 19"=0.0, "TC 20"=0.0, "TC 21"=0.0, "TC 22"=0.0, "TC 23"=0.0, "TC 24"=0.0, "TC 25"=0.0, "TC 26"=0.0, "TC 27"=0.0, "TC 28"=0.0, "TC 29"=0.0, "TC 30"=0.0}, "Station 5 TCs"={"TC 1"=0.0, "TC 2"=0.0, "TC 3"=0.0, "TC 4"=0.0, "TC 5"=0.0, "TC 6"=0.0, "TC 7"=0.0, "TC 8"=0.0, "TC 9"=0.0, "TC 10"=0.0, "TC 11"=0.0, "TC 12"=0.0, "TC 13"=0.0, "TC 14"=0.0, "TC 15"=0.0, "TC 16"=0.0, "TC 17"=0.0, "TC 18"=0.0, "TC 19"=0.0, "TC 20"=0.0, "TC 21"=0.0, "TC 22"=0.0, "TC 23"=0.0, "TC 24"=0.0, "TC 25"=0.0, "TC 26"=0.0, "TC 27"=0.0, "TC 28"=0.0, "TC 29"=0.0, "TC 30"=0.0}, "Station 6 TCs"={"TC 1"=0.0, "TC 2"=0.0, "TC 3"=0.0, "TC 4"=0.0, "TC 5"=0.0, "TC 6"=0.0, "TC 7"=0.0, "TC 8"=0.0, "TC 9"=0.0, "TC 10"=0.0, "TC 11"=0.0, "TC 12"=0.0, "TC 13"=0.0, "TC 14"=0.0, "TC 15"=0.0, "TC 16"=0.0, "TC 17"=0.0, "TC 18"=0.0, "TC 19"=0.0, "TC 20"=0.0, "TC 21"=0.0, "TC 22"=0.0, "TC 23"=0.0, "TC 24"=0.0, "TC 25"=0.0, "TC 26"=0.0, "TC 27"=0.0, "TC 28"=0.0, "TC 29"=0.0, "TC 30"=0.0}, "Station 7 TCs"={"TC 1"=0.0, "TC 2"=0.0, "TC 3"=0.0, "TC 4"=0.0, "TC 5"=0.0, "TC 6"=0.0, "TC 7"=0.0, "TC 8"=0.0, "TC 9"=0.0, "TC 10"=0.0, "TC 11"=0.0, "TC 12"=0.0, "TC 13"=0.0, "TC 14"=0.0, "TC 15"=0.0, "TC 16"=0.0, "TC 17"=0.0, "TC 18"=0.0, "TC 19"=0.0, "TC 20"=0.0, "TC 21"=0.0, "TC 22"=0.0, "TC 23"=0.0, "TC 24"=0.0, "TC 25"=0.0, "TC 26"=0.0, "TC 27"=0.0, "TC 28"=0.0, "TC 29"=0.0, "TC 30"=0.0}, "Station 8 TCs"={"TC 1"=0.0, "TC 2"=0.0, "TC 3"=0.0, "TC 4"=0.0, "TC 5"=0.0, "TC 6"=0.0, "TC 7"=0.0, "TC 8"=0.0, "TC 9"=0.0, "TC 10"=0.0, "TC 11"=0.0, "TC 12"=0.0, "TC 13"=0.0, "TC 14"=0.0, "TC 15"=0.0, "TC 16"=0.0, "TC 17"=0.0, "TC 18"=0.0, "TC 19"=0.0, "TC 20"=0.0, "TC 21"=0.0, "TC 22"=0.0, "TC 23"=0.0, "TC 24"=0.0, "TC 25"=0.0, "TC 26"=0.0, "TC 27"=0.0, "TC 28"=0.0, "TC 29"=0.0, "TC 30"=0.0}, "MX 5 (AUX Data)"={"AUX 1_1"=0.0, "AUX 1_2"=0.0, "AUX 2_1"=0.0, "AUX 2_2"=0.0, "AUX 3_1"=0.0, "AUX 3_2"=0.0, "AUX 4_1"=0.0, "AUX 4_2"=0.0, "AUX 5_1"=0.0, "AUX 5_2"=0.0, "AUX 6_1"=0.0, "AUX 6_2"=0.0, "AUX 7_1"=0.0, "AUX 7_2"=0.0, "AUX 8_1"=0.0, "AUX 8_2"=0.0, "CAL CL1S"=0.0, "CAL CL2S"=0.0, "CAL CL3S"=0.0, "CAL CL4S"=0.0, "CAL CL5"=0.0, "CAL CL6"=0.0, "CAL CL7"=0.0, "CAL CL8"=0.0}, "Door Output Relays"={"Station 1 Freezer"=FALSE, "Station 1 Cab"=FALSE, "Station 1 Slide"=FALSE, "Station 2 Freezer"=FALSE, "Station 2 Cab"=FALSE, "Station 2 Slide"=FALSE, "Station 3 Freezer"=FALSE, "Station 3 Cab"=FALSE, "Station 3 Slide"=FALSE, "Station 4 Freezer"=FALSE, "Station 4 Cab"=FALSE, "Station 4 Slide"=FALSE, "Station 5 Freezer"=FALSE, "Station 5 Cab"=FALSE, "Station 5 Slide"=FALSE, "Station 6 Freezer"=FALSE, "Station 6 Cab"=FALSE, "Station 6 Slide"=FALSE, "Station 7 Freezer"=FALSE, "Station 7 Cab"=FALSE, "Station 7 Slide"=FALSE, "Station 8 Freezer"=FALSE, "Station 8 Cab"=FALSE, "Station 8 Slide"=FALSE, "Door Opener Enable"=FALSE}, "Contactor Settings(*All Check Out)"={"Station 1"={"60 Hz Power"=FALSE, "50 Hz Power"=FALSE, "120V Range"=FALSE, "240V Range"=FALSE, "Ground Line"=FALSE, "Ground Neutral"=FALSE, "Room OK"=FALSE, "Ground Leakage"=enum."0 - Normal GL"}, "Station 2"={"60 Hz Power"=FALSE, "50 Hz Power"=FALSE, "120V Range"=FALSE, "240V Range"=FALSE, "Ground Line"=FALSE, "Ground Neutral"=FALSE, "Fault"=FALSE, "Ground Leakage"=enum."0 - Normal GL"}, "Station 3"={"60 Hz Power"=FALSE, "50 Hz Power"=FALSE, "120V Range"=FALSE, "240V Range"=FALSE, "Ground Line"=FALSE, "Ground Neutral"=FALSE, "Room Heat"=FALSE, "Ground Leakage"=enum."0 - Normal GL"}, "Station 4"={"60 Hz Power"=FALSE, "50 Hz Power"=FALSE, "120V Range"=FALSE, "240V Range"=FALSE, "Ground Line"=FALSE, "Ground Neutral"=FALSE, "Room Blower"=FALSE, "Ground Leakage"=enum."0 - Normal GL"}, "Station 5"={"60 Hz Power"=FALSE, "50 Hz Power"=FALSE, "120V Range"=FALSE, "240V Range"=FALSE, "Ground Line"=FALSE, "Ground Neutral"=FALSE, "Spare"=FALSE, "Ground Leakage"=enum."0 - Normal GL"}, "Station 6"={"60 Hz Power"=FALSE, "50 Hz Power"=FALSE, "120V Range"=FALSE, "240V Range"=FALSE, "Ground Line"=FALSE, "Ground Neutral"=FALSE, "Room Pump"=FALSE, "Ground Leakage"=enum."0 - Normal GL"}, "Station 7"={"60 Hz Power"=FALSE, "50 Hz Power"=FALSE, "120V Range"=FALSE, "240V Range"=FALSE, "Ground Line"=FALSE, "Ground Neutral"=FALSE, "Spare"=FALSE, "Ground Leakage"=enum."0 - Normal GL"}, "Station 8"={"60 Hz Power"=FALSE, "50 Hz Power"=FALSE, "120V Range"=FALSE, "240V Range"=FALSE, "Ground Line"=FALSE, "Ground Neutral"=FALSE, "Spare"=FALSE, "Ground Leakage"=enum."0 - Normal GL"}}, "Measured Input Data (Target)"={"Voltage Setpoint 1 (*Volt Set1)"=0.0, "Voltage Setpoint 2 (*Volt Set2)"=0.0, "Voltage Setpoint 3 (*Volt Set3)"=0.0, "Voltage Setpoint 4 (*Volt Set4)"=0.0, "Voltage Setpoint 5 (*Volt Set5)"=0.0, "Voltage Setpoint 6 (*Volt Set6)"=0.0, "Voltage Setpoint 7 (*Volt Set7)"=0.0, "Voltage Setpoint 8 (*Volt Set8)"=0.0, "Room Setpoints"={"Room Setpoint Temperature (*RM Dry Set P1)"=0.0, "Room Setpoint Humidity (*RM Hum Set P1)"=0.0, "Room Cool Temperature (*RM Cool Setp 1)"=0.0, "Room Dehum Temperature (*RM De Hum Set P1)"=0.0}}, "Room PID Settings"={"Room Dry P(*RM Dry P1)"=0, "Room Dry I (*RM Dry I1)"=0, "Room Humidity P (*RM Hum P1)"=0, "Room Humidity I (*RM Hum I1)"=0, "Room Heat P (*RM Heat P1)"=0, "Room Heat I (*RM Heat I1)"=0, "Room Cool Temperature P (*RM Cool P1)"=0, "Room Cool Temperature I (*RM Cool I1)"=0, "Room Dehumid Temperature P (*RM Dehum P1)"=0, "Room Dehumid Temperature I (*RM Dehum I1)"=0}, "Room Conditions (Measured)"={"twDoorEna(*Door Enable)"=0, "twStatus(*Rm Status1)"=0, "twRoomTemp (*Rm Dry1)"=0.0, "twRoomHum (*Rm Hum1)"=0.0, "twSuppTemp(*Rm Supp T1)"=0.0, "twCoolTemp(*Rm Cool T1)"=0.0, "twDehumTemp(*Rm Dehum T1)"=0.0, "twGlycolTemp(*Rm Gly T1-Not Used)"=0.0, "twDehumRate(*Rm Dehum Valve1)"=0.0, "twCoolRate(*Rm Cool Valve1)"=0.0, "twSteamRate(*Rm Steam Valve1)"=0.0, "twHeatRate (*Rm Heat Ctrl1)"=0.0}, "APLUS System Headers"=[], "MX100 System Headers"=[], "Wago System Headers"=[]}  # Chamber Data
        w663 = u16 502  # Modbus Remote Port
        w662 = T54 {"Clients"=[], "Listener"=refnum, "Data Array"=[]}  # Data
        w666 = T57 {"Current VI Reference"=refnum, "Close Panel on Exit?"=FALSE}  # Core
        n254 = Bundle("Core"=w666, "Wago Data Input"="Wago Data Input", "Device Connections"="Device Connections", "Modbus Remote Port"=w663, "Chamber Data"=w661, "Data"=w662, "RTS Config Setup"=T4 {"Wago RTS"={"Disable"=0, "Interval"=0, "Controller"=0, "Address"=0, "IP Address"="", "AtoDmax"=0, "FullScale"=0, "VoltageType"=0, "Window1"=0, "Control1"=0, "Window2"=0, "Control2"=0}, "APLUS Array"=[], "Yokogawa MX100 RTS Array"=[], "Replay Server"=[], "Server Configuration Array"=[], "Station Settings"={"Point Files"={"Point File 1"=path "", "Point File 2"=path "", "Point File 3"=path "", "Point File 4"=path "", "Point File 5"=path "", "Point File 6"=path "", "Point File 7"=path "", "Point File 8"=path ""}, "Save Status"={"Save Status 1"=FALSE, "Save Status 2"=FALSE, "Save Status 3"=FALSE, "Save Status 4"=FALSE, "Save Status 5"=FALSE, "Save Status 6"=FALSE, "Save Status 7"=FALSE, "Save Status 8"=FALSE}, "Setup Info"={"Setup Info Station 1"=[], "Setup Info Station 2"=[], "Setup Info Station 3"=[], "Setup Info Station 4"=[], "Setup Info Station 5"=[], "Setup Info Station 6"=[], "Setup Info Station 7"=[], "Setup Info Station 8"=[]}, "Chamber Test Pattern"={" Pattern 1"=path "", "Pattern 2"=path "", "Pattern 3"=path "", "Pattern 4"=path "", "Pattern 5"=path "", "Pattern 6"=path "", "Pattern 7"=path "", "Pattern 8"=path ""}}}, "Send Data"=w660, "CSV Data Save"="CSV Data Save", "All Door Opener Ctrl"=T13 {"Station 1"={"Station Freezer"={"Time Count (s)"=2.941037178039551, "Status"="Delay", "Door State"=FALSE, "Delay"=TRUE, "Chamber 1-1"=[], "Index"=0, "Delay Status"=""}, "Station Cab"={"Time Count (s)"=1.00654935836792, "Status"="Door Closed", "Door State"=FALSE, "Delay"=FALSE, "Chamber 1-1"=[], "Index"=0, "Delay Status"=""}, "Station Slide"={"Time Count (s)"=14.805169582366943, "Status"="Delay", "Door State"=FALSE, "Delay"=TRUE, "Chamber 1-1"=[], "Index"=0, "Delay Status"=""}, "1st Complete"=TRUE, "2nd Complete"=FALSE, "3rd Complete"=FALSE}, "Station 2"={"Station Freezer"={"Time Count (s)"=5.893074989318848, "Status"="Door Closed", "Door State"=FALSE, "Delay"=TRUE, "Chamber 1-1"=[], "Index"=0, "Delay Status"=""}, "Station Cab"={"Time Count (s)"=0.9960207939147949, "Status"="Delay", "Door State"=FALSE, "Delay"=TRUE, "Chamber 1-1"=[], "Index"=0, "Delay Status"=""}, "Station Slide"={"Time Count (s)"=0.9960207939147949, "Status"="Delay", "Door State"=FALSE, "Delay"=TRUE, "Chamber 1-1"=[], "Index"=0, "Delay Status"=""}, "1st Complete"=FALSE, "2nd Complete"=FALSE, "3rd Complete"=FALSE}, "Station 3"={"Station Freezer"={"Time Count (s)"=0.9955215454101562, "Status"="Delay", "Door State"=FALSE, "Delay"=TRUE, "Chamber 1-1"=[], "Index"=0, "Delay Status"=""}, "Station Cab"={"Time Count (s)"=0.9955215454101562, "Status"="Delay", "Door State"=FALSE, "Delay"=FALSE, "Chamber 1-1"=[], "Index"=0, "Delay Status"=""}, "Station Slide"={"Time Count (s)"=14.805142879486084, "Status"="Delay", "Door State"=FALSE, "Delay"=TRUE, "Chamber 1-1"=[], "Index"=0, "Delay Status"=""}, "1st Complete"=TRUE, "2nd Complete"=FALSE, "3rd Complete"=FALSE}, "Station 4"={"Station Freezer"={"Time Count (s)"=5.8854570388793945, "Status"="Door Closed", "Door State"=FALSE, "Delay"=TRUE, "Chamber 1-1"=[], "Index"=0, "Delay Status"=""}, "Station Cab"={"Time Count (s)"=0.9955201148986816, "Status"="Delay", "Door State"=FALSE, "Delay"=TRUE, "Chamber 1-1"=[], "Index"=0, "Delay Status"=""}, "Station Slide"={"Time Count (s)"=0.0, "Status"="Delay", "Door State"=FALSE, "Delay"=TRUE, "Chamber 1-1"=[], "Index"=0, "Delay Status"=""}, "1st Complete"=FALSE, "2nd Complete"=FALSE, "3rd Complete"=FALSE}, "Station 5"={"Station Freezer"={"Time Count (s)"=0.9955196380615234, "Status"="Delay", "Door State"=FALSE, "Delay"=TRUE, "Chamber 1-1"=[], "Index"=0, "Delay Status"=""}, "Station Cab"={"Time Count (s)"=0.0, "Status"="Delay", "Door State"=FALSE, "Delay"=FALSE, "Chamber 1-1"=[], "Index"=0, "Delay Status"=""}, "Station Slide"={"Time Count (s)"=14.805170059204102, "Status"="Delay", "Door State"=FALSE, "Delay"=TRUE, "Chamber 1-1"=[], "Index"=0, "Delay Status"=""}, "1st Complete"=TRUE, "2nd Complete"=FALSE, "3rd Complete"=FALSE}, "Station 6"={"Station Freezer"={"Time Count (s)"=5.8724236488342285, "Status"="Door Closed", "Door State"=FALSE, "Delay"=TRUE, "Chamber 1-1"=[], "Index"=0, "Delay Status"=""}, "Station Cab"={"Time Count (s)"=0.9950180053710938, "Status"="Delay", "Door State"=FALSE, "Delay"=FALSE, "Chamber 1-1"=[], "Index"=0, "Delay Status"=""}, "Station Slide"={"Time Count (s)"=0.0, "Status"="Delay", "Door State"=FALSE, "Delay"=FALSE, "Chamber 1-1"=[], "Index"=0, "Delay Status"=""}, "1st Complete"=TRUE, "2nd Complete"=FALSE, "3rd Complete"=FALSE}, "Station 7"={"Station Freezer"={"Time Count (s)"=0.0, "Status"="Delay", "Door State"=FALSE, "Delay"=FALSE, "Chamber 1-1"=[], "Index"=0, "Delay Status"=""}, "Station Cab"={"Time Count (s)"=0.0, "Status"="Delay", "Door State"=FALSE, "Delay"=FALSE, "Chamber 1-1"=[], "Index"=0, "Delay Status"=""}, "Station Slide"={"Time Count (s)"=14.80466890335083, "Status"="Delay", "Door State"=FALSE, "Delay"=FALSE, "Chamber 1-1"=[], "Index"=0, "Delay Status"=""}, "1st Complete"=TRUE, "2nd Complete"=FALSE, "3rd Complete"=FALSE}, "Station 8"={"Station Freezer"={"Time Count (s)"=5.860893726348877, "Status"="Door Closed", "Door State"=FALSE, "Delay"=FALSE, "Chamber 1-1"=[], "Index"=0, "Delay Status"=""}, "Station Cab"={"Time Count (s)"=0.0, "Status"="Delay", "Door State"=FALSE, "Delay"=FALSE, "Chamber 1-1"=[], "Index"=0, "Delay Status"=""}, "Station Slide"={"Time Count (s)"=0.0, "Status"="Delay", "Door State"=FALSE, "Delay"=FALSE, "Chamber 1-1"=[], "Index"=0, "Delay Status"=""}, "1st Complete"=TRUE, "2nd Complete"=FALSE, "3rd Complete"=FALSE}}, "Custom Command"=w656) -> (w668:T55)  [unwired: 1 in]
        n255 = call <vilib>:"Add State(s) to Queue__jki_lib_state_machine.vi"("State(s) in (\"\")"=w670) -> ("States Out"=w669:string)  [unwired: 14 in]
      }
      frame "Data: Cleanup" {
        # "Cleanup any data and references, here.\n(this is called automatically, by the Macro: Exit)"
        n256 = Unbundle By Name(w672) -> ("Core.Current VI Reference"=w674:refnum<vi>)
        n257 = Close Reference(reference=w674, error in (no error)=w673) -> (error out=w671:errorcluster)
        n258 = call <vilib>:"Add State(s) to Queue__jki_lib_state_machine.vi"("State(s) in (\"\")"=w676) -> ("States Out"=w675:string)  [unwired: 14 in]
      }
      frame "---------- UI ----------" {
        # "Do not put any code in this frame.\n(It is a separator no-op. You can make a copy of this frame to create a new UI frame)"
        n259 = call <vilib>:"Add State(s) to Queue__jki_lib_state_machine.vi"("State(s) in (\"\")"=w680) -> ("States Out"=w679:string)  [unwired: 14 in]
      }
      frame "UI: Initialize" {
        # "Need to build different versions listening on \ndifferent ports"
        n260 = Unbundle By Name(w685) -> ("RTS Config Setup.Server Configuration Array"=w684:T9[])
        n261 = local write "Chamber 1 Connections"(0 ("# of Connections")) -> ()
        n262 = Index Array(array=w684, index=0) -> (element=w682:T9)
        n263 = Unbundle By Name(w682) -> ("TcpIP"=w681:u16)
        n264 = TCP Create Listener(8:w689, 10:w681) -> (0:w688:errorcluster, 3:w686:refnum<k5>)  [unwired: 4 out]
        n265 = Bundle By Name(cluster=w685, "Data.Listener"=w686) -> (w687:T55)
        n266 = call <vilib>:"Add State(s) to Queue__jki_lib_state_machine.vi"("State(s) in (\"\")"=w692) -> ("States Out"=w691:string)  [unwired: 14 in]
      }
      frame "UI: Cursor Set" {
        # "Argument"
        # "Set and Unset Cursor Busy.\n(Usage: \"UI: Cursor Set >> Busy|Idle\")"
        n267 = case shown="\"Idle\", Default" w693 {
          tunnel: w695 -> [w700 w702]
          tunnel: [w699 w701] -> w694
          frame "Idle", Default {
            n268 = call <vilib>:"Unset Busy.vi"("error in (no error)"=w700) -> ("error out"=w699:errorcluster)  [unwired: 10 in]
          }
          frame "Busy" {
            n269 = call <vilib>:"Set Busy.vi"("error in (no error)"=w702) -> ("error out"=w701:errorcluster)  [unwired: 9 in, 1 out]
          }
        }
        n270 = call <vilib>:"Add State(s) to Queue__jki_lib_state_machine.vi"("State(s) in (\"\")"=w698) -> ("States Out"=w697:string)  [unwired: 14 in]
      }
      frame "UI: Front Panel State" {
        # "Argument"
        # "Set Front Panel Open or Closed\n(Usage: \"UI: Front Panel State >> Open|Close\")"
        n271 = Unbundle By Name(w705) -> ("Core.Current VI Reference"=w704:refnum<vi>)
        n272 = case shown="\"Open\", Default" w703 {
          tunnel: w707 -> [w713 w726]
          tunnel: [w715 w727] -> w706
          tunnel: w704 -> [w714 w724]
          frame "Open", Default {
            n273 = property class="VI"(reference=w714, error in=w713) -> (reference out=w711:refnum<vi>, error out=w712:errorcluster, "Front Panel.Open"=w710:bool)
            n274 = case shown="True" w710 {
              tunnel: [w718 w721] -> w715
              tunnel: w712 -> [w717 w721]
              tunnel: w711 -> [w716 _]
              frame False {
                n275 = invoke class="VI" method="FP.Open"(reference=w716, error in=w717, "Activate"=TRUE, "State"=T52."Standard") -> (error out=w718:errorcluster)  [unwired: 1 in, 4 out]
              }
              frame True {
              }
            }
          }
          frame "Close" {
            n276 = property class="VI"(reference=w724, error in=w726) -> (reference out=w723:refnum<vi>, error out=w725:errorcluster, "Front Panel.Open"=w722:bool)
            n277 = case shown="True" w722 {
              tunnel: [w728 w731] -> w727
              tunnel: w725 -> [w728 w730]
              tunnel: w723 -> [_ w729]
              frame False {
              }
              frame True {
                n278 = invoke class="VI" method="FP.Close"(reference=w729, error in=w730) -> (error out=w731:errorcluster)  [unwired: 1 in, 2 out]
              }
            }
          }
        }
        n279 = call <vilib>:"Add State(s) to Queue__jki_lib_state_machine.vi"("State(s) in (\"\")"=w709) -> ("States Out"=w708:string)  [unwired: 14 in]
      }
      frame "Read Config Files" {
        w732 = T19 "Sys1" ("System Number")
        n280 = call "RTS Read Configuration Files.vi"("System Number"=w732, "Error In"=w738, "Core System Path"="Core System Path") -> ("Error Out"=w737:errorcluster, "RTS Config Setup Output"=w734:T4)  [unwired: 7 in]
        "RTS Config Setup Output" <- w734
        n281 = Bundle By Name(cluster=w736, "RTS Config Setup"=w734) -> (w735:T55)
        n282 = call <vilib>:"Add State(s) to Queue__jki_lib_state_machine.vi"("State(s) in (\"\")"=w740) -> ("States Out"=w739:string)  [unwired: 14 in]
        "System Number" <- w732
      }
      frame "Open Wago Connection" {
        n283 = Unbundle By Name(w744) -> ("RTS Config Setup.Wago RTS.IP Address"=w741:string, "Modbus Remote Port"=w743:u16)
        n284 = call-poly <vilib>:"Create Modbus Instance.vi"("error in"=w746, "port (502)"=w743, "address"=w741) -> ("error out"=w745:errorcluster, "TCP master instance"=w742:refnum<class "Modbus Master.lvclass">)  [unwired: 7 in]
        n285 = Bundle By Name(cluster=w744, "Device Connections.Wago ModBus Connection"=w742) -> (w747:T55)
        n286 = call <vilib>:"Add State(s) to Queue__jki_lib_state_machine.vi"("State(s) in (\"\")"=w749) -> ("States Out"=w748:string)  [unwired: 14 in]
      }
      frame "Open TDMS" {
        n287 = Unbundle By Name(w751) -> ("CSV Data Save"=w750:T2)
        n288 = disable-structure shown="Enabled" {
          disable-tunnel: w755 -> [w761 w762]
          disable-tunnel: [w760 w762] -> w753
          disable-tunnel: [w759 w763] -> w752
          disable-tunnel: w750 -> [w758 w763]
          frame Disabled {
            n289 = call "RTS Open All TDMS Files.vi"("error in (no error)"=w761, "TDMS Data Save Input"=w758) -> ("error out"=w760:errorcluster, "TDMS Data Save Output"=w759:T2)  [unwired: 8 in]
          }
          frame Enabled {
          }
        }
        n290 = Bundle By Name(cluster=w751, "CSV Data Save"=w752) -> (w754:T55)
        n291 = call <vilib>:"Add State(s) to Queue__jki_lib_state_machine.vi"("State(s) in (\"\")"=w757) -> ("States Out"=w756:string)  [unwired: 14 in]
      }
      frame "Close TDMS" {
        # "Build a Control for returning data from client...\nadd the station number"
        n292 = Unbundle By Name(w769) -> ("RTS Config Setup"=w764:T4, "CSV Data Save"=w768:T2)
        n293 = disable-structure shown="Enabled" {
          disable-tunnel: w768 -> [w778 _]
          disable-tunnel: w767 -> [w777 w779]
          disable-tunnel: [w776 w779] -> w766
          disable-tunnel: [w775 w780] -> w765
          disable-tunnel: w764 -> [w774 w780]
          frame Disabled {
            n294 = call "RTS Close TDMS.vi"("RTS Config Setup Input"=w774, "Error In"=w777, "Tree Selection"="1-1" ("Station ID"), "TDMS Data Save in"=w778) -> ("Error Out"=w776:errorcluster, "RTS Config Setup Output"=w775:T4)  [unwired: 6 in]
          }
          frame Enabled {
          }
        }
        n295 = Bundle By Name(cluster=w769, "RTS Config Setup"=w765) -> (w770:T55)
        n296 = call <vilib>:"Add State(s) to Queue__jki_lib_state_machine.vi"("State(s) in (\"\")"=w772) -> ("States Out"=w771:string)  [unwired: 14 in]
      }
      frame "Close Wago Connection" {
        n297 = Unbundle By Name(w782) -> ("Device Connections.Wago ModBus Connection"=w781:refnum<class "Modbus Master.lvclass">)
        n298 = call-dynamic "Shutdown.vi"("error in"=w784, "Modbus master in"=w781) -> ("error out"=w783:errorcluster)  [unwired: 9 in]
        n299 = call <vilib>:"Add State(s) to Queue__jki_lib_state_machine.vi"("State(s) in (\"\")"=w786) -> ("States Out"=w785:string)  [unwired: 14 in]
      }
      frame "Open APLUS Connection" {
        n300 = Unbundle By Name(w792) -> ("Device Connections"=w790:T48, "RTS Config Setup"=w789:T4, "Modbus Remote Port"=w791:u16)
        n301 = local read "Disable APLUS"() -> (w787:bool)
        n302 = case shown="False" w787 {
          tunnel: w794 -> [w804 w805]
          tunnel: [w803 w805] -> w793
          tunnel: w791 -> [w802 _]
          tunnel: w790 -> [w801 w806]
          tunnel: w789 -> [w800 _]
          tunnel: [w799 w806] -> w788
          frame False {
            n303 = call "RTS APLUS Open Close.vi"("Open Connection?"=TRUE, "error in (no error)"=w804, "Modbus Remote Port"=w802, "RTS Config Setup Output"=w800, "Modbus Connections In"=w801) -> ("error out"=w803:errorcluster, "Modbus Connections Out"=w799:T48)  [unwired: 5 in]
          }
          frame True {
          }
        }
        n304 = Bundle By Name(cluster=w792, "Device Connections"=w788) -> (w795:T55)
        n305 = call <vilib>:"Add State(s) to Queue__jki_lib_state_machine.vi"("State(s) in (\"\")"=w797) -> ("States Out"=w796:string)  [unwired: 14 in]
      }
      frame "Close APLUS Connection" {
        n306 = Unbundle By Name(w810) -> ("Device Connections"=w811:T48)
        n307 = local read "Disable APLUS"() -> (w807:bool)
        n308 = case shown="True" w807 {
          tunnel: w811 -> [w817 _]
          tunnel: w809 -> [w815 w818]
          tunnel: [w814 w818] -> w808
          frame False {
            n309 = call "RTS APLUS Open Close.vi"("Open Connection?"=FALSE, "error in (no error)"=w815, "Modbus Connections In"=w817) -> ("error out"=w814:errorcluster)  [unwired: 7 in, 1 out]
          }
          frame True {
          }
        }
        n310 = call <vilib>:"Add State(s) to Queue__jki_lib_state_machine.vi"("State(s) in (\"\")"=w813) -> ("States Out"=w812:string)  [unwired: 14 in]
      }
      frame "Open MX Connection" {
        n311 = Unbundle By Name(w825) -> ("Device Connections"=w824:T48, "RTS Config Setup"=w820:T4)
        n312 = local read "Disable MX"() -> (w819:bool)
        n313 = case shown="False" w819 {
          tunnel: w824 -> [w834 w835]
          tunnel: [w833 w835] -> w823
          tunnel: w822 -> [w832 w836]
          tunnel: [w831 w836] -> w821
          tunnel: w820 -> [w829 _]
          frame False {
            n314 = call "RTS MX Open Close.vi"("Open Connection?"=TRUE, "error in (no error)"=w832, "RTS Config Setup Output"=w829, "Device Connections In"=w834) -> ("error out"=w831:errorcluster, "Device Connections Out"=w833:T48)  [unwired: 6 in]
          }
          frame True {
          }
        }
        n315 = Bundle By Name(cluster=w825, "Device Connections"=w823) -> (w826:T55)
        n316 = call <vilib>:"Add State(s) to Queue__jki_lib_state_machine.vi"("State(s) in (\"\")"=w828) -> ("States Out"=w827:string)  [unwired: 14 in]
      }
      frame "Start Data Save Loop" {
        n317 = call <vilib>:"Add State(s) to Queue__jki_lib_state_machine.vi"("State(s) in (\"\")"=w841) -> ("States Out"=w840:string)  [unwired: 14 in]
        "Start Data Save Loop" <- TRUE
      }
      frame "Close MX Connection" {
        n318 = Unbundle By Name(w844) -> ("Device Connections"=w843:T48)
        n319 = local read "Disable MX"() -> (w842:bool)
        n320 = case shown="False" w842 {
          tunnel: w846 -> [w851 w853]
          tunnel: [w850 w853] -> w845
          tunnel: w843 -> [w849 _]
          frame False {
            n321 = call "RTS MX Open Close.vi"("Open Connection?"=FALSE, "error in (no error)"=w851, "Device Connections In"=w849) -> ("error out"=w850:errorcluster)  [unwired: 7 in, 1 out]
          }
          frame True {
          }
        }
        n322 = call <vilib>:"Add State(s) to Queue__jki_lib_state_machine.vi"("State(s) in (\"\")"=w848) -> ("States Out"=w847:string)  [unwired: 14 in]
      }
      frame "Send Modbus CMD" {
        n323 = Unbundle By Name(w860) -> ("Device Connections"=w854:T48, "Custom Command"=w855:string[])
        n324 = call "RTS Parse Custom CMDs.vi"("Error In"=w858, "Array"=w855, "Device Connections In"=w854) -> ("Error Out"=w857:errorcluster, "Device Connections Out"=w856:T48)  [unwired: 7 in]
        n325 = Bundle By Name(cluster=w860, "Device Connections"=w856) -> (w859:T55)
        n326 = call <vilib>:"Add State(s) to Queue__jki_lib_state_machine.vi"("State(s) in (\"\")"=w862) -> ("States Out"=w861:string)  [unwired: 14 in]
      }
      frame "Send Filename Data" {
        w872 = T58 0 items=["both", "start of string", "end of string"] ("location (both)")
        # "I could probably clean this up a bit. It standard.\nProbably need to just include matrix flips in the \nsubVI and reduce string ops...maybe later"
        # "This VI is used on the \nclient side too"
        n327 = Unbundle By Name(w865) -> ("RTS Config Setup"=w876:T4)
        n328 = call "RTS Build Filename List.vi"("Error In"=w874, "RTS Config Setup"=w876) -> ("Error Out"=w873:errorcluster, "Full Filename List"=w875:string)  [unwired: 8 in]
        n329 = call "RTS Send File Setup Data.vi"("Error In"=w873, "Setup Info"=w875, "Tree Selection"=T53 "", "path"=path "") -> ("Error Out"=w879:errorcluster, "File Setup Data"=w867:string)  [unwired: 6 in]
        n330 = call <vilib>:"Trim Whitespace.vi"("string"=w867, "location (both)"=w872) -> ("trimmed string"=w869:string)
        n331 = Spreadsheet String To Array(delimiter (Tab)=",", format string="%s", spreadsheet string=w869, array type (2D Dbl)=string[][] [] ("Setup Info Station 8")) -> (array=w863:string[][])
        n332 = call <vilib>:"Add State(s) to Queue__jki_lib_state_machine.vi"("State(s) in Front (\"\")"="Output Data" ("State(s) in Front (\"\")"), "State(s) in (\"\")"=w881) -> ("States Out"=w880:string)  [unwired: 13 in]
        n333 = Bundle By Name(cluster=w865, "Send Data"=w863) -> (w864:T55)
      }
      frame "---------- Macro ----------" {
        # "Do not put any code in this frame.\n(It is a separator no-op. You can make a copy of this frame to create a new Macro frame)"
        n334 = call <vilib>:"Add State(s) to Queue__jki_lib_state_machine.vi"("State(s) in (\"\")"=w885) -> ("States Out"=w884:string)  [unwired: 14 in]
      }
      frame "Macro: Initialize" {
        w886 = "Data: Initialize\nInitialize Core Data\nRead Config Files\nUI: Initialize\nUI: Front Panel State >> Open"  # Data: Initialize Initialize Core Data Read Config Files UI: Initialize UI: Front Panel State >> Open
        # "Initialization Macro\n(This is called once, when the VI starts)"
        n335 = call <vilib>:"Add State(s) to Queue__jki_lib_state_machine.vi"("State(s) in Front (\"\")"=w886, "State(s) in (\"\")"=w890) -> ("States Out"=w889:string)  [unwired: 13 in]
      }
      frame "Macro: Exit" {
        (unwired) "Close Wago Connection\nClose APLUS Connection\nClose MX Connection\nData: Cleanup\nExit"
        n336 = Unbundle By Name(w897) -> ("Core.Close Panel on Exit?"=w896:bool)
        n337 = Select(t="UI: Front Panel State >> Close", s=w896, f="") -> (s? t:f=w893:string)
        n338 = call <vilib>:"Add State(s) to Queue__jki_lib_state_machine.vi"("State(s) in (\"\")"=w893, "State(s) at Back (\"\")"="Close Wago Connection\nData: Cleanup\nExit") -> ("States Out"=w891:string)  [unwired: 13 in]
        n339 = call <vilib>:"Add State(s) to Queue__jki_lib_state_machine.vi"("State(s) in Front (\"\")"=w891, "State(s) in (\"\")"=w900) -> ("States Out"=w899:string)  [unwired: 13 in]
      }
      frame "----------General Routine ----------" {
        # "Template Separator\n(You can make a copy of, or modify, this frame)"
        n340 = call <vilib>:"Add State(s) to Queue__jki_lib_state_machine.vi"("State(s) in (\"\")"=w904) -> ("States Out"=w903:string)  [unwired: 14 in]
      }
      frame "Status Check" {
        w913 = 100  # timeout ms
        n341 = Unbundle By Name(w909) -> ("Data.Listener"=w910:refnum<k5>)
        n342 = TCP Wait On Listener(8:w907, 9:w913, 11:w910) -> (0:w912:errorcluster, 4:w911:refnum<k5>)  [unwired: 4 out]
        n343 = case shown="No Error" w912 {
          selector: w912 -> [w917 w926]
          tunnel: w911 -> [w918 _]
          tunnel: w909 -> [w919 w923]
          tunnel: [w916 w923] -> w908
          tunnel: [w917 w924] -> w906
          frame No Error {
            # "Add the new client connection to the state data and go to the 'Send Data' state."
            n344 = in-place {
              in-place-border: w918 -> [w920]
              n345 = in-place-cluster #1(w919) -> ("Data.Clients"=w922:refnum<k5>[])
              n346 = Build Array (concatenate)(w922, w920) -> (w921:refnum<k5>[])
              n347 = in-place-cluster #1("Data.Clients"=w921) -> (w916:T55)
            }
          }
          frame Error {
            # "Ignore timeout errors. If there are any clients, go to the 'Send Data' state."
            n348 = Unbundle By Name(w926) -> ("code"=w925:i32)
            n349 = case shown="Default" w925 {
              tunnel: w926 -> [w927 _]
              tunnel: [w927 w928] -> w924
              frame Default {
              }
              frame 56 {
                w928 = errorcluster {"status"=FALSE, "code"=0, "source"=""}  # no error
              }
            }
          }
        }
        n350 = call <vilib>:"Add State(s) to Queue__jki_lib_state_machine.vi"("State(s) in Front (\"\")"="APLUS 1\nAPLUS 2\nAPLUS 3\nAPLUS 4\nAPLUS 5\nAPLUS 6\nAPLUS 7\nAPLUS 8\nMX 1\nMX 2\nMX 3\nMX 4\nMX 5\nWago Input Image\nWago Output Image\nSave Data\nCheck WH Reset\nOutput Data\nDoor Op Setup\n", "State(s) in (\"\")"=w915) -> ("States Out"=w914:string)  [unwired: 13 in]
      }
      frame "APLUS 1" {
        n351 = Unbundle By Name(w938) -> ("Device Connections.APLUS 1 Modbus Connection"=w935:refnum<class "Modbus Master.lvclass">)
        n352 = call "APLUS Get Data.vi"("Use String Data?"=FALSE, "Debug"="Disable APLUS", "error in (no error)"=w940, "Modbus Master in"=w935) -> ("error out"=w939:errorcluster, "APLUS Data"=w932:string[][], "PowerData"=w934:T22, "Modbus Master out"=w936:refnum<class "Modbus Master.lvclass">)  [unwired: 2 in, 2 out]
        n353 = Index Array(array=w932, index (col)=0 ("disabled index (col)")) -> (element=w930:string[])  [unwired: 1 in]
        n354 = Bundle By Name(cluster=w938, "Device Connections.APLUS 1 Modbus Connection"=w936, "Chamber Data.Station 1"=w934, "Chamber Data.APLUS System Headers"=w930) -> (w937:T55)
        n355 = call <vilib>:"Add State(s) to Queue__jki_lib_state_machine.vi"("State(s) in (\"\")"=w942) -> ("States Out"=w941:string)  [unwired: 14 in]
      }
      frame "APLUS 2" {
        n356 = Unbundle By Name(w948) -> ("Device Connections.APLUS 2 Modbus Connection"=w949:refnum<class "Modbus Master.lvclass">)
        n357 = local read "Disable APLUS"() -> (w943:bool)
        n358 = call "APLUS Get Data.vi"("Use String Data?"=FALSE, "Debug"=w943, "error in (no error)"=w951, "Modbus Master in"=w949) -> ("error out"=w950:errorcluster, "PowerData"=w945:T22, "Modbus Master out"=w946:refnum<class "Modbus Master.lvclass">)  [unwired: 2 in, 3 out]
        n359 = Bundle By Name(cluster=w948, "Device Connections.APLUS 2 Modbus Connection"=w946, "Chamber Data.Station 2"=w945) -> (w947:T55)
        n360 = call <vilib>:"Add State(s) to Queue__jki_lib_state_machine.vi"("State(s) in (\"\")"=w953) -> ("States Out"=w952:string)  [unwired: 14 in]
      }
      frame "APLUS 3" {
        n361 = Unbundle By Name(w957) -> ("Device Connections.APLUS 3 Modbus Connection"=w962:refnum<class "Modbus Master.lvclass">)
        n362 = local read "Disable APLUS"() -> (w954:bool)
        n363 = call "APLUS Get Data.vi"("Use String Data?"=FALSE, "Debug"=w954, "error in (no error)"=w960, "Modbus Master in"=w962) -> ("error out"=w959:errorcluster, "PowerData"=w956:T22, "Modbus Master out"=w961:refnum<class "Modbus Master.lvclass">)  [unwired: 2 in, 3 out]
        n364 = Bundle By Name(cluster=w957, "Device Connections.APLUS 3 Modbus Connection"=w961, "Chamber Data.Station 3"=w956) -> (w958:T55)
        n365 = call <vilib>:"Add State(s) to Queue__jki_lib_state_machine.vi"("State(s) in (\"\")"=w964) -> ("States Out"=w963:string)  [unwired: 14 in]
      }
      frame "APLUS 4" {
        n366 = Unbundle By Name(w969) -> ("Device Connections.APLUS 4 Modbus Connection"=w973:refnum<class "Modbus Master.lvclass">)
        n367 = local read "Disable APLUS"() -> (w965:bool)
        n368 = call "APLUS Get Data.vi"("Use String Data?"=FALSE, "Debug"=w965, "error in (no error)"=w971, "Modbus Master in"=w973) -> ("error out"=w970:errorcluster, "PowerData"=w967:T22, "Modbus Master out"=w972:refnum<class "Modbus Master.lvclass">)  [unwired: 2 in, 3 out]
        n369 = call <vilib>:"Add State(s) to Queue__jki_lib_state_machine.vi"("State(s) in (\"\")"=w975) -> ("States Out"=w974:string)  [unwired: 14 in]
        n370 = Bundle By Name(cluster=w969, "Device Connections.APLUS 4 Modbus Connection"=w972, "Chamber Data.Station 4"=w967) -> (w968:T55)
      }
      frame "APLUS 5" {
        n371 = Unbundle By Name(w980) -> ("Device Connections.APLUS 5 Modbus Connection"=w984:refnum<class "Modbus Master.lvclass">)
        n372 = local read "Disable APLUS"() -> (w976:bool)
        n373 = call "APLUS Get Data.vi"("Use String Data?"=FALSE, "Debug"=w976, "error in (no error)"=w982, "Modbus Master in"=w984) -> ("error out"=w981:errorcluster, "PowerData"=w978:T22, "Modbus Master out"=w983:refnum<class "Modbus Master.lvclass">)  [unwired: 2 in, 3 out]
        n374 = call <vilib>:"Add State(s) to Queue__jki_lib_state_machine.vi"("State(s) in (\"\")"=w986) -> ("States Out"=w985:string)  [unwired: 14 in]
        n375 = Bundle By Name(cluster=w980, "Device Connections.APLUS 5 Modbus Connection"=w983, "Chamber Data.Station 5"=w978) -> (w979:T55)
      }
      frame "APLUS 6" {
        n376 = Unbundle By Name(w991) -> ("Device Connections.APLUS 6 Modbus Connection"=w995:refnum<class "Modbus Master.lvclass">)
        n377 = local read "Disable APLUS"() -> (w987:bool)
        n378 = call "APLUS Get Data.vi"("Use String Data?"=FALSE, "Debug"=w987, "error in (no error)"=w993, "Modbus Master in"=w995) -> ("error out"=w992:errorcluster, "PowerData"=w989:T22, "Modbus Master out"=w994:refnum<class "Modbus Master.lvclass">)  [unwired: 2 in, 3 out]
        n379 = Bundle By Name(cluster=w991, "Device Connections.APLUS 6 Modbus Connection"=w994, "Chamber Data.Station 6"=w989) -> (w990:T55)
        n380 = call <vilib>:"Add State(s) to Queue__jki_lib_state_machine.vi"("State(s) in (\"\")"=w997) -> ("States Out"=w996:string)  [unwired: 14 in]
      }
      frame "APLUS 7" {
        n381 = Unbundle By Name(w1002) -> ("Device Connections.APLUS 7 Modbus Connection"=w1006:refnum<class "Modbus Master.lvclass">)
        n382 = local read "Disable APLUS"() -> (w998:bool)
        n383 = call "APLUS Get Data.vi"("Use String Data?"=FALSE, "Debug"=w998, "error in (no error)"=w1004, "Modbus Master in"=w1006) -> ("error out"=w1003:errorcluster, "PowerData"=w1000:T22, "Modbus Master out"=w1005:refnum<class "Modbus Master.lvclass">)  [unwired: 2 in, 3 out]
        n384 = Bundle By Name(cluster=w1002, "Device Connections.APLUS 7 Modbus Connection"=w1005, "Chamber Data.Station 7"=w1000) -> (w1001:T55)
        n385 = call <vilib>:"Add State(s) to Queue__jki_lib_state_machine.vi"("State(s) in (\"\")"=w1008) -> ("States Out"=w1007:string)  [unwired: 14 in]
      }
      frame "APLUS 8" {
        n386 = Unbundle By Name(w1013) -> ("Device Connections.APLUS 8 Modbus Connection"=w1017:refnum<class "Modbus Master.lvclass">)
        n387 = local read "Disable APLUS"() -> (w1009:bool)
        n388 = call "APLUS Get Data.vi"("Use String Data?"=FALSE, "Debug"=w1009, "error in (no error)"=w1015, "Modbus Master in"=w1017) -> ("error out"=w1014:errorcluster, "PowerData"=w1011:T22, "Modbus Master out"=w1016:refnum<class "Modbus Master.lvclass">)  [unwired: 2 in, 3 out]
        n389 = Bundle By Name(cluster=w1013, "Device Connections.APLUS 8 Modbus Connection"=w1016, "Chamber Data.Station 8"=w1011) -> (w1012:T55)
        n390 = call <vilib>:"Add State(s) to Queue__jki_lib_state_machine.vi"("State(s) in (\"\")"=w1019) -> ("States Out"=w1018:string)  [unwired: 14 in]
      }
      frame "MX 1" {
        n391 = Unbundle By Name(w1026) -> ("Chamber Data"=w1029:T21, "Device Connections"=w1021:T48)
        n392 = call "RTS Get MX Data.vi"("Debug"="Disable MX", "MX Number"=u8 1, "Error In"=w1028, "Device Connections In"=w1021, "Chamber 1 Data in"=w1029) -> ("Error Out"=w1027:errorcluster, "Device Connections Out"=w1020:T48, "Chamber 1 Data out"=w1023:T21)  [unwired: 4 in]
        n393 = Bundle By Name(cluster=w1026, "Chamber Data"=w1023, "Device Connections"=w1020) -> (w1025:T55)
        n394 = call <vilib>:"Add State(s) to Queue__jki_lib_state_machine.vi"("State(s) in (\"\")"=w1031) -> ("States Out"=w1030:string)  [unwired: 14 in]
      }
      frame "MX 2" {
        n395 = Unbundle By Name(w1037) -> ("Chamber Data"=w1038:T21, "Device Connections"=w1033:T48)
        n396 = local read "Disable MX"() -> (w1034:bool)
        n397 = call "RTS Get MX Data.vi"("Debug"=w1034, "MX Number"=u8 2, "Error In"=w1040, "Device Connections In"=w1033, "Chamber 1 Data in"=w1038) -> ("Error Out"=w1039:errorcluster, "Device Connections Out"=w1032:T48, "Chamber 1 Data out"=w1035:T21)  [unwired: 4 in]
        n398 = Bundle By Name(cluster=w1037, "Chamber Data"=w1035, "Device Connections"=w1032) -> (w1036:T55)
        n399 = call <vilib>:"Add State(s) to Queue__jki_lib_state_machine.vi"("State(s) in (\"\")"=w1043) -> ("States Out"=w1042:string)  [unwired: 14 in]
      }
      frame "MX 3" {
        n400 = Unbundle By Name(w1048) -> ("Chamber Data"=w1050:T21, "Device Connections"=w1049:T48)
        n401 = local read "Disable MX"() -> (w1045:bool)
        n402 = call "RTS Get MX Data.vi"("Debug"=w1045, "MX Number"=u8 3, "Error In"=w1052, "Device Connections In"=w1049, "Chamber 1 Data in"=w1050) -> ("Error Out"=w1051:errorcluster, "Device Connections Out"=w1044:T48, "Chamber 1 Data out"=w1046:T21)  [unwired: 4 in]
        n403 = Bundle By Name(cluster=w1048, "Chamber Data"=w1046, "Device Connections"=w1044) -> (w1047:T55)
        n404 = call <vilib>:"Add State(s) to Queue__jki_lib_state_machine.vi"("State(s) in (\"\")"=w1055) -> ("States Out"=w1054:string)  [unwired: 14 in]
      }
      frame "MX 4" {
        n405 = Unbundle By Name(w1060) -> ("Chamber Data"=w1062:T21, "Device Connections"=w1061:T48)
        n406 = local read "Disable MX"() -> (w1057:bool)
        n407 = call "RTS Get MX Data.vi"("Debug"=w1057, "MX Number"=u8 4, "Error In"=w1064, "Device Connections In"=w1061, "Chamber 1 Data in"=w1062) -> ("Error Out"=w1063:errorcluster, "Device Connections Out"=w1056:T48, "Chamber 1 Data out"=w1058:T21)  [unwired: 4 in]
        n408 = Bundle By Name(cluster=w1060, "Chamber Data"=w1058, "Device Connections"=w1056) -> (w1059:T55)
        n409 = call <vilib>:"Add State(s) to Queue__jki_lib_state_machine.vi"("State(s) in (\"\")"=w1067) -> ("States Out"=w1066:string)  [unwired: 14 in]
      }
      frame "MX 5" {
        n410 = Unbundle By Name(w1072) -> ("Chamber Data"=w1074:T21, "Device Connections"=w1073:T48)
        n411 = local read "Disable MX"() -> (w1069:bool)
        n412 = call "RTS Get MX Data.vi"("Debug"=w1069, "MX Number"=u8 5, "Error In"=w1076, "Device Connections In"=w1073, "Chamber 1 Data in"=w1074) -> ("Error Out"=w1075:errorcluster, "Device Connections Out"=w1068:T48, "Chamber 1 Data out"=w1070:T21)  [unwired: 4 in]
        n413 = Bundle By Name(cluster=w1072, "Chamber Data"=w1070, "Device Connections"=w1068) -> (w1071:T55)
        n414 = call <vilib>:"Add State(s) to Queue__jki_lib_state_machine.vi"("State(s) in (\"\")"=w1079) -> ("States Out"=w1078:string)  [unwired: 14 in]
      }
      frame "Wago Input Image" {
        n415 = Unbundle By Name(w1087) -> ("Device Connections.Wago ModBus Connection"=w1088:refnum<class "Modbus Master.lvclass">, "Wago Data Input"=w1089:T43)
        n416 = call "Wago Input Image.vi"("Error In"=w1081, "Wago Data Input"=w1089, "Modbus Master in"=w1088) -> ("Error Out"=w1080:errorcluster, "Wago Data Output"=w1084:T43, "Modbus master out"=w1085:refnum<class "Modbus Master.lvclass">)  [unwired: 6 in]
        n417 = Unbundle By Name(w1084) -> ("Input Process Image.Measured Input Data (Target)"=w1083:T28, "Input Process Image.Software Constants.Room PID Settings"=w1082:T30)
        n418 = Bundle By Name(cluster=w1087, "Device Connections.Wago ModBus Connection"=w1085, "Wago Data Input"=w1084, "Chamber Data.Measured Input Data (Target)"=w1083, "Chamber Data.Room PID Settings"=w1082) -> (w1086:T55)
        n419 = call <vilib>:"Add State(s) to Queue__jki_lib_state_machine.vi"("State(s) in (\"\")"=w1091) -> ("States Out"=w1090:string)  [unwired: 14 in]
      }
      frame "Wago Output Image" {
        n420 = Unbundle By Name(w1098) -> ("Device Connections.Wago ModBus Connection"=w1100:refnum<class "Modbus Master.lvclass">, "Wago Data Input"=w1099:T43)
        n421 = call "Wago Output Image.vi"("error in (no error)"=w1102, "Wago Data"=w1099, "Modbus Master in"=w1100) -> ("error out"=w1101:errorcluster, "Wago Data Output"=w1095:T43, "Modbus Master out"=w1096:refnum<class "Modbus Master.lvclass">)  [unwired: 6 in]
        "Wago Data Output" <- w1095
        n422 = Unbundle By Name(w1095) -> ("Output Data Process Image.Room Conditions (Measured)"=w1094:T31, "Output Data Process Image.Door Output Relays"=w1093:T25, "Output Data Process Image.Contactor Settings(*All Check Out)"=w1092:T26)
        n423 = Bundle By Name(cluster=w1098, "Device Connections.Wago ModBus Connection"=w1096, "Wago Data Input"=w1095, "Chamber Data.Room Conditions (Measured)"=w1094, "Chamber Data.Door Output Relays"=w1093, "Chamber Data.Contactor Settings(*All Check Out)"=w1092) -> (w1097:T55)
        n424 = call <vilib>:"Add State(s) to Queue__jki_lib_state_machine.vi"("State(s) in (\"\")"=w1104) -> ("States Out"=w1103:string)  [unwired: 14 in]
      }
      frame "Save Data" {
        n425 = Unbundle By Name(w1114) -> ("CSV Data Save"=→"TDMS Data Save Loop":T2, "RTS Config Setup"=w1111:T4, "Chamber Data"=w1115:T21, "CSV Data Save"=w1106:T2)
        "RTS Config Setup Save Loop" <- w1111
        n426 = call "RTS Server Save Data.vi"("All Data?"="All Data?", "RTS Config Setup Output"=w1111, "Error In"=w1116, "TDMS Data Save In"=w1106, "Chamber 1 Data in"=w1115) -> ("Error Out"=w1110:errorcluster, "Custom Saved Titles"=→"Custom Saved Title Save Loop":T1, "TDMS Data Save Out"=w1105:T2, "Send Data"=w1112:string[][])  [unwired: 3 in]
        "CSV Data Save Out" <- w1105
        n427 = Bundle By Name(cluster=w1114, "Send Data"=w1112, "CSV Data Save"=w1105) -> (w1113:T55)
        n428 = call <vilib>:"Add State(s) to Queue__jki_lib_state_machine.vi"("State(s) in (\"\")"=w1118) -> ("States Out"=w1117:string)  [unwired: 14 in]
      }
      frame "Check WH Reset" {
        n429 = Unbundle By Name(w1125) -> ("Device Connections"=w1123:T48, "CSV Data Save"=w1122:T2)
        n430 = call "RTS Check WH Reset.vi"("Error In"=w1120, "TDMS Data Save in"=w1122, "Device Connections in"=w1123) -> ("Error Out"=w1119:errorcluster, "Device Connections out"=w1121:T48)  [unwired: 7 in]
        n431 = Bundle By Name(cluster=w1125, "Device Connections"=w1121) -> (w1124:T55)
        n432 = call <vilib>:"Add State(s) to Queue__jki_lib_state_machine.vi"("State(s) in (\"\")"=w1127) -> ("States Out"=w1126:string)  [unwired: 14 in]
      }
      frame "Output Data" {
        # "Post data to the \nclients"
        n433 = Unbundle By Name(w1140) -> ("Chamber Data"=→"Chamber Data":T21, "RTS Config Setup"=w1133:T4, "Send Data"=w1137:string[][], "Data"=w1141:T54, "CSV Data Save"=w1132:T2)
        "Server to Client Data" <- w1137
        n434 = call "RTS Equipment Send TCP Data.vi"("RTS Config Setup Input"=w1133, "Error In"=w1143, "TDMS Data Save"=w1132, "Data"=w1141, "Send Data"=w1137) -> ("Error Out"=w1142:errorcluster, "# of Connections"=→"Chamber 1 Connections":i32, "Data Out"=w1135:T54, "RTS Config Setup Output"=w1134:T4, "Custom Commands"=w1130:string[], "TDMS Data Save Output"=w1131:T2, "Read Door CMD"=w1128:string)
        "Custom Commands" <- w1130
        "Read Door CMD" <- w1128
        n435 = call "RTS Send Custom Command.vi"("Custom Commands"=w1130, "Read Door CMD in"=w1128) -> ("States"=w1129:string)  [unwired: 8 in, 1 out]
        n436 = local write "RTS Config Setup Output"(w1134) -> ()
        n437 = Bundle By Name(cluster=w1140, "CSV Data Save"=w1131, "RTS Config Setup"=w1134, "Data"=w1135, "Custom Command"=w1130) -> (w1139:T55)
        n438 = call <vilib>:"Add State(s) to Queue__jki_lib_state_machine.vi"("State(s) in Front (\"\")"=w1129, "State(s) in (\"\")"=w1145) -> ("States Out"=w1144:string)  [unwired: 13 in]
      }
      frame "Read Door Setup" {
        n439 = Unbundle By Name(w1150) -> ("RTS Config Setup"=w1153:T4, "All Door Opener Ctrl"=w1147:T13)
        n440 = call "RTS Read Latest Pattern Data.vi"("Error In"=w1152, "All Door Opener Ctrl in"=w1147, "RTS Config Setup"=w1153) -> ("Error Out"=w1151:errorcluster, "All Door Opener Ctrl out"=w1148:T13)  [unwired: 7 in]
        n441 = Bundle By Name(cluster=w1150, "All Door Opener Ctrl"=w1148) -> (w1149:T55)
        n442 = call <vilib>:"Add State(s) to Queue__jki_lib_state_machine.vi"("State(s) in Front (\"\")"="Set Chamber Parameters" ("x"), "State(s) in (\"\")"=w1154) -> ("States Out"=w1155:string)  [unwired: 13 in]
      }
      frame "Door Op Setup" {
        n443 = Unbundle By Name(w1166) -> ("Wago Data Input.Output Data Process Image.Door Output Relays"=w1163:T25, "Device Connections.Wago ModBus Connection"=w1165:refnum<class "Modbus Master.lvclass">, "All Door Opener Ctrl"=w1158:T13, "RTS Config Setup"=w1157:T4)
        n444 = call "RTS Door Op Setup.vi"("Door Output Relays"=w1163, "Error In"=w1169, "RTS Config Setup Input"=w1157, "All Door Opener Ctrl in"=w1158, "Input"=w1165) -> ("Error Out"=w1168:errorcluster, "RTS Config Setup Output"=w1156:T4, "All Door Opener Ctrl out"=w1159:T13, "Output"=w1164:refnum<class "Modbus Master.lvclass">, "States"=w1162:string)  [unwired: 2 in]
        n445 = Bundle By Name(cluster=w1166, "Device Connections.Wago ModBus Connection"=w1164, "All Door Opener Ctrl"=w1159, "RTS Config Setup"=w1156) -> (w1167:T55)
        n446 = call <vilib>:"Add State(s) to Queue__jki_lib_state_machine.vi"("State(s) in (\"\")"=w1162) -> ("States Out"=w1161:string)  [unwired: 14 in]
        n447 = call <vilib>:"Add State(s) to Queue__jki_lib_state_machine.vi"("State(s) in (\"\")"=w1161, "State(s) at Back (\"\")"="Display Door Ops" ("State(s) in Front (\"\")")) -> ("States Out"=w1170:string)  [unwired: 13 in]
      }
      frame "Door Ops 1" {
        # "The sequencial kinda works. I have\nto move on. I have almost 3 weeks tinkering\nwith this...real pain.\n\nIt does not work when i change order. Need\nto fix"
        n448 = Unbundle By Name(w1178) -> ("Wago Data Input.Output Data Process Image.Door Output Relays"=w1173:T25, "Device Connections.Wago ModBus Connection"=w1174:refnum<class "Modbus Master.lvclass">, "All Door Opener Ctrl"=w1175:T13)
        n449 = call "RTS Door Ops Sequence Delay.vi"("Door Output Relays"=w1173, "Station #"=u8 1, "error in (no error)"=w1180, "All Door Opener Ctrl in"=w1175, "Wago ModBus Connection"=w1174) -> ("error out"=w1172:errorcluster, "All Door Opener Ctrl out"=w1176:T13, "Modbus Master Out"=w1171:refnum<class "Modbus Master.lvclass">)  [unwired: 4 in]
        n450 = Bundle By Name(cluster=w1178, "Device Connections.Wago ModBus Connection"=w1171, "All Door Opener Ctrl"=w1176) -> (w1179:T55)
        n451 = call <vilib>:"Add State(s) to Queue__jki_lib_state_machine.vi"("State(s) in (\"\")"=w1182) -> ("States Out"=w1181:string)  [unwired: 14 in]
      }
      frame "Door Ops 2" {
        n452 = Unbundle By Name(w1192) -> ("Wago Data Input.Output Data Process Image.Door Output Relays"=w1187:T25, "Device Connections.Wago ModBus Connection"=w1186:refnum<class "Modbus Master.lvclass">, "All Door Opener Ctrl"=w1184:T13)
        n453 = call "RTS Door Ops Sequence Delay.vi"("Door Output Relays"=w1187, "Station #"=u8 2, "error in (no error)"=w1189, "All Door Opener Ctrl in"=w1184, "Wago ModBus Connection"=w1186) -> ("error out"=w1188:errorcluster, "All Door Opener Ctrl out"=w1185:T13, "Modbus Master Out"=w1183:refnum<class "Modbus Master.lvclass">)  [unwired: 4 in]
        n454 = Bundle By Name(cluster=w1192, "Device Connections.Wago ModBus Connection"=w1183, "All Door Opener Ctrl"=w1185) -> (w1191:T55)
        n455 = call <vilib>:"Add State(s) to Queue__jki_lib_state_machine.vi"("State(s) in (\"\")"=w1194) -> ("States Out"=w1193:string)  [unwired: 14 in]
      }
      frame "Door Ops 3" {
        n456 = Unbundle By Name(w1199) -> ("Wago Data Input.Output Data Process Image.Door Output Relays"=w1203:T25, "Device Connections.Wago ModBus Connection"=w1202:refnum<class "Modbus Master.lvclass">, "All Door Opener Ctrl"=w1201:T13)
        n457 = call "RTS Door Ops Sequence Delay.vi"("Door Output Relays"=w1203, "Station #"=u8 3, "error in (no error)"=w1197, "All Door Opener Ctrl in"=w1201, "Wago ModBus Connection"=w1202) -> ("error out"=w1196:errorcluster, "All Door Opener Ctrl out"=w1200:T13, "Modbus Master Out"=w1195:refnum<class "Modbus Master.lvclass">)  [unwired: 4 in]
        n458 = Bundle By Name(cluster=w1199, "Device Connections.Wago ModBus Connection"=w1195, "All Door Opener Ctrl"=w1200) -> (w1198:T55)
        n459 = call <vilib>:"Add State(s) to Queue__jki_lib_state_machine.vi"("State(s) in (\"\")"=w1206) -> ("States Out"=w1205:string)  [unwired: 14 in]
      }
      frame "Door Ops 4" {
        n460 = Unbundle By Name(w1208) -> ("Wago Data Input.Output Data Process Image.Door Output Relays"=w1215:T25, "Device Connections.Wago ModBus Connection"=w1214:refnum<class "Modbus Master.lvclass">, "All Door Opener Ctrl"=w1213:T13)
        n461 = call "RTS Door Ops Sequence Delay.vi"("Door Output Relays"=w1215, "Station #"=u8 4, "error in (no error)"=w1211, "All Door Opener Ctrl in"=w1213, "Wago ModBus Connection"=w1214) -> ("error out"=w1210:errorcluster, "All Door Opener Ctrl out"=w1212:T13, "Modbus Master Out"=w1207:refnum<class "Modbus Master.lvclass">)  [unwired: 4 in]
        n462 = Bundle By Name(cluster=w1208, "Device Connections.Wago ModBus Connection"=w1207, "All Door Opener Ctrl"=w1212) -> (w1209:T55)
        n463 = call <vilib>:"Add State(s) to Queue__jki_lib_state_machine.vi"("State(s) in (\"\")"=w1218) -> ("States Out"=w1217:string)  [unwired: 14 in]
      }
      frame "Door Ops 5" {
        n464 = Unbundle By Name(w1223) -> ("Wago Data Input.Output Data Process Image.Door Output Relays"=w1227:T25, "Device Connections.Wago ModBus Connection"=w1226:refnum<class "Modbus Master.lvclass">, "All Door Opener Ctrl"=w1225:T13)
        n465 = call "RTS Door Ops Sequence Delay.vi"("Door Output Relays"=w1227, "Station #"=u8 5, "error in (no error)"=w1221, "All Door Opener Ctrl in"=w1225, "Wago ModBus Connection"=w1226) -> ("error out"=w1220:errorcluster, "All Door Opener Ctrl out"=w1224:T13, "Modbus Master Out"=w1219:refnum<class "Modbus Master.lvclass">)  [unwired: 4 in]
        n466 = Bundle By Name(cluster=w1223, "Device Connections.Wago ModBus Connection"=w1219, "All Door Opener Ctrl"=w1224) -> (w1222:T55)
        n467 = call <vilib>:"Add State(s) to Queue__jki_lib_state_machine.vi"("State(s) in (\"\")"=w1230) -> ("States Out"=w1229:string)  [unwired: 14 in]
      }
      frame "Door Ops 6" {
        n468 = Unbundle By Name(w1235) -> ("Wago Data Input.Output Data Process Image.Door Output Relays"=w1239:T25, "Device Connections.Wago ModBus Connection"=w1238:refnum<class "Modbus Master.lvclass">, "All Door Opener Ctrl"=w1237:T13)
        n469 = call "RTS Door Ops Sequence Delay.vi"("Door Output Relays"=w1239, "Station #"=u8 6, "error in (no error)"=w1233, "All Door Opener Ctrl in"=w1237, "Wago ModBus Connection"=w1238) -> ("error out"=w1232:errorcluster, "All Door Opener Ctrl out"=w1236:T13, "Modbus Master Out"=w1231:refnum<class "Modbus Master.lvclass">)  [unwired: 4 in]
        n470 = Bundle By Name(cluster=w1235, "Device Connections.Wago ModBus Connection"=w1231, "All Door Opener Ctrl"=w1236) -> (w1234:T55)
        n471 = call <vilib>:"Add State(s) to Queue__jki_lib_state_machine.vi"("State(s) in (\"\")"=w1242) -> ("States Out"=w1241:string)  [unwired: 14 in]
      }
      frame "Door Ops 7" {
        n472 = Unbundle By Name(w1247) -> ("Wago Data Input.Output Data Process Image.Door Output Relays"=w1251:T25, "Device Connections.Wago ModBus Connection"=w1250:refnum<class "Modbus Master.lvclass">, "All Door Opener Ctrl"=w1249:T13)
        n473 = call "RTS Door Ops Sequence Delay.vi"("Door Output Relays"=w1251, "Station #"=u8 7, "error in (no error)"=w1245, "All Door Opener Ctrl in"=w1249, "Wago ModBus Connection"=w1250) -> ("error out"=w1244:errorcluster, "All Door Opener Ctrl out"=w1248:T13, "Modbus Master Out"=w1243:refnum<class "Modbus Master.lvclass">)  [unwired: 4 in]
        n474 = Bundle By Name(cluster=w1247, "Device Connections.Wago ModBus Connection"=w1243, "All Door Opener Ctrl"=w1248) -> (w1246:T55)
        n475 = call <vilib>:"Add State(s) to Queue__jki_lib_state_machine.vi"("State(s) in (\"\")"=w1254) -> ("States Out"=w1253:string)  [unwired: 14 in]
      }
      frame "Door Ops 8" {
        n476 = Unbundle By Name(w1259) -> ("Wago Data Input.Output Data Process Image.Door Output Relays"=w1263:T25, "Device Connections.Wago ModBus Connection"=w1262:refnum<class "Modbus Master.lvclass">, "All Door Opener Ctrl"=w1261:T13)
        n477 = call "RTS Door Ops Sequence Delay.vi"("Door Output Relays"=w1263, "Station #"=u8 8, "error in (no error)"=w1257, "All Door Opener Ctrl in"=w1261, "Wago ModBus Connection"=w1262) -> ("error out"=w1256:errorcluster, "All Door Opener Ctrl out"=w1260:T13, "Modbus Master Out"=w1255:refnum<class "Modbus Master.lvclass">)  [unwired: 4 in]
        n478 = Bundle By Name(cluster=w1259, "Device Connections.Wago ModBus Connection"=w1255, "All Door Opener Ctrl"=w1260) -> (w1258:T55)
        n479 = call <vilib>:"Add State(s) to Queue__jki_lib_state_machine.vi"("State(s) in (\"\")"=w1266) -> ("States Out"=w1265:string)  [unwired: 14 in]
      }
      frame "Set Chamber Parameters" {
        # "This checks the current chamber \nsetpoints and compares them to the \ndesired...if different.. it changes it. Only\nworks during door ops. Only changes temp and \nhumidity. You can change Cool and Dehum\ntemp without an effect. (Long term, I want to\nput Cool and Dehum on a software PID)"
        n480 = Unbundle By Name(w1277) -> ("Chamber Data.Measured Input Data (Target).Room Setpoints"=w1271:T29, "All Door Opener Ctrl"=w1272:T13, "Device Connections.Wago ModBus Connection"=w1278:refnum<class "Modbus Master.lvclass">)
        "Room Setpoints Set Parameter Algo" <- w1271
        "All Door Opener Ctrl 2" <- w1272
        n481 = call "RTS Set Chamber Temp Humidity.vi"("Room Setpoints"=w1271, "All Door Opener Ctrl"=w1272, "Error In"=w1274, "Modbus Master in"=w1278) -> ("Error Out"=w1273:errorcluster, "Matching Setpoints?"=→"Matching Setpoints?":bool, "Set Chamber Conditions"=→"Set Chamber Conditions":bool, "Modbus master out"=w1275:refnum<class "Modbus Master.lvclass">, "Chamber 1-1"=→"Chamber Setpoint Reference":T16, "Index"=→"Index":i32)  [unwired: 2 in]
        n482 = Bundle By Name(cluster=w1277, "Device Connections.Wago ModBus Connection"=w1275) -> (w1276:T55)
        n483 = call <vilib>:"Add State(s) to Queue__jki_lib_state_machine.vi"("State(s) in (\"\")"=w1280) -> ("States Out"=w1279:string)  [unwired: 14 in]
      }
      frame "Display Door Ops" {
        n484 = Unbundle By Name(w1282) -> ("Wago Data Input.Output Data Process Image.Door Output Relays"=→"Door Output Relays":T25, "All Door Opener Ctrl"=w1281:T13)
        n485 = local write "All Door Opener Ctrl"(w1281) -> ()
        n486 = call <vilib>:"Add State(s) to Queue__jki_lib_state_machine.vi"("State(s) in (\"\")"=w1286) -> ("States Out"=w1285:string)  [unwired: 14 in]
      }
    }
    n487 = case shown="True" "Main Array" {
      tunnel: w29 -> [w44 w47]
      tunnel: w26 -> [_ w46]
      tunnel: [w44 w45] -> w28
      frame False {
      }
      frame True {
        n488 = Build Array (concatenate)(w47, w46) -> (w45:string[])
      }
    }
    "Main Array" <- w28
  }
  "Error Out" <- w10
  n489 = call <vilib>:"Add State(s) to Queue__jki_lib_state_machine.vi"("State(s) in (\"\")"="Data: Initialize") -> ("States Out"=w9:string)  [unwired: 14 in]
  n490 = while "Data Save" {
    shift-right: [w1297] -> _
    shift-left: _ -> [w1296]
    shift-right: [w1300] -> _
    shift-left: _ -> [w1295]
    shift-right: [w1299] -> _
    shift-left: w9 -> [w1301]
    shift-right: [w1288] -> _
    shift-left: string[] [] -> [w1291]
    tunnel: w3 -> [w1287]
    stop <- w1298 stop-if-true
    # "Data Save Loop"
    n491 = call <vilib>:"Parse State Queue__jki_lib_state_machine.vi"("State Queue"=w1301, "Error In (no error)"=w1295) -> ("Remaining States"=w1303:string, "Current State"=w1289:string, "Arguments"=w1302:string)  [unwired: 11 in]
    n492 = Multiply(x="Save Rate (Sec)", y=1000) -> (x*y=w1292:i32)
    n493 = case shown="\"Save Data\"" w1289 {
      selector: w1289 -> [_ _ w1341 _ _ _ _ _ _ _ _]
      tunnel: w1303 -> [w1314 w1340 w1345 w1357 w1362 w1366 w1372 w1380 w1405 w1415 w1421]
      tunnel: w1302 -> [_ _ _ _ _ _ _ _ _ _ _]
      tunnel: w1296 -> [w1312 w1337 w1343 w1354 w1360 w1363 _ w1377 w1397 w1413 w1419]
      tunnel: [w1311 w1338 w1347 errorcluster {"status"=FALSE, "code"=0, "source"=""} ("error out") w1359 w1364 w1369 w1378 w1402 w1410 w1418] -> w1300
      tunnel: w1295 -> [w1310 w1338 w1346 w1353 w1359 w1364 w1369 w1378 w1403 w1411 w1418]
      tunnel: [w1313 w1339 w1344 w1356 w1361 w1365 w1371 w1379 w1404 w1414 w1420] -> w1299
      tunnel: [_ _ _ _ TRUE _ _ _ _ _ _] -> w1298
      tunnel: [w1309 w1337 w1343 w1354 w1360 w1363 w1370 w1377 w1396 w1413 w1419] -> w1297
      tunnel: w1292 -> [w1308 _ _ _ _ _ _ _ _ _ _]
      tunnel: w1287 -> [_ _ _ _ _ _ _ _ _ w1412 _]
      frame "", "Event Structure", "Idle" {
        n494 = event shown="[0] Timeout" {
          selector: _ -> [_]
          dyn-events: _ -> [_]
          timeout: w1308 -> [_]
          tunnel: w1314 -> [w1331]
          tunnel: [w1330] -> w1313
          tunnel: w1312 -> [w1328]
          tunnel: [w1329] -> w1311
          tunnel: w1310 -> [w1329]
          tunnel: [w1328] -> w1309
          event Timeout {
            n495 = event-data() -> ()  [unwired: 1 in, 1 out]
            n496 = local read "CSV Data Save Out"() -> (w1326:T2)
            n497 = Unbundle By Name(w1326) -> ("CSV File Location"=w1325:path, "CSV File Location 2"=w1324:path, "CSV File Location 3"=w1323:path, "CSV File Location 4"=w1322:path, "CSV File Location 5"=w1321:path, "CSV File Location 6"=w1320:path, "CSV File Location 7"=w1319:path, "CSV File Location 8"=w1318:path)
            n498 = Build Array(w1325, w1324, w1323, w1322, w1321, w1320, w1319, w1318) -> (w1317:path[])
            n499 = for {
              tunnel: w1317 -> [w1336] mode=indexing
              tunnel: [w1334] -> w1316 mode=indexing
              n500 = Equal?(x=w1336, y=path "") -> (x = y?=w1334:bool)
            }
            n501 = And Array Elements(Boolean array=w1316) -> (logical AND=w1315:bool)
            n502 = case shown="False" w1315 {
              tunnel: ["Save Data\nCheck Exit" ("State(s) in Front (\"\")") "Check Exit" ("State(s) in Front (\"\")")] -> w1327
              frame False {
              }
              frame True {
              }
            }
            n503 = call <vilib>:"Add State(s) to Queue__jki_lib_state_machine.vi"("State(s) in Front (\"\")"=w1327, "State(s) in (\"\")"=w1331) -> ("States Out"=w1330:string)  [unwired: 13 in]
          }
        }
      }
      frame "---------- Core ----------" {
        # "Do not put any code in this frame.\n(it is a separator no-op)"
        n504 = call <vilib>:"Add State(s) to Queue__jki_lib_state_machine.vi"("State(s) in (\"\")"=w1340) -> ("States Out"=w1339:string)  [unwired: 14 in]
      }
      frame Default {
        w1350 = 42 items=["No error", "Argument error", "Memory is full", "Out of zone", "End of file", "File already open", "Generic file I/O error", "File not found", "File permission error", "Disk is full", "Duplicate path", "Too many files open", "System feature not enabled", "Resource file not found", "Cannot add resource", "Resource not found", "Image not found", "Image memory error", "Pen does not exist", "Config type invalid", "Config token not found", "Config parse error", "Config memory error", "Bad external code format", "Bad external code offset", "External code not present", "Null window", "Destroy window error", "Null menu", "Print aborted", "Bad print record", "Print driver error", "Windows error during printing", "Memory error during printing", "Print dialog error", "Generic print error", "Invalid device refnum", "Device not found", "Device parameter error", "Device unit error", "Cannot open device", "Device call aborted", "Generic error", "Cancelled by user", "Object ID too low", "Object ID too high", "Object not in heap", "Unknown heap", "Unknown object (invalid DefProc)", "Unknown object (DefProc not in table)", "Message out of range", "Invalid (null) method", "Unknown message", "Manager call not supported", "Bad address", "Network operation in progress", "Network operation timed out", "Connection is busy", "Network attribute not supported", "Network error", "Address in use", "System out of memory", "Connection aborted", "Connection refused", "Not connected", "Already connected", "Connection closed", "Initialization error (interapplication manager)", "Bad occurrence", "Wait on unbound occurrence handler", "Occurrence queue overflow", "Datalog type conflict", "Unused", "Unrecognized type (interapplication manager)", "Memory corrupt", "Failed to make temporary DLL", "Old CIN version", "Drag socket not found", "Failed to load drop-object", "Failed to register OLE object", "Failed to release OLE object", "Format specifier type mismatch", "Unknown format specifier", "Too few format specifiers", "Too many format specifiers", "Scan failed", "Newer CIN version", "Error converting to variant", "Runtime menu error", "Password tampered", "Variant attribute not found", "Incompatible variant data type", "Event data is not available", "Event Store is not present", "Occurrence is not found", "Event Queue is not created", "Event info is not available", "Refnum passed is NULL", "Error retrieving Class GUID", "Error retrieving CoClass GUID", "Error retrieving TypeLib GUID.", "Bad built application magic bytes.", "Specific driver is different from the specific driver associated with the Logical Name.", "There is no session opened to the class driver.", "Max Error", "MAX - Error with config objects", "MAX - Error loading configuration", "MAX - Group not supported"]
        # "Current State"
        # "Do not delete, rename, or modify this frame.\n(this is used to capture unhandled states and typos)"
        # "Handle mistyped state name (developer tool)"
        n505 = Format Into String(format string="Software Exception: Unhandled State \"%s\"." ("message"), error in=w1346, w1341) -> (resulting string=w1349:string, error out=w1348:errorcluster)  [unwired: 1 in]
        n506 = call <vilib>:"Error Cluster From Error Code.vi"("show call chain? (False)"=TRUE, "error in (no error)"=w1348, "error message (\"\")"=w1349, "error code (0)"=w1350) -> ("error out"=w1347:errorcluster)  [unwired: 5 in]
        n507 = call <vilib>:"Add State(s) to Queue__jki_lib_state_machine.vi"("State(s) in (\"\")"=w1345) -> ("States Out"=w1344:string)  [unwired: 14 in]
      }
      frame "Error Handler" {
        # "Unhandled Error -- Display it"
        # "Handle any errors here.\nYou can also output any states to clean-up after errors occur"
        # "Clear error"
        n508 = call <vilib>:"General Error Handler.vi"("error in (no error)"=w1353) -> ()  [unwired: 10 in, 5 out]
        n509 = call <vilib>:"Add State(s) to Queue__jki_lib_state_machine.vi"("State(s) in Front (\"\")"="/* Post Error States", "State(s) in (\"\")"=w1357) -> ("States Out"=w1356:string)  [unwired: 13 in]
      }
      frame "Exit" {
        # "Do not put any code in this frame.\n(No errors that occur here will be handled.)"
        n510 = call <vilib>:"Add State(s) to Queue__jki_lib_state_machine.vi"("State(s) in (\"\")"=w1362) -> ("States Out"=w1361:string)  [unwired: 14 in]
      }
      frame "---------- Data ----------" {
        # "Do not put any code in this frame.\n(It is a separator no-op. You can make a copy of this frame to create a new Data frame)"
        n511 = call <vilib>:"Add State(s) to Queue__jki_lib_state_machine.vi"("State(s) in (\"\")"=w1366) -> ("States Out"=w1365:string)  [unwired: 14 in]
      }
      frame "Data: Initialize" {
        # "Initialize the shift-register data, here.\n(data names are defined by what you wire into the bundle function)"
        n512 = while {
          tunnel: [w1376] -> w1368
          tunnel: [w1373] -> w1367
          stop <- w1375 stop-if-true
          w1373 = T2 {"CSV File Location"=path "", "CSV File Location 2"=path "", "CSV File Location 3"=path "", "CSV File Location 4"=path "", "CSV File Location 5"=path "", "CSV File Location 6"=path "", "CSV File Location 7"=path "", "CSV File Location 8"=path "", "Save References"={"CSV 1"=refnum, "CSV 2"=refnum, "CSV 3"=refnum, "CSV 4"=refnum, "CSV 5"=refnum, "CSV 6"=refnum, "CSV 7"=refnum, "CSV 8"=refnum}}  # CSV Data Save (Updated)
          (unwired) T3 {"CSV 1"=refnum, "CSV 2"=refnum, "CSV 3"=refnum, "CSV 4"=refnum, "CSV 5"=refnum, "CSV 6"=refnum, "CSV 7"=refnum, "CSV 8"=refnum}  # Save References
          w1376 = T57 {"Current VI Reference"=refnum, "Close Panel on Exit?"=FALSE}  # Core
          n513 = local read "Start Data Save Loop"() -> (w1375:bool)
          n514 = Wait Until Next ms Multiple(millisecond multiple=u32 100) -> ()  [unwired: 1 out]
        }
        n515 = Bundle("Core"=w1368, "CSV Data Save (Updated)"=w1367) -> (w1370:T60)  [unwired: 1 in]
        n516 = call <vilib>:"Add State(s) to Queue__jki_lib_state_machine.vi"("State(s) in (\"\")"=w1372) -> ("States Out"=w1371:string)  [unwired: 14 in]
      }
      frame "---------- Data Save Stuff ----------" {
        # "Template Separator\n(You can make a copy of, or modify, this frame)"
        n517 = call <vilib>:"Add State(s) to Queue__jki_lib_state_machine.vi"("State(s) in (\"\")"=w1380) -> ("States Out"=w1379:string)  [unwired: 14 in]
      }
      frame "Save Data" {
        # "The locations come from the client...which is processed in the above loop...and \nsend to this loop"
        # "I offload the references to this loop.\nProbably a better way..but seems to work"
        n518 = local read "Custom Saved Title Save Loop"() -> (w1401:T1)
        n519 = local read "CSV Data Save Out"() -> (w1399:T2)
        n520 = Unbundle By Name(w1397) -> ("CSV Data Save (Updated).Save References"=w1395:T3)
        n521 = local read "RTS Config Setup Save Loop"() -> (w1400:T4)
        n522 = Bundle By Name(cluster=w1399, "Save References"=w1395) -> (w1398:T2)
        n523 = call "RTS Save Cluster.vi"("error in (no error)"=w1403, "RTS Config Setup Save Loop"=w1400, "CSV Data Save Loop"=w1398, "Custom Saved Title Save Loop"=w1401) -> ("error out"=w1402:errorcluster, "CSV Data Save Output"=w1381:T2)  [unwired: 6 in]
        n524 = Unbundle By Name(w1381) -> ("Save References"=w1394:T3)
        n525 = Equal?(x=w1395, y=w1394) -> (x = y?=w1392:T61)
        n526 = Unbundle By Name(w1392) -> ("CSV 1"=w1391:bool, "CSV 2"=w1390:bool, "CSV 3"=w1389:bool, "CSV 4"=w1388:bool, "CSV 5"=w1387:bool, "CSV 6"=w1386:bool, "CSV 7"=w1385:bool, "CSV 8"=w1384:bool)
        n527 = Build Array(w1391, w1390, w1389, w1388, w1387, w1386, w1385, w1384) -> (w1383:bool[])
        n528 = And Array Elements(Boolean array=w1383) -> (logical AND=w1382:bool)
        n529 = Bundle By Name(cluster=w1397, "CSV Data Save (Updated)"=w1381) -> (w1396:T60)
        n530 = case shown="False" w1382 {
          tunnel: ["Send Event" ("State(s) in Front (\"\")") "" ("State(s) in Front (\"\")")] -> w1393
          frame False {
          }
          frame True {
          }
        }
        n531 = call <vilib>:"Add State(s) to Queue__jki_lib_state_machine.vi"("State(s) in Front (\"\")"=w1393, "State(s) in (\"\")"=w1405) -> ("States Out"=w1404:string)  [unwired: 13 in]
      }
      frame "Send Event" {
        n532 = Unbundle By Name(w1413) -> ("CSV Data Save (Updated)"=w1409:T2)
        n533 = Generate User Event(priority (normal)=usereventprio."high priority", user event=w1412, event data cluster=w1409, error in=w1411) -> (error out=w1410:errorcluster)  [unwired: 1 out]
        n534 = call <vilib>:"Add State(s) to Queue__jki_lib_state_machine.vi"("State(s) in (\"\")"=w1415) -> ("States Out"=w1414:string)  [unwired: 14 in]
      }
      frame "Check Exit" {
        n535 = local read "Exit"() -> (w1416:bool)
        n536 = case shown="False" w1416 {
          tunnel: ["" ("State(s) in Front (\"\")") "Exit" ("State(s) in Front (\"\")")] -> w1417
          frame False {
          }
          frame True {
          }
        }
        n537 = call <vilib>:"Add State(s) to Queue__jki_lib_state_machine.vi"("State(s) in Front (\"\")"=w1417, "State(s) in (\"\")"=w1421) -> ("States Out"=w1420:string)  [unwired: 13 in]
      }
    }
    n538 = case shown="True" "Save Array" {
      tunnel: w1291 -> [w1304 w1307]
      tunnel: w1289 -> [_ w1306]
      tunnel: [w1304 w1305] -> w1288
      frame False {
      }
      frame True {
        n539 = Build Array (concatenate)(w1307, w1306) -> (w1305:string[])
        "Save Array" <- w1305
      }
    }
  }
  n540 = call <vilib>:"Simple Error Handler.vi"("error in (no error)"=w10) -> ()  [unwired: 1 in, 8 out]
